vi "UHR-Fleezers Control (host) - 10.2.vi"() -> ()   [LabVIEW 2010]
uses:
  <vilib>/rvi/interface/nirviMethod/nirviMethod.xnode
  <vilib>/rvi/interface/nirviCloseFPGA/nirviCloseFPGA.xnode
  <vilib>/express/express analysis/Spectral/XNode/ExpressSpectralMeasurementsBlockNode.xnode
  <vilib>/rvi/interface/nirviReadWriteControl/nirviReadWriteControl.xnode
  <vilib>/Analysis/NI_AALBase.lvlib
  <vilib>/express/express analysis/Spectral/Block/exnSpectralBlock spectral measurements PSD poly.vi
  <vilib>/rvi/interface/nirviOpenFPGA/nirviOpenFPGA.xnode
  <vilib>/vision/Avi1.llb/AviRefnum.ctl
  <vilib>/Platform/TimedLoop/XDataNode/XDataNode.xnode
  <vilib>/Platform/TimedLoop/XDataNode/nitl_modes.ctl
  <vilib>/Platform/TimedLoop/XDataNode/XDNodeRunTimeDep.lvlib
  <vilib>/Platform/TimedLoop/XDataNode/wakeup.ctl
  <vilib>/Platform/TimedLoop/XDataNode/timing_clust.ctl
  <vilib>/Utility/miscctls.llb/LVPoint32TypeDef.ctl
  <vilib>/userDefined/High Color/nirio_resource_hc.ctl
  openfpgaref.8.6.ctl
  <vilib>/Utility/miscctls.llb/LVMinMaxIncTypeDef.ctl
  <vilib>/rvi/errors/niLvFpgaWhatHappensToTopLevelVI.ctl
  <vilib>/rvi/interface/common/niFpgaNodeNameForErrorReporting.ctl
  <vilib>/rvi/errors/niLvFpgaAdjustHostInterfaceError.vi
  <vilib>/vision/NI_Vision_Development_Module.lvlib
  <vilib>/Instr/_visa.llb/VISA Configure Serial Port (Instr).vi
  <vilib>/RVI Host/nirviSupport.llb/nirviErrorClusterFromErrorCode.vi
  FPGA Bitfiles/UHR-Fleezers Instr~3C_FPGA Target_UHR-Fleezers Contr~4B.lvbitx
  <vilib>/Waveform/WDTOps.llb/WDT Append Waveforms DBL.vi
  <vilib>/express/express analysis/Spectral/Block/exnSpectralBlock spectral measurements PSD WFM.vi
  UHR-Fleezers Control (fpga) - 10.3.vi
  FPGA Bitfiles/UHR-Fleezers Instr~F0_FPGA Target_UHR-Fleezers Contr~5A.lvbitx
  <vilib>/FPGAPlugInAG/PCIe-7852R/niLvFpga_Close_PCIe-7852R.vi
panel:
  in  "Sample Channel Flow":bool
  in  "Pump 3 contents":string="Left: ADig beads" caption="contents"
  in  "Pump 1 contents":string="Right: DNA beads" caption="contents"
  in  "Scripts":T1(tab)=enum."Stepping data"
  in  "Take Stepping Data":bool
  in  "Cap 1 Samp Flow ON":bool=TRUE
  in  "Cap 2 Samp Flow ON":bool=TRUE
  in  "Got DNA bead":bool
  in  "Got ADig bead":bool
  in  "Cap 2 Flow ON":bool=TRUE
  in  "Cap 1 Flow ON":bool=TRUE
  in  "Cap 2 T ON":bool=TRUE
  in  "Move Cap. 2 (ADig Left)":bool
  in  "Move Cap. 1 (DNA Right)":bool
  in  "Cal/Data Acq. Spot":bool
  in  "Dump Beads":bool
  in  "Lower Ch. Cap.":bool
  in  "Cap 1 T ON":bool=TRUE
  in  "Offset 2 Set":dbl=2.0
  in  "Offset 1 Set":dbl
  in  "Cal @ (MHz)":dbl=15.0
  in  "W/ Offset 1":bool=TRUE
  in  "Offset 1 Start (MHz)":dbl=13.0
  in  "W/ Offset 2":bool=TRUE
  in  "Offset 2 Start (MHz)":dbl=16.0
  in  "Move to Delta 2 (MHz)":dbl=13.0
  in  "Attempt Limit":dbl=30.0 caption="Limit"
  out "Attempts":dbl=1.0
  in  "Wait Before Save (s)":u32=1
  in  "Fish for Tether":bool
  in  "Closest Delta (MHz)":dbl=9.5 step=0.25
  in  "Stop F (pN)":dbl=3.0
  in  "Then...":string(combo)="5"
  in  "Move to Delta 1 (MHz)":dbl=13.0
  in  "Tether Alarm?":bool=TRUE
  out "Tether":bool
  in  "TA Cancel Save?":bool=TRUE
  in  "TA Green Off?":bool=TRUE
  in  "Raster Set Upon Tether":u32=1
  in  "Save at end (5, 6)":bool
  in  "N Steps":dbl=20.0
  in  "Step Size (nm)":dbl=0.34
  in  "Save ave factor":dbl=1.0
  in  "Dip Trap Delta 1 (MHz)":dbl=15.0
  in  "Move Trap Before?":bool
  in  "Save Data After?":bool
  in  "Green ON After?":bool
  in  "Dip Trap Delta 2 (MHz)":dbl=15.0
  in  "Move Trap After?":bool
  in  "Duration (s)":dbl=1.0
  in  "Dip for Protein":bool
  in  "APD to Watch":bool
  out "Duration (s)":dbl
  in  "Action":string(combo)="Yank"
  in  "Fl. Triggered...":bool
  in  "Fl. Delta Thresh. (kHz)":dbl=0.6
  out "Waiting":bool
  out "Fl. High":bool
  in  "N pts to average":u16=6
  in  "Yank Delay (s)":dbl=3.5
  in  "Yank to Delta Array (MHz)":dbl[](array[numeric])=[16.3, 15.85, 14.85]
  in  "N Array El":u8=3 min=1 step=1
  in  "Random Choice":bool=TRUE
  in  "Force Yank":bool
  in  "Force Reset":bool
  in  "Y change (mm)":dbl
  in  "Profile":bool
  out "Current Position":cluster{dbl, dbl, dbl}
  out "Sigma/Mean 2":dbl=nan caption="Sigma/Mean" format="%#_2g"
  out "Rate sigma (Hz) 2":dbl caption="Sigma (Hz)" format="%0.2f"
  out "APD 2 Rate (Hz)":dbl format="%#_3p"
  out "Primary Video Display":T2(plugin-control)
  out "Waveform Graph":dbl[](graph) caption="APD Line Scan"
  in  "Inject Pump 3":bool
  in  "Inject Pump 1":bool
  out "Messages":string="4:54 PM\tLost tether (723 s).\r4:42 PM\tFormed tether in 1 attempt(s).\r4:41 PM\tLost tether (470 s).\r4:34 PM\tFormed tether in 7 attempt(s).\r4:32 PM\tLost tether (992 s).\r4:15 PM\tFormed tether in 1 attempt(s).\r4:14 PM\tLost tether (454 s).\r4:06 PM\tFormed tether in 5 attempt(s).\r4:05 PM\tLost tether (206 s).\r4:01 PM\tFormed tether in 3 attempt(s).\r4:00 PM\tLost tether (153 s).\r3:57 PM\tFormed tether in 5 attempt(s).\r3:56 PM\tLost tether (759 s).\r3:43 PM\tFormed tether in 17 attempt(s).\r3:39 PM\tUHR-Fleezers ready.\r"
  in  "APD Ave N":dbl=10.0
  out "Int. Time (s)":dbl=3.0
  in  "Stop All":bool=TRUE
  out "Sigma/Mean":dbl=nan format="%#_2g"
  out "Rate sigma (Hz)":dbl caption="Sigma (Hz)" format="%0.2f"
  in  "Tab Control 6":T3(tab)
  in  "APD 2 Offset":dbl
  in  "APD 1 Offset":dbl
  out "RMS (Ang)":dbl=2.2363215515597568 format="%_2g"
  in  "Bead Sep. Int. Time (s)":dbl=5.0 caption="Int. Time (s)"
  in  "Below (kHz)":dbl=0.5
  in  "Above (kHz)":dbl=2.0
  in  "Adjust Scale\nto Mean":bool
  in  "Rescale on Mean":bool
  in  "Offset (nm)":dbl
  out "Mean":dbl=0.35502251163091847 caption="Mean (pN)" format="%#_3g"
  out "Force":waveform(dbl)[](graph)=[{"t0"=timestamp(4478.100000001255 s since 1904-01-01), "dt"=0.15, "Y"=[0.6544682133105884, 0.6829563430169571], "attributes"=variant("NI_ChannelName"=variant(string "T1 X"))}, {"t0"=timestamp(4478.100000001255 s since 1904-01-01), "dt"=0.15, "Y"=[0.05685503756215739, 0.025810452633971234], "attributes"=variant("NI_ChannelName"=variant(string "T2 X"))}]
  out "APD Chart":waveform(dbl)[](graph)=[{"t0"=timestamp(4478.100000001255 s since 1904-01-01), "dt"=0.15, "Y"=[0.0, 0.0], "attributes"=variant("NI_ChannelName"=variant(string "APD 1"))}, {"t0"=timestamp(4478.100000001255 s since 1904-01-01), "dt"=0.15, "Y"=[0.0, 0.0], "attributes"=variant("NI_ChannelName"=variant(string "APD 2"))}]
  in  "Calibration":u16(ring)=2 items=["None", "Position", "Force"]
  out "T1 X":dbl=0.6687122781637727 caption="T1 X (pN)" format="%0.2f"
  out "T2 X":dbl=-0.04133274509806431 caption="T2 X (pN)" format="%0.2f"
  out "Bead Separation":waveform(dbl)(graph)={"t0"=timestamp(4478.100000001255 s since 1904-01-01), "dt"=0.15, "Y"=[-2.9090620115549504, -2.8815158675481127], "attributes"=variant("NI_ChannelName"=variant(string "T1 X"))}
  in  "Amplitude (nm)":dbl=3.0
  out "Bead Mean (nm)":dbl=-2.9725093766937554 caption="Mean (nm)" format="%0.2f"
  out "Difference":dbl=0.6273795330657084 caption="Difference (pN)" format="%.2g"
  in  "Take Detection Laser\nImage":bool
  out "APD 2":T2(plugin-control) caption="APD 2 (Cy5)"
  in  "Flip Green Filter":bool
  in  "Set X Only":bool
  in  "Set Y Only":bool
  out "APD 1":T2(plugin-control) caption="APD 1 (Cy3)"
  out "Detection Laser Y":T2(plugin-control)
  out "Pointer Y (V)":dbl format="%_3g"
  out "Pointer X (V)":dbl format="%_3g"
  in  "Set Confocal Spot (X-Y)":bool
  out "Detection Laser X":T2(plugin-control)
  out "Saved APD":dbl[][](graph) caption="Most Recent Time Trace"
  out "Trap Delta Graph":dbl[](graph)=[-89.38744840610437, -89.37006347356015, -89.24966097161428, -89.27535644051642, -89.22559285551776, -88.86555051929984, -88.57164165504085, -88.51902465601101, -88.63501771008777, -89.20867383045751, -89.55461281382372, -89.55813284408976, -89.07876691073398, -89.12824891342606, -88.87613266846802, -89.2801470410057, -89.52897456305874, -89.30818962554463, -89.2603892282628, -89.55143394553988, -89.11898533922138, -89.25742201435101, -88.7246017921867, -89.05704019082833, -89.00438612954582, -89.05564776220227, -89.01771654795576, -88.8637677243877, -88.73420125440117, -88.90230035101814, -88.93449064288166, -88.68475787636112, -88.71497640229151, -88.98867971389947, -88.98987818265206, -88.8663554218612, -89.21049798942109, -88.87888603452649, -88.83494841134385, -88.8517410807533, -88.94938680318202, -88.98692447842114, -89.13767155188884, -89.05931890170092, -89.08641661114396, -89.05365179724527, -89.20227840355159, -89.31178251999566, -89.45607605619048, -88.83940363384923, -89.15369570967569, -89.08546468517298, -89.05175431278485, -88.87130156752026, -89.02771493961416, -89.34443740021561, -89.4552359343601, -89.16107171540548, -89.11889587027639, -89.3436162545047, -89.33942660204508, -89.3473584178231, -89.19585027499929, -89.139379143746, -89.2555989459276, -89.20141717607427, -89.21660561984382, -89.46769272591796, -89.07315603501014, -89.03933689450355, -89.0993712485838, -89.35756915821324, -89.35331075709209, -89.22317576092196, -89.508816612592, -89.2518218067191, -89.20936039087964, -89.44092145450193, -89.6477278697556, -89.08293610392039, -89.53347805395603, -89.64410456441405, -89.35761400349834, -89.34886843709035, -89.37851091701371, -89.41649939174766, -89.36071107503787, -89.57311912534034, -89.63101869252588, -89.43405030861993, -89.31069880452256, -89.3430526304503, -89.21823174554396, -89.21501556105062, -88.9111722206407, -89.18733719432157, -89.18722963976052, -89.32292422573383, -89.39588663013811, -89.82453679095343, -89.10638459364176, -89.47188371738739, -89.54185028737668, -89.5729147724991, -89.54460422995446, -89.18025179411762, -89.34220054522804, -89.5575088561865, -89.42069201414144, -89.26950662803745, -89.10557494488836, -89.34610419003715, -89.49955675225459, -89.22456738111956, -89.2027117963072, -89.1349219342003, -89.14160870895898, -89.33136024231399, -89.33342512716312, -89.37714552414755, -89.3803929736005, -89.35573543764183, -89.52038271838603, -89.27965821960461, -89.35600452793587, -89.22650740978278, -89.22614620509182, -89.12635779184048, -89.48788165476256, -89.13068590269111, -89.17357255767598, -89.08072258562063, -88.86940497190369, -88.77122041116284, -88.99968531958817, -89.00921784902013, -88.81448561314173, -88.84031989144572, -89.39146413421481, -88.86339059547717, -89.1673772901552, -89.15159384824292, -89.06085219395777, -89.51260432037202, -89.5536217833934, -88.98677652908017, -89.2701030586531, -89.24195272293136, -89.71292340734871, -89.2910030757885, -89.47786455696955, -89.48954430167501, -89.26584207463125, -89.10233578501436, -89.17707533292848, -89.305147933605, -89.18901651866418, -89.34296303989353, -89.09380910376896, -89.463391307056, -89.57679916102225, -88.71111300258505, -88.94498405110207, -88.49140535622053, -88.7341514685107, -88.89889681017223, -88.59002712151397, -88.76524603655983, -88.87121714891552, -89.1510876045764, -88.91862351911718, -88.82548575374531, -88.80051417887705, -88.54837294030075, -88.87140478869503, -88.89456579635265, -89.0056346348357, -88.55907846911137, -88.66759749781659, -88.44149474414237, -88.6870846816969, -88.6466799778529, -88.63814297254739, -88.78805261976106, -88.96824024662688, -89.1103699249511, -89.3905085878867, -88.9323741748437, -88.75430601059085, -88.82089140957092, -89.4535647245052, -88.85616866717044, -88.79523221810146, -88.9348514263713, -89.16871433406047, -88.67265636299146, -88.56040235473944, -88.91232897311664, -88.8089571372157, -88.91314583351732, -88.88683122051, -88.68204457129616, -88.85998808560862, -89.14884267359204, -89.22322206568205, -88.95108210276138, -88.64718246491319, -89.13249650680967, -88.76829543884, -88.95527962559021, -89.21056707808899, -89.0089527300235, -88.91866866096028, -88.80863987306557, -88.80089852688, -88.78342735706066, -88.56360335694336, -88.67735013119068, -88.59275253806658, -88.69077558769106, -89.13757241655324, -88.73750458538608, -88.78152831683693, -88.99066615201534, -88.82091590097372, -88.82476418112773, -88.85316711473837, -88.66503995216488, -88.79388285985826, -88.9563338555671, -88.71352135994421, -88.83999603213721, -88.74633806352192, -88.60900128977838, -88.53872550741977, -88.18424116231269, -88.3705578352791, -88.62148742046897, -88.54394496460543, -88.36251412656927, -88.4093878967337, -88.50258216055909, -88.35494559212471, -88.34341283426755, -88.37395270939074, -88.4979905289099, -88.46189758015758, -88.26844057461545, -88.2326502387395, -88.55042578244075, -88.63499132099773, -88.51319899426838, -88.73389987228151, -88.26715288988908, -88.21859961845635, -88.58277595542361, -88.59002127369436, -88.55251451009755, -88.37746006671004, -88.41015869076773, -88.51995467108634, -88.20521115956211, -88.2804480699595, -88.43819946605072, -88.33640124221915, -88.6531593764619, -88.34679755650652, -88.52043428631671, -88.95056941775016, -89.15761826470202, -89.0652452180153, -89.29976884961121, -89.28829699493275, -88.2664323951737, -88.30873224535377, -88.44209877116936, -88.24099191432931, -88.22287833843131, -88.29139893670066, -88.46447280750237, -88.3910852296664, -88.29985148131229, -88.30822091752688, -88.28362819582696, -88.48902213455159, -88.54998575425876, -88.60669758609019, -88.49144847059677, -88.16296003837576, -88.51396970073476, -88.33982443813122, -88.22394802157045, -88.29260704896129, -88.41055824500185, -88.33497551461949, -88.67759606488578, -88.58700366093623, -88.35694653040895, -88.47296601718023, -88.33423129919967, -88.47752188464662, -88.35512247733888, -88.3777986712967, -88.729655522916, -88.73598917774595, -88.51630362857102, -88.2074894465274, -88.29181479700983, -88.4672686755314, -88.16849552794635, -88.5951381838874, -88.13062428528687, -88.17216964798284, -88.10524634348789, -88.27800416343854, -88.13335451761374, -88.37825316932381, -88.56140566187452, -88.4425002811831, -88.0656866086508, -88.42547083397028, -88.25095406936146, -88.30824818401392, -87.68332283229768, -88.17932407982077, -88.1532062150512, -88.53375395739056, -88.30311164463794, -88.41589198652929, -88.30407778660808, -88.40367169747444, -88.3437214846239, -88.35594639765567, -88.45652784227724, -88.5842630911653, -88.41297448484298, -88.54859586632723, -88.58103611816637, -88.84792541633075, -88.01907631016554, -87.95324520506506, -87.78481343426844, -87.95560385851115, -87.85804482449285, -88.18551136231898, -88.01656053816524, -88.02895257484454, -87.92828548442509, -87.79710285471337, -88.00738538313797, -87.73682830549747, -88.07275568855894, -87.99433270558389, -87.72770755009651, -87.9267710314997, -87.96904944990774, -87.9253259336599, -88.05705393409421, -88.01203421488725, -87.91328847459181, -87.8071326736109, -88.01735651800155, -88.01900222553235, -87.9545136667229, -88.12450941379944, -87.93910654707737, -87.87354402092201, -87.92735293954016, -88.19340411458231, -88.30401091141142, -87.95775584337821, -87.73163787609764, -88.15344693968393, -87.96650228747762, -88.11064491691332, -87.54860462573924, -88.09354412638375, -87.8519133361432, -87.85881854278162, -88.20509785833131, -87.91760524446005, -87.95035519016639, -88.04278622326103, -88.02524699015602, -88.15194655200104, -88.00407435605808, -88.05793027060378, -87.77335005358424, -88.16544477454528, -87.89450200769897, -88.13982524656109, -87.97826541537938, -88.16268206508684, -87.71879293293877, -87.94985415206207, -87.8064061100325, -87.99934582850895, -88.22615609606846, -87.86093151137626, -87.6700537142207, -88.03078580167295, -87.87513742989012, -87.82347052576961, -87.94732046431275, -88.1156839391357, -88.20232764763225, -88.2994531521694, -88.18386916539099, -88.09031322297545, -88.15313742433287, -87.80239936551692, -87.60250611850887, -87.64533018569459, -87.60991041695632, -87.72676066199486, -87.33559917500989, -87.45284913194946, -87.25817364254561, -87.65430559235227, -87.53602431965585, -87.39786877894335, -87.58615486117924, -87.43227285896955, -87.71344886287676, -87.23377729485536, -87.64014203399677, -87.60239562637292, -87.2919811059202, -87.37115314323583, -87.37275952371664, -87.15051723589367, -87.39185774051927, -87.48653698268699, -87.45749749831653, -87.18067937552632, -87.27483719659506, -87.41864167455336, -87.25027078789361, -86.98471314584748, -87.28270035864435, -87.57027222590403, -87.7665499148163, -87.37999966120944, -87.28971186976376, -87.52306556218589, -87.36410821351811, -87.48529464229739, -87.44136200138482, -87.58907511569913, -87.78643723152783, -87.55681182743275, -87.48385705148843, -87.63330822003329, -87.61184020150489, -87.71616882826622, -87.5282648586323, -87.57071058488614, -87.57236293781206, -87.31757130397664, -87.77813876094464, -87.6257729513794, -87.69068528914049, -87.84520252155934, -87.86085934550638, -87.88195380904611, -87.60311641516779, -87.69122196636401, -87.8020108027814, -87.83361495277228, -87.67067092860452, -87.58389183513452, -87.56129213793758, -87.85975339337645, -87.40220585601887, -87.91728954021838, -87.75864018540607, -87.74689815457056, -87.68245059351156, -88.18451430943892, -87.88738917293477, -87.63757611994254, -87.5708434435605, -87.77278345407868, -87.93142286703629, -87.86352661774805, -87.76673769548492, -88.01908196291075, -87.89074636276199, -87.72684473268411, -87.57289839262214, -87.71597780604532, -87.78577424237625, -87.69032008091057, -87.62589406030267, -87.8174289613667, -87.67707669627433, -87.51845749917389, -87.71466525148008, -87.5606836249847, -87.7139674908129, -87.74094794957122, -87.7005157479694, -87.76640578300322, -87.70527246506592, -87.71611718410986, -87.81476293350636, -87.79251662258699, -87.88265447337088, -87.75795727658604, -87.9823722895671, -88.0836963787135, -87.62714330665065, -88.0089934508544, -87.40707301914264, -88.05177962004032, -87.8229318229869, -87.94390489036448, -87.84493365424993, -87.59509612382958, -87.72856415566281, -87.81497085062107, -87.92128557509571, -87.75918240002704, -87.93548815031771, -87.9012355596515, -87.54139193308774, -87.55828881541663, -87.51056903539299, -87.52039866561812, -87.63682624093673, -87.5432671707731, -87.64742561154168, -87.3288423556632, -87.48046022363206, -87.58910493044621, -87.6911525123038, -87.37349047159623, -87.4448807965905, -87.28808399952601, -87.54929046394128, -87.45969579508173, -87.58502984558035, -87.80226057043029, -88.0303971858355, -87.60810918962494, -87.84113021898624, -87.54927790962793, -87.56484012122169, -87.28054131732654, -87.70220256814717, -87.76341332349702, -87.54370605152829, -87.79205016647634, -88.09313027253401, -88.0620175534996, -87.94063041986826, -87.96896727307845, -87.80256403811197, -87.67239701062852, -87.6399317276719, -87.65889725479741, -87.28729774193249, -87.5214594744474, -87.62016692063344, -87.62735969457016, -87.45027005933, -87.21012664990556, -87.06867512023265, -87.33435958229319, -87.3177444330734, -87.34788825501778, -87.56436416954135, -87.61950903708983, -87.55425148575165, -87.55083323246308, -87.68012788709825, -87.51834206500418, -87.69598428135353, -87.71876397280123, -87.44913472298718, -87.6048484121969, -87.864444966875, -87.5501946692936, -87.45216722120793, -87.58237945926253, -87.78969615154085, -87.67686931387769, -87.5522680359406, -87.44068603371, -87.76799995194563, -87.60672463029596, -87.38968106380253, -87.63066293473824, -88.02940059078153, -87.86955200993, -87.9565636486737, -86.8106204704307, -87.18970625895963, -87.86114644151831, -87.58153303504436, -87.35048262951038, -87.51654038824094, -87.52922696429981, -87.36262242324574, -87.41629136303413, -87.28824237872385, -87.4798012921965, -87.41374424314733, -87.49898141290439, -87.49418606631315, -87.51862153043166, -87.71063407904339, -87.6430033186609, -87.57827338876646, -87.54690816845391, -87.37313105200109, -87.46919199453606, -87.25478433494307, -87.57636908224944, -87.58441520954747, -87.54338977306715, -87.67092323117731, -87.75299003095911, -87.48833905986369, -87.68958700633844, -87.45965031693086, -87.66116717927812, -87.27532000081274, -87.57990013934989, -87.3358908739909, -87.50397985078497, -87.46173599047975, -87.48897346231755, -87.72646057917159, -87.92686417098798, -87.66179360238937, -87.71096805882274, -87.58618277512232, -87.6988941155976, -87.5326287528062, -87.80961641383038, -87.30238479981065, -87.03358687200033, -87.2089031253125, -87.2851268921435, -87.57229679049586, -87.6250778220362, -87.63097627402095, -87.57340931013754, -87.37087860062384, -87.44919654211628, -87.55770928649892, -87.32390714182918, -87.3792060612991, -87.82257062874059, -87.91123683327902, -87.65663152557195, -87.45233009538237, -87.4503607791947, -87.44856346726229, -87.54674508286985, -87.48734914385216, -87.53493633794486, -87.77322141957666, -87.5360093515083, -87.92890453759716, -87.74937580384537, -88.0245676727105, -87.68532561768353, -87.63053250593893, -87.78213147465999, -87.78859059897012, -87.86455124009606, -87.82301747913752, -87.74384895388138, -87.53642726658066, -87.70265895169524, -87.6807943581295, -87.67232336986555, -87.55827287052955, -88.07948443555617, -87.63008108422747, -87.5546049107237, -88.02124763911905, -87.79747135539168, -87.69866730651353, -87.4907995965221, -87.66252496338981, -87.66651266475806, -87.32618843167079, -87.56224440214163, -87.7667193383105, -87.67475148682402, -87.67403549332289, -87.95538747106701, -87.84275776737468, -87.87501919379514, -87.71447099135949, -87.38634807332252, -87.67076191051662, -87.5610535281519, -87.72945280500126, -87.77329172363045, -87.58111844851547, -87.392924048304, -87.99966297359707, -87.66302572401112, -87.70180504315596, -87.7633988137739, -87.49898068274233, -87.60398327290125, -87.55264054889946, -87.7317147994365, -87.44896090874326, -87.73988451581835, -87.6824066023823, -87.7957256934875, -87.61022656628427, -87.63754876347582, -87.5711889574363, -87.81578244682522, -87.51567128404804, -87.5154423142066, -87.52661520916558, -87.90110240253, -87.72240271355116, -87.68284011358159, -87.47969610871385, -87.59549328973137, -87.49486631433797, -87.46292721937864, -87.53242593240981, -87.45177658061101, -87.49650273688985, -87.42222432382316, -87.40924809559812, -87.46155584573685, -87.67740538525773, -87.56795415780982, -87.38569221168117, -87.72497836510254, -87.63212095662197, -87.84874086155294, -87.68423502594806, -87.69248881745025, -87.55053270519312, -87.63792276742947, -87.79361374259113, -87.82594928518766, -88.02381615123241, -87.78573568385676, -87.627134578756, -87.48447531083156, -87.73805939615202, -87.48798012324937, -87.33294279112297, -87.4083676430875, -87.2125741263701, -87.64422154601172, -87.79647571090814, -87.60503235567646, -87.468032119514, -87.5182669364431, -87.69978210057371, -87.50350852296302, -87.05604169095596, -87.54120213385531, -87.52140297291606, -87.40543345419292, -87.5303247718758, -87.53081075788629, -87.29491010008809, -87.55816400580258, -87.41618663405671, -87.40015492786631, -87.66754109572479, -87.64535395323043, -87.7226826283207, -87.76140908067617, -87.55084152605826, -87.67412930855458, -87.66651847157189, -87.59259808382153, -87.76203239123596, -87.82422546599133, -87.83988157302704, -87.63815911780895, -87.49616243720268, -87.33562809133211, -87.4146581786975, -87.57917461085796, -87.58962249843225, -87.530135156205, -87.09582028024963, -87.24486712722238, -87.41117686085059, -87.43803047596957, -87.73298888735778, -87.54712937634724, -87.46411106964821, -87.54784999696707, -87.56584887970729, -87.4903532769867, -87.51231599593729, -87.33147942981621, -87.36305774594335, -87.89964736785245, -87.53883983178878, -87.53308382106005, -87.47942176100906, -87.56968963749078, -87.69694395129795, -87.60185059154233, -87.40409833135215, -87.48565441094152, -87.45295785173542, -87.8598746465701, -87.63829115936099, -87.72329824070167, -87.57755847822077, -87.34233590638961, -87.2456387390855, -87.69022291588266, -87.73497292018078, -87.67861746974165, -87.86636101340743, -87.86785313484236, -87.63076103469672, -87.73204340004872, -87.79896896759101, -87.81165856747944, -87.78886319309825, -87.47167338848682, -87.79033896032894, -87.7394988120906, -87.3593100996421, -87.67569559372204, -87.77973202885244, -87.55832238989285, -87.79523137457565, -87.47172572986554, -87.69117985917633, -87.8026233792443, -87.68335651454673, -87.71072805299252, -87.35688163306679, -87.68247685399328, -88.04111074383601, -87.71006837060239, -87.56964717410253, -87.67187827443692, -87.39882043046879, -87.49501995524523, -87.29313321533394, -87.58729015911976, -87.27415480591418, -87.553455177222, -87.28462813652112, -87.39034628415033, -87.58108941169114, -87.44564719863513, -87.53436292084444, -87.33001410378813, -87.36337024723107, -87.63510719338177, -87.65980368332251, -87.43363496068739, -87.4255269325382, -87.41182525493925, -87.72815339935283, -87.67216110676736, -87.72283448284864, -87.6723969435237, -87.6560403010696, -87.38016535112635, -87.55609880554229, -87.5762178841565, -87.72026364293265, -87.69566289957541, -87.31489376030962, -87.52499386095835, -87.56560915150533, -87.71637669594824, -87.65296554469052, -87.78329628957886, -87.76052147520979, -87.86389250978719, -87.60691705192471, -87.73801394328754, -87.53083942658031, -87.4768796085828, -87.78184542579447, -87.54612819815853, -87.36965481448632, -87.4204871602231, -87.50661200564672, -87.4524351274625, -87.76563007263547, -87.81140346193699, -87.35314925668533, -86.10503470178419, -89.85266012832051, -89.64460892206411, -89.63573878694366, -89.67437474838317, -89.43897047411551, -89.3737613977331, -89.28788917865882, -89.58069848429386, -89.53810567580396, -89.37138670815206, -89.42570077300456, -89.54084483748144, -89.38127981165223, -89.5094888428512, -89.43628497289689, -89.82742727406759, -89.58878997780671, -89.05083051594639, -89.2715449510282, -89.18302882011236, -89.11757972469984, -89.450025337766, -89.4918182082358, -89.48714535759302, -89.45673286538067, -89.3721865723953, -89.22628822081519, -89.54189155991992, -89.3527578161816, -89.55295636678755, -89.61525268024653, -89.60177253387754, -89.35091333052947, -89.65096893870835, -89.43826482992947, -89.26405785507977, -89.13333984803354, -89.27090710005496, -89.61146885238918, -89.38160521758422, -89.41398091645064, -89.56444238217698, -89.55467011390908, -89.49128237350648, -89.50437810521063, -89.49811847441696, -89.58142008085757, -89.70565907063485, -89.79032016312806, -89.49368126396514, -89.43538457890372, -89.22236432143751, -89.30147719799409, -89.6871672866815, -89.39666762420819, -89.53287835086593, -89.53103400899184, -89.30264681130458, -89.20241016917116, -89.20185024762415, -89.14667769335148, -89.4091163236507, -89.5303897169196, -89.37364072083844, -89.36478136588747, -89.52127318590307, -89.47972650316281, -89.5730482533163, -89.62064623540789, -89.5836723763713, -89.51543500545677, -89.38239305279464, -89.62184644095112, -89.7728958272249, -89.683935508047, -89.67854975684114, -89.50641274850042, -89.66409060311157, -89.22826919030574, -89.5351698052126, -89.52386617594226, -89.5762566923911, -89.12011896829341, -89.39440120296695, -89.31526150363645, -89.40699770807561, -89.27641788881832, -88.9980934526029, -89.22189882622396, -89.18320922801408, -89.07312242319608, -88.83297400882918, -89.2234100301694, -88.85288595229059, -89.2377991335614, -89.35741830027712, -89.26107817432187, -89.43580762503471, -89.41514590200433, -89.45677685231738, -89.34136783820585, -89.21998788359926, -88.86601818955353, -89.36404024707687, -89.18530760698397, -89.43678951078016, -89.18406807997061, -89.37969189195263, -89.62263416697985, -89.37304214824837, -89.3440877767074, -89.3598322726397, -89.34954279527221, -89.19348306086874, -89.2146973031071, -89.43625648517998, -89.34417299103697, -89.52160411222111, -89.53337708387906, -89.342069859851, -89.5743618155725, -89.30272336229824, -89.15741114850327, -89.21817485093237, -89.30503477455262, -89.36081784103939, -89.52459993172579, -89.6111165131166, -89.2619524554189, -89.35664568024671, -89.22996326941124, -89.42804922425438, -89.42197549285336, -89.62869122920705, -89.38083285342586, -89.54868019256227, -89.31926914035074, -89.55393076075502, -89.39585117735736, -89.56232500771125, -89.58429220453907, -89.2853335425489, -88.9554979363846, -89.82366236227894, -90.03241697822503, -89.87535834289318, -89.68803825964758, -89.90985739705187, -89.65052212097332, -89.63592492369258, -89.68901377113175, -89.61580926284557, -89.47648673035042, -89.5763572557888, -89.62979756653974, -89.48581314130413, -89.60156409856245, -89.521773057561, -89.2283702112482, -89.36270907008742, -89.3762029830632, -89.37264199967436, -89.47817702167433, -88.96620231000924, -89.54818090594742, -89.80996257603499, -89.63617690920825, -89.27694912725786, -89.17404501094248, -89.36048391493902, -88.88941872416451, -88.84313652275561, -89.25869975047635, -89.51915145305644, -89.3148346155159, -89.23949602638928, -89.27060642492778, -88.82059631185331, -89.22377299622616, -89.40471068902889, -89.67545363713047, -89.7105622164905, -89.59379751329226, -89.43763803920422, -89.73367902969775, -89.25258989064338, -88.92196116042703, -89.49284759320145, -89.43652161750485, -89.14923694928899, -89.31570366092012, -89.14198709968517, -89.22103878715308, -89.31243636768616, -89.35968282595243, -89.45840321040957, -88.9639394112719, -89.41425315620818, -89.36940537708537, -89.43031076815686, -89.20706343917448, -89.43495800271168, -89.29789897809772, -89.17597071053217, -89.2602152121373, -89.55991216232033, -89.13369209792404, -89.26909295138859, -89.3238551922488, -89.48669087227324, -89.423659006272, -89.50933552398729, -89.60114730778753, -89.36920727072032, -89.20780895747096, -89.67447177677113, -89.88591928368581, -89.34584482112372, -89.44820280802116, -89.49125823457338, -89.6568084287604, -89.43129708145736, -89.19178935178499, -89.28690969251289, -88.84810710672292, -89.40764696202572, -89.98838207910475, -89.46179401598928, -89.96003721353357, -90.29385321683213, -89.60860309937391, -89.06511935921438, -89.03125538678515, -89.51945033113051, -88.9977216866873, -89.23373707873185, -89.21931962136915, -89.87772162313416, -88.81461035446387, -89.41037526458646, -89.21597949792773, -89.12932586845321, -88.89371870329344, -89.33259816499356, -89.40470973446673, -89.3877910698847, -89.29257692524722, -89.76283867032404, -89.10096113503705, -89.0024552709693, -89.3505470549878, -89.37600264393359, -89.26597700316711, -89.5802441405524, -89.57893446891464, -88.91904199379911, -89.3815923013336, -89.18055657100285, -88.96373412987602, -89.15474436507003, -89.05102563118294, -88.91995887489625, -89.07392479076549, -89.34741814351625, -89.87526391116663, -89.19926148148149, -89.119620884163, -89.0393605559567, -88.77208870822894, -89.32195301903197, -89.09069786094281, -89.19673976535732, -89.14714102710515, -89.10779711665595, -89.08023600035908, -89.04761082212389, -89.00208857126661, -88.96839649386507, -88.76778670987548, -89.17048722940753, -89.30230976822241, -89.29160258844252, -89.3333423944874, -89.21683284951314, -89.31454210337398, -89.05934971458657, -89.23120006336663, -88.88610370286466, -88.97987228055663, -89.55143616735391, -89.45064218424297, -89.0965360803919, -89.14366272878738, -89.31218063333657, -89.0432226236395, -89.307677489395, -89.34063352548658, -89.32168023132036, -89.3126281281213, -89.20696593023561, -89.05718230378571, -89.16465103462701, -89.11847781964123, -89.24427371080426, -89.23214449007804, -89.27216161870632, -89.46769195656496, -89.45641376742469, -89.44714253031034, -89.04140792595314, -89.24701195071574, -89.39451905841605, -89.08543130907711, -89.45861193371825, -89.89974996696542, -89.43123387431251, -89.08641401326244, -89.13619110631862, -89.1826801708081, -89.17246493676171, -89.15652161423958, -88.78487650718846, -89.11971463463695, -88.76150695192209, -89.22036295485265, -89.20267147034549, -89.11729408223869, -89.4393059908418, -89.14636436459836, -89.15795395207269, -89.4275262122909, -89.22238485841942, -89.21940749412003, -89.08009114913443, -89.48920642046721, -89.15156442516772, -89.45698509789325, -88.87338314085522, -89.11045757349817, -89.46914647939062, -89.39797361779893, -89.420351098198, -89.38772867407957, -89.53347062365026, -89.25834313541426, -89.41957494353836, -89.29725722999143, -89.32381954159032, -89.39665434288693, -89.27290066010944, -89.49545804363956, -89.27060062024876, -89.3447405329835, -89.08272641196109, -89.305114113685, -89.42518021075358, -89.2482325160118, -89.38755628933976, -89.42168348053734, -89.04454862092464, -89.14915329392596, -89.37450589674879, -89.04039420204515, -89.1981375340063, -89.17596255924028, -89.13528304594989, -89.00356265969344, -89.261399469586, -88.96269949077983, -89.14333106859672, -89.41455145051421, -89.04943284927722, -88.86088894489063, -89.17453593650691, -88.66918119841439, -89.294146960962, -89.00819033468315, -89.04068043481627, -89.17620516400488, -89.09515362657663, -88.95981966328938, -89.15098552560895, -88.86236589470138, -89.21890741278276, -88.98251136025263, -89.03656163327432, -89.06019956154205, -89.23130134405736, -88.85390859847459, -89.22274938143335, -89.31166831425534, -89.76364552125162, -89.69880521261672, -89.34933991804397, -89.40903838807759, -89.11958827058041, -89.34058831435459, -89.64853755096333, -89.15690431343052, -89.45072666387912, -89.13948595908302, -89.40378733596806, -89.4634451436483, -88.0871954402557, -90.2523886297195, -90.32635437152004, -90.24503616401293, -90.17296891811858, -89.96316337641721, -90.19549823074706, -90.23014161336732, -90.13269117603848, -90.13546395158026, -90.24674659520822, -90.40157823810915, -89.73909437391183, -90.096832647288, -90.07515881472611, -90.41954622389525, -90.3825268323373, -90.18163811914361, -90.32412477840575, -90.19229216788813, -90.44522597500249, -90.13766390475877, -89.66968325889837, -89.9126565384995, -90.35605823166685, -90.28443307623621, -90.2234051820104, -90.21097840754392, -90.1434932206816, -90.24664411952034, -90.16297084625032, -89.99669745613257, -90.21337271531756, -90.021247708263, -90.06112766083584, -90.15294351289444, -90.19356620613507, -90.51319106617697, -90.09652105317282, -90.16690415325345, -90.45503996596538, -90.55116792842264, -90.07640911035573, -90.36256889908509, -90.20735243748508, -90.5326486662778, -90.41875749798626, -89.96515492584263, -89.8797442385357, -89.99429197617584, -90.21637803668041, -90.23608863956005, -90.30275101535133, -90.41942234871539, -90.33711424926108, -90.42214648701524, -90.27257976521608, -90.05960656456891, -90.03794536093727, -90.08741347741497, -90.43472618317658, -90.2522644360195, -90.29086269882997, -90.40629287671857, -90.61792619604786, -90.36613512437535, -90.29050508079987, -90.48790384558785, -90.12556116500082, -90.40000509329306, -90.51190694229909, -90.48024005146416, -90.63891561252724, -90.64839317421082, -90.1166652138771, -90.07533432694785, -90.34473101826771, -90.43451148283822, -90.61504799434994, -90.35172125444156, -90.5824314759526, -90.42203000224241, -90.45334459367774, -90.50472974606436, -90.64884364476089, -90.30968289889046, -90.45213831077214, -90.39147347172283, -90.17120557360909, -90.47525243001763, -90.396195657183, -90.31707930262343, -90.48713957741559, -90.42975001686625, -90.29789082657939, -90.46790304802579, -90.0947530517084, -90.328084029011, -90.30997424183043, -90.37316674979998, -90.29985642166363, -90.45006812043209, -90.17167534801723, -90.25468560102487, -90.15474421553142, -89.83393535067671, -90.20056478170406, -90.00296367297801, -90.21273519120342, -90.03490472002353, -89.94516964918006, -90.11067497816705, -90.18166776257632, -89.98882698225557, -89.85974377965816, -90.26505571518203, -90.15363713435593, -89.93316277964567, -89.95255251704741, -90.09698121390325, -90.04473329210172, -90.20534251503767, -90.458225224308, -90.2193790684706, -90.4599285306242, -90.5129940662291, -90.42282464467658, -90.37899575214976, -90.51315578513703, -90.50498529009057, -90.49201239331842, -90.50509139004552, -90.65465381069006, -90.24135716282727, -90.49818058178988, -90.54508650659335, -90.590507880303, -90.22481588702846, -90.44954328100238, -90.42767895442282, -90.40665355719054, -90.46603422132092, -90.22992008635563, -90.40089196820325, -90.2634868147749, -90.10206808676487, -90.536708726445, -90.1142016245376, -90.14149772635739, -90.14744631109205, -89.96547180840015, -90.21348545778108, -90.19073297991473, -90.37810903808769, -90.36879841716365, -90.42386666329647, -90.3715419481675, -90.29534431533034, -90.4028894344913, -90.15910175646306, -90.37091186837088, -90.1514934185192, -90.08503985404151, -90.29758609982272, -90.24521262721103, -90.22694052004285, -90.34910590301128, -90.31444089221904, -90.35215687320854, -90.26487760335966, -90.26219431605509, -89.97109692967945, -90.33087070872675, -90.45526539699613, -90.46167631785531, -90.44946334620084, -90.26650949052697, -90.38637346294726, -90.30254359116161, -89.97816869969462, -90.12232129716138, -91.63843000396554, -89.7362298577711, -89.54498333392092, -89.49938002867206, -89.49058379559563, -89.55044220270838, -89.60560601688277, -90.17027697268526, -89.6463463438765, -89.53794199525763, -89.10021704348154, -89.5457703413785, -89.25321894536543, -89.33345773463982, -89.58058389614905, -89.5168680518304, -89.47368234056128, -89.4058238856133, -89.15141597620514, -89.19282754602571, -89.58609886577267, -89.37019238993713, -89.37365136237787, -89.64303187671761, -89.2393858200982, -88.80127698898539, -89.11581946876925, -89.80767872863254, -88.93708737205955, -88.90962554991867, -88.88195933948012, -89.25706660886158, -89.02345428583934, -89.3022672789113, -89.2838649764038, -89.14654756383041, -88.86384783388766, -88.9175525867171, -89.21412651700874, -89.04860439238527, -89.25613750447775, -88.96517619327935, -89.12360954681394, -89.11224916640745, -89.16770424614049, -89.06094806010964, -89.0191470090751, -89.45687258453175, -89.60591860772492, -89.29585239378879, -89.83889261634286, -89.41013138045021, -89.63967513661015, -89.25797313024034, -89.6814018591188, -89.68821168672036, -89.58541567807737, -89.54188235417723, -89.61661971119183, -89.40723078839817, -89.34843089690773, -89.60515585313834, -89.56246156265125, -89.59370346754119, -89.66038143523066, -89.62559461914364, -89.42478326266355, -89.73029454506324, -89.43000935590837, -89.428288891753, -89.37564130633967, -89.02189968500151, -89.10788041065231, -89.32596209412588, -89.39404483901504, -89.4129768306943, -89.22209321815708, -89.10303797163806, -89.24924057430192, -89.49693081718887, -89.70833547833459, -89.6786839552272, -89.64591606711676, -89.51344631340291, -89.41101181324719, -88.44650019934619, -90.17731549807735, -90.27908072664212, -90.30349753540256, -90.42640638338176, -90.5461620039406, -90.40250304826327, -90.55184676162722, -90.22330217548966, -90.34604266504405, -90.34685720527591, -90.43543106648633, -90.32093998642343, -90.74190071075202, -90.36816598571811, -90.20018695449596, -89.69118008843904, -90.5408534144869, -90.44853203217406, -90.19896449655212, -90.26215618254675, -90.39783468271995, -90.19854594234243, -90.26812455801539, -90.4749038130671, -90.38385254518266, -90.38905614539564, -90.34356884533197, -90.06500891937931, -90.45591618755515, -90.18150542797281, -90.19969514913056, -90.37320685771269, -90.61570682788782, -90.34813631956763, -90.13750975570412, -90.07569812371833, -90.37642677753739, -90.33435317419614, -90.22555657098471, -90.23895375028121, -90.270246205725, -90.37600302883945, -90.2835538905631, -90.28385266083197, -89.78164047619508, -90.196635103456, -90.4809556207527, -90.01232719313069, -90.06390676586018, -90.22571765197469, -90.01167064927066, -90.29315367326132, -90.58357366716768, -90.26604080937142, -90.38515554970854, -90.1664830928737, -90.25566610607, -90.29182101093004, -90.33159656914417, -90.29740664846878, -90.12152543912441, -90.22505748118813, -90.07255937894185, -90.32626829459986, -90.29779540771625, -90.04335682238323, -90.14280906535224, -90.55964225477469, -90.30453958962217, -90.19593466265141, -89.77794966586396, -90.22246406101418, -90.49007992662617, -90.26741236776786, -89.94141182542884, -90.23288838691548, -90.07689253262124, -90.01473799333098, -89.96463099083859, -90.07745323671415, -89.94899441375048, -89.95495681210551, -90.00328638642554, -89.86870577366334, -90.08219568718776, -91.38615529550509, -89.0821447095635, -89.16820375058256, -89.10993184807809, -89.35779724956876, -89.36303709784403, -89.49757924729965, -89.44022066961067, -89.72624177725754, -89.75530879533176, -89.30836834709211, -89.7946009825269, -89.55671449854206, -89.61780451376646, -89.79357732437859, -89.44162363081644, -89.33239502158372, -89.478663009932, -89.66432476618351, -89.4937459042744, -89.41688638394041, -89.44460080624765, -89.43006349407366, -89.53283286899145, -89.48506102868743, -89.40024490411534, -89.32159922616273, -89.49189035607932, -89.0906531149945, -89.57154035461157, -89.3279294963929, -89.5262028900506, -89.4618575942215, -89.04150927193281, -89.23254167591475, -89.32036225135491, -89.52639856617733, -89.6790289190201, -89.8305547288756, -89.23930386276109, -89.5796936157711, -89.32856869184184, -89.48158078475134, -89.72828762784434, -89.32988515382098, -89.82246553111887, -89.1985184370172, -89.53893988629702, -89.54004424539605, -89.31296804318146, -89.40664149900778, -89.4095605730308, -88.90452677109064, -89.27638428969453, -89.4867258866616, -89.30965894808136, -89.05026439296921, -89.20221731059893, -89.15241321656985, -89.03046768602977, -88.97775540843435, -89.35393638033742, -88.87746997687707, -89.01446489393777, -89.42998809448717, -89.41951629723886, -89.29657619825127, -89.66517853351598, -89.26719513501837, -89.19856737181169, -89.31331613858958, -89.20024330138921, -89.68675314326693, -89.18691067885689, -89.44827735606182, -89.56832116008042, -89.3991673752302, -89.35338237886637, -89.19281493368959, -89.5844563456998, -89.59068903809967, -89.58125550151313, -89.55030349938028, -89.48631315915387, -89.49298165244711, -89.19463050450781, -89.41437069631509, -89.12268571079467, -89.18900910332924, -89.3859894958023, -89.25519191016045, -89.66257524290295, -89.33650806620477, -89.20722749651145, -89.38932496965388, -89.29148478789386, -89.39818187499321, -89.15663754761036, -89.5072792261119, -89.32672769334965, -89.57350830973445, -89.05634034293683, -89.00490134040983, -89.01083406418745, -89.37676924966965, -89.21254475296408, -89.03124620071928, -89.39281240345495, -89.33884438506695, -89.33682455468552, -89.49510453196741, -89.2372114044394, -89.55110664840826, -89.46857253003795, -89.05525600766862, -89.51341705464556, -89.49189351125247, -88.69254044548302, -88.8764894755446, -89.17120213281257, -89.22492294329365, -89.63664086781168, -89.74122661974911, -89.42327979427549, -89.55211561515353, -89.33928655995086, -89.30731392907573, -89.42224560331604, -89.21698045572563, -89.30015620250015, -72.02170105722757, 0.14802746146348256, 0.18182087058933108, 0.23145938781077158, 0.3745260603907764, 0.14339761464982548, 0.13744307201019235, 0.1999682238582624, 0.0488607450323251, 0.18909217445305565, 0.15803496802367173, 0.14030285755402744, -0.029758937979426924, -0.07388335400978263, 0.05173577743792419, 0.1120128372807348, -0.18369537610293946, -0.11094340057605118, -0.20700246867226446, 0.10559275090425473, -0.04850788802633353, -0.13341306859012336, -0.175179384438497, -0.147304334629956, -0.046157193510941066, -2.110428849563225, -2.827260759231172, -2.7882000038039294, -3.065306614418958, -2.6738823113174797, -2.840374309742303, -2.8750738677830467, -3.1398929972536034, -3.2420787696181153, -2.909460090063946, -3.322654750798421, -2.9504354301491165, -2.892884216735465, -2.6600659669938373, -2.962705147898145, -2.8667664458259563, -2.9913143616991413, -3.0237422733393706, -3.1941671849037543, -3.100885335284091, -2.648488912011631, -3.1201611300592274, -2.8671399365956125, -2.9393444108016835, -2.889238638161287, -3.067559137434417, -2.907857804168715, -2.715504853234837, -2.943189444947173, -2.749942778041302, -2.765556336531846, -2.8495372144488034, -3.2467998174444275, -3.0843775217642735, -2.7246418838225157, -2.915095163918644, -3.28651986346745, -2.868575252095781, -3.2263560407303267, -2.665341243673598, -2.9235009817725723, -2.7262262496104523, -2.956706675877592, -3.0687540749024307, -2.7511714031298604, -2.6762217304609814, -2.597560824458633, -3.1314839397787306, -2.939241757727324, -3.3114231119313624, -3.083958003204651, -3.018880629301152, -2.6562071342673255] caption="Most Recent Time Trace"
  out "Save APD Deriv":dbl[][](graph) caption="Most Recent Time Trace"
  out "Delta Fl. 1":dbl
  out "Delta Fl. 2":dbl
  out "All Signals":waveform(dbl)[](graph)=[{"t0"=timestamp(4478.100000001255 s since 1904-01-01), "dt"=0.15, "Y"=[0.0, 0.0], "attributes"=variant("NI_ChannelName"=variant(string "APD 1"))}, {"t0"=timestamp(4478.100000001255 s since 1904-01-01), "dt"=0.15, "Y"=[0.0, 0.0], "attributes"=variant("NI_ChannelName"=variant(string "APD 2"))}, {"t0"=timestamp(4478.100000001255 s since 1904-01-01), "dt"=0.15, "Y"=[0.03832069939271974, 0.03825193921460892], "attributes"=variant("NI_ChannelName"=variant(string "T1 Y"))}, {"t0"=timestamp(4478.100000001255 s since 1904-01-01), "dt"=0.15, "Y"=[-0.04115430382333141, -0.04098539428791512], "attributes"=variant("NI_ChannelName"=variant(string "T1 X"))}, {"t0"=timestamp(4478.100000001255 s since 1904-01-01), "dt"=0.15, "Y"=[8.223135319071018, 8.222352671895505], "attributes"=variant("NI_ChannelName"=variant(string "T1 Sum"))}, {"t0"=timestamp(4478.100000001255 s since 1904-01-01), "dt"=0.15, "Y"=[0.049969565217666184, 0.05022434551426698], "attributes"=variant("NI_ChannelName"=variant(string "T2 Y"))}, {"t0"=timestamp(4478.100000001255 s since 1904-01-01), "dt"=0.15, "Y"=[-0.04609831905596902, -0.04591761419661594], "attributes"=variant("NI_ChannelName"=variant(string "T2 X"))}, {"t0"=timestamp(4478.100000001255 s since 1904-01-01), "dt"=0.15, "Y"=[8.16038734092227, 8.159965300454726], "attributes"=variant("NI_ChannelName"=variant(string "T2 Sum"))}, {"t0"=timestamp(4478.100000001255 s since 1904-01-01), "dt"=0.15, "Y"=[0.008344782840181541, 0.008352712723844287], "attributes"=variant("NI_ChannelName"=variant(string "T1 FB X"))}, {"t0"=timestamp(4478.100000001255 s since 1904-01-01), "dt"=0.15, "Y"=[8.999798211615344, 8.999808099612414], "attributes"=variant("NI_ChannelName"=variant(string "T1 FB Sum"))}, {"t0"=timestamp(4478.100000001255 s since 1904-01-01), "dt"=0.15, "Y"=[0.01562539899484444, 0.015629296930858246], "attributes"=variant("NI_ChannelName"=variant(string "T2 FB X"))}, {"t0"=timestamp(4478.100000001255 s since 1904-01-01), "dt"=0.15, "Y"=[8.999790185247353, 8.999797753837703], "attributes"=variant("NI_ChannelName"=variant(string "T2 FB Sum"))}, {"t0"=timestamp(4478.100000001255 s since 1904-01-01), "dt"=0.15, "Y"=[-4.908334489551589, -4.898547275139339], "attributes"=variant("NI_ChannelName"=variant(string "PSD Y"))}, {"t0"=timestamp(4478.100000001255 s since 1904-01-01), "dt"=0.15, "Y"=[-0.42967373813057286, -0.42906247102062434], "attributes"=variant("NI_ChannelName"=variant(string "PSD X"))}, {"t0"=timestamp(4478.100000001255 s since 1904-01-01), "dt"=0.15, "Y"=[-0.019742362743003634, -0.019780571916867582], "attributes"=variant("NI_ChannelName"=variant(string "PSD Y Sum"))}]
  in  "Signals to Plot":i32(listbox)
  out "Trap Disp. Freq. (Hz)":dbl=6.666666666666667 caption="Freq. (Hz)" format="%#_6p"
  out "Display Period (s)":dbl=0.15 caption="Period (s)" format="%#_6p"
  in  "Trap Disp. Downsample":dbl=10000.0 caption="Downsample" max=20000.0
  in  "APD Disp. Scale":dbl=0.1 caption="Scale (Divide,\nfor above plot only)"
  in  "APD Disp. Downsample":dbl=15.0 caption="Integrate" min=1.0 max=30.0 step=1.0
  out "APD Display Freq. (Hz)":dbl=6.666666666666667 caption="Freq. (Hz)"
  out "APD Display Period (s)":dbl=0.15 caption="Period (s)"
  out "FFT 1":cluster{"f0":dbl, "df":dbl, "magnitude":dbl[]}[](graph)=[{"f0"=0.0, "df"=3.3333333333333335, "magnitude"=array[10000 elements]}, {"f0"=0.0, "df"=3.3333333333333335, "magnitude"=array[10000 elements]}]
  out "FFT 2":cluster{"f0":dbl, "df":dbl, "magnitude":dbl[]}[](graph)=[{"f0"=0.0, "df"=3.3333333333333335, "magnitude"=array[10000 elements]}, {"f0"=0.0, "df"=3.3333333333333335, "magnitude"=array[10000 elements]}]
  in  "FFT 1 Choice 1":u16(ring) items=["T1 Y", "T1 X", "T1 Sum", "T2 Y", "T2 X", "T2 Sum", "T1 FB X", "T1 FB Sum", "T2 FB X", "T2 FB Sum", "PSD Y", "PSD X", "PSD Y Sum", "none"]
  in  "FFT 2 Choice 1":u16(ring)=3 items=["T1 Y", "T1 X", "T1 Sum", "T2 Y", "T2 X", "T2 Sum", "T1 FB X", "T1 FB Sum", "T2 FB X", "T2 FB Sum", "PSD Y", "PSD X", "PSD Y Sum", "none"]
  in  "FFT 1 Choice 2":u16(ring)=1 items=["T1 Y", "T1 X", "T1 Sum", "T2 Y", "T2 X", "T2 Sum", "T1 FB X", "T1 FB Sum", "T2 FB X", "T2 FB Sum", "PSD Y", "PSD X", "PSD Y Sum", "none"]
  in  "FFT 2 Choice 2":u16(ring)=4 items=["T1 Y", "T1 X", "T1 Sum", "T2 Y", "T2 X", "T2 Sum", "T1 FB X", "T1 FB Sum", "T2 FB X", "T2 FB Sum", "PSD Y", "PSD X", "PSD Y Sum", "none"]
  in  "Compute FFT":bool=TRUE
  in  "Reset FFT":bool
  in  "# Spectra to Ave.":dbl=25.0
  out "Ave. Time (s)":dbl=7.5
  out "1 Channel":waveform(dbl)(graph)={"t0"=timestamp(0 s since 1904-01-01), "dt"=1.4999999999999999e-05, "Y"=array[20000 elements], "attributes"=variant("NI_ChannelName"=variant(string "T1 Y"))}
  out "Slow mean":dbl=0.04741485510254009 format="%0.2f"
  in  "Slow mean N ave.":dbl=1.0 min=1.0 step=1.0
  out "Mean Intensity":dbl=0.04741485510254009
  out "Sigma":dbl=0.006116447585273888
  out "Sigma/Mean":dbl=0.12899855060289364
  in  "Subtract mean":bool
  in  "High Res. Display":u16(ring) items=["T1 Y", "T1 X", "T1 Sum", "T2 Y", "T2 X", "T2 Sum", "T1 FB X", "T1 FB Sum", "T2 FB X", "T2 FB Sum", "PSD Y", "PSD X", "PSD Y Sum"]
  out "APD 1 Rate (Hz)":dbl format="%#_3p"
  in  "Tab Control":T4(tab)
  out "Stage Moving":bool
  in  "Read Cal":bool
  in  "Confocal Linescan":bool
  in  "Speed (nm/s)":dbl=100.0
  in  "Furthest Withdraw (MHz)":dbl=15.0
  in  "Confocal Image":bool
  in  "Round T1 X":bool caption="Round"
  in  "T1 offset_x (mV)":dbl=-45.0347243000155 format="%#_2g"
  in  "T1 kappa_x (pN/nm)":dbl=0.2471971927099238 min=0.0 step=0.001 format="%#_2g"
  out "Time (s)":dbl=279.9
  out "Total Time (s)":dbl=60.0
  in  "Start Saving":bool
  in  "Cal sets to save":u32=50 min=1 step=1
  in  "Comment (data description)":string="testing confocal setup"
  out "Calibrating Trap...":bool
  in  "Trap 2 (ON/OFF)":bool=TRUE
  in  "Trap 1 (ON/OFF)":bool=TRUE
  in  "Save Calibration":bool
  in  "N sets to save":u32=200 caption="N Sets"
  in  "Save N Sets":bool
  out "Save file name":path=path "E:/Data/101028/101028_052.dat"
  in  "Save ave N":dbl=500.0 caption="Averaging Factor"
  out "Saving...":bool
  in  "Stop Saving":bool
  out "Progress":u16(slide) scale=0.0..100.0
  out "Manipulating Trap":bool
  out "Buffer Status":dbl(slide) scale=0.0..1.0
  out "Overflow (data lost)":bool
  in  "Reset":bool
  out "Data Rate (Hz)":dbl=66666.66666666667 caption="Trap Data Rate (Hz)" format="%#_3p"
  out "Data Period (s)":dbl=1.4999999999999999e-05 caption="Trap Data Period (s)" format="%#_6p"
  out "Save Data Rate (Hz)":dbl=133.33333333333334 caption="Rate (Hz)" format="%#_6p"
  out "Save Data Period (s)":dbl=0.0075 caption="Period (s)" format="%#_6p"
  in  "T1 alpha_x (nm/V)":dbl=682.2856484824291 step=10.0 format="%#_3g"
  in  "T2 alpha_x (nm/V)":dbl=790.1873608955543 step=10.0 format="%#_3g"
  in  "T2 kappa_x (pN/nm)":dbl=0.2174132196053945 min=0.0 step=0.001 format="%#_2g"
  in  "T2 offset_x (mV)":dbl=-45.767376265464655 format="%#_2g"
  in  "BD 1 Frequency 1 (MHz)":dbl=70.0 caption="T1 X (MHz)" min=60.0 max=90.0 step=1.0 format="%#_6p"
  in  "BD 1 Frequency 2 (MHz)":dbl=85.0 caption="T2 X (MHz)" min=60.0 max=90.0 step=1.0 format="%#_6p"
  in  "Green Laser ON/Interlacing":bool
  in  "Round T2 X":bool caption="Round"
  in  "AO1":dbl(slide)=6.408063513378007 caption="Confocal Y (V)" min=0.0 max=10.0 step=0.01 scale=0.0..10.0 scale format="%_1f"
  in  "AO2":dbl(slide)=2.4332770775475328 caption="Confocal X (V)" min=0.0 max=10.0 step=0.01 scale=0.0..10.0 scale format="%_1f"
  in  "Trap Raster Scan":bool
  out "Raster Scanning...":bool
  in  "Trap Delta (MHz)":dbl=15.0
  in  "Setpoints (V)":cluster{"Set 1":dbl, "Set 2":dbl}={"Set 1"=9.0, "Set 2"=9.0}
  in  "Index":dbl=52.0 caption="Save File Index" min=1.0 step=1.0
  in  "Position Label 5":string="upper flow spot (UvrD)" caption="5"
  in  "Move to Position":bool
  in  "Position":dbl=1.0 min=1.0 max=10.0 step=1.0
  in  "Set Position":bool
  in  "Saved Stage Positions":dbl[][](array[numeric])=[[1.0, 2.24438, -0.22402, 0.00732], [2.0, 0.0, 0.0, 0.0], [3.0, 2.75063, -0.30498, 0.00732], [4.0, 2.75063, 0.39507, 0.00732], [5.0, 2.75063, -2.32612, 0.00732], [6.0, 0.0, 0.0, 0.0], [7.0, 0.0, 0.0, 0.0], [8.0, 0.0, 0.0, 0.0], [9.0, 0.0, 0.0, 0.0], [10.0, 0.0, 0.0, 0.0]]
  in  "Move to Position 5":bool
  in  "z nudge increment (um)":dbl=0.5
  in  "+z":bool
  in  "Position 1 Label":string="Right capillary (DNA beads)" caption="1"
  in  "Set Position 1":bool
  in  "Set Position 2":bool
  in  "Set Position 3":bool
  in  "Set Position 4":bool
  in  "Move to Position 3":bool
  in  "Move to Position 4":bool
  in  "Move to Position 2":bool
  in  "Move to Position 1":bool
  in  "Position 2 Label":string="Left capillary (ADig beads)" caption="2"
  in  "Position 3 Label":string="lower flow spot (ATP)" caption="3"
  in  "Position 4 Label":string="Dump beads" caption="4"
  in  "-z":bool
  in  "Set Position 5":bool
  out "Stage Control Serial Error":errorcluster={"status"=FALSE, "code"=1073676293, "source"="VISA Read in Set Stage Position.vi->UHR-Fleezers Control (host) - 10.2.vi"}
  out "Pump 3 cont disp":string="Left: ADig beads"
  out "Pump 1 cont disp":string="Right: DNA beads "
  in  "Ch 1 Inject Rate (ul/h)":dbl=50.0
  in  "Pump write delay (ms)":dbl=300.0
  in  "All Pump Parameters":T5={"Pump 1"={"Diameter (mm)"=4.61, "Units"=4.0, "Volume"=100.0, "Rate"=50.0}, "Pump 2"={"Diameter (mm)"=4.61, "Units"=3.0, "Volume"=0.0, "Rate"=0.0}, "Pump 3"={"Diameter (mm)"=4.61, "Units"=4.0, "Volume"=100.0, "Rate"=250.0}}
  in  "Ch 2 Inject Volume (uL)":dbl=100.0
  in  "Pump pause delay (ms)":u32
  in  "Ch 3 Inject Volume (uL)":dbl=100.0
  in  "Ch 3 Inject Rate (ul/h)":dbl=250.0
  in  "Flush Center Ch Volume (uL)":dbl=15.0
  in  "Flush Center Ch Rate (ul/m)":dbl=100.0
  in  "Inject Pump 2":bool caption="Inject Pump 2\n(Flush Center)"
  in  "Total Volume\nFlushed (uL)":dbl
  in  "Tab Control 2":T6(tab)=enum."AOD Raster Scan"
  out "Total Counts (ticks)":u32=600
  in  "Trap ON/OFF X or Y Amp?":bool=TRUE
  in  "Oscillate Set 1":bool
  in  "Trap 1 ON":bool=TRUE
  in  "Number Interlace Sets":u8=3 min=1 max=3
  in  "DIO count 3 (ticks)":u32=200
  in  "DIO count 2 (ticks)":u32=200
  in  "DIO count 1 (ticks)":u32=200
  in  "BD 2 Amplitude 3 (%)":dbl min=0.0 max=50.0 step=1.0
  in  "BD 2 Amplitude 2 (%)":dbl min=0.0 max=50.0 step=1.0
  in  "BD 2 Amplitude 1 (%)":dbl min=0.0 max=50.0 step=1.0
  in  "BD 1 Amplitude 3 (%)":dbl min=0.0 max=50.0 step=1.0
  in  "BD 1 Amplitude 2 (%)":dbl=35.0 min=0.0 max=50.0 step=1.0
  in  "BD 1 Amplitude 1 (%)":dbl=10.0 min=0.0 max=50.0 step=1.0
  in  "BD 2 Frequency 3 (MHz)":dbl=26.0 min=0.0 max=40.0 step=1.0 format="%#_6p"
  in  "BD 1 Frequency 3 (MHz)":dbl=70.0 min=60.0 max=90.0 step=1.0 format="%#_6p"
  in  "BD 2 Frequency 2 (MHz)":dbl=26.0 min=0.0 max=40.0 step=1.0 format="%#_6p"
  in  "BD 2 Frequency 1 (MHz)":dbl=26.0 min=0.0 max=40.0 step=1.0 format="%#_6p"
  in  "Not-Interlacing Set":enum32{"Set 1", "Set 2", "Set 3"}(radio)
  in  "Interlace":bool=TRUE
  in  "Trap 2 ON":bool=TRUE
  in  "Trap 3 ON":bool
  in  "Scan axis 2":bool=TRUE
  in  "Osc. freq. (Hz)":dbl=0.25
  in  "Osc. amp. (MHz)":dbl=2.0
  out "Coords":T7
  in  "Manipulation Scaling":cluster{"Horizontal":dbl, "Vertical":dbl}={"Horizontal"=0.075, "Vertical"=0.01}
  in  "Freq or Amp switch first":bool=TRUE
  in  "Swap F1 and F2":bool
  in  "Freq switch delay":u16
  in  "Amp switch delay":u16=5
  in  "MCL Step Increment (V_int)":dbl=3.0
  out "Time to Finish All (min)":dbl=0.66667 format="%#_2p"
  in  "Scan Speed (nm/s)":dbl=1.36
  in  "Scan Range (nm)":dbl=500.0
  in  "Step Size (nm)":dbl=1.0
  in  "MCL/AOM Scale Tweak":dbl=1.0
  in  "MCL Step Position Ratio":dbl=0.5
  in  "Move MCL Also?":bool=TRUE
  out "Final sep (nm)":dbl=1170.1999999999998
  out "Initial sep (nm)":dbl=1143.0
  out "Save index":dbl=52.0
  out "Final delta (MHz)":dbl=16.22113821138211
  out "Initial delta (MHz)":dbl=16.0
  out "Final freq. (MHz)":dbl=68.77886178861789
  out "Initial freq. (MHz)":dbl=69.0
  in  "Saved AOD Raster Scan Parameter Sets":T8(array[cluster])=[{"Scan Range AOD (nm) 2"=500.0, "Step Size AOD (nm) 2"=1.0, "Scan Speed AOD (nm/s) 2"=100.0, "Number of scans (AOD) 2"=1, "Label"="offset curve"}, {"Scan Range AOD (nm) 2"=420.0, "Step Size AOD (nm) 2"=1.0, "Scan Speed AOD (nm/s) 2"=100.0, "Number of scans (AOD) 2"=1, "Label"="hp raster check"}, {"Scan Range AOD (nm) 2"=6.8, "Step Size AOD (nm) 2"=0.34, "Scan Speed AOD (nm/s) 2"=0.34, "Number of scans (AOD) 2"=1, "Label"="3.4 kbp - 1 bp steps"}]
  in  "Load parameters":bool
  out "Scan Range (MHz)":dbl=-0.22113821138211381
  in  "Restart DMA? (AOD)":bool=TRUE caption="Restart DMA?"
  out "Incr. int (AOD)":i64=-10553126509
  out "Time/Scan (s) (AOD)":dbl=20.0001 format="%#_2p"
  out "Data points/scans":dbl=2666680.0
  out "Data points/scan (f/b)":dbl=2666680.0
  in  "Save scans":bool=TRUE
  out "AOD Scan I":u64=2 caption="Scan I"
  in  "Continuous AOD Scanning":bool caption="Continuous Scanning"
  in  "Abort AOD Scan":bool caption="Abort Scan"
  in  "Scan BD":bool=TRUE
  out "Cycles/step (AOD)":u64=66667 format="%.3p"
  in  "Number of F/B Scans (AOD)":u16=1 min=1
  out "Scan steps (AOD)":u64=20
  out "Scan Increment (MHz)":dbl=-0.01163885323063757
  out "AOD Scanning":bool caption="Scanning"
  in  "Start AOD Scan":bool caption="Start Scan"
  out "N sets should be saved":dbl=133.334
  out "Progress 2":u16(slide) caption="Progress" scale=0.0..100.0
  in  "Abort save 2":bool caption="Abort save"
  in  "Trap 1 Bead Size (nm)":dbl=860.0
  in  "Trap 2 Bead Size (nm)":dbl=790.0
  out "MCL Count":dbl=57626414.84707534
  in  "All FB On/Off":bool=TRUE
  in  "AI2 to Setpoint":cluster{"Set 1":bool, "Set 2":bool}
  out "AI2 (V)":cluster{"Set 1":dbl, "Set 2":dbl}={"Set 1"=8.970915860469376, "Set 2"=9.001129184850612}
  in  "Reset Feedback":cluster{"Set 1":bool, "Set 2":bool}
  in  "PID Gains":T9={"Set 1"={"proportional gain (Kc)"=0, "integral gain (Kc*Ts/Ti)"=5, "derivative gain (Kc*Td/Ts)"=0}, "Set 2"={"proportional gain (Kc)"=0, "integral gain (Kc*Ts/Ti)"=5, "derivative gain (Kc*Td/Ts)"=0}}
  in  "Feedback On/Off":cluster{"Set 1":bool, "Set 2":bool}={"Set 1"=TRUE, "Set 2"=TRUE}
  in  "Set SP to Reading":bool
  out "Trap X (AI1)":T10={"Trap 1"=-0.035400390625, "Trap 2"=-0.04693603515625}
  in  "Trap Pos FB SP":fxp<+/-,16,1>=-0.092803955078125 caption="Setpoint"
  in  "Trap Pos. FB ON":bool
  in  "Reset Trap Pos. FB":bool
  out "Trap Positions":waveform(dbl)[](graph)=[{"t0"=timestamp(4478.100000001255 s since 1904-01-01), "dt"=0.15, "Y"=[68.99999999999966, 68.99999999999966], "attributes"=variant("NI_ChannelName"=variant(string "Trap 1 Pos."))}, {"t0"=timestamp(4478.100000001255 s since 1904-01-01), "dt"=0.15, "Y"=[85.00000000000045, 85.00000000000045], "attributes"=variant("NI_ChannelName"=variant(string "Trap 2 Pos."))}]
  in  "Tab Control 8":enum32{"Main Setting", "Details"}(tab)
  in  "Trap Pos FB Int Count":u16=100
  in  "Trap Pos. FB Gains":T11={"proportional gain (Kc)"=10.0, "integral gain (Kc*Ts/Ti)"=10.0, "derivative gain (Kc*Td/Ts)"=0.0} {"proportional gain (Kc)" format="%.11g"; "integral gain (Kc*Ts/Ti)" format="%.11g"; "derivative gain (Kc*Td/Ts)" format="%.11g"}
  in  "Trap Pos. FB Offset Factor":i64
  in  "Trap Pos FB Negate Action":bool
  in  "Trap Pos. FB Mult Factor":i64=33554432
  in  "Trap Pos. AI1 X Pre-scale":u16
  in  "Trap Pos. FB Range":T12={"output high"=0.999969482421875, "output low"=-1.0}
  out "Trap Pos FB Int Signal":fxp<+/-,24,9>=-3.95257568359375 format="%.18g"
  out "Trap Pos FB Int-Norm Signal":fxp<+/-,16,1>=-0.039520263671875 format="%.16g"
  in  "Set SP Using...":bool
  in  "Trap Pos FB Monitor\nT1 or T2":bool
  out "Trap X AI1 (DMA)":T13={"Set 1"=-0.040985107421875, "Set 2"=-0.045928955078125}
  in  "N El. to Ave.":dbl=10000.0
  out "Trap Pos FB Action":i64=-32768
  out "Action (%)":dbl(knob)=-100.0030518509476 scale=-100.0..100.0
  in  "Trap Pos. FB Out Scale 2^n":u8=23 caption="Action Scale"
  out "Mean T1 Position (nm)":dbl caption="Mean T1 (nm)" format="%0.2f"
  out "Trap 1 Position RMS (A)":dbl caption="RMS (Ang)"
  in  "Tab Control 3":enum32{"Timing", "MCL Scan", "Analog Out"}(tab)
  out "APD 2 Gate Late Counter":u32
  out "APD 2 Gate Relative Phase":i16
  in  "Phase Adj. (APD 2 Gate)":i16=20
  in  "Initial Phase Adjustment (APD 2 Gate)":i16=55
  out "APD 1 Gate Late Counter":u32
  in  "- phase (APD 1 Gate)":bool
  in  "+ phase (APD 1 Gate)":bool
  out "APD 1 Gate Relative Phase":i16
  in  "Phase Adj. (APD 1 Gate)":i16=20
  in  "Initial Phase Adjustment (APD 1 Gate)":i16=60
  in  "Save APD Data\nwith Trap Data":bool=TRUE
  out "APD FIFO Elements Remaining":u32
  in  "- phase (APD Acq)":bool
  in  "+ phase (APD Acq)":bool
  out "APD Acq Late Counter":u32
  out "APD Acq Relative Phase":i16
  in  "Phase Adj. (APD Acq)":i16=20
  in  "Initial Phase Adjustment (APD Acq)":i16
  in  "Invert APD Gate":bool caption="Invert Gate"
  in  "APD Gate OFF Count":u32=450 caption="Gate OFF Count"
  in  "APD Gate ON Count":u32=150 caption="Gate ON Count"
  in  "APD Gate":enum32{"ON", "OFF", "Interlace"}(radio)=enum."Interlace"
  in  "APD Integration Time (s)":dbl=0.01 caption="Integration Time (s)"
  out "APD Acq Rate (Hz)":dbl=100.0 caption="Rate (Hz)"
  out "APD Samples/FIFO Acq.":dbl=30.0
  out "APD Elements/DMA read":u32=60
  out "APD Int. Count":u32=400000 format="%.0p"
  in  "+ phase (APD 2 Gate)":bool
  in  "- phase (APD 2 Gate)":bool
  in  "Tab Control 5":enum32{"PSD X", "PSD Y", "Other Data Channel"}(tab)
  out "Data map":dbl[][](graph)
  in  "Channel":i32=4
  in  "Abort MCL Scan":bool
  out "MCL Scan I":u64=2
  out "MCL Scanning":bool
  in  "Start MCL Scan":bool
  out "wait to reset values":bool
  in  "Tab Control 4":enum32{"Scan Settings", "MCL FPGA Loop Timing"}(tab)
  out "Total Time (s)":dbl=48.0
  in  "Scan lines (y)":u64=20
  in  "Fast Scan Dir":bool=TRUE
  in  "2D or 1D Scan":bool=TRUE
  out "Initial X":dbl
  out "Initial Y":dbl
  out "Time/f+b scan (s) (MCL)":dbl=2.4 caption="Time/scan (s)"
  in  "Number of scans (MCL)":u64=1 caption="Scans"
  in  "Scan steps (MCL)":u64=40 caption="Scan steps (x)"
  in  "N APD Samp/step":dbl=3.0
  in  "Scan Range (V)\n(of steps)":dbl=3.5
  in  "Restart DMA? (MCL)":bool=TRUE caption="Restart DMA?"
  in  "Continuous MCL Scanning":bool caption="Cont. Scanning"
  in  "Center Scan":bool=TRUE
  in  "Save Data (MCL)":bool=TRUE caption="Save Data"
  out "Actual Incr. int (MCL)":i16=294 caption="Incr. int"
  out "Desired incr (int)":dbl=294.0628205128205
  out "Desired Scan Incr (V)":dbl=0.08974358974358974
  out "N sets should be saved (MCL)":dbl=160.0 caption="N sets should be saved"
  out "Data points/scans (MCL)":dbl=4800.0 caption="Data points/scans"
  out "Data points/scan (f+b)":dbl=240.0 caption="points/scan (f+b)"
  out "Cycles/step (MCL)":u64=2000 caption="Cycles/step" format="%.0p"
  out "Actual MCL Inc (V)":dbl=0.08972441785943175
  in  "Phase adjust (MCL)":i16 caption="Phase adjust"
  out "Relative Phase (MCL)":i16 caption="Relative Phase"
  in  "Initial Phase Adj. (MCL)":i16 caption="Initial Phase Adj."
  in  "Update Count (MCL)":u32=600
  in  "+ phase (MCL)":bool
  in  "- phase (MCL)":bool
  out "MCL Late Counter":u32
  in  "APD 1 AO Mult.":i16=1 min=1
  in  "APD 2 AO Mult.":i16=1 min=1
  in  "Tab Control 7":enum32{"Green FB Signals", "Slow MCL Scan"}(tab)
  out "Green FB Plot":dbl(graph)=-0.012512588885158849
  out "MCL Scan 2":cluster{"Begin (V)":dbl, dbl, dbl[]}(graph)
  out "MCL Scan":cluster{"Begin (V)":dbl, dbl, dbl[]}(graph)
  in  "Green laser mode":enum32{"Laser ON", "Laser OFF", "Interlace"}(radio)=enum."Interlace"
  in  "GI Frequency, ON count":u32=150 min=1 step=1
  in  "Invert GI":bool
  out "GI Late Counter":u32
  in  "Phase adj. (GI)":i16=5
  out "GI relative phase":i16
  in  "+ phase (GI)":bool
  in  "Initial Phase Adjustment (GI)":i16=19
  in  "GI Frequency, OFF count":u32=450 min=1 step=1
  in  "- phase (GI)":bool
  out "Green FB Signals (V)":cluster{"Y":dbl, "X":dbl, "Sum":dbl}={"Y"=-799.1951219512196, "X"=-799.1951219512196, "Sum"=-0.012512588885158849}
  out "Relative phase (Green FB)":i16
  in  "+ phase (Green FB)":bool
  in  "- phase (Green FB)":bool
  in  "Green FB Count":u32=600
  in  "Phase adj. (Green FB)":i16=10
  in  "Initial Phase Adjustment (Green FB)":i16=50
  in  "Green FB On/Off":bool=TRUE
  in  "Current When FB OFF (%)":dbl=87.0 min=0.0 max=100.0 step=1.0
  in  "Green int current ON count adj":u32=150
  in  "Green FB Gains":T14={"proportional gain (Kc)"=10, "integral gain (Kc*Ts/Ti)"=5, "derivative gain (Kc*Td/Ts)"=0}
  in  "Green FB Setpoint (mV)":dbl=100.0
  in  "- phase (GI) 2":bool
  in  "Initial Phase Adjustment (GI) 2":i16=-100
  in  "+ phase (GI) 2":bool
  out "GI relative phase 2":i16
  in  "Phase adj. (GI) 2":i16=20
  out "GI Late Counter 2":u32
  in  "Trap Position FIFO Depth":u32=300000 format="%.0p"
  in  "# Samples/trap":u32=20000 format="%.0p"
  out "Trap AI Elements/DMA read":u32=320000 format="%.0p"
  out "Ave. Rate (Hz)":dbl=200000.0 format="%#_6p"
  out "FIFO El. Rem.":u32 format="%.0p"
  in  "Phase adj. (AI1)":i16=15
  out "Relative phase (AI1)":i16
  in  "+ phase (AI1)":bool
  in  "- phase (AI1)":bool
  out "Late Counter (AI1)":u32
  in  "Initial Phase Adjustment (AI1)":i16=220
  out "AI rate (Hz)":dbl=200000.0 format="%#_6p"
  in  "AI Count (ticks)":u32=200
  out "# Samples/channel":u32=40000 format="%.0p"
  in  "Trap AI FIFO Depth":u32=600000 format="%.0p"
  in  "Detector Type":string(combo)="IR-QPD + PSD + FB-QPD X position"
  in  "N Acq Sets (Traps + Fl.)":i16=3
  in  "Sets to FIFO (Traps)":T15={"Set 1"=TRUE, "Set 2"=TRUE, "Set 3"=FALSE}
  in  "FPGA Ave.":dbl=1.0 min=1.0 step=1.0
  out "Ave. Period (s)":dbl=5e-06 format="%#_6p"
  out "DMA Update Period (s)":dbl=0.3
  out "FPGA Averaging":bool
  out "Trap Sets":u32=2
  out "Counts/DMA":dbl=12000000.0 format="%#_6p"
  out "Trap Pos FIFO El Remaining":u32=450
  out "Trap Pos Elements/DMA read":u32=120000 format="%.0p"
  out "Trap AI FIFO Timeout":u16
  out "Trap Pos FIFO Timeout":u16
  in  "Video Capture Rate (Hz)":dbl=30.0
  in  "Video Index":dbl=1.0 min=1.0 step=1.0
  in  "New Video File":bool
  in  "Save Video":bool
  in  "Reset Averaging":bool
  in  "Averaging":bool
  in  "Save Image":bool
  in  "Image Index":dbl=1.0 min=1.0
  out "Path Out":path
  in  "Center Point":cluster{"X":i32, "Y":i32}={"X"=335, "Y"=271}
  in  "Zoom Factor":sgl=7.0
  out "Window Size":cluster{"Width":i32, "Height":i32}
  out "Window Position":cluster{"X Position":i32, "Y Position":i32}={"X Position"=40, "Y Position"=40}
  in  "Initial Window Size":cluster{"Width":i32, "Height":i32}={"Width"=884, "Height"=619}
  in  "Initial Window Position":cluster{"X Position":i32, "Y Position":i32}={"X Position"=796, "Y Position"=4}
  in  "Intensity Upper":dbl=88.0
  in  "Intensity Lower":dbl=66.0
  out "error out":errorcluster
  out "error out 2":errorcluster
  in  "Harvard Syringe Pump Serial Port":refnum<visa-resource-name>="ASRL5::INSTR"
  in  "Lost Tether Alarm Threshold (pN)":dbl=0.5
  in  "AOM X Cal (nm/MHz)":dbl=123.0
  in  "MCL X Cal (nm/V)":dbl=1070.0
  out "X RF Amplitude Limits (%)":T16={"Minimum"=0.0, "Maximum"=50.0, "Increment"=1.0}
  out "X RF Frequency Limits (MHz)":T16={"Minimum"=60.0, "Maximum"=90.0, "Increment"=1.0}
  out "Y RF Frequency Limits (MHz)":T16={"Minimum"=0.0, "Maximum"=40.0, "Increment"=1.0}
  out "Y RF Amplitude Limits (%)":T16={"Minimum"=0.0, "Maximum"=50.0, "Increment"=1.0}
  in  "Manip. X?":bool=TRUE
  in  "Manip. Y?":bool
  in  "Force Manip Abort":bool
  out "Read cal error":errorcluster
  in  "DAQ Delay (ms)":u32=1000
  in  "Start Scan":bool
  in  "Scan axis":bool=TRUE
  in  "Osc. amp. (V)":dbl=5.0
  in  "Osc. center (V)":dbl=5.0
  in  "Osc. freq. (Hz) 2":dbl=1.0
  in  "MCL Mode":u16(ring) items=["Manual Positioning", "Sinusoidal Wave", "Linear Scan"]
  in  "Begin (V)":dbl
  in  "End (V)":dbl=10.0
  in  "N Points":dbl=20.0
  in  "Delay to Interlace (s)":dbl
  in  "Delayed Interlace Start":bool
  in  "Read Lateness and Rel Phase":bool
  out "Vec Mean of T1 T2":dbl[](array[numeric])=[0.35566162543637286, 0.35438339782546413]
  in  "Cal read wait (s)":u32=5
  out "Time tether formed":timestamp=timestamp(3371146929.513132 s since 1904-01-01)
  in  "Sample Chamber Stage Serial Port":refnum<visa-resource-name>="ASRL4::INSTR"
  in  "Chemyx Syringe Pump Serial Port":refnum<visa-resource-name>="ASRL3::INSTR"
  in  "Limit Min (MHz)":dbl=10.0 caption="Min (MHz)"
  in  "Limit Max (MHz)":dbl=16.0 caption="Max (MHz)"
  in  "Limits Enable":bool=TRUE caption="Enable"
  out "AI labels":string[](array[string])=["T1 Y", "T1 X", "T1 Sum", "T2 Y", "T2 X", "T2 Sum", "T1 FB X", "T1 FB Sum", "T2 FB X", "T2 FB Sum", "PSD Y", "PSD X", "PSD Y Sum"]
  in  "Save Trap Pos. Data":bool=TRUE
  # "After"
  # "During"
  # "Trap On?"
  # "BD Flow ON?"
  # "Samp Flow ON?"
  # "1"
  # "2"
  # "Trap Display:"
  # "APD Display:"
  # "DAQ"
  # "Trap Manipulation"
  # "Data Saving"
  # "Bead Calibration"
  # "Harvard Pump\n(sample channel for flow exp)"
  # "Chemyx Pump 2"
  # "Units: \n1 = ml/m\n2 = ml/h\n3 = ul/m\n4 = ul/h"
  # "Rate param is ul/h\nVolume param is ul"
  # "X"
  # "Y"
  # "Oscillate Set 1 freq. (debugging)"
  # "BD 1"
  # "BD 2"
  # "AOD Raster Scan"
  # "Approx. trap separations"
  # "X"
  # "Y"
  # "FPGA\nreading"
  # "DMA\ntransfer"
  # "APD Gates"
  # "APD 2"
  # "APD 1"
  # "X"
  # "2D"
  # "Y"
  # "1D"
  # "Green Laser Interlacing"
  # "Green FB Measurement"
  # "Digital Gate"
  # "Current Analog Control"
  # "Total AI Rates (NOT rates/trap)"
  # "(Samples/trap x Trap Sets)"
  # "(Samples/channel x\n8 if averaging (8 channels)\n4 if no averaging)"
  # "Trap 1"
  # "Trap 2"
  # "Flour./Trap 3"
  # "External Video Window"
  # "MCL Position Debugging"
  # "Temporary Control Storage\n(these used to be somewhere else, still want to keep them)"
  # "Y"
  # "X"
  # "Trap Position Difference Limits"
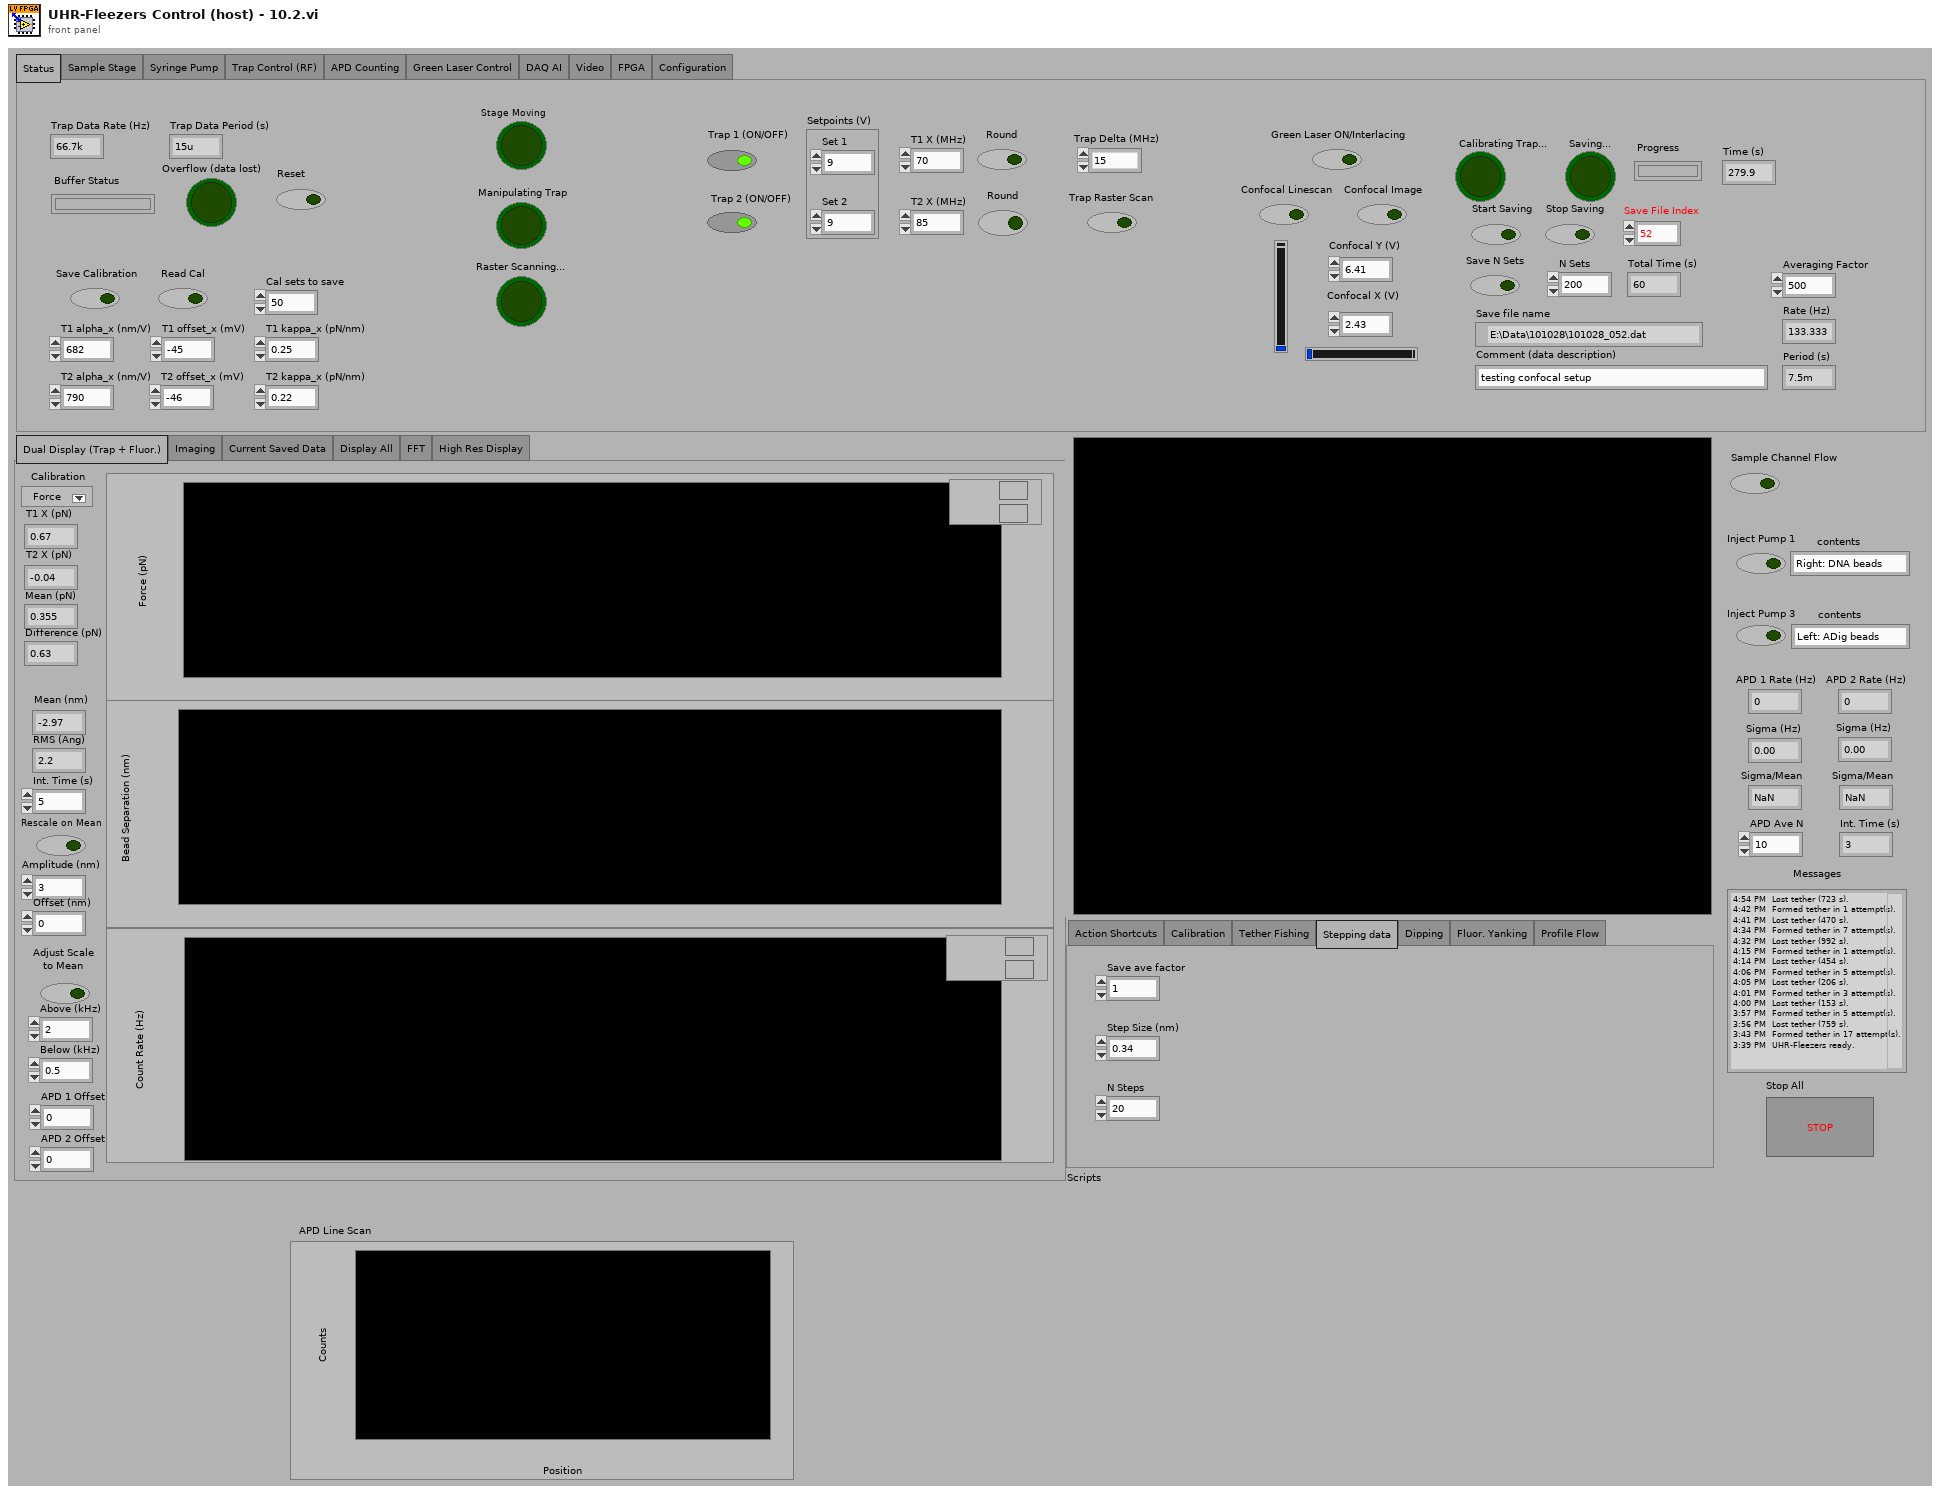
[diagram p1: front panel]
types:
  T1 = enum32{"Action Shortcuts", "Calibration", "Tether Fishing", "Stepping data", "Dipping", "Fluor. Yanking", "Profile Flow"}
  T2 = typedef "IMAQ Image.ctl" = refnum<image>
  T3 = enum32{"Dual Display (Trap + Fluor.)", "Imaging", "Current Saved Data", "Display All", "FFT", "High Res Display"}
  T4 = enum32{"Status", "Sample Stage", "Syringe Pump", "Trap Control (RF)", "APD Counting", "Green Laser Control", "DAQ AI", "Video", "FPGA", "Configuration"}
  T5 = cluster{"Pump 1":cluster{"Diameter (mm)":dbl, "Units":dbl, "Volume":dbl, "Rate":dbl}, "Pump 2":cluster{"Diameter (mm)":dbl, "Units":dbl, "Volume":dbl, "Rate":dbl}, "Pump 3":cluster{"Diameter (mm)":dbl, "Units":dbl, "Volume":dbl, "Rate":dbl}}
  T6 = enum32{"IR Laser Interlacing (Direct RF Board Control Method)", "AOD Raster Scan", "Feedback on Trap Intensity", "Feedback on Trap Position"}
  T7 = typedef "LVPoint32TypeDef.ctl" = cluster{"Horizontal":i32, "Vertical":i32}
  T8 = cluster{"Scan Range AOD (nm) 2":dbl, "Step Size AOD (nm) 2":dbl, "Scan Speed AOD (nm/s) 2":dbl, "Number of scans (AOD) 2":u16, "Label":string}[]
  T9 = cluster{"Set 1":cluster{"proportional gain (Kc)":i16, "integral gain (Kc*Ts/Ti)":i16, "derivative gain (Kc*Td/Ts)":i16}, "Set 2":cluster{"proportional gain (Kc)":i16, "integral gain (Kc*Ts/Ti)":i16, "derivative gain (Kc*Td/Ts)":i16}}
  T10 = cluster{"Trap 1":fxp<+/-,16,1>, "Trap 2":fxp<+/-,16,1>}
  T11 = cluster{"proportional gain (Kc)":fxp<+/-,16,8>, "integral gain (Kc*Ts/Ti)":fxp<+/-,16,8>, "derivative gain (Kc*Td/Ts)":fxp<+/-,16,8>}
  T12 = cluster{"output high":fxp<+/-,16,1>, "output low":fxp<+/-,16,1>}
  T13 = cluster{"Set 1":fxp<+/-,16,1>, "Set 2":fxp<+/-,16,1>}
  T14 = cluster{"proportional gain (Kc)":i16, "integral gain (Kc*Ts/Ti)":i16, "derivative gain (Kc*Td/Ts)":i16}
  T15 = cluster{"Set 1":bool, "Set 2":bool, "Set 3":bool}
  T16 = typedef "LVMinMaxIncTypeDef.ctl" = cluster{"Minimum":dbl, "Maximum":dbl, "Increment":dbl}
  T17 = typedef "Image Type" = u32
  T18 = typedef "nirio_resource_hc.ctl" = tag
  T19 = typedef "openfpgaref.8.6.ctl" = refnum<k20>
  T20 = typedef "niFpgaNodeNameForErrorReporting.ctl" = enum16{"Open FPGA VI Reference", "Read/Write Control", "Invoke Method: Abort", "Invoke Method: Acknowledge IRQ", "Invoke Method: Download", "Invoke Method: FIFO.Configure", "Invoke Method: FIFO.Read", "Invoke Method: FIFO.Start", "Invoke Method: FIFO.Stop", "Invoke Method: FIFO.Write", "Invoke Method: Reset", "Invoke Method: Run", "Invoke Method: Wait on IRQ", "Close FPGA VI Reference"}
  T21 = typedef "niLvFpgaWhatHappensToTopLevelVI.ctl" = enum16{"top level VI scripted behind XNode", "top level VI inlined behind XNode"}
  T22 = cluster{"New Image":T2, "New Image":T2, "New Image":T2, "New Image":T2}
  T23 = typedef "XDNodeRunTimeDep.lvlib/timing_clust.ctl" = cluster{"Expected End [f-1]":u64, "Actual End [f-1]":u64, "Finished Late? [f-1]":bool, "Expected End [i-1]":u64, "Actual End [i-1]":u64, "Finished Late? [i-1]":bool, "Expected Start [i]":u64, "Actual Start [i]":u64, "Expected Start [f]":u64, "Actual Start [f]":u64, "Source Name":string, "Structure Name":string, "Period":i64, "Deadline":i64, "Offset":i64, "Start":i64, "Priority":i32, "Timeout":i32, "Mode":T24, "Wakeup Reason":T25, "Error":errorcluster, "Source Type":string, "Secondary Source Type":string, "Global End Time":u64, "Global Start Time":u64, "Frame Duration":u64, "Iteration Duration":u64, "Assigned CPU":i32, "I/O Scan Engine Mode":u32}
  T24 = typedef "XDNodeRunTimeDep.lvlib/nitl_modes.ctl" = enum32{"No Change", "Process missed periods, maintain original phase", "Discard missed periods, maintain original phase", "Process missed periods, ignore original phase", "Discard missed periods, ignore original phase"}
  T25 = typedef "XDNodeRunTimeDep.lvlib/wakeup.ctl" = enum32{"Normal", "Aborted", "Asynchronous wakeup", "Timing source error", "Timed loop error", "Timeout"}
  T26 = enum32{"Normal Display", "Dual Display (APD)", "FFT", "High Res Display"}
  T27 = cluster{"Origin Pixel":cluster{"X":sgl, "Y":sgl}, "Angle Relative to Horizontal (deg)":sgl, "Axis Reference":u32}
  T28 = typedef "Simple Grid Descriptor" = cluster{"X Step":sgl, "Y Step":sgl, "Unit":T29}
  T29 = typedef "Image Unit" = enum32{"Undefined", "Angström", "Micrometer", "Millimeter", "Centimeter", "Meter", "Kilometer", "Microinch", "Inch", "Feet", "Nautical miles", "Standard miles", "Steps"}
  T30 = cluster{"averaging mode":u16, "weighting mode":u16, "number of averages":u32}
  T31 = cluster{"dB On (F)":bool, "unwrap phase (F)":bool, "convert to degree (F)":bool}
  T32 = enum16{"open", "replace", "create", "open or create", "replace or create", "replace or create with confirmation"}
  T33 = enum16{"big-endian, network order", "native, host order", "little-endian"}
  T34 = cluster{string, string, string, string, string, string, string, string}
  T35 = cluster{string, string, string, string, string, string, string, string, string, string, string, string}
  T36 = cluster{string, string, string, string, string, string, string, string, string, string, string, string, string}
  T37 = cluster{string, string, string, string, string, string, string, string, string, string, string, string, string, string}
  T38 = cluster{"BD 1 Frequency 1 (MHz)":dbl, "BD 1 Frequency 2 (MHz)":dbl}
  T39 = cluster{"f0":dbl, "df":dbl, "magnitude":dbl[]}[][]
  T40 = cluster{"Scan Range AOD (nm) 2":dbl, "Step Size AOD (nm) 2":dbl, "Scan Speed AOD (nm/s) 2":dbl, "Number of scans (AOD) 2":u16, "Label":string}
  T41 = cluster{"[0]":dbl, "[1]":dbl, "[2]":dbl, "[3]":dbl, "[4]":dbl, "[5]":dbl}
  T42 = cluster{"Diameter (mm)":dbl, "Units":dbl, "Volume":dbl, "Rate":dbl}
  T43 = cluster{"Left":i32, "Top":i32, "Width":u32, "Height":u32}
  T44 = cluster{cluster{"Left":i32, "Top":i32, "Width":u32, "Height":u32}}[]
  T45 = enum32{"setting", "request", "request control", "info", "statistics", "system settings", "I/O sub system", "HRT control", "camera descriptions", "device specific data", "event sub system settings", "event sub system results", "image memory manager"}
  T46 = typedef "AviRefnum.ctl" = refnum<k1>
  T47 = typedef "imagedata.ctl" = cluster{"image type":i32, "image depth":i32, "image":u8[], "mask":u8[], "colors":u32[], "Rectangle":cluster{"left":i16, "top":i16, "right":i16, "bottom":i16}}
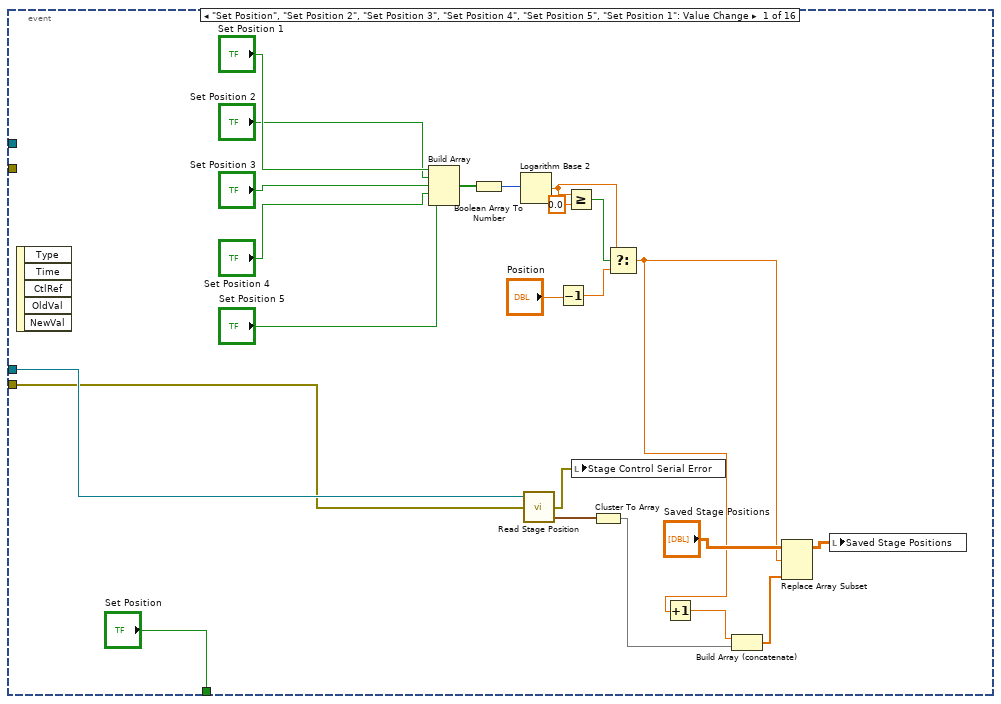
[diagram p2: hidden frame]
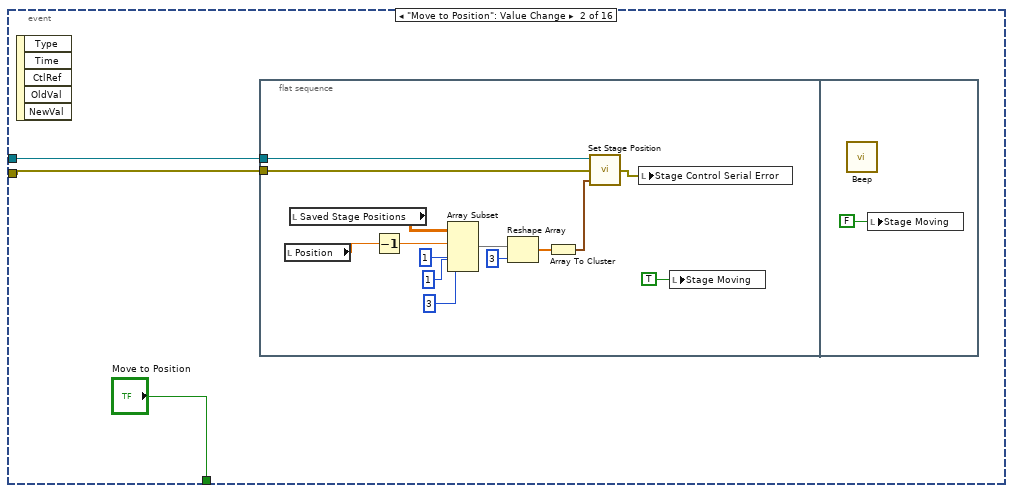
[diagram p3: hidden frame]
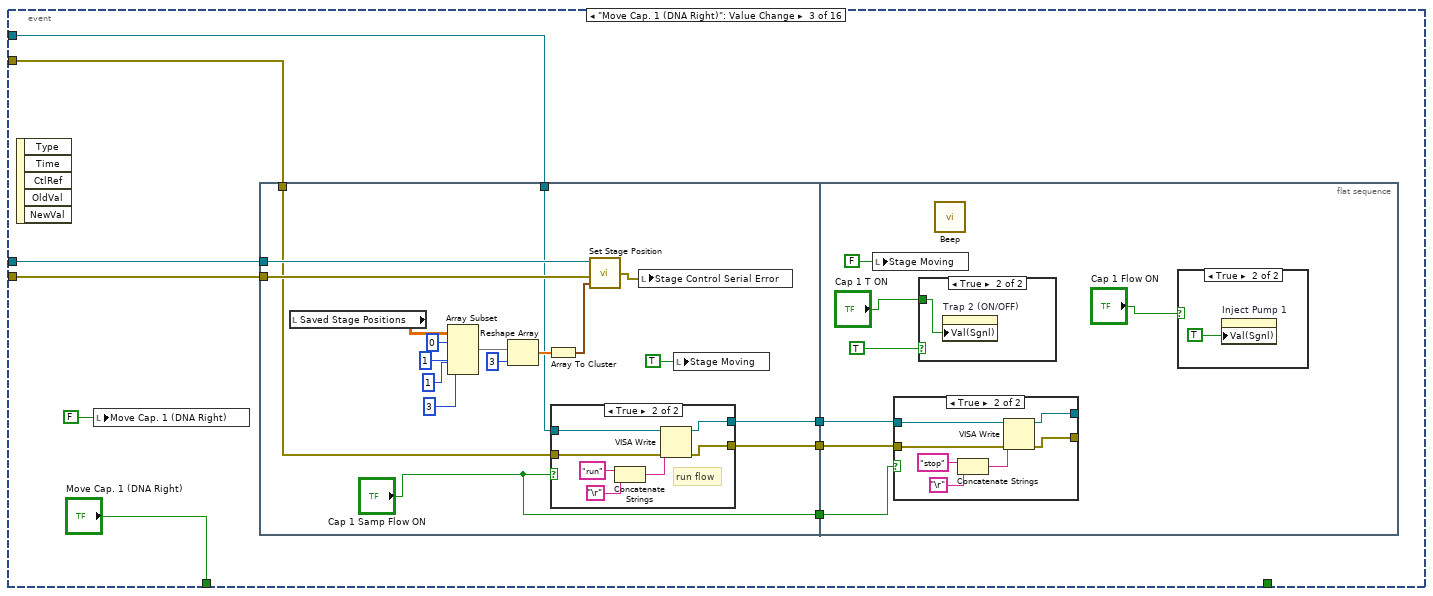
[diagram p4: hidden frame]
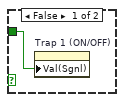
[diagram p8: hidden frame]
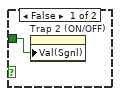
[diagram p12: hidden frame]
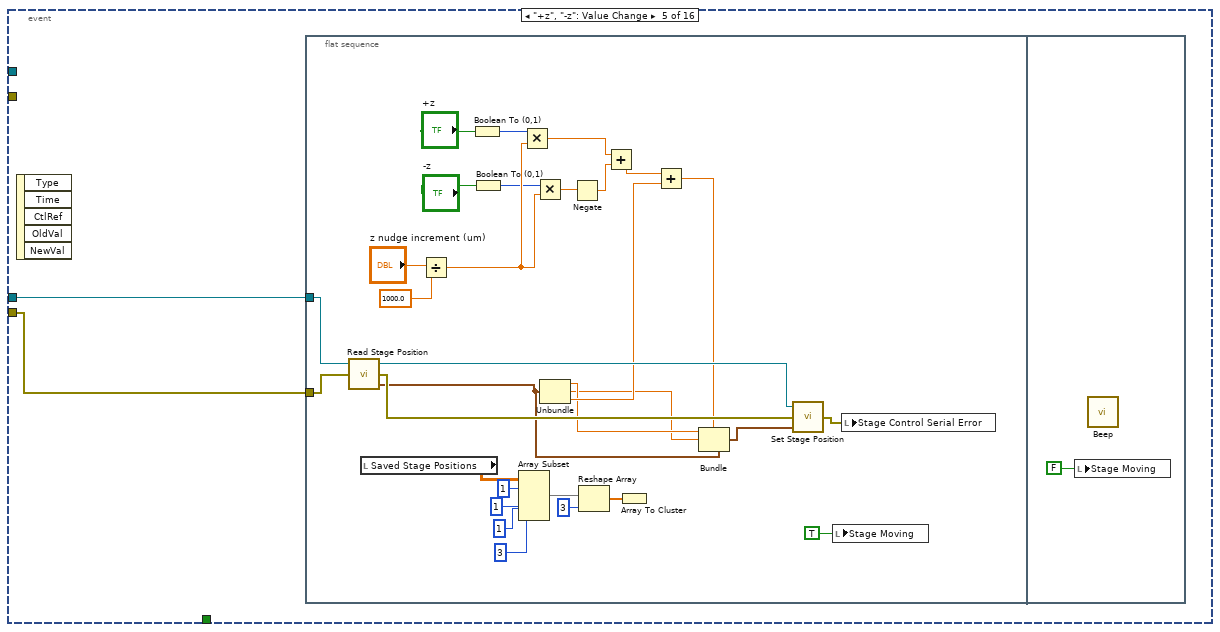
[diagram p13: hidden frame]
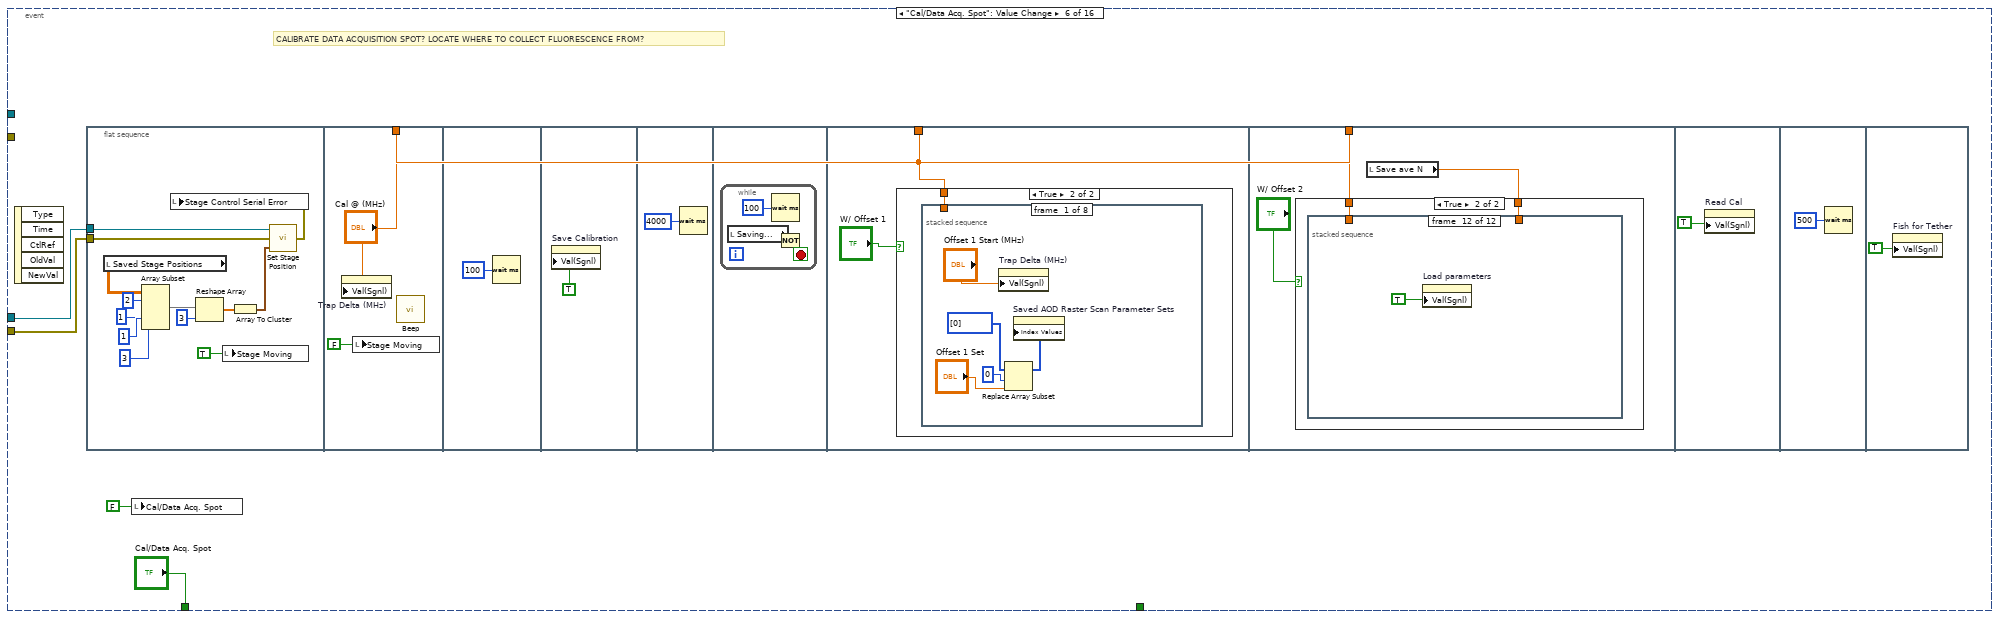
[diagram p14: hidden frame]
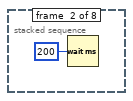
[diagram p16: hidden frame]
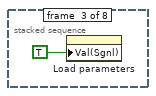
[diagram p17: hidden frame]
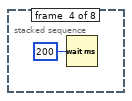
[diagram p18: hidden frame]
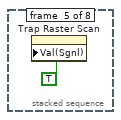
[diagram p19: hidden frame]
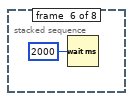
[diagram p20: hidden frame]
diagram:
  w25 = u16 20 items=["1.0"=10, "1.5"=15, "2.0"=20] ("stop bits (10: 1 bit)")
  w32 = T17 2 items=["Grayscale (U8)", "Grayscale (I16)", "Grayscale (SGL)", "Complex (CSG)", "RGB (U32)", "HSL (U32)", "RGB (U64)", "Grayscale (U16)"] ("Image Type")
  w100 = cluster{"output high":i16, "output low":i16} {"output high"=3000, "output low"=0} ("FB output range 1")
  w182 = 10.0 ("y")
  w181 = 32767.0 ("y")
  w197 = 6.0  # clock mult.
  w198 = 49152000.0  # TCXO frequ.
  n1 = Build Array("DIO count 1 (ticks)", "DIO count 2 (ticks)", "DIO count 3 (ticks)") -> (w87:u32[])
  n2 = Multiply(x="APD Integration Time (s)", y=40000000.0) -> (x*y=w107:dbl)
  n3 = Reciprocal(x="APD Integration Time (s)") -> (1/x=w104:dbl)
  n4 = local write "APD Acq Rate (Hz)"(w104) -> ()
  n5 = local read "AO1"() -> (w176:dbl)
  n6 = local read "AO2"() -> (w175:dbl)
  n7 = To Unsigned Long Integer(number=w107) -> (unsigned 32bit integer=w106:u32)
  "APD Int. Count" <- w106
  n8 = local read "Scan Increment (MHz)"() -> (w193:dbl)
  n9 = local read "Continuous MCL Scanning"() -> (w163:bool)
  n10 = local read "Fast Scan Dir"() -> (w162:bool)
  n11 = local read "Number of scans (MCL)"() -> (w164:u64)
  n12 = Multiply(x=w176, y=w181) -> (x*y=w178:dbl)
  n13 = Multiply(x=w175, y=w181) -> (x*y=w180:dbl)
  n14 = Divide(x=w178, y=w182) -> (x/y=w177:dbl)
  n15 = Divide(x=w180, y=w182) -> (x/y=w179:dbl)
  n16 = To Word Integer(number=w177) -> (16bit integer=w174:i16)
  n17 = To Word Integer(number=w179) -> (16bit integer=w173:i16)
  n18 = Not(x=w162) -> (.not. x?=w157:bool)
  n19 = local read "Cycles/step (MCL)"() -> (w165:u64)
  n20 = Multiply(x=w193, y=1000.0) -> (x*y=w200:dbl)
  n21 = local read "Scan steps (MCL)"() -> (w166:u64)
  n22 = local write "Trap Pos FIFO Timeout"(u16 0 ("Trap Pos FIFO Timeout")) -> ()
  n23 = local read "Desired Scan Incr (V)"() -> (w168:dbl)
  n24 = Scale By Power Of 2(n=48, x=w200) -> (x*2^n=w201:dbl)
  n25 = Multiply(x=w198, y=w197) -> (x*y=w196:dbl)
  n26 = Divide(x=w201, y=w196) -> (x/y=w195:dbl)
  n27 = local read "Setpoints (V)"() -> (w215:cluster{"Set 1":dbl, "Set 2":dbl})
  n28 = local read "Number Interlace Sets"() -> (w80:u8)
  n29 = Split 1D Array(array=w87, index=w80) -> (first subarray=w89:u32[])  [unwired: 1 out]
  n30 = Add Array Elements(numeric array=w89) -> (sum=w88:u32)
  n31 = property on="AI Count (ticks)" class="DigNum (strict)"("Val(Sgnl)"="AI Count (ticks)") -> ()  [unwired: 2 in, 2 out]
  n32 = local read "# Samples/channel"() -> (w185:u32)
  n33 = local read "Number of F/B Scans (AOD)"() -> (w186:u16)
  n34 = To Quad Integer(1:w195) -> (0:w192:i64)
  n35 = local read "Not-Interlacing Set"() -> (w79:enum32{"Set 1", "Set 2", "Set 3"})
  n36 = To Unsigned Byte Integer(number=w79) -> (unsigned 8bit integer=w85:u8)
  n37 = Index Array(array=w87, index=w85) -> (element=w86:u32)
  n38 = local read "Feedback On/Off"() -> (w218:cluster{"Set 1":bool, "Set 2":bool})
  n39 = local read "PID Gains"() -> (w210:T9)
  n40 = Divide(x=40000000.0, y="AI Count (ticks)") -> (x/y=w153:dbl)
  n41 = Multiply(x=w168, y=32767.0) -> (x*y=w170:dbl)
  n42 = local read "Scan steps (AOD)"() -> (w191:u64)
  n43 = local read "All FB On/Off"() -> (w219:bool)
  n44 = local read "Cycles/step (AOD)"() -> (w190:u64)
  n45 = local write "AI rate (Hz)"(w153) -> ()
  n46 = Divide(x=w170, y=10.0) -> (x/y=w169:dbl)
  n47 = Multiply(x=w191, y=w190) -> (x*y=w189:u64)
  n48 = Multiply(x=3276.7, y=w215) -> (x*y=w214:cluster{"Set 1":dbl, "Set 2":dbl})
  n49 = To Word Integer(number=w169) -> (16bit integer=w167:i16)
  n50 = Multiply(x=w189, y=u64 2) -> (x*y=w187:u64)
  n51 = local read "Sets to FIFO (Traps)"() -> (w222:T15)
  n52 = Divide(x=w153, y="FPGA Ave.") -> (x/y=w154:dbl)
  n53 = To Word Integer(number=w214) -> (16bit integer=w213:cluster{"Set 1":i16, "Set 2":i16})
  n54 = xnode "Open FPGA VI Reference"("resource name"=T18 "750kHzDAQ") -> ("FPGA VI Reference Out"=w207:T19, "error out"=w206:errorcluster)  [unwired: 1 in]
  n55 = Unbundle By Name(w210) -> ("Set 1"=w209:T14, "Set 2"=w208:T14)
  n56 = Multiply(x=w187, y=w186) -> (x*y=w184:u64)
  n57 = local write "Ave. Rate (Hz)"(w154) -> ()
  n58 = Divide(x=w184, y=w185) -> (x/y=w183:dbl)
  n59 = Unbundle By Name(w213) -> ("Set 1"=w212:i16, "Set 2"=w211:i16)
  n60 = local read "2D or 1D Scan"() -> (w101:bool)
  n61 = local write "Data points/scans"(w184) -> ()
  n62 = local read "Scan BD"() -> (w202:bool)
  n63 = And(x=w218, y=w219) -> (x .and. y?=w217:cluster{"Set 1":bool, "Set 2":bool})
  n64 = local write "Data points/scan (f/b)"(w187) -> ()
  n65 = Reciprocal(x=w154) -> (1/x=w155:dbl)
  n66 = local read "N Acq Sets (Traps + Fl.)"() -> (w146:i16)
  n67 = local write "N sets should be saved"(w183) -> ()
  n68 = Unbundle By Name(w217) -> ("Set 1"=w221:bool, "Set 2"=w220:bool)
  n69 = local read "Interlace"() -> (w81:bool)
  n70 = Select(t=w88, s=w81, f=w86) -> (s? t:f=w78:u32)
  n71 = local write "Update Count (MCL)"(w78) -> ()
  n72 = local write "Total Counts (ticks)"(w78) -> ()
  n73 = xnode "Invoke Method"("FPGA VI Reference In"=w207, "error in"=w206) -> ("FPGA VI Reference Out"=w99:T19, "error out"=w120:errorcluster)
  n74 = local write "Ave. Period (s)"(w155) -> ()
  n75 = property on="2D or 1D Scan" class="Bool (strict)"("Val(Sgnl)"=w101) -> ()  [unwired: 2 in, 2 out]
  n76 = xnode "Read/Write Control"("FPGA VI Reference In"=w98, "error in"=w120, "ai count"="AI Count (ticks)", "Interlace ON/OFF"=w81, "Number Interlace Cycles"=w80, "AI1 Sets to FIFO"=w222, "FB On/Off Set 1"=w221, "FB On/Off Set 2"=w220, "Interlace Off Parameters"=w79, "FB Setpoint Set 1"=w212, "FB Setpoint Set 2"=w211, "FB Gains Set 1"=w209, "FB Gains Set 2"=w208, "FB output range 1"=w100, "FB output range 2"=w100, "Cycles per step"=w190, "Scan BD"=w202, "Number of scans"=w186, "Scan steps"=w191, "Scan freq.  increment"=w192, "AO1"=w174, "AO2"=w173, "Scan freq.  increment (MCL)"=w167, "Scan steps (MCL)"=w166, "Cycles per step (MCL)"=w165, "Number of scans (MCL)"=w164, "MCL count"=w78, "Cont. Scan (MCL)"=w163, "MCL Scan Axis"=w157, "1D or 2D Scan?"=w101, "N of AI1 Int Acq Sets"=w146, "Freq or Amp switch first"="Freq or Amp switch first", "Freq switch delay"="Freq switch delay", "Amp switch delay"="Amp switch delay", "Swap F1 and F2"="Swap F1 and F2", "APD Acq Rate Count"=w106, "APD to FIFO"=FALSE, "APD Gate Operating Mode"="APD Gate", "APD Gate ON Count"="APD Gate ON Count", "APD Gate OFF Count"="APD Gate OFF Count", "Invert APD Gate"="Invert APD Gate", "DIO count 1 (ticks)"="DIO count 1 (ticks)", "DIO count 2 (ticks)"="DIO count 2 (ticks)", "DIO count 3 (ticks)"="DIO count 3 (ticks)", "APD 1 AO scale factor"="APD 1 AO Mult.", "APD 2 AO scale factor"="APD 2 AO Mult.") -> ("FPGA VI Reference Out"=w73:T19, "error out"=w75:errorcluster)  [unwired: 1 in]
  n77 = local read "Green Laser ON/Interlacing"() -> (w76:bool)
  n78 = local read "Green laser mode"() -> (w77:enum32{"Laser ON", "Laser OFF", "Interlace"})
  n79 = local read "GI Frequency, OFF count"() -> (w69:u32)
  n80 = local read "GI Frequency, ON count"() -> (w68:u32)
  n81 = Multiply(x="Current When FB OFF (%)", y=655.35) -> (x*y=w59:dbl)
  n82 = local read "Green FB Count"() -> (w67:u32)
  n83 = Multiply(x="Green FB Setpoint (mV)", y=3.2767) -> (x*y=w56:dbl)
  n84 = To Unsigned Word Integer(number=w59) -> (unsigned 16bit integer=w57:u16)
  n85 = local read "Invert GI"() -> (w71:bool)
  n86 = To Word Integer(number=w56) -> (16bit integer=w54:i16)
  n87 = case shown="False" w76 {
    tunnel: w77 -> [_ w248]
    tunnel: [enum32{"Laser ON", "Laser OFF", "Interlace"}."Laser OFF" ("Green laser mode") w248] -> w70
    frame False {
    }
    frame True {
    }
  }
  n88 = local read "Trap Pos. AI1 X Pre-scale"() -> (w11:u16)
  n89 = local read "Trap Pos FB Monitor\nT1 or T2"() -> (w18:bool)
  n90 = local read "Trap Pos FB Int Count"() -> (w4:u16)
  n91 = local read "Trap Pos FB Negate Action"() -> (w17:bool)
  n92 = local read "Trap Pos. FB Offset Factor"() -> (w16:i64)
  n93 = local read "Trap Pos. FB Mult Factor"() -> (w15:i64)
  n94 = local read "Trap Pos. FB Gains"() -> (w13:T11)
  n95 = local read "Trap Pos. FB Range"() -> (w14:T12)
  n96 = xnode "Read/Write Control"("FPGA VI Reference In"=w73, "error in"=w75, "Green interlace ON count 2"=w68, "Green interlace OFF count 2"=w69, "Invert GI 2"=w71, "Operating Mode 2"=w70, "Green FB Gains"="Green FB Gains", "Green FB Setpoint"=w54, "Green FB On/Off"="Green FB On/Off", "Current Out"=w57, "Green int current ON count adj"="Green int current ON count adj", "Green FB Count"=w67, "Operating Mode"=w70, "Green interlace OFF count"=w69, "Green interlace ON count"=w68, "Invert GI"=w71, "Trap Pos FB Monitor T1 or T2"=w18, "Trap Pos FB Negate Action"=w17, "Trap Pos. FB Offset Factor"=w16, "Trap Pos. FB Mult Factor"=w15, "Trap Pos. FB Range"=w14, "Trap Pos. FB Gains"=w13, "Force feedback"=FALSE, "AI1 X Scale"=w11, "Trap Pos to FIFO"=TRUE, "Trap Pos FB Int Count"=w4) -> ("FPGA VI Reference Out"=w72:T19, "error out"=w74:errorcluster)
  n97 = xnode "Invoke Method"("FPGA VI Reference In"=w72, "error in"=w74, "Depth"="Trap AI FIFO Depth") -> ("FPGA VI Reference Out"=w21:T19, "error out"=w20:errorcluster)
  n98 = xnode "Invoke Method"("FPGA VI Reference In"=w21, "error in"=w20, "Depth"="Trap Position FIFO Depth") -> ("FPGA VI Reference Out"=w6:T19, "error out"=w5:errorcluster)
  n99 = flat-sequence {
    tunnel: w99 -> [w253]
    tunnel: [w253] -> w98
    tunnel: [w252] -> w97
    tunnel: [w251] -> w96
    tunnel: [w249] -> w94
    tunnel: [w250] -> w95
    frame #0 {
      w250 = T16 {"Minimum"=0.0, "Maximum"=40.0, "Increment"=1.0} ("Min Max Inc")
      w249 = T16 {"Minimum"=0.0, "Maximum"=50.0, "Increment"=1.0} ("Data Entry Limits")
      w252 = T16 {"Minimum"=60.0, "Maximum"=90.0, "Increment"=1.0} ("Min Max Inc")
      w251 = T16 {"Minimum"=0.0, "Maximum"=50.0, "Increment"=1.0} ("Data Entry Limits")
      n100 = property on="BD 2 Frequency 1 (MHz)" class="DigNum (strict)"("Data Range"=w250) -> ()  [unwired: 2 in, 2 out]
      n101 = property on="BD 2 Frequency 3 (MHz)" class="DigNum (strict)"("Data Range"=w250) -> ()  [unwired: 2 in, 2 out]
      n102 = property on="BD 2 Frequency 2 (MHz)" class="DigNum (strict)"("Data Range"=w250) -> ()  [unwired: 2 in, 2 out]
      n103 = property on="BD 1 Frequency 1 (MHz)" class="DigNum (strict)"("Data Range"=w252) -> ()  [unwired: 2 in, 2 out]
      n104 = property on="BD 1 Frequency 2 (MHz)" class="DigNum (strict)"("Data Range"=w252) -> ()  [unwired: 2 in, 2 out]
      n105 = property on="BD 1 Frequency 3 (MHz)" class="DigNum (strict)"("Data Range"=w252) -> ()  [unwired: 2 in, 2 out]
      n106 = property on="BD 2 Amplitude 1 (%)" class="DigNum (strict)"("Data Range"=w249) -> ()  [unwired: 2 in, 2 out]
      n107 = property on="BD 2 Amplitude 2 (%)" class="DigNum (strict)"("Data Range"=w249) -> ()  [unwired: 2 in, 2 out]
      n108 = property on="BD 2 Amplitude 3 (%)" class="DigNum (strict)"("Data Range"=w249) -> ()  [unwired: 2 in, 2 out]
      n109 = property on="BD 1 Amplitude 3 (%)" class="DigNum (strict)"("Data Range"=w251) -> ()  [unwired: 2 in, 2 out]
      n110 = property on="BD 1 Amplitude 2 (%)" class="DigNum (strict)"("Data Range"=w251) -> ()  [unwired: 2 in, 2 out]
      n111 = property on="BD 1 Amplitude 1 (%)" class="DigNum (strict)"("Data Range"=w251) -> ()  [unwired: 2 in, 2 out]
      "X RF Frequency Limits (MHz)" <- w252
      "X RF Amplitude Limits (%)" <- w251
      "Y RF Amplitude Limits (%)" <- w249
      "Y RF Frequency Limits (MHz)" <- w250
    }
  }
  n112 = xnode "Invoke Method"("FPGA VI Reference In"=w6, "error in"=w5) -> ("FPGA VI Reference Out"=w119:T19, "error out"=w118:errorcluster)  [unwired: 1 out]
  n113 = flat-sequence "Initial FPGA Loop Relative Phase Adjustment" {
    tunnel: "Initial Phase Adjustment (AI1)" -> [w264]
    tunnel: "Initial Phase Adjustment (GI)" -> [w263]
    tunnel: w119 -> [w262]
    tunnel: w118 -> [w261]
    tunnel: "Initial Phase Adj. (MCL)" -> [w260]
    tunnel: [w265] -> w128
    tunnel: [w259] -> w124
    tunnel: "Initial Phase Adjustment (APD Acq)" -> [w258]
    tunnel: "Initial Phase Adjustment (APD 1 Gate)" -> [w257]
    tunnel: "Initial Phase Adjustment (Green FB)" -> [w256]
    tunnel: "Initial Phase Adjustment (GI) 2" -> [w255]
    tunnel: "Initial Phase Adjustment (APD 2 Gate)" -> [w254]
    tunnel: w128 -> [w323]
    tunnel: [w324] -> w125
    tunnel: w124 -> [w324]
    tunnel: [w323] -> w123
    tunnel: w125 -> [w327]
    tunnel: w123 -> [w326]
    tunnel: [w329] -> w122
    tunnel: [w328] -> w121
    tunnel: [w387] -> w126
    tunnel: [w388] -> w127
    tunnel: w122 -> [w388]
    tunnel: w121 -> [w387]
    frame #0 {
      n114 = xnode "Read/Write Control"("FPGA VI Reference In"=w262, "error in"=w261, "Phase count adjustment"=w264, "Phase count adjustment (GI)"=w263, "Phase count adjustment (MCL)"=w260, "Phase Count Adjustment (APD Acq)"=w258, "Phase count adjustment (APD 1 Gate)"=w257, "Phase count adjustment (APD 2 Gate)"=w254, "Phase count adjustment (Green FB)"=w256, "Phase count adjustment (GI) 2"=w255) -> ("FPGA VI Reference Out"=w259:T19, "error out"=w265:errorcluster)
    }
    frame #1 {
      n115 = Wait (ms)(milliseconds to wait=u32 100) -> ()  [unwired: 1 out]
    }
    frame #2 {
      w325 = TRUE
      n116 = xnode "Read/Write Control"("FPGA VI Reference In"=w327, "error in"=w326, "+ phase"=w325, "+ phase (GI)"=w325, "+ phase (MCL)"=w325, "+ phase (APD Acq)"=w325, "+ phase (APD 1 Gate)"=w325, "+ phase (APD 2 Gate)"=w325, "+ phase (Green FB)"=w325, "+ phase (GI) 2"=w325) -> ("FPGA VI Reference Out"=w328:T19, "error out"=w329:errorcluster)
    }
    frame #3 {
      n117 = Wait (ms)(milliseconds to wait=u32 100) -> ()  [unwired: 1 out]
    }
  }
  n118 = local read "Phase adj. (Green FB)"() -> (w90:i16)
  n119 = local read "Phase adj. (GI) 2"() -> (w60:i16)
  n120 = local read "Phase adjust (MCL)"() -> (w158:i16)
  n121 = local read "Phase adj. (AI1)"() -> (w160:i16)
  n122 = local read "Phase adj. (GI)"() -> (w159:i16)
  n123 = xnode "Read/Write Control"("FPGA VI Reference In"=w126, "error in"=w127, "Phase count adjustment"=w160, "Phase count adjustment (GI)"=w159, "Phase count adjustment (MCL)"=w158, "Phase Count Adjustment (APD Acq)"="Phase Adj. (APD Acq)", "Phase count adjustment (APD 1 Gate)"="Phase Adj. (APD 1 Gate)", "Phase count adjustment (APD 2 Gate)"="Phase Adj. (APD 2 Gate)", "Phase count adjustment (Green FB)"=w90, "Phase count adjustment (GI) 2"=w60) -> ("FPGA VI Reference Out"=w46:T19, "error out"=w135:errorcluster)
  n124 = call "Initialize RF boards - interlace 3.vi"("error in"=w135, "FPGA VI Reference In"=w46) -> ("error out"=w133:errorcluster, "FPGA VI Reference Out"=w134:T19)
  n125 = call "set RF board frequency - interlace.vi"("Board 2 Frequency Limits"=w95, "Board 1 Frequency Limits"=w97, "error in"=w133, "FPGA VI Reference In"=w134, "Board 2 Frequency 3 (MHz)"="BD 2 Frequency 3 (MHz)", "Board 1 Frequency 3 (MHz)"="BD 1 Frequency 3 (MHz)", "Board 2 Frequency 2 (MHz)"="BD 2 Frequency 2 (MHz)", "Board 2 Frequency 1 (MHz)"="BD 2 Frequency 1 (MHz)", "Board 1 Frequency 2 (MHz)"="BD 1 Frequency 2 (MHz)", "Board 1 Frequency 1  (MHz)"="BD 1 Frequency 1 (MHz)") -> ("error out"=w237:errorcluster, "FPGA VI Reference Out"=w238:T19)
  n126 = call "set RF board amplitude - interlace.vi"("Board 2 Amplitude Limits"=w94, "Board 1 Amplitude Limits"=w96, "error in"=w237, "FPGA VI Reference In"=w238, "Board 2 Amplitude 3 (%)"="BD 2 Amplitude 3 (%)", "Board 1 Amplitude 3 (%)"="BD 1 Amplitude 3 (%)", "Board 2 Amplitude 2 (%)"="BD 2 Amplitude 2 (%)", "Board 2 Amplitude 1 (%)"="BD 2 Amplitude 1 (%)", "Board 1 Amplitude 2 (%)"="BD 1 Amplitude 2 (%)", "Board 1 Amplitude 1 (%)"="BD 1 Amplitude 1 (%)") -> ("error out"=w225:errorcluster, "FPGA VI Reference Out"=w226:T19)
  n127 = flat-sequence {
    tunnel: w226 -> [w397]
    tunnel: w225 -> [w396]
    tunnel: [w395] -> w230
    tunnel: [w394] -> w229
    tunnel: [w422] -> w228
    tunnel: w230 -> [w422]
    tunnel: [w421] -> w227
    tunnel: w229 -> [w421]
    tunnel: w228 -> [w431]
    tunnel: w227 -> [w430]
    tunnel: [w429] -> w8
    tunnel: [w428] -> w7
    frame #0 {
      n128 = local read "Trap 1 (ON/OFF)"() -> (w389:bool)
      n129 = xnode "Read/Write Control"("FPGA VI Reference In"=w397, "error in"=w396, "Direct RF Box  Communication"=FALSE) -> ("FPGA VI Reference Out"=w395:T19, "error out"=w394:errorcluster)
      n130 = local write "Saving..."(FALSE ("Saving Data")) -> ()
      n131 = local write "Stop All"(FALSE ("Stop All")) -> ()
      n132 = local write "Index"(1.0 ("Index")) -> ()
      n133 = property on="Trap 1 ON" class="Bool (strict)"("Value"=w389) -> ()  [unwired: 2 in, 2 out]
      "Manipulating Trap" <- FALSE ("Manipulating Trap")
    }
    frame #1 {
      n134 = local read "Trap 2 (ON/OFF)"() -> (w420:bool)
      n135 = Wait (ms)(milliseconds to wait=u32 10) -> ()  [unwired: 1 out]
      n136 = property on="Trap 2 ON" class="Bool (strict)"("Val(Sgnl)"=w420) -> ()  [unwired: 2 in, 2 out]
    }
    frame #2 {
      n137 = local read "Scan Range (nm)"() -> (w424:dbl)
      n138 = xnode "Read/Write Control"("FPGA VI Reference In"=w431, "error in"=w430, "FPGA Controls  RF Box"=TRUE ("Direct RF Box  Communication")) -> ("FPGA VI Reference Out"=w429:T19, "error out"=w428:errorcluster)
      n139 = call "Update messages.vi"("Message to add"="UHR-Fleezers ready.", "Old message string"="") -> ("New message string"=w427:string)
      n140 = local write "Messages"(w427) -> ()
      n141 = property on="Scan Range (nm)" class="DigNum (strict)"("Val(Sgnl)"=w424) -> ()  [unwired: 2 in, 2 out]
    }
  }
  n142 = Subtract(x="BD 1 Frequency 1 (MHz)", y="BD 1 Frequency 2 (MHz)") -> (x-y=w145:dbl)
  n143 = Subtract(x="BD 2 Frequency 1 (MHz)", y="BD 2 Frequency 2 (MHz)") -> (x-y=w144:dbl)
  n144 = Square(x=w144) -> (x^2=w142:dbl)
  n145 = Square(x=w145) -> (x^2=w143:dbl)
  n146 = Add(x=w143, y=w142) -> (x+y=w141:dbl)
  n147 = Square Root(x=w141) -> (sqrt(x)=w140:dbl)
  n148 = local write "Trap Delta (MHz)"(w140) -> ()
  n149 = call-poly "VISA Configure Serial Port"("VISA resource name"="Sample Chamber Stage Serial Port") -> ("VISA resource name out"=w41:refnum<visa-resource-name>, "error out"=w42:errorcluster)  [unwired: 5 in, 8 out]
  "Stage Control Serial Error" <- w42
  n150 = call "IMAQ Create"("Image Name"="APD 1 Image", "Image Type"=w32) -> ("New Image"=w31:T2)  [unwired: 3 in, 1 out]
  n151 = call "IMAQ Create"("Image Name"="APD 2 Image", "Image Type"=w32) -> ("New Image"=w30:T2)  [unwired: 3 in, 1 out]
  n152 = call "IMAQ Create"("Image Name"="Det. X Image", "Image Type"=w32) -> ("New Image"=w29:T2)  [unwired: 3 in, 1 out]
  n153 = call "IMAQ Create"("Image Name"="Det. Y Image", "Image Type"=w32) -> ("New Image"=w28:T2)  [unwired: 3 in, 1 out]
  n154 = call-poly "VISA Configure Serial Port"("VISA resource name"="Harvard Syringe Pump Serial Port", "baud rate (9600)"=u32 115200, "stop bits (10: 1 bit)"=w25) -> ("VISA resource name out"=w22:refnum<visa-resource-name>, "error out"=w23:errorcluster)  [unwired: 4 in, 7 out]
  n155 = Bundle("New Image"=w31, "New Image"=w30, "New Image"=w29, "New Image"=w28) -> (w27:T22)  [unwired: 1 in]
  n156 = node-c288(i64 1 ("Period"), 1 ("Processor")) -> (w149:T23)  [unwired: 2 out]
  n157 = node-c288(2 ("Processor")) -> (w50:T23)  [unwired: 3 out]
  n158 = node-c288() -> (w37:T23)  [unwired: 4 in]
  n159 = node-c288() -> (w52:T23)  [unwired: 4 out]
  n160 = node-c288(3 ("Processor")) -> (w48:T23)  [unwired: 3 out]
  n161 = disable-structure shown="Disabled" {
    disable-tunnel: [w455 _] -> w205
    disable-tunnel: w8 -> [w454 _]
    frame Disabled {
      n162 = node-c288() -> (w457:T23)  [unwired: 4 out]
      n163 = timed-loop "Rough control of MCL mirror stage (debugging)" {
        tunnel: w454 -> [w460]
        tunnel: [w459] -> w455
        timing: w457 -> [_]
        timing-out: [_] -> w456
        stop <- w459 stop-if-true
        n164 = node-c288() -> ()  [unwired: 2 out]
        n165 = case shown="1" "MCL Mode" {
          tunnel: w460 -> [_ w463 w536]
          frame 0, Default {
          }
          frame 1 {
            n166 = node-c288() -> (w465:T23)  [unwired: 4 out]
            n167 = timed-loop "Oscillate MCL mirror" {
              timing: w465 -> [_]
              timing-out: [_] -> w464
              tunnel: w463 -> [w504]
              i -> [w503]
              stop <- w466 stop-if-true
              n168 = node-c288() -> (w502:i64)  [unwired: 1 out]
              n169 = Multiply(x="AO1", y=32767.0) -> (x*y=w498:dbl)
              n170 = Multiply(x="AO2", y=32767.0) -> (x*y=w493:dbl)
              n171 = Divide(x=w498, y=10.0) -> (x/y=w499:dbl)
              n172 = Divide(x=w493, y=10.0) -> (x/y=w494:dbl)
              n173 = To Word Integer(number=w499) -> (16bit integer=w491:i16)
              n174 = To Word Integer(number=w494) -> (16bit integer=w490:i16)
              n175 = Divide(x=w502, y=i64 1000) -> (x/y=w473:dbl)
              n176 = Multiply(x=w473, y=w503) -> (x*y=w484:dbl)
              n177 = Multiply(x="Osc. freq. (Hz) 2", y=6.283185307179586) -> (x*y=w485:dbl)
              n178 = Multiply(x=w485, y=w484) -> (x*y=w483:dbl)
              n179 = Sine(x=w483) -> (sin(x)=w482:dbl)
              n180 = Multiply(x=w482, y="Osc. amp. (V)") -> (x*y=w480:dbl)
              n181 = Add(x=w480, y="Osc. center (V)") -> (x+y=w478:dbl)
              n182 = Divide(x=w478, y=10.0) -> (x/y=w476:dbl)
              n183 = Multiply(x=w476, y=32767.0) -> (x*y=w471:dbl)
              n184 = Select(t=w471, s="Scan axis", f=w491) -> (s? t:f=w489:dbl)
              n185 = Select(t=w490, s="Scan axis", f=w471) -> (s? t:f=w488:dbl)
              n186 = local read "MCL Mode"() -> (w470:u16)
              n187 = Not Equal?(x=w470, y=u16 1) -> (x != y?=w467:bool)
              n188 = local read "Stop All"() -> (w468:bool)
              n189 = xnode "Read/Write Control"("FPGA VI Reference In"=w504, "AO1"=w489, "AO2"=w488) -> ()  [unwired: 1 in, 2 out]
              n190 = Compound Arithmetic op=OR(w468, w467) -> (w466:bool)
              n191 = node-c288() -> ()  [unwired: 2 out]
            }
            n192 = node-c288(w464) -> ()  [unwired: 1 out]
          }
          frame 2 {
            n193 = case shown="True" "Start Scan" {
              tunnel: w536 -> [_ w548]
              frame False {
              }
              frame True {
                n194 = Subtract(x="End (V)", y="Begin (V)") -> (x-y=w544:dbl)
                n195 = Decrement(x="N Points") -> (x-1=w543:dbl)
                n196 = Divide(x=w544, y=w543) -> (x/y=w541:dbl)
                n197 = for {
                  N: "N Points" -> [_]
                  tunnel: "Begin (V)" -> [w561]
                  tunnel: w548 -> [w553]
                  tunnel: [w552] -> w547 mode=indexing
                  tunnel: w541 -> [w551]
                  tunnel: [w549] -> w540 mode=indexing
                  i -> [w560]
                  n198 = Multiply(x=w551, y=w560) -> (x*y=w559:dbl)
                  n199 = Add(x=w561, y=w559) -> (x+y=w556:dbl)
                  n200 = local read "Scan axis"() -> (w550:bool)
                  n201 = local read "AO1"() -> (w558:dbl)
                  n202 = local read "AO2"() -> (w557:dbl)
                  n203 = Select(t=w556, s=w550, f=w558) -> (s? t:f=w555:dbl)
                  n204 = Select(t=w557, s=w550, f=w556) -> (s? t:f=w554:dbl)
                  n205 = flat-sequence {
                    tunnel: w555 -> [w565]
                    tunnel: w554 -> [w564]
                    tunnel: w553 -> [w562]
                    tunnel: [w601] -> w552
                    tunnel: [w600] -> w549
                    frame #0 {
                      w568 = 10.0 ("y")
                      w563 = 32767.0 ("y")
                      n206 = Multiply(x=w565, y=w563) -> (x*y=w571:dbl)
                      n207 = Multiply(x=w564, y=w563) -> (x*y=w569:dbl)
                      n208 = Divide(x=w571, y=w568) -> (x/y=w572:dbl)
                      n209 = Divide(x=w569, y=w568) -> (x/y=w570:dbl)
                      n210 = To Word Integer(number=w572) -> (16bit integer=w566:i16)
                      n211 = To Word Integer(number=w570) -> (16bit integer=w567:i16)
                      n212 = xnode "Read/Write Control"("FPGA VI Reference In"=w562, "AO1"=w566, "AO2"=w567) -> ()  [unwired: 1 in, 2 out]
                    }
                    frame #1 {
                      n213 = Wait (ms)(milliseconds to wait="DAQ Delay (ms)") -> ()  [unwired: 1 out]
                    }
                    frame #2 {
                      n214 = local read "Slow mean"() -> (w601:dbl)
                      n215 = local read "Sigma"() -> (w600:dbl)
                    }
                  }
                }
                n216 = Bundle("Begin (V)"="Begin (V)", w541, w547) -> (→"MCL Scan":cluster{"Begin (V)":dbl, dbl, dbl[]})  [unwired: 1 out]
                n217 = Bundle("Begin (V)"="Begin (V)", w541, w540) -> (→"MCL Scan 2":cluster{"Begin (V)":dbl, dbl, dbl[]})  [unwired: 1 out]
              }
            }
          }
        }
        n218 = local read "Stop All"() -> (w459:bool)
        n219 = node-c288() -> ()  [unwired: 2 out]
      }
      n220 = node-c288(w456) -> ()  [unwired: 1 out]
    }
    frame Enabled {
    }
  }
  n221 = timed-loop "Acquire Data" {
    tunnel: w8 -> [w855]
    tunnel: w7 -> [w854]
    tunnel: [w885] -> w245
    tunnel: [w879] -> w243
    timing: w149 -> [_]
    timing-out: [_] -> w148
    tunnel: w27 -> [w680]
    stop <- "Stop All" stop-if-true
    w665 = "NI_ChannelName" ("name")
    n222 = node-c288() -> ()  [unwired: 2 out]
    n223 = First Call?() -> (First Call?: T/F=w630:bool)
    n224 = Or(x="Reset", y=w630) -> (x .or. y?=w631:bool)
    n225 = case "Reset data stream" shown="True" w631 {
      tunnel: w855 -> [w2122 w2130]
      tunnel: w854 -> [w2121 w2129]
      tunnel: [w2122 w2124] -> w850
      tunnel: [w2121 w2123] -> w849
      frame False {
      }
      frame True {
        w2127 = TRUE ("AI to FIFO")
        n226 = local write "Overflow (data lost)"(FALSE ("Overflow (data lost)")) -> ()
        n227 = call "reset FPGA DMA.vi"("error in"=w2129, "FPGA VI Reference In"=w2130) -> ("error out"=w2125:errorcluster, "FPGA VI Reference Out"=w2126:T19)
        n228 = xnode "Read/Write Control"("FPGA VI Reference In"=w2126, "error in"=w2125, "AI to FIFO"=w2127, "APD to FIFO"=w2127) -> ("FPGA VI Reference Out"=w2124:T19, "error out"=w2123:errorcluster)
      }
    }
    n229 = Or(x="Start AOD Scan", y="Trap Raster Scan") -> (x .or. y?=w800:bool)
    n230 = case "Start AOM raster scan" shown="True" w800 {
      tunnel: w850 -> [w1768 w1778]
      tunnel: w849 -> [w1767 w1777]
      tunnel: [w1768 w1771] -> w848
      tunnel: [w1767 w1770] -> w847
      frame False {
      }
      frame True {
        n231 = case shown="True" "Restart DMA? (AOD)" {
          tunnel: [w1939 w1941] -> w1772
          tunnel: [w1938 w1940] -> w1773
          tunnel: w1778 -> [w1939 w1943]
          tunnel: w1777 -> [w1938 w1942]
          frame False {
          }
          frame True {
            n232 = local write "Overflow (data lost)"(FALSE ("Overflow (data lost)")) -> ()
            n233 = call "reset FPGA DMA.vi"("error in"=w1942, "FPGA VI Reference In"=w1943) -> ("error out"=w1940:errorcluster, "FPGA VI Reference Out"=w1941:T19)
          }
        }
        n234 = local write "Trap Raster Scan"(FALSE ("Trap Raster Scan")) -> ()
        n235 = case shown="True" "Move MCL Also?" {
          tunnel: w1773 -> [w1781 w1841]
          tunnel: w1772 -> [w1782 w1842]
          tunnel: [w1780 w1845] -> w1771
          tunnel: [w1779 w1844] -> w1770
          frame False {
            w1783 = TRUE ("AI to FIFO")
            n236 = xnode "Read/Write Control"("FPGA VI Reference In"=w1782, "error in"=w1781, "AI to FIFO"=w1783, "APD to FIFO"=w1783, "Start scan"=w1783) -> ("FPGA VI Reference Out"=w1780:T19, "error out"=w1779:errorcluster)
          }
          frame True {
            w1838 = FALSE ("1D or 2D Scan?")
            w1843 = TRUE ("AI to FIFO")
            # "Count for MCL loop"
            # "N total cycles"
            # "N steps"
            # "V_int"
            n237 = local read "Scan Range (nm)"() -> (w1820:dbl)
            n238 = local read "Number of F/B Scans (AOD)"() -> (w1837:u16)
            n239 = Sign(1:w1820) -> (0:w1819:dbl)
            n240 = Compound Arithmetic op=MULTIPLY(w1820, "MCL Step Position Ratio", "MCL/AOM Scale Tweak") -> (w1824:dbl)
            n241 = Negate(x=w1819) -> (-x=w1816:dbl)
            n242 = Multiply(x=w1816, y="MCL Step Increment (V_int)") -> (x*y=w1818:dbl)
            n243 = Divide(x=w1824, y="MCL X Cal (nm/V)") -> (x/y=w1830:dbl)
            n244 = Multiply(x=32767.0 ("y"), y=w1830) -> (x*y=w1836:dbl)
            n245 = local read "Total Counts (ticks)"() -> (w1821:u32)
            n246 = local read "Cycles/step (AOD)"() -> (w1832:u64)
            n247 = local read "Scan steps (AOD)"() -> (w1833:u64)
            n248 = Divide(x=w1836, y=10.0) -> (x/y=w1829:dbl)
            n249 = Divide(x=w1829, y="MCL Step Increment (V_int)") -> (x/y=w1827:dbl)
            n250 = Absolute Value(x=w1827) -> (abs(x)=w1815:dbl)
            n251 = Compound Arithmetic op=MULTIPLY(w1833, w1832, w1821) -> (w1828:u64)
            n252 = local write "wait to reset values"(w1843) -> ()
            n253 = local write "MCL Scanning"(w1843) -> ()
            n254 = Divide(x=w1828, y=w1815) -> (x/y=w1825:dbl)
            "MCL Count" <- w1825
            n255 = xnode "Read/Write Control"("FPGA VI Reference In"=w1842, "error in"=w1841, "Scan steps (MCL)"=w1815, "Number of scans (MCL)"=w1837, "Cycles per step (MCL)"=u64 1, "Scan freq.  increment (MCL)"=w1818, "1D or 2D Scan?"=w1838, "MCL Scan Axis"=w1838, "Cont. Scan (MCL)"=w1838, "MCL count"=w1825) -> ("FPGA VI Reference Out"=w1840:T19, "error out"=w1839:errorcluster)
            n256 = xnode "Read/Write Control"("FPGA VI Reference In"=w1840, "error in"=w1839, "AI to FIFO"=w1843, "APD to FIFO"=w1843, "Start scan"=w1843, "Start scan (MCL)"=w1843) -> ("FPGA VI Reference Out"=w1845:T19, "error out"=w1844:errorcluster)
          }
        }
        "Raster Scanning..." <- TRUE ("Scanning...")
      }
    }
    n257 = And(x="Save scans", y=w800) -> (x .and. y?=w846:bool)
    n258 = Compound Arithmetic op=OR("Start MCL Scan", "Confocal Image", "Confocal Linescan") -> (w798:bool)
    n259 = And(x="Save Data (MCL)", y=w798) -> (x .and. y?=w845:bool)
    n260 = case "Start MCL raster scan" shown="True" w798 {
      tunnel: w848 -> [w1283 w1298]
      tunnel: w847 -> [w1282 w1297]
      tunnel: [w1283 w1293] -> w678
      tunnel: [w1282 w1292] -> w677
      tunnel: [FALSE w1291] -> w831
      tunnel: "Start MCL Scan" -> [_ w1286]
      tunnel: "Confocal Image" -> [_ w1285]
      tunnel: "Confocal Linescan" -> [_ _]
      frame False {
      }
      frame True {
        w1291 = TRUE
        n261 = case shown="True" "Restart DMA? (MCL)" {
          tunnel: [w1415 w1417] -> w1296
          tunnel: [w1414 w1416] -> w1295
          tunnel: w1298 -> [w1415 w1420]
          tunnel: w1297 -> [w1414 w1419]
          frame False {
          }
          frame True {
            n262 = call "reset FPGA DMA.vi"("error in"=w1419, "FPGA VI Reference In"=w1420) -> ("error out"=w1416:errorcluster, "FPGA VI Reference Out"=w1417:T19)
            n263 = local write "Overflow (data lost)"(FALSE ("Overflow (data lost)")) -> ()
          }
        }
        n264 = case shown="False" w1286 {
          selector: w1286 -> [_ w1302]
          tunnel: w1285 -> [w1301 _]
          tunnel: [w1301 w1302] -> w1284
          frame False {
            n265 = property on="2D or 1D Scan" class="Bool (strict)"("Val(Sgnl)"=w1301) -> ()  [unwired: 2 in, 2 out]
            n266 = property on="Confocal Image" class="Bool (strict)"("Value"=FALSE ("Start Confocal Map")) -> ()  [unwired: 2 in, 2 out]
          }
          frame True {
          }
        }
        n267 = local write "MCL Scanning"(w1291) -> ()
        n268 = local read "AO1"() -> (w1288:dbl)
        n269 = local read "AO2"() -> (w1287:dbl)
        n270 = case shown="True" "Center Scan" {
          tunnel: w1296 -> [w1309 w1372]
          tunnel: w1295 -> [w1308 w1371]
          tunnel: [w1307 w1370] -> w1293
          tunnel: [w1306 w1369] -> w1292
          tunnel: [w1304 w1356] -> w1290
          tunnel: [w1303 w1355] -> w1289
          tunnel: w1288 -> [w1304 w1361]
          tunnel: w1287 -> [w1303 w1364]
          tunnel: w1284 -> [_ _]
          frame False {
            w1305 = TRUE ("AI to FIFO")
            n271 = xnode "Read/Write Control"("FPGA VI Reference In"=w1309, "error in"=w1308, "AI to FIFO"=w1305, "APD to FIFO"=w1305, "Start scan (MCL)"=w1305) -> ("FPGA VI Reference Out"=w1307:T19, "error out"=w1306:errorcluster)
          }
          frame True {
            w1368 = TRUE ("AI to FIFO")
            n272 = local read "Scan steps (MCL)"() -> (w1347:u64)
            n273 = local read "Scan lines (y)"() -> (w1343:u64)
            n274 = local read "Fast Scan Dir"() -> (w1354:bool)
            n275 = local read "Actual MCL Inc (V)"() -> (w1344:dbl)
            n276 = Decrement(x=w1343) -> (x-1=w1342:u64)
            n277 = Decrement(x=w1347) -> (x-1=w1346:u64)
            n278 = Multiply(x=w1344, y=w1342) -> (x*y=w1341:dbl)
            n279 = Divide(x=w1341, y=2.0) -> (x/y=w1351:dbl)
            n280 = Multiply(x=w1344, y=w1346) -> (x*y=w1345:dbl)
            n281 = Divide(x=w1345, y=2.0) -> (x/y=w1350:dbl)
            n282 = Select(t=w1350, s=w1354, f=w1351) -> (s? t:f=w1349:dbl)
            n283 = Select(t=w1351, s=w1354, f=w1350) -> (s? t:f=w1353:dbl)
            n284 = Subtract(x=w1361, y=w1353) -> (x-y=w1352:dbl)
            n285 = Subtract(x=w1364, y=w1349) -> (x-y=w1348:dbl)
            n286 = local read "2D or 1D Scan"() -> (w1366:bool)
            n287 = Not(x=w1354) -> (.not. x?=w1360:bool)
            n288 = Not(x=w1366) -> (.not. x?=w1362:bool)
            n289 = And(x=w1354, y=w1362) -> (x .and. y?=w1363:bool)
            n290 = And(x=w1362, y=w1360) -> (x .and. y?=w1365:bool)
            n291 = Select(t=w1364, s=w1365, f=w1348) -> (s? t:f=w1355:dbl)
            n292 = Select(t=w1361, s=w1363, f=w1352) -> (s? t:f=w1356:dbl)
            n293 = call "Volt to I16.vi"("Voltage In"=w1356) -> ("I16 Voltage Out"=w1359:i16)
            n294 = call "Volt to I16.vi"("Voltage In"=w1355) -> ("I16 Voltage Out"=w1358:i16)
            n295 = xnode "Read/Write Control"("FPGA VI Reference In"=w1372, "error in"=w1371, "AI to FIFO"=w1368, "APD to FIFO"=w1368, "Start scan (MCL)"=w1368, "AO1"=w1359, "AO2"=w1358) -> ("FPGA VI Reference Out"=w1370:T19, "error out"=w1369:errorcluster)
          }
        }
        "Initial Y" <- w1290
        "Initial X" <- w1289
        "wait to reset values" <- w1291
      }
    }
    n296 = local read "Trap Pos Elements/DMA read"() -> (w674:u32)
    n297 = local read "Trap AI Elements/DMA read"() -> (w759:u32)
    n298 = local read "APD Elements/DMA read"() -> (w719:u32)
    n299 = xnode "Get APD Data"("FPGA VI Reference In"=w678, "error in"=w677, "Number of Elements"=w719, "Timeout (ms)"=-1) -> ("Data"=w718:void[], "Elements Remaining"=→"APD FIFO Elements Remaining")  [unwired: 2 out]
    n300 = xnode "Invoke Method"("FPGA VI Reference In"=w678, "error in"=w677, "Number of Elements"=w674, "Timeout (ms)"=-1) -> ("Data"=w637:void[], "Elements Remaining"=→"Trap Pos FIFO El Remaining")  [unwired: 2 out]
    n301 = xnode "Get Trap Data"("FPGA VI Reference In"=w678, "error in"=w677, "Number of Elements"=w759, "Timeout (ms)"=-1 ("Timeout")) -> ("FPGA VI Reference Out"=w748:T19, "error out"=w747:errorcluster, "Data"=w638:void[], "Elements Remaining"=w894)
    "FIFO El. Rem." <- w894
    n302 = local read "Trap AI FIFO Depth"() -> (w896:u32)
    n303 = Subtract(x=w896, y=w759) -> (x-y=w895:u32)
    n304 = Decimate 1D Array(w637) -> (w634:void[], w636:void[], w635:void[])
    n305 = Divide(x=w894, y=w895) -> (x/y=w893:dbl)
    "Buffer Status" <- w893
    n306 = To Unsigned Long Integer(number=w634) -> (unsigned 32bit integer=w633:u32[])
    n307 = Join Numbers(hi=w636, lo=w635) -> ((hi.lo)=w632:u32)
    n308 = Equal?(x=w893, y=1.0) -> (x = y?=w891:bool)
    n309 = Join Numbers(hi=w633, lo=w632) -> ((hi.lo)=w626:u64[])
    n310 = call "IR AOM word to freq - vec.vi"("Frequency Word In (double vec)"=w626) -> ("Frequency Out"=w673:dbl[])
    n311 = case "Alert buffer overflow" shown="True" w891 {
      frame False {
      }
      frame True {
        n312 = call <vilib>:"Beep.vi"() -> ()  [unwired: 3 in, 9 out]
        "Overflow (data lost)" <- TRUE ("Overflow (data lost)")
      }
    }
    n313 = Decimate 1D Array(w673) -> (w672:dbl[], w671:dbl[])
    n314 = Build Array(w672, w671) -> (w670:dbl[][])
    n315 = local read "Trap Sets"() -> (w758:u32)
    n316 = case "Deinterlace trap data, average down PSD" shown="1, Default" w758 {
      tunnel: w638 -> [w1450 w1515]
      tunnel: [w1447 w1512] -> w751
      tunnel: [w1450 w1514] -> w629
      tunnel: "Detector Type" -> [w1449 w1510]
      tunnel: [w1448 w1513] -> w750
      tunnel: [w1446 w1511] -> w866
      frame 1, Default {
        n317 = Divide(x=w1450, y=3276.7) -> (x/y=w1451:dbl)
        n318 = Decimate 1D Array(w1451) -> (w1460:dbl[], w1459:dbl[], w1458:dbl[], w1457:dbl[], w1456:dbl[], w1455:dbl[], w1454:dbl[], w1453:dbl[])
        n319 = case shown="\"IR-QPD + PSD + FB-QPD position\"" w1449 {
          tunnel: w1460 -> [w1484 w1509]
          tunnel: w1459 -> [w1483 w1508]
          tunnel: w1458 -> [w1468 w1486]
          tunnel: w1457 -> [w1469 w1496]
          tunnel: w1456 -> [w1482 w1507]
          tunnel: w1455 -> [w1481 w1506]
          tunnel: w1454 -> [w1465 w1487]
          tunnel: w1453 -> [w1464 w1485]
          tunnel: [w1463 w1493] -> w1448
          tunnel: [w1462 w1492] -> w1447
          tunnel: [w1461 w1491] -> w1446
          frame "IR-QPD + PSD + FB-QPD", Default {
            w1461 = 0  # Channel pattern
            n320 = Divide(x=w1484, y=w1469) -> (x/y=w1471:dbl[])
            n321 = Divide(x=w1483, y=w1469) -> (x/y=w1470:dbl[])
            n322 = Divide(x=w1482, y=w1465) -> (x/y=w1467:dbl[])
            n323 = Divide(x=w1481, y=w1464) -> (x/y=w1466:dbl[])
            n324 = Build Array(w1471, w1470, w1469, w1468, w1467, w1466, w1465, w1464) -> (w1462:dbl[][])
            n325 = Bundle("T1 Y", "T1 X", "T1 Sum", "FB Sum", "PSD Y", "PSD X", "PSD Y Sum", "PSD X Sum") -> (w1480:T34)  [unwired: 1 out]
            n326 = Cluster To Array(cluster=w1480) -> (array=w1463:string[])
          }
          frame "IR-QPD + PSD + FB-QPD position" {
            w1491 = 3  # Channel pattern
            n327 = Negate(x=w1487) -> (-x=w1488:dbl[])
            n328 = Divide(x=w1509, y=w1496) -> (x/y=w1498:dbl[])
            n329 = Divide(x=w1508, y=w1496) -> (x/y=w1497:dbl[])
            n330 = Divide(x=w1507, y=w1487) -> (x/y=w1495:dbl[])
            n331 = Divide(x=w1506, y=w1488) -> (x/y=w1494:dbl[])
            n332 = Build Array(w1498, w1497, w1496, w1485, w1486, w1495, w1494, w1487) -> (w1492:dbl[][])
            n333 = Bundle("T1 Y", "T1 X", "T1 Sum", "FB X", "FB Sum", "PSD Y", "PSD X", "PSD Y Sum") -> (w1505:T34)  [unwired: 1 out]
            n334 = Cluster To Array(cluster=w1505) -> (array=w1493:string[])
          }
        }
      }
      frame 2 {
        n335 = case shown="\"IR-QPD + PSD + FB-QPD X position\"" w1510 {
          tunnel: w1515 -> [w1577 w1644 w1715]
          tunnel: [w1516 w1635 w1646] -> w1514
          tunnel: [w1543 w1626 w1693] -> w1513
          tunnel: [w1542 w1589 w1660] -> w1512
          tunnel: [w1536 w1624 w1691] -> w1511
          frame "IR-QPD + PSD + FB-QPD", Default {
            w1536 = 1  # Channel pattern
            # "time average x2 the 4th signal and the 4 psd signals (detection laser)"
            # "deinterlace 3 signals from qpd"
            n336 = Decimate 1D Array(w1577) -> (w1576:void[], w1575:void[], w1541:void[], w1574:void[], w1564:void[], w1562:void[], w1561:void[], w1559:void[])
            n337 = Decimate 1D Array(w1541) -> (w1540:void[], w1539:void[])
            n338 = Decimate 1D Array(w1576) -> (w1573:void[], w1545:void[])
            n339 = Decimate 1D Array(w1575) -> (w1572:void[], w1570:void[])
            n340 = Decimate 1D Array(w1574) -> (w1571:void[], w1569:void[])
            n341 = call "downsample 1D array - double.vi"("Ave N"=2.0, "Array In"=w1564) -> ("Array Out"=w1563:dbl[])  [unwired: 1 out]
            n342 = call "downsample 1D array - double.vi"("Ave N"=2.0, "Array In"=w1562) -> ("Array Out"=w1544:dbl[])  [unwired: 1 out]
            n343 = call "downsample 1D array - double.vi"("Ave N"=2.0, "Array In"=w1561) -> ("Array Out"=w1560:dbl[])  [unwired: 1 out]
            n344 = call "downsample 1D array - double.vi"("Ave N"=2.0, "Array In"=w1559) -> ("Array Out"=w1558:dbl[])  [unwired: 1 out]
            n345 = Interleave 1D Arrays(w1573, w1572, w1571, w1545, w1570, w1569, w1540, w1539, w1563, w1544, w1560, w1558) -> (w1557:dbl[])
            n346 = Divide(x=w1557, y=3276.7) -> (x/y=w1556:dbl[])
            n347 = Decimate 1D Array(w1556) -> (w1555:dbl[], w1554:dbl[], w1553:dbl[], w1552:dbl[], w1551:dbl[], w1550:dbl[], w1538:dbl[], w1537:dbl[], w1549:dbl[], w1548:dbl[], w1547:dbl[], w1546:dbl[])
            n348 = Divide(x=w1555, y=w1553) -> (x/y=w1523:dbl[])
            n349 = Divide(x=w1554, y=w1553) -> (x/y=w1522:dbl[])
            n350 = Divide(x=w1552, y=w1550) -> (x/y=w1521:dbl[])
            n351 = Divide(x=w1551, y=w1550) -> (x/y=w1520:dbl[])
            n352 = Divide(x=w1549, y=w1547) -> (x/y=w1519:dbl[])
            n353 = Divide(x=w1548, y=w1546) -> (x/y=w1518:dbl[])
            n354 = Build Array(w1523, w1522, w1553, w1521, w1520, w1550, w1538, w1537, w1519, w1518, w1547, w1546) -> (w1542:dbl[][])
            n355 = Bundle("T1 Y", "T1 X", "T1 Sum", "T2 Y", "T2 X", "T2 Sum", "T1 FB Sum", "T2 FB Sum", "PSD Y", "PSD X", "PSD Y Sum", "PSD X Sum") -> (w1524:T35)  [unwired: 1 out]
            n356 = To Word Integer(number=w1557) -> (16bit integer=w1516:i16[])
            n357 = Cluster To Array(cluster=w1524) -> (array=w1543:string[])
          }
          frame "IR-QPD + PSD + FB-QPD X position" {
            w1624 = 2  # Channel pattern
            # "time average x2 the 3 psd signals (detection laser)"
            # "deinterlace 3 signals from qpds"
            n358 = Decimate 1D Array(w1644) -> (w1643:void[], w1642:void[], w1625:void[], w1641:void[], w1587:void[], w1584:void[], w1581:void[], w1612:void[])
            n359 = Decimate 1D Array(w1625) -> (w1610:void[], w1608:void[])
            n360 = Decimate 1D Array(w1643) -> (w1640:void[], w1627:void[])
            n361 = Decimate 1D Array(w1642) -> (w1639:void[], w1637:void[])
            n362 = Decimate 1D Array(w1641) -> (w1638:void[], w1636:void[])
            n363 = Decimate 1D Array(w1612) -> (w1611:void[], w1609:void[])
            n364 = call "downsample 1D array - I16.vi"("Ave N"=2.0, "Array In"=w1587) -> ("Array Out"=w1585:i16[])  [unwired: 1 in]
            n365 = call "downsample 1D array - I16.vi"("Ave N"=2.0, "Array In"=w1581) -> ("Array Out"=w1579:i16[])  [unwired: 1 in]
            n366 = call "downsample 1D array - I16.vi"("Ave N"=2.0, "Array In"=w1584) -> ("Array Out"=w1582:i16[])  [unwired: 1 in]
            n367 = Interleave 1D Arrays(w1640, w1639, w1638, w1627, w1637, w1636, w1611, w1610, w1609, w1608, w1585, w1582, w1579) -> (w1635:i16[])
            n368 = Divide(x=w1635, y=3276.7) -> (x/y=w1634:dbl[])
            n369 = Decimate 1D Array(w1634) -> (w1633:dbl[], w1632:dbl[], w1631:dbl[], w1630:dbl[], w1629:dbl[], w1628:dbl[], w1600:dbl[], w1598:dbl[], w1597:dbl[], w1595:dbl[], w1594:dbl[], w1593:dbl[], w1590:dbl[])
            n370 = Negate(x=w1590) -> (-x=w1588:dbl[])
            n371 = Divide(x=w1594, y=w1590) -> (x/y=w1592:dbl[])
            n372 = Divide(x=w1593, y=w1588) -> (x/y=w1591:dbl[])
            n373 = Divide(x=w1633, y=w1631) -> (x/y=w1616:dbl[])
            n374 = Divide(x=w1632, y=w1631) -> (x/y=w1615:dbl[])
            n375 = Divide(x=w1630, y=w1628) -> (x/y=w1614:dbl[])
            n376 = Divide(x=w1629, y=w1628) -> (x/y=w1613:dbl[])
            n377 = Divide(x=w1600, y=w1598) -> (x/y=w1599:dbl[])
            n378 = Divide(x=w1597, y=w1595) -> (x/y=w1596:dbl[])
            n379 = Build Array(w1616, w1615, w1631, w1614, w1613, w1628, w1599, w1598, w1596, w1595, w1592, w1591, w1590) -> (w1589:dbl[][])
            n380 = Bundle("T1 Y", "T1 X", "T1 Sum", "T2 Y", "T2 X", "T2 Sum", "T1 FB X", "T1 FB Sum", "T2 FB X", "T2 FB Sum", "PSD Y", "PSD X", "PSD Y Sum") -> (w1617:T36)  [unwired: 1 out]
            n381 = Cluster To Array(cluster=w1617) -> (array=w1626:string[])
          }
          frame "IR-QPD + PSD + FB-QPD XY positions" {
            w1691 = 4  # Channel pattern
            # "time average x2 the 3 psd signals (detection laser)"
            # "deinterlace 3 signals from qpds"
            n382 = Decimate 1D Array(w1715) -> (w1714:void[], w1713:void[], w1692:void[], w1712:void[], w1658:void[], w1704:void[], w1703:void[], w1680:void[])
            n383 = Decimate 1D Array "Feedback Sum"(w1692) -> (w1676:void[], w1674:void[])
            n384 = Decimate 1D Array "QPD Y"(w1714) -> (w1711:void[], w1694:void[])
            n385 = Decimate 1D Array "QPD X"(w1713) -> (w1710:void[], w1708:void[])
            n386 = Decimate 1D Array "Feedback Y"(w1658) -> (w1657:void[], w1656:void[])
            n387 = Decimate 1D Array "QPD Sum"(w1712) -> (w1709:void[], w1707:void[])
            n388 = Decimate 1D Array "Feedback X"(w1680) -> (w1677:void[], w1675:void[])
            n389 = call "downsample 1D array - double.vi"("Ave N"=2.0, "Array In"=w1704) -> ("Array Out"=w1679:dbl[])  [unwired: 1 out]
            n390 = call "downsample 1D array - double.vi"("Ave N"=2.0, "Array In"=w1703) -> ("Array Out"=w1678:dbl[])  [unwired: 1 out]
            n391 = Interleave 1D Arrays(w1711, w1710, w1709, w1694, w1708, w1707, w1657, w1677, w1676, w1656, w1675, w1674, w1679, w1678) -> (w1702:dbl[])
            n392 = Divide(x=w1702, y=3276.7) -> (x/y=w1701:dbl[])
            n393 = Decimate 1D Array(w1701) -> (w1700:dbl[], w1699:dbl[], w1698:dbl[], w1697:dbl[], w1696:dbl[], w1695:dbl[], w1653:dbl[], w1667:dbl[], w1651:dbl[], w1652:dbl[], w1665:dbl[], w1649:dbl[], w1663:dbl[], w1661:dbl[])
            n394 = Negate(x=w1661) -> (-x=w1659:dbl[])
            n395 = Divide(x=w1663, y=w1659) -> (x/y=w1662:dbl[])
            n396 = Divide(x=w1652, y=w1649) -> (x/y=w1648:dbl[])
            n397 = Divide(x=w1653, y=w1651) -> (x/y=w1650:dbl[])
            n398 = Divide(x=w1700, y=w1698) -> (x/y=w1684:dbl[])
            n399 = Divide(x=w1699, y=w1698) -> (x/y=w1683:dbl[])
            n400 = Divide(x=w1697, y=w1695) -> (x/y=w1682:dbl[])
            n401 = Divide(x=w1696, y=w1695) -> (x/y=w1681:dbl[])
            n402 = Divide(x=w1667, y=w1651) -> (x/y=w1666:dbl[])
            n403 = Divide(x=w1665, y=w1649) -> (x/y=w1664:dbl[])
            n404 = Build Array(w1684, w1683, w1698, w1682, w1681, w1695, w1650, w1666, w1651, w1648, w1664, w1649, w1662, w1661) -> (w1660:dbl[][])
            n405 = Bundle("T1 Y", "T1 X", "T1 Sum", "T2 Y", "T2 X", "T2 Sum", "T1 FB Y", "T1 FB X", "T1 FB Sum", "T2 FB Y", "T2 FB X", "T2 FB Sum", "PSD X", "PSD Y Sum") -> (w1647:T37)  [unwired: 1 out]
            n406 = To Word Integer(number=w1702) -> (16bit integer=w1646:i16[])
            n407 = Cluster To Array(cluster=w1647) -> (array=w1693:string[])
          }
        }
      }
    }
    "AI labels" <- w750
    n408 = Decimate 1D Array(w718) -> (w746:void[], w682:void[])
    n409 = local read "DMA Update Period (s)"() -> (w760:dbl)
    n410 = local read "BD 1 Frequency 2 (MHz)"() -> (w621:dbl)
    n411 = local read "BD 1 Frequency 1 (MHz)"() -> (w622:dbl)
    n412 = Build Array(w746, w682) -> (w828:void[])
    n413 = local read "Data Period (s)"() -> (w731:dbl)
    n414 = Decimate 1D Array(w629) -> (w653:i16[], w652:i16[], w650:i16[], w649:i16[])  [unwired: 9 out]
    n415 = To Double Precision Float(number=w828) -> (double precision float=w829:dbl[])
    n416 = local read "APD Integration Time (s)"() -> (w695:dbl)
    n417 = Divide(x=w653, y=w652) -> (x/y=w654:dbl[])
    n418 = Divide(x=w650, y=w649) -> (x/y=w651:dbl[])
    n419 = feedback #1(0.0) -> (w667:dbl)
    n420 = Add(x=w760, y=w667) -> (x+y=w868:dbl)
    n421 = feedback-in #1(w868) -> ()
    n422 = local read "AOM X Cal (nm/MHz)"() -> (w619:dbl)
    n423 = To Time Stamp(1:w667) -> (0:w666:timestamp)
    n424 = Split 1D Array(array=w654, index="N El. to Ave.") -> (second subarray=w657:dbl[])  [unwired: 1 out]
    n425 = Split 1D Array(array=w651, index="N El. to Ave.") -> (second subarray=w656:dbl[])  [unwired: 1 out]
    n426 = local read "Trap X AI1 (DMA)"() -> (w655:T13)
    n427 = Multiply(x=w731, y="Trap Disp. Downsample") -> (x*y=w668:dbl)
    "Display Period (s)" <- w668
    n428 = Bundle("BD 1 Frequency 1 (MHz)"=w622, "BD 1 Frequency 2 (MHz)"=w621) -> (w623:T38)  [unwired: 1 out]
    n429 = for "Trap AI" {
      tunnel: [w1445] -> w862 mode=indexing
      tunnel: w666 -> [w1435]
      tunnel: "Trap Disp. Downsample" -> [w1443]
      tunnel: w751 -> [w1441] mode=indexing
      tunnel: w731 -> [w1440]
      tunnel: w750 -> [w1439] mode=indexing
      tunnel: w665 -> [w1438]
      tunnel: [w1437] -> w706 mode=indexing
      tunnel: w668 -> [w1436]
      workers-P: _ -> [_]
      n430 = Bundle By Name("Y"=w1441, "dt"=w1440) -> (w1442:waveform(dbl))  [unwired: 1 out]
      n431 = Set Waveform Attribute(5:w1439, 6:w1438, 7:w1442) -> (3:w1437:waveform(dbl))  [unwired: 1 in, 2 out]
      n432 = call "downsample 1D array - double.vi"("Ave N"=w1443, "Array In"=w1441) -> ("Array Out"=w1444:dbl[])  [unwired: 1 out]
      n433 = Bundle By Name(cluster=w1437, "t0"=w1435, "Y"=w1444, "dt"=w1436) -> (w1445:waveform(dbl))
    }
    n434 = call <vilib>:"Mean.vi"("X"=w656) -> ("mean"=w644:dbl)  [unwired: 1 out]
    n435 = call <vilib>:"Mean.vi"("X"=w657) -> ("mean"=w645:dbl)  [unwired: 1 out]
    n436 = Cluster To Array(cluster=w623) -> (array=w620:dbl[])
    n437 = Reciprocal(x=w668) -> (1/x=→"Trap Disp. Freq. (Hz)":dbl)
    n438 = local read "Data points/scans (MCL)"() -> (w840:dbl)
    n439 = To Fixed-Point(number=w644) -> (fixed-point=w642:fxp<+/-,16,1>)  [unwired: 1 in]
    n440 = To Fixed-Point(number=w645) -> (fixed-point=w643:fxp<+/-,16,1>)  [unwired: 1 in]
    n441 = Bundle("Trap 1 Pos.", "Trap 2 Pos.") -> (w664:cluster{string, string})  [unwired: 1 out]
    n442 = Bundle By Name(cluster=w655, "Set 1"=w643, "Set 2"=w642) -> (→"Trap X AI1 (DMA)":T13)
    n443 = Cluster To Array(cluster=w664) -> (array=w661:string[])
    n444 = for "Trap Position" {
      tunnel: w670 -> [w912] mode=indexing
      tunnel: "Trap Disp. Downsample" -> [w911]
      tunnel: w668 -> [w909]
      tunnel: w666 -> [w908]
      tunnel: w665 -> [w906]
      tunnel: w661 -> [w905] mode=indexing
      tunnel: [w904] -> w618 mode=indexing
      tunnel: w620 -> [w902] mode=indexing
      tunnel: w619 -> [w900]
      n445 = call "downsample 1D array - double.vi"("Ave N"=w911, "Array In"=w912) -> ("Array Out"=w910:dbl[])  [unwired: 1 out]
      n446 = Subtract(x=w910, y=w902) -> (x-y=w903:dbl[])
      n447 = Multiply(x=w900, y=w903) -> (x*y=w901:dbl[])
      n448 = Bundle By Name("Y"=w901, "dt"=w909, "t0"=w908) -> (w907:waveform(dbl))  [unwired: 1 out]
      n449 = Set Waveform Attribute(5:w905, 6:w906, 7:w907) -> (3:w904:waveform(dbl))  [unwired: 1 in, 2 out]
    }
    "Trap Positions" <- w618
    n450 = Bundle("APD 1", "APD 2") -> (w861:cluster{string, string})  [unwired: 1 out]
    n451 = Cluster To Array(cluster=w861) -> (array=w858:string[])
    n452 = for "APD" {
      tunnel: w829 -> [w1424] mode=indexing
      tunnel: w695 -> [w1432]
      tunnel: [w1428] -> w702 mode=indexing
      tunnel: "APD Disp. Scale" -> [w1429]
      tunnel: w665 -> [w1427]
      tunnel: w858 -> [w1426] mode=indexing
      tunnel: "APD Disp. Downsample" -> [w1422]
      tunnel: [w1425] -> w857
      workers-P: _ -> [_]
      tunnel: w666 -> [w1421]
      n453 = call "integrate 1D array interval - double.vi"("Ave N"=w1422, "Array In"=w1424) -> ("Array Out"=w1423:dbl[])  [unwired: 1 out]
      n454 = Multiply(x=w1432, y=w1422) -> (x*y=w1425:dbl)
      n455 = Divide(x=w1423, y=w1429) -> (x/y=w1430:dbl[])
      n456 = Bundle By Name("t0"=w1421, "Y"=w1430, "dt"=w1425) -> (w1431:waveform(dbl))  [unwired: 1 out]
      n457 = Set Waveform Attribute(5:w1426, 6:w1427, 7:w1431) -> (3:w1428:waveform(dbl))  [unwired: 1 in, 2 out]
    }
    "APD Display Period (s)" <- w857
    n458 = Reciprocal(x=w857) -> (1/x=→"APD Display Freq. (Hz)":dbl)
    n459 = local read "Display Period (s)"() -> (w730:dbl)
    n460 = Increment(x=w840) -> (x+1=w841:dbl)
    n461 = Index Array(array=w618, index=0) -> (element=w616:waveform(dbl))
    n462 = To Double Precision Float(number=w746) -> (double precision float=w745:dbl[])
    n463 = feedback #2(w841) -> (w844:dbl)
    n464 = Select(t=0, s=w831, f=w844) -> (s? t:f=w837:dbl)
    n465 = Array Size(array=w745) -> (size(s)=w843:i32)
    n466 = Add(x=w843, y=w837) -> (x+y=w838:dbl)
    n467 = Unbundle By Name(w616) -> ("Y"=w614:dbl[])
    n468 = feedback #3(w746) -> (w827:u32[])
    n469 = Build Array (concatenate)(w827, w746) -> (w824:u32[])
    n470 = feedback #4(w682) -> (w701:u32[])
    n471 = Divide(x="Bead Sep. Int. Time (s)", y=w730) -> (x/y=w612:dbl)
    n472 = Build Array (concatenate)(w701, w682) -> (w700:u32[])
    n473 = Greater?(x=w838, y=w840) -> (0:w839:bool)
    n474 = feedback #5(w614) -> (w615:dbl[])
    n475 = Build Array (concatenate)(w614, w615) -> (w613:dbl[])
    n476 = Select(t=w837, s=w839, f=w838) -> (s? t:f=w836:dbl)
    n477 = feedback-in #2(w836) -> ()
    n478 = Array Size(array=w824) -> (size(s)=w821:i32)
    n479 = Array Size(array=w746) -> (size(s)=w823:i32)
    n480 = local read "MCL Scanning"() -> (w834:bool)
    n481 = local read "APD Integration Time (s)"() -> (w709:dbl)
    n482 = Build Array (concatenate)(w702, w862) -> (w704:waveform(dbl)[])
    "All Signals" <- w704
    n483 = Split 1D Array(array=w613, index=w612) -> (first subarray=w606:dbl[])  [unwired: 1 out]
    n484 = feedback-in #5(w606) -> ()
    n485 = Multiply(x=w823, y="APD Ave N") -> (x*y=w822:dbl)
    n486 = Greater?(x=w821, y=w822) -> (0:w825:bool)
    n487 = Not(x=w839) -> (.not. x?=w833:bool)
    n488 = To Double Precision Float(number=w682) -> (double precision float=w681:dbl[])
    n489 = call <vilib>:"Mean.vi"("X"=w606) -> ("mean"=w605:dbl)  [unwired: 1 out]
    "Mean T1 Position (nm)" <- w605
    n490 = Subtract(x=w606, y=w605) -> (x-y=w611:dbl[])
    n491 = Square(x=w611) -> (x^2=w610:dbl[])
    n492 = And(x=w833, y=w834) -> (x .and. y?=w835:bool)
    n493 = call <vilib>:"Mean.vi"("X"=w610) -> ("mean"=w609:dbl)  [unwired: 1 out]
    n494 = case shown="True" w825 {
      tunnel: w824 -> [w1133 w1140]
      tunnel: [w1133 w1138] -> w765
      tunnel: w822 -> [_ w1135]
      tunnel: w821 -> [_ w1139]
      tunnel: w700 -> [w1132 w1137]
      tunnel: [w1132 w1134] -> w697
      frame False {
      }
      frame True {
        n495 = Subtract(x=w1139, y=w1135) -> (x-y=w1136:dbl)
        n496 = Array Subset(array=w1140, index=w1136, length=w1135) -> (w1138:u32[])
        n497 = Array Subset(array=w1137, index=w1136, length=w1135) -> (w1134:u32[])
      }
    }
    n498 = feedback-in #3(w765) -> ()
    n499 = feedback-in #4(w697) -> ()
    n500 = Or(x=w835, y=w831) -> (x .or. y?=w832:bool)
    n501 = Square Root(x=w609) -> (sqrt(x)=w608:dbl)
    n502 = Equal?(x="Tab Control 6", y=T26."High Res Display") -> (x = y?=w754:bool)
    n503 = Multiply(x="APD Disp. Scale", y=w702) -> (x*y=w711:waveform(dbl)[])
    n504 = Multiply(x="APD Disp. Downsample", y=w709) -> (x*y=w707:dbl)
    n505 = Multiply(x=10.0, y=w608) -> (x*y=→"Trap 1 Position RMS (A)":dbl)
    n506 = Divide(x=w711, y=w707) -> (x/y=w679:waveform(dbl)[])
    n507 = Index Array(array=w679, index=0) -> (element=w689:waveform(dbl))
    n508 = case "For computing FFTs for display" shown="True" "Compute FFT" {
      tunnel: w706 -> [_ w1972]
      frame False {
      }
      frame True {
        n509 = Build Array("FFT 1 Choice 1", "FFT 1 Choice 2", "FFT 2 Choice 1", "FFT 2 Choice 2") -> (w1965:u16[])
        n510 = Array Size(array=w1972) -> (size(s)=w1971:i32)
        n511 = feedback-in #6(w1965) -> ()
        n512 = feedback #6(u16[] [100, 100, 100, 100]) -> (w1966:u16[])
        n513 = feedback-in #7("# Spectra to Ave.") -> ()
        n514 = feedback #7("# Spectra to Ave.") -> (w1963:dbl)
        n515 = Not Equal?(x="# Spectra to Ave.", y=w1963) -> (x != y?=w1962:bool)
        n516 = Not Equal?(x=w1965, y=w1966) -> (x != y?=w1964:bool)
        n517 = feedback #8(1.0) -> (w1949:dbl)
        n518 = Compound Arithmetic op=OR("Reset FFT", w1964, w1962) -> (w1947:bool)
        n519 = Select(t=1.0, s=w1947, f=w1949) -> (s? t:f=w1951:dbl)
        n520 = Greater?(x=w1951, y="# Spectra to Ave.") -> (0:w1970:bool)
        n521 = Increment(x=w1951) -> (x+1=w1950:dbl)
        n522 = feedback-in #8(w1950) -> ()
        n523 = local read "DMA Update Period (s)"() -> (w1945:dbl)
        n524 = Multiply(x="# Spectra to Ave.", y=w1945) -> (x*y=→"Ave. Time (s)":dbl)
        n525 = Build Array(cluster{"f0":dbl, "df":dbl, "magnitude":dbl[]} {"f0"=0.0, "df"=0.0, "magnitude"=[]} ("PSD")) -> (w1954:cluster{"f0":dbl, "df":dbl, "magnitude":dbl[]}[])
        n526 = Build Array(w1954, w1954, w1954, w1954) -> (w1956:T39)
        n527 = feedback #9(w1956) -> (w1961:T39)
        n528 = for {
          N: 4 -> [_]
          tunnel: w1965 -> [w1994] mode=indexing
          tunnel: w1972 -> [w1995]
          tunnel: w1971 -> [w1997]
          tunnel: w1947 -> [w1990]
          tunnel: w1970 -> [w1989]
          tunnel: "# Spectra to Ave." -> [w1988]
          tunnel: [w1987] -> w1960 mode=indexing
          tunnel: w1961 -> [w1992] mode=indexing
          tunnel: [w1991] -> w1948 mode=indexing
          tunnel: w1951 -> [w1986]
          n529 = Less?(x=w1994, y=w1997) -> (x < y?=w1996:bool)
          n530 = Index Array(array=w1995, index=w1994) -> (element=w1993:waveform(dbl))
          n531 = case shown="True" w1996 {
            tunnel: w1993 -> [_ w2014]
            tunnel: w1992 -> [w1999 w2012]
            tunnel: [w1999 w2000] -> w1991
            tunnel: w1990 -> [_ w2011]
            tunnel: w1989 -> [_ w2004]
            tunnel: w1988 -> [_ w2003]
            tunnel: [cluster{"f0":dbl, "df":dbl, "magnitude":dbl[]} {"f0"=0.0, "df"=0.0, "magnitude"=[]} ("PSD") w2005] -> w1987
            tunnel: w1986 -> [_ w2002]
            frame False {
            }
            frame True {
              n532 = call <vilib>:"Std Deviation and Variance.vi"("X"=w2014) -> ("mean"=w2015:dbl)  [unwired: 1 in, 2 out]
              n533 = Subtract(x=w2014, y=w2015) -> (x-y=w2013:waveform(dbl))
              n534 = xnode "Spectral Measurements"("Signals"=w2013) -> ("PSD"=w2007:cluster{"f0":dbl, "df":dbl, "magnitude":dbl[]})  [unwired: 1 in, 1 out]
              n535 = case shown="False" w2011 {
                tunnel: w2012 -> [w2024 _]
                tunnel: [w2020 w2029] -> w2000
                tunnel: w2007 -> [w2023 w2030]
                tunnel: w2004 -> [w2022 _]
                frame False {
                  n536 = Build Array (concatenate)(w2024, w2023) -> (w2021:cluster{"f0":dbl, "df":dbl, "magnitude":dbl[]}[])
                  n537 = case shown="True" w2022 {
                    tunnel: w2021 -> [w2025 w2028]
                    tunnel: [w2025 w2026] -> w2020
                    frame False {
                    }
                    frame True {
                      n538 = Delete From Array(array=w2028, index=0) -> (array with subset deleted=w2026:cluster{"f0":dbl, "df":dbl, "magnitude":dbl[]}[])  [unwired: 1 in, 1 out]
                    }
                  }
                }
                frame True {
                  n539 = Build Array(w2030) -> (w2029:cluster{"f0":dbl, "df":dbl, "magnitude":dbl[]}[])
                }
              }
              n540 = for {
                tunnel: w2000 -> [w2019] mode=indexing
                tunnel: [w2018] -> w2010 mode=indexing
                workers-P: _ -> [_]
                n541 = Unbundle By Name(w2019) -> ("magnitude"=w2018:dbl[])
              }
              n542 = Transpose 2D Array(2D array=w2010) -> (transposed array=w2009:dbl[][])
              n543 = for {
                tunnel: w2009 -> [w2017] mode=indexing
                tunnel: [w2016] -> w2008 mode=indexing
                workers-P: _ -> [_]
                n544 = Add Array Elements(numeric array=w2017) -> (sum=w2016:dbl)
              }
              n545 = Select(t=w2003, s=w2004, f=w2002) -> (s? t:f=w2001:dbl)
              n546 = Divide(x=w2008, y=w2001) -> (x/y=w2006:dbl[])
              n547 = Bundle By Name(cluster=w2007, "magnitude"=w2006) -> (w2005:cluster{"f0":dbl, "df":dbl, "magnitude":dbl[]})
            }
          }
        }
        n548 = case shown="True" w1947 {
          tunnel: w1948 -> [w1979 w1985]
          tunnel: [w1979 w1980] -> w1946
          frame False {
          }
          frame True {
            n549 = Array Subset(array=w1985, index (row)=0 ("index"), length (row)=4 ("length"), index (col)=0 ("index"), length (col)=1 ("length")) -> (w1980:T39)
          }
        }
        n550 = feedback-in #9(w1946) -> ()
        n551 = Split 1D Array(array=w1960, index=2) -> (first subarray=→"FFT 1":cluster{"f0":dbl, "df":dbl, "magnitude":dbl[]}[], second subarray=→"FFT 2":cluster{"f0":dbl, "df":dbl, "magnitude":dbl[]}[])
      }
    }
    n552 = Index Array(array=w679, index=1) -> (element=w687:waveform(dbl))
    n553 = case "For displaying the high resolution display (no downsampling)" shown="True" w754 {
      tunnel: w706 -> [_ w932]
      frame False {
      }
      frame True {
        n554 = Index Array(array=w932, index="High Res. Display") -> (element=w933:waveform(dbl))
        n555 = call <vilib>:"Std Deviation and Variance.vi"("X"=w933) -> ("mean"=w940:dbl, "standard deviation"=w945:dbl)  [unwired: 1 in, 1 out]
        "Mean Intensity" <- w940
        "Sigma" <- w945
        n556 = Subtract(x=w933, y=w940) -> (x-y=w939:waveform(dbl))
        n557 = Select(t=w939, s="Subtract mean", f=w933) -> (s? t:f=→"1 Channel":waveform(dbl))
        n558 = Divide(x=w945, y=w940) -> (x/y=→"Sigma/Mean":dbl)
        n559 = feedback #10(1) -> (w934:i32)
        n560 = Greater Or Equal?(x=w934, y="Slow mean N ave.") -> (x >= y?=w947:bool)
        n561 = Increment(x=w934) -> (x+1=w949:i32)
        n562 = Select(t=1, s=w947, f=w949) -> (s? t:f=w936:i32)
        n563 = feedback-in #10(w936) -> ()
        n564 = feedback #11() -> (w937:waveform(dbl))  [unwired: 1 out]
        n565 = case shown="Default" w934 {
          tunnel: [w952 w955] -> w938
          tunnel: w937 -> [w954 _]
          tunnel: w933 -> [w953 w955]
          frame Default {
            n566 = call-poly <vilib>:"Append Waveforms.vi"("waveform B"=w953, "waveform A"=w954) -> ("waveform out"=w952:waveform(dbl))  [unwired: 1 in, 8 out]
          }
          frame 1 {
          }
        }
        n567 = feedback-in #11(w938) -> ()
        n568 = case shown="True" w947 {
          tunnel: w938 -> [_ w951]
          frame False {
          }
          frame True {
            n569 = call <vilib>:"Mean.vi"("X"=w951) -> ("mean"=→"Slow mean":dbl)  [unwired: 1 out]
          }
        }
      }
    }
    n570 = case "For plotting results of scanning MCL" shown="True" w832 {
      tunnel: w831 -> [_ w1173]
      tunnel: w745 -> [_ w1269]
      tunnel: w840 -> [_ _]
      tunnel: w706 -> [_ w1243]
      tunnel: w681 -> [_ w1174]
      tunnel: w680 -> [_ w1147]
      frame False {
      }
      frame True {
        w1154 = u32 0 items=["Horizontal", "Vertical", "Central", "1st Diagonal", "2nd Diagonal"] ("Type of Symmetry")
        w1182 = u32 0 items=["Horizontal", "Vertical", "Central", "1st Diagonal", "2nd Diagonal"] ("Type of Symmetry")
        w1185 = u32 0 items=["Horizontal", "Vertical", "Central", "1st Diagonal", "2nd Diagonal"] ("Type of Symmetry")
        w1214 = u32 0 items=["Horizontal", "Vertical", "Central", "1st Diagonal", "2nd Diagonal"] ("Type of Symmetry")
        n571 = Index Array(array=w1243, index=10) -> (element=w1249:waveform(dbl))
        n572 = Index Array(array=w1243, index=11) -> (element=w1246:waveform(dbl))
        n573 = local read "Cycles/step (MCL)"() -> (w1199:u64)
        n574 = Index Array(array=w1243, index="Channel") -> (element=w1245:waveform(dbl))
        n575 = Unbundle(w1147) -> ("New Image"=w1146:T2, "New Image"=w1145:T2, "New Image"=w1144:T2, "New Image"=w1143:T2)
        n576 = Unbundle By Name(w1249) -> ("Y"=w1201:dbl[])
        n577 = Unbundle By Name(w1246) -> ("Y"=w1203:dbl[])
        n578 = Unbundle By Name(w1245) -> ("Y"=w1208:dbl[])
        n579 = call "downsample 1D array - double.vi"("Ave N"=w1199, "Array In"=w1201) -> ("Array Out"=w1200:dbl[])  [unwired: 1 out]
        n580 = call "downsample 1D array - double.vi"("Ave N"=w1199, "Array In"=w1203) -> ("Array Out"=w1202:dbl[])  [unwired: 1 out]
        n581 = call "downsample 1D array - double.vi"("Ave N"=w1199, "Array In"=w1208) -> ("Array Out"=w1207:dbl[])  [unwired: 1 out]
        n582 = feedback #12(w1269) -> (w1270:dbl[])
        n583 = Build Array (concatenate)(w1270, w1269) -> (w1251:dbl[])
        n584 = feedback #13(w1174) -> (w1176:dbl[])
        n585 = Build Array (concatenate)(w1176, w1174) -> (w1175:dbl[])
        n586 = local read "Scan steps (MCL)"() -> (w1156:u64)
        n587 = Select(t=w1269, s=w1173, f=w1251) -> (s? t:f=w1255:dbl[])
        n588 = feedback-in #12(w1255) -> ()
        n589 = Select(t=w1174, s=w1173, f=w1175) -> (s? t:f=w1157:dbl[])
        n590 = feedback-in #13(w1157) -> ()
        n591 = local read "Scan lines (y)"() -> (w1142:u64)
        n592 = local read "N APD Samp/step"() -> (w1158:dbl)
        n593 = feedback #14(w1200) -> (w1257:dbl[])
        n594 = Build Array (concatenate)(w1257, w1200) -> (w1248:dbl[])
        n595 = feedback #15(w1207) -> (w1267:dbl[])
        n596 = Build Array (concatenate)(w1267, w1207) -> (w1266:dbl[])
        n597 = feedback #16(w1202) -> (w1259:dbl[])
        n598 = Build Array (concatenate)(w1259, w1202) -> (w1260:dbl[])
        n599 = Select(t=w1200, s=w1173, f=w1248) -> (s? t:f=w1204:dbl[])
        n600 = feedback-in #14(w1204) -> ()
        n601 = Select(t=w1207, s=w1173, f=w1266) -> (s? t:f=w1206:dbl[])
        n602 = feedback-in #15(w1206) -> ()
        n603 = Select(t=w1202, s=w1173, f=w1260) -> (s? t:f=w1205:dbl[])
        n604 = feedback-in #16(w1205) -> ()
        n605 = Multiply(x=w1156, y=u64 2) -> (x*y=w1141:u64)
        n606 = call "integrate 1D array interval - double.vi"("Ave N"=w1158, "Array In"=w1157) -> ("Array Out"=w1169:dbl[])  [unwired: 1 out]
        n607 = call "integrate 1D array interval - double.vi"("Ave N"=w1158, "Array In"=w1255) -> ("Array Out"=w1254:dbl[])  [unwired: 1 out]
        n608 = Array Size(array=w1169) -> (size(s)=w1170:i32)
        n609 = Array Size(array=w1254) -> (size(s)=w1256:i32)
        n610 = Multiply(x=w1142, y=w1141) -> (x*y=w1172:u64)
        n611 = Multiply(x=w1142, y=w1141) -> (x*y=w1264:u64)
        n612 = call <vilib>:"Mean.vi"("X"=w1204) -> ("mean"=w1188:dbl)  [unwired: 1 out]
        n613 = Subtract(x=w1172, y=w1170) -> (x-y=w1163:u64)
        n614 = call <vilib>:"Mean.vi"("X"=w1206) -> ("mean"=w1193:dbl)  [unwired: 1 out]
        n615 = call <vilib>:"Mean.vi"("X"=w1205) -> ("mean"=w1191:dbl)  [unwired: 1 out]
        n616 = call <vilib>:"Mean.vi"("X"=w1169) -> ("mean"=w1160:dbl)  [unwired: 1 out]
        n617 = Subtract(x=w1264, y=w1256) -> (x-y=w1198:u64)
        n618 = call <vilib>:"Mean.vi"("X"=w1254) -> ("mean"=w1195:dbl)  [unwired: 1 out]
        n619 = Initialize Array(1.0 ("element"), w1163) -> (w1159:dbl[])
        n620 = Initialize Array(1.0 ("element"), w1198) -> (w1189:dbl[])
        n621 = Multiply(x=w1159, y=w1160) -> (x*y=w1161:dbl[])
        n622 = Multiply(x=w1189, y=w1191) -> (x*y=w1192:dbl[])
        n623 = Multiply(x=w1189, y=w1193) -> (x*y=w1194:dbl[])
        n624 = Multiply(x=w1189, y=w1188) -> (x*y=w1190:dbl[])
        n625 = Multiply(x=w1189, y=w1195) -> (x*y=w1196:dbl[])
        n626 = Build Array (concatenate)(w1204, w1190) -> (w1258:dbl[])
        n627 = Build Array (concatenate)(w1206, w1194) -> (w1262:dbl[])
        n628 = Build Array (concatenate)(w1205, w1192) -> (w1261:dbl[])
        n629 = Build Array (concatenate)(w1169, w1161) -> (w1171:dbl[])
        n630 = Build Array (concatenate)(w1254, w1196) -> (w1263:dbl[])
        n631 = Reshape Array(w1258, w1142, w1141) -> (w1224:dbl[][])
        n632 = Reshape Array(w1171, w1142, w1141) -> (w1167:dbl[][])
        n633 = Reshape Array(w1262, w1142, w1141) -> (w1216:dbl[][])
        n634 = Reshape Array(w1261, w1142, w1141) -> (w1231:dbl[][])
        n635 = Reshape Array(w1263, w1142, w1141) -> (w1241:dbl[][])
        n636 = Array Subset(array=w1231, index (col)=0 ("index"), length (col)=w1156) -> (w1236:dbl[][])  [unwired: 2 in]
        n637 = Array Subset(array=w1231, index (col)=w1156) -> (w1234:dbl[][])  [unwired: 3 in]
        n638 = Array Subset(array=w1216, index (col)=0 ("index"), length (col)=w1156) -> (w1222:dbl[][])  [unwired: 2 in]
        n639 = Array Subset(array=w1216, index (col)=w1156) -> (w1220:dbl[][])  [unwired: 3 in]
        n640 = Array Subset(array=w1167, index (col)=0 ("index"), length (col)=w1156) -> (w1166:dbl[][])  [unwired: 2 in]
        n641 = Array Subset(array=w1167, index (col)=w1156) -> (w1164:dbl[][])  [unwired: 3 in]
        n642 = Array Subset(array=w1241, index (col)=0 ("index"), length (col)=w1156) -> (w1240:dbl[][])  [unwired: 2 in]
        n643 = Array Subset(array=w1241, index (col)=w1156) -> (w1238:dbl[][])  [unwired: 3 in]
        n644 = Array Subset(array=w1224, index (col)=0 ("index"), length (col)=w1156) -> (w1229:dbl[][])  [unwired: 2 in]
        n645 = Array Subset(array=w1224, index (col)=w1156) -> (w1227:dbl[][])  [unwired: 3 in]
        n646 = for {
          tunnel: w1236 -> [w1278] mode=indexing
          tunnel: [w1277] -> w1235 mode=indexing
          workers-P: _ -> [_]
          n647 = Reverse 1D Array(array=w1278) -> (reversed array=w1277:dbl[])
        }
        n648 = for {
          tunnel: w1222 -> [w1274] mode=indexing
          tunnel: [w1273] -> w1221 mode=indexing
          workers-P: _ -> [_]
          n649 = Reverse 1D Array(array=w1274) -> (reversed array=w1273:dbl[])
        }
        n650 = for {
          tunnel: w1166 -> [w1272] mode=indexing
          tunnel: [w1271] -> w1165 mode=indexing
          workers-P: _ -> [_]
          n651 = Reverse 1D Array(array=w1272) -> (reversed array=w1271:dbl[])
        }
        n652 = for {
          tunnel: w1240 -> [w1280] mode=indexing
          tunnel: [w1279] -> w1239 mode=indexing
          workers-P: _ -> [_]
          n653 = Reverse 1D Array(array=w1280) -> (reversed array=w1279:dbl[])
        }
        n654 = for {
          tunnel: w1229 -> [w1276] mode=indexing
          tunnel: [w1275] -> w1228 mode=indexing
          workers-P: _ -> [_]
          n655 = Reverse 1D Array(array=w1276) -> (reversed array=w1275:dbl[])
        }
        n656 = Index Array(array=w1241, index (row)=0) -> (element=→"Waveform Graph":dbl[])  [unwired: 1 in]
        n657 = Add(x=w1235, y=w1234) -> (x+y=w1233:dbl[][])
        n658 = Add(x=w1221, y=w1220) -> (x+y=w1219:dbl[][])
        n659 = Add(x=w1165, y=w1164) -> (x+y=w1149:dbl[][])
        n660 = Add(x=w1239, y=w1238) -> (x+y=w1213:dbl[][])
        n661 = Add(x=w1228, y=w1227) -> (x+y=w1226:dbl[][])
        n662 = Divide(x=w1219, y=2) -> (x/y=w1217:dbl[][])
        n663 = Divide(x=w1233, y=2) -> (x/y=w1178:dbl[][])
        n664 = Divide(x=w1226, y=2) -> (x/y=w1180:dbl[][])
        n665 = To Single Precision Float(number=w1213) -> (single precision float=w1212:sgl[][])
        n666 = Transpose 2D Array(2D array=w1217) -> (transposed array=→"Data map":dbl[][])
        n667 = To Single Precision Float(number=w1149) -> (single precision float=w1153:sgl[][])
        n668 = To Single Precision Float(number=w1178) -> (single precision float=w1184:sgl[][])
        n669 = To Single Precision Float(number=w1180) -> (single precision float=w1181:sgl[][])
        n670 = call "IMAQ ArrayToImage"("Image Pixels (Float)"=w1212, "Image"=w1146) -> ("Image Out"=w1215:T2)  [unwired: 8 in, 1 out]
        n671 = call "IMAQ ArrayToImage"("Image Pixels (Float)"=w1153, "Image"=w1145) -> ("Image Out"=w1155:T2)  [unwired: 8 in, 1 out]
        n672 = call "IMAQ ArrayToImage"("Image Pixels (Float)"=w1184, "Image"=w1144) -> ("Image Out"=w1186:T2)  [unwired: 8 in, 1 out]
        n673 = call "IMAQ ArrayToImage"("Image Pixels (Float)"=w1181, "Image"=w1143) -> ("Image Out"=w1183:T2)  [unwired: 8 in, 1 out]
        n674 = call "IMAQ Symmetry"("Type of Symmetry"=w1214, "Image Src"=w1215) -> ("Image Dst Out"=w1210:T2)  [unwired: 3 in, 1 out]
        n675 = call "IMAQ Symmetry"("Type of Symmetry"=w1154, "Image Src"=w1155) -> ("Image Dst Out"=w1151:T2)  [unwired: 3 in, 1 out]
        n676 = call "IMAQ Symmetry"("Type of Symmetry"=w1185, "Image Src"=w1186) -> ("Image Dst Out"=→"Detection Laser X":T2)  [unwired: 3 in, 1 out]
        n677 = call "IMAQ Symmetry"("Type of Symmetry"=w1182, "Image Src"=w1183) -> ("Image Dst Out"=→"Detection Laser Y":T2)  [unwired: 3 in, 1 out]
        n678 = call "IMAQ Set Simple Calibration"("Calibration Axis Info"=T27 {"Origin Pixel"={"X"=0.0, "Y"=0.0}, "Angle Relative to Horizontal (deg)"=0.0, "Axis Reference"=0}, "Grid Descriptor"=T28 {"X Step"=0.3, "Y Step"=0.3, "Unit"=enum."Undefined"}, "Image"=w1210) -> ("Calibrated Image"=→"APD 1":T2)  [unwired: 7 in, 1 out]
        n679 = call "IMAQ Set Simple Calibration"("Calibration Axis Info"=T27 {"Origin Pixel"={"X"=0.0, "Y"=0.0}, "Angle Relative to Horizontal (deg)"=0.0, "Axis Reference"=0}, "Grid Descriptor"=T28 {"X Step"=0.3, "Y Step"=0.3, "Unit"=enum."Undefined"}, "Image"=w1151) -> ("Calibrated Image"=→"APD 2":T2)  [unwired: 7 in, 1 out]
      }
    }
    n680 = Subtract(x=w687, y="APD 2 Offset") -> (x-y=w684:waveform(dbl))
    n681 = Subtract(x=w689, y="APD 1 Offset") -> (x-y=w685:waveform(dbl))
    n682 = Index Array(array=w704, index=3) -> (element=w776:waveform(dbl))
    n683 = Index Array(array=w704, index=6) -> (element=w773:waveform(dbl))
    n684 = Build Array(w685, w684) -> (→"APD Chart":waveform(dbl)[])
    n685 = Array Size(array=w765) -> (size(s)=w820:i32)
    n686 = call <vilib>:"Std Deviation and Variance.vi"("X"=w697) -> ("standard deviation"=w696:dbl)  [unwired: 1 in, 2 out]
    n687 = Add Array Elements(numeric array=w697) -> (sum=w699:u32)
    n688 = Add Array Elements(numeric array=w765) -> (sum=w830:u32)
    n689 = call <vilib>:"Std Deviation and Variance.vi"("X"=w765) -> ("standard deviation"=w764:dbl)  [unwired: 1 in, 2 out]
    n690 = Divide(x="T1 offset_x (mV)", y=1000.0) -> (x/y=w777:dbl)
    n691 = Divide(x=w696, y=w695) -> (x/y=w692:dbl)
    "Rate sigma (Hz) 2" <- w692
    n692 = Multiply(x=w695, y=w820) -> (x*y=w698:dbl)
    "Int. Time (s)" <- w698
    n693 = Divide(x=w699, y=w698) -> (x/y=w693:dbl)
    "APD 2 Rate (Hz)" <- w693
    n694 = Divide(x=w830, y=w698) -> (x/y=w762:dbl)
    "APD 1 Rate (Hz)" <- w762
    n695 = Divide(x=w764, y=w695) -> (x/y=w763:dbl)
    "Rate sigma (Hz)" <- w763
    n696 = Divide(x=w692, y=w693) -> (x/y=→"Sigma/Mean 2":dbl)
    n697 = Divide(x=w763, y=w762) -> (x/y=→"Sigma/Mean":dbl)
    n698 = Divide(x="T2 offset_x (mV)", y=1000.0) -> (x/y=w775:dbl)
    n699 = case shown="0, Default" "Calibration" {
      tunnel: "T1 alpha_x (nm/V)" -> [_ w1109 w1130]
      tunnel: "T1 kappa_x (pN/nm)" -> [_ _ w1120]
      tunnel: "T2 alpha_x (nm/V)" -> [_ w1108 w1128]
      tunnel: "T2 kappa_x (pN/nm)" -> [_ _ w1121]
      tunnel: w776 -> [w1091 w1106 w1126]
      tunnel: w773 -> [w1090 w1104 w1124]
      tunnel: [w1091 w1103 w1123] -> w806
      tunnel: [w1090 w1102 w1122] -> w805
      tunnel: ["T1 X (V)" ("Label.Text") "T1 X (nm)" ("Label.Text") "T1 X (pN)" ("Label.Text")] -> w794
      tunnel: ["T2 X (V)" ("Label.Text") "T2 X (nm)" ("Label.Text") "T2 X (pN)" ("Label.Text")] -> w793
      tunnel: ["Position (V)" ("Label.Text") "Position (nm)" ("Label.Text") "Force (pN)" ("Label.Text")] -> w795
      tunnel: w775 -> [_ w1094 w1113]
      tunnel: w777 -> [_ w1097 w1115]
      tunnel: ["Mean (V)" ("Label.Text") "Mean (nm)" ("Label.Text") "Mean (pN)" ("Label.Text")] -> w790
      tunnel: ["Difference (V)" ("Label.Text") "Difference (nm)" ("Label.Text") "Difference (pN)" ("Label.Text")] -> w712
      frame 0, Default {
      }
      frame 1 {
        n700 = Unbundle By Name(w1106) -> ("Y"=w1110:dbl[])
        n701 = Unbundle By Name(w1104) -> ("Y"=w1095:dbl[])
        n702 = Subtract(x=w1110, y=w1097) -> (x-y=w1098:dbl[])
        n703 = Subtract(x=w1095, y=w1094) -> (x-y=w1096:dbl[])
        n704 = Multiply(x=w1096, y=w1108) -> (x*y=w1105:dbl[])
        n705 = Multiply(x=w1109, y=w1098) -> (x*y=w1107:dbl[])
        n706 = Bundle By Name(cluster=w1104, "Y"=w1105) -> (w1102:waveform(dbl))
        n707 = Bundle By Name(cluster=w1106, "Y"=w1107) -> (w1103:waveform(dbl))
      }
      frame 2 {
        n708 = Unbundle By Name(w1126) -> ("Y"=w1131:dbl[])
        n709 = Unbundle By Name(w1124) -> ("Y"=w1129:dbl[])
        n710 = Subtract(x=w1129, y=w1113) -> (x-y=w1114:dbl[])
        n711 = Subtract(x=w1131, y=w1115) -> (x-y=w1116:dbl[])
        n712 = Compound Arithmetic op=MULTIPLY(w1114, w1128, w1121) -> (w1125:dbl[])
        n713 = Compound Arithmetic op=MULTIPLY(w1120, w1130, w1116) -> (w1127:dbl[])
        n714 = Bundle By Name(cluster=w1124, "Y"=w1125) -> (w1122:waveform(dbl))
        n715 = Bundle By Name(cluster=w1126, "Y"=w1127) -> (w1123:waveform(dbl))
      }
    }
    n716 = feedback-in #17("Calibration") -> ()
    n717 = feedback #17(u16 1 ("Calibration")) -> (w797:u16)
    n718 = Not Equal?(x=w797, y="Calibration") -> (x != y?=w752:bool)
    n719 = Unbundle By Name(w776) -> ("Y"=w779:dbl[])
    n720 = Unbundle By Name(w773) -> ("Y"=w782:dbl[])
    n721 = Subtract(x=w779, y=w777) -> (x-y=w780:dbl[])
    n722 = Subtract(x=w782, y=w775) -> (x-y=w781:dbl[])
    n723 = Multiply(x=w781, y="T2 alpha_x (nm/V)") -> (x*y=w772:dbl[])
    n724 = Multiply(x="T1 alpha_x (nm/V)", y=w780) -> (x*y=w771:dbl[])
    n725 = Multiply(x=w805, y=-1.0) -> (x*y=w784:waveform(dbl))
    n726 = case shown="True" "Read Lateness and Rel Phase" {
      tunnel: w748 -> [w956 w978]
      tunnel: w747 -> [w957 w977]
      tunnel: [w956 w976] -> w768
      tunnel: [w957 w975] -> w767
      frame False {
      }
      frame True {
        n727 = xnode "Read/Write Control"("FPGA VI Reference In"=w978, "error in"=w977) -> ("FPGA VI Reference Out"=w976:T19, "error out"=w975:errorcluster, "GI Relative phase"=→"GI relative phase", "Relative phase"=→"Relative phase (AI1)", "AI Late Counter"=→"Late Counter (AI1)", "GI Late Counter"=→"GI Late Counter", "MCL Late Counter"=→"MCL Late Counter", "MCL Relative Phase"=→"Relative Phase (MCL)", "APD Acq Relative Phase"=→"APD Acq Relative Phase", "APD 1 Gate Relative Phase"=→"APD 1 Gate Relative Phase", "APD 2 Gate Relative Phase"=→"APD 2 Gate Relative Phase", "APD Acq Late Counter"=→"APD Acq Late Counter", "APD 1 Gate Late Counter"=→"APD 1 Gate Late Counter", "APD 2 Gate Late Counter"=→"APD 2 Gate Late Counter", "Green FB Relative Phase"=→"Relative phase (Green FB)", "GI Relative phase 2"=→"GI relative phase 2", "GI Late Counter 2"=→"GI Late Counter 2", "Trap Pos FIFO Timeout"=→"Trap Pos FIFO Timeout", "Trap AI FIFO Timeout"=→"Trap AI FIFO Timeout")
      }
    }
    n728 = Subtract(x=w772, y=w771) -> (x-y=w770:dbl[])
    n729 = Unbundle By Name(w805) -> ("Y"=w737:dbl[])
    n730 = Unbundle By Name(w806) -> ("Y"=w738:dbl[])
    n731 = Build Array(w806, w784) -> (→"Force":waveform(dbl)[])
    n732 = Subtract(x=w770, y="Offset (nm)") -> (x-y=w735:dbl[])
    n733 = call <vilib>:"Mean.vi"("X"=w737) -> ("mean"=w716:dbl)  [unwired: 1 out]
    "T2 X" <- w716
    n734 = Absolute Value(x=w738) -> (abs(x)=w739:dbl[])
    n735 = Absolute Value(x=w737) -> (abs(x)=w740:dbl[])
    n736 = call <vilib>:"Mean.vi"("X"=w738) -> ("mean"=w717:dbl)  [unwired: 1 out]
    "T1 X" <- w717
    n737 = Add(x=w739, y=w740) -> (x+y=w741:dbl[])
    n738 = Bundle By Name(cluster=w776, "Y"=w735) -> (w703:waveform(dbl))
    "Bead Separation" <- w703
    n739 = Divide(x=w741, y=2.0) -> (x/y=→"Vec Mean of T1 T2":dbl[])
    n740 = case shown="True" w752 {
      tunnel: w795 -> [_ w1084]
      tunnel: w794 -> [_ w1083]
      tunnel: w793 -> [_ w1082]
      tunnel: w790 -> [_ w1081]
      tunnel: w712 -> [_ w1080]
      frame False {
      }
      frame True {
        n741 = property on="Force" class="WFChart (strict)"("YScale.NameLbl.Text"=w1084) -> ()  [unwired: 2 in, 2 out]
        n742 = property on="T2 X" class="DigNum (strict)"("Caption.Text"=w1082) -> ()  [unwired: 2 in, 2 out]
        n743 = property on="T1 X" class="DigNum (strict)"("Caption.Text"=w1083) -> ()  [unwired: 2 in, 2 out]
        n744 = property on="Mean" class="DigNum (strict)"("Caption.Text"=w1081) -> ()  [unwired: 2 in, 2 out]
        n745 = property on="Difference" class="DigNum (strict)"("Caption.Text"=w1080) -> ()  [unwired: 2 in, 2 out]
      }
    }
    n746 = local read "Tether"() -> (w744:bool)
    n747 = Absolute Value(x=w717) -> (abs(x)=w714:dbl)
    n748 = Absolute Value(x=w716) -> (abs(x)=w713:dbl)
    n749 = Add(x=w714, y=w713) -> (x+y=w792:dbl)
    n750 = Subtract(x=w714, y=w713) -> (x-y=→"Difference":dbl)
    n751 = feedback #18(w735) -> (w734:dbl[])
    n752 = Divide(x=w792, y=2.0) -> (x/y=w743:dbl)
    "Mean" <- w743
    n753 = case shown="True" w744 {
      tunnel: w743 -> [_ w915]
      frame False {
      }
      frame True {
        n754 = Greater?(x="Lost Tether Alarm Threshold (pN)", y=w915) -> (0:w913:bool)
        n755 = case shown="True" w913 {
          frame False {
          }
          frame True {
            n756 = flat-sequence {
              frame #0 {
                # "stop only if saving"
                n757 = local read "Saving..."() -> (w928:bool)
                n758 = And(x=w928, y="TA Cancel Save?") -> (x .and. y?=w927:bool)
                n759 = local write "Stop Saving"(w927) -> ()
              }
              frame #1 {
                n760 = case shown="True" "TA Green Off?" {
                  frame False {
                  }
                  frame True {
                    w931 = FALSE ("Fl. Triggered...")
                    n761 = local write "Fl. Triggered..."(w931) -> ()
                    n762 = property on="Green Laser ON/Interlacing" class="Bool (strict)"("Val(Sgnl)"=w931) -> ()  [unwired: 2 in, 2 out]
                  }
                }
              }
            }
            n763 = local read "Time tether formed"() -> (w922:timestamp)
            n764 = Get Date/Time In Seconds() -> (seconds since 1Jan1904=w923:timestamp)
            n765 = Subtract(x=w923, y=w922) -> (x-y=w921:dbl)
            n766 = Number To Decimal String(number=w921) -> (decimal integer string=w918:string)  [unwired: 1 out]
            n767 = local read "Messages"() -> (w925:string)
            n768 = call <vilib>:"Beep.vi"() -> ()  [unwired: 3 in, 9 out]
            n769 = Concatenate Strings("Lost tether (" ("Message to add"), w918, " s)." ("string")) -> (w920:string)
            n770 = local write "Tether"(FALSE ("Tether")) -> ()
            n771 = call "Update messages.vi"("Message to add"=w920, "Old message string"=w925) -> ("New message string"=w924:string)
            n772 = local write "Messages"(w924) -> ()
            n773 = property on="Trap Pos. FB ON" class="Bool (strict)"("Val(Sgnl)"=FALSE ("Value (Signaling)")) -> ()  [unwired: 2 in, 2 out]
          }
        }
      }
    }
    n774 = Build Array (concatenate)(w735, w734) -> (w733:dbl[])
    n775 = Split 1D Array(array=w733, index=w612) -> (first subarray=w729:dbl[])  [unwired: 1 out]
    n776 = feedback-in #18(w729) -> ()
    n777 = call <vilib>:"Mean.vi"("X"=w729) -> ("mean"=w728:dbl)  [unwired: 1 out]
    "Bead Mean (nm)" <- w728
    n778 = Subtract(x=w729, y=w728) -> (x-y=w727:dbl[])
    n779 = Square(x=w727) -> (x^2=w726:dbl[])
    n780 = call <vilib>:"Mean.vi"("X"=w726) -> ("mean"=w725:dbl)  [unwired: 1 out]
    n781 = Square Root(x=w725) -> (sqrt(x)=w724:dbl)
    n782 = Multiply(x=10.0, y=w724) -> (x*y=→"RMS (Ang)":dbl)
    n783 = xnode "Read/Write Control"("FPGA VI Reference In"=w768, "error in"=w767) -> ("FPGA VI Reference Out"=w886:T19, "error out"=w880:errorcluster, "AI2 Y Sum Set 1"=w876, "AI2 Y Sum Set 2"=w875, "AI1 X Set 1"=w647, "AI1 X Set 2"=w646, "Trap Pos FB Int Signal"=→"Trap Pos FB Int Signal", "Trap Pos FB Int-Norm Signal"=→"Trap Pos FB Int-Norm Signal", "Trap Pos FB Action"=w640, "Scanning"=→"AOD Scanning", "Scan I"=→"AOD Scan I", "Scanning MCL"=w878, "Scan I (MCL)"=→"MCL Scan I", "Green FB Signals"=w815)  [unwired: 1 out]
    "MCL Scanning" <- w878
    "Trap Pos FB Action" <- w640
    n784 = local read "AI2 (V)"() -> (w877:cluster{"Set 1":dbl, "Set 2":dbl})
    n785 = Bundle By Name(cluster=w877, "Set 1"=w876, "Set 2"=w875) -> (w873:cluster{"Set 1":dbl, "Set 2":dbl})
    n786 = Divide(x=w640, y=327.67) -> (x/y=→"Action (%)":dbl)
    n787 = local read "Trap X (AI1)"() -> (w660:T10)
    n788 = Divide(x=w873, y=3276.7) -> (x/y=w872:cluster{"Set 1":dbl, "Set 2":dbl})
    n789 = local write "AI2 (V)"(w872) -> ()
    n790 = Bundle(cluster=w660, "Trap 1"=w647, "Trap 2"=w646) -> (→"Trap X (AI1)":T10)
    n791 = Divide(x=w815, y=3276.7) -> (x/y=w811:dbl)
    n792 = Unbundle By Name(w811) -> ("Green FB Ch 0"=w814, "Green FB Ch 1"=w813, "Green FB Ch 2"=w812)
    n793 = Divide(x=w814, y=w812) -> (x/y=w810:dbl)
    n794 = Divide(x=w813, y=w812) -> (x/y=w809:dbl)
    n795 = flat-sequence "To save data" {
      tunnel: [w2185] -> w898
      tunnel: [w2186] -> w897
      tunnel: w846 -> [w2179]
      tunnel: w731 -> [w2183]
      tunnel: ["Save Calibration"] -> w869
      tunnel: w866 -> [w2182]
      tunnel: [w2175] -> w865
      tunnel: [w2172] -> w864
      tunnel: [w2169] -> w863
      tunnel: w845 -> [w2171]
      tunnel: w750 -> [w2165]
      tunnel: [w2165] -> w749
      tunnel: ["Start Saving"] -> w705
      tunnel: [w2159] -> w628
      tunnel: [w2158] -> w627
      tunnel: w898 -> [w2420]
      tunnel: w897 -> [w2419]
      tunnel: w629 -> [w2418]
      tunnel: w869 -> [w2417]
      tunnel: w865 -> [w2415]
      tunnel: w864 -> [w2414]
      tunnel: w863 -> [w2413]
      tunnel: w718 -> [w2412]
      tunnel: w760 -> [w2411]
      tunnel: w749 -> [w2410]
      tunnel: w705 -> [w2409]
      tunnel: w703 -> [w2408]
      tunnel: w679 -> [w2407]
      tunnel: w628 -> [w2406]
      tunnel: w627 -> [w2405]
      tunnel: w626 -> [w2404]
      frame #0 {
        n796 = Or(x="Save N Sets", y="Start Saving") -> (x .or. y?=w2166:bool)
        n797 = To Double Precision Float(number=w2182) -> (double precision float=w2176:dbl)
        n798 = Build Array(w2166, "Save Calibration", w2179, w2171) -> (w2181:bool[])
        n799 = Compound Arithmetic op=OR("Save Calibration", w2179, w2166, w2171) -> (w2184:bool)
        n800 = Boolean Array To Number(Boolean array=w2181) -> (number=w2178:u32)
        n801 = feedback #19(FALSE ("Save APD Data\nwith Trap Data")) -> (w2160:bool)
        n802 = feedback #20(refnum<k0> refnum) -> (w2187:refnum<file>)
        n803 = feedback #21(refnum<k0> refnum) -> (w2162:refnum<file>)
        n804 = feedback #22(FALSE ("Save APD Data\nwith Trap Data")) -> (w2170:bool)
        n805 = feedback #23(refnum<k0> refnum) -> (w2173:refnum<file>)
        n806 = feedback #24(0) -> (w2189:i32)
        n807 = feedback #25() -> (w2177:u32)  [unwired: 1 out]
        n808 = case shown="True" w2184 {
          tunnel: [w2196 1] -> w2185
          tunnel: w2189 -> [w2198 _]
          tunnel: [w2197 w2216] -> w2186
          tunnel: w2187 -> [w2197 _]
          tunnel: w2183 -> [_ w2236]
          tunnel: w2176 -> [_ w2234]
          tunnel: w2178 -> [_ w2237]
          tunnel: [w2195 w2215] -> w2175
          tunnel: w2177 -> [w2195 _]
          tunnel: [w2194 w2213] -> w2172
          tunnel: w2173 -> [w2194 _]
          tunnel: [w2193 w2212] -> w2169
          tunnel: w2170 -> [w2193 _]
          tunnel: "Start Saving" -> [_ w2210]
          tunnel: w2165 -> [_ w2209]
          tunnel: [w2192 w2200] -> w2158
          tunnel: w2162 -> [w2192 _]
          tunnel: [w2191 w2199] -> w2159
          tunnel: w2160 -> [w2191 _]
          frame False {
            n809 = Increment(x=w2198) -> (x+1=w2196:i32)
          }
          frame True {
            w2206 = FALSE ("Start Saving")
            w2211 = 9.0  # File Version
            w2219 = FALSE ("prepend array or string size? (T)")
            w2217 = T33."big-endian, network order" ("byte order (0:big-endian, network order)")
            n810 = local read "BD 1 Frequency 1 (MHz)"() -> (w2233:dbl)
            n811 = local read "BD 2 Frequency 1 (MHz)"() -> (w2232:dbl)
            n812 = local read "BD 1 Frequency 2 (MHz)"() -> (w2231:dbl)
            n813 = local read "BD 2 Frequency 2 (MHz)"() -> (w2230:dbl)
            n814 = local read "BD 1 Frequency 3 (MHz)"() -> (w2229:dbl)
            n815 = local read "BD 2 Frequency 3 (MHz)"() -> (w2228:dbl)
            n816 = Array Size(array=w2209) -> (size(s)=w2208:i32)
            n817 = To Double Precision Float(number=w2208) -> (double precision float=w2207:dbl)
            n818 = local write "Save Calibration"(w2206) -> ()
            n819 = local write "Start Saving"(w2206) -> ()
            n820 = Build Array("Save APD Data\nwith Trap Data", "Save Trap Pos. Data") -> (w2203:bool[])
            n821 = Boolean Array To Number(Boolean array=w2203) -> (number=w2202:u32)
            n822 = Build Array(w2233, w2232, w2231, w2230, w2229, w2228) -> (w2227:dbl[])
            n823 = case shown="4" w2237 {
              tunnel: w2236 -> [w2308 w2328 w2344 w2382]
              tunnel: w2207 -> [w2313 w2335 w2364 w2401]
              tunnel: w2234 -> [w2312 w2334 w2363 w2400]
              tunnel: [w2309 w2330 w2355 w2392] -> w2225
              tunnel: [w2300 "Cal sets to save" w2345 w2383] -> w2215
              tunnel: w2227 -> [w2310 w2331 w2357 w2394]
              tunnel: "Save APD Data\nwith Trap Data" -> [w2307 _ w2341 w2380]
              tunnel: [w2307 w2322 w2341 w2380] -> w2212
              tunnel: w2211 -> [w2303 w2323 w2339 w2378]
              tunnel: w2210 -> [w2302 _ _ _]
              tunnel: [w2293 w2322 w2338 w2368] -> w2199
              tunnel: "Save Trap Pos. Data" -> [w2293 _ w2338 w2368]
              tunnel: w2202 -> [w2292 _ w2337 w2367]
              frame 1, Default {
                # "timeseries"
                n824 = case shown="True" "Profile" {
                  tunnel: [w2316 w2320] -> w2297
                  tunnel: [w2316 w2319] -> w2296
                  tunnel: [w2316 w2318] -> w2295
                  tunnel: [w2316 w2317] -> w2294
                  frame False {
                    w2316 = 0.0 ("f")
                  }
                  frame True {
                    n825 = local read "Current Position"() -> (w2321:cluster{dbl, dbl, dbl})
                    n826 = local read "Y change (mm)"() -> (w2317:dbl)
                    n827 = Unbundle(w2321) -> (w2320:dbl, w2319:dbl, w2318:dbl)
                  }
                }
                n828 = local read "Save ave N"() -> (w2315:dbl)
                n829 = Multiply(x=w2315, y=w2308) -> (x*y=w2314:dbl)
                n830 = To Double Precision Float(number=w2292) -> (double precision float=w2306:dbl)
                n831 = Build Array(w2303, w2308, w2314, w2313, w2312, 0.0 ("f")) -> (w2311:dbl[])
                n832 = Build Array(w2306, w2297, w2296, w2295, w2294) -> (w2304:dbl[])
                n833 = Select(t=u32 4000000000, s=w2302, f="N sets to save") -> (s? t:f=w2300:u32)
                n834 = Build Array (concatenate)(w2311, w2310, w2304) -> (w2309:dbl[])
              }
              frame 2 {
                w2325 = 0.0 ("f")
                w2322 = FALSE ("Save APD Data\nwith Trap Data")
                # "calibration"
                n835 = Boolean To (0,1)(Boolean=w2322) -> (0, 1=w2327:i16)
                n836 = To Double Precision Float(number=w2327) -> (double precision float=w2326:dbl)
                n837 = Build Array(w2326, w2325, w2325, w2325, w2325) -> (w2324:dbl[])
                n838 = Build Array(w2323, w2328, w2328, w2335, w2334, 1.0 ("t")) -> (w2332:dbl[])
                n839 = Build Array (concatenate)(w2332, w2331, w2324) -> (w2330:dbl[])
                "Calibrating Trap..." <- TRUE ("Calibrating...")
              }
              frame 4 {
                w2342 = 0.0 ("f")
                # "scan dir (x/y = 0/1)"
                # "cycles/step"
                # "n scans (f/b)"
                # "steps"
                # "freq. range"
                # "AOD raster scan"
                n840 = local read "Number of F/B Scans (AOD)"() -> (w2349:u16)
                n841 = local read "Cycles/step (AOD)"() -> (w2351:u64)
                n842 = local read "Scan Range (MHz)"() -> (w2354:dbl)
                n843 = local read "Scan steps (AOD)"() -> (w2353:u64)
                n844 = local read "Scan BD"() -> (w2361:bool)
                n845 = local read "Save ave N"() -> (w2366:dbl)
                n846 = Boolean To (0,1)(Boolean=w2361) -> (0, 1=w2360:i16)
                n847 = To Double Precision Float(number=w2349) -> (double precision float=w2348:dbl)
                n848 = To Double Precision Float(number=w2353) -> (double precision float=w2352:dbl)
                n849 = To Double Precision Float(number=w2351) -> (double precision float=w2350:dbl)
                n850 = To Double Precision Float(number=w2360) -> (double precision float=w2359:dbl)
                n851 = Multiply(x=w2366, y=w2344) -> (x*y=w2365:dbl)
                n852 = To Double Precision Float(number=w2337) -> (double precision float=w2343:dbl)
                n853 = Build Array(w2343, w2342, w2342, w2342, w2342) -> (w2340:dbl[])
                n854 = local read "N sets should be saved"() -> (w2346:dbl)
                n855 = Build Array(w2359, w2354, w2352, w2350, w2348) -> (w2356:dbl[])
                n856 = Build Array(w2339, w2344, w2365, w2364, w2363, 2.0 ("t")) -> (w2358:dbl[])
                n857 = Round Toward +Infinity(x=w2346) -> (ceil(x): smallest int >= x=w2347:dbl)
                n858 = Build Array (concatenate)(w2358, w2357, w2340, w2356) -> (w2355:dbl[])
                n859 = To Unsigned Long Integer(number=w2347) -> (unsigned 32bit integer=w2345:u32)
              }
              frame 8 {
                w2375 = 0.0 ("f")
                # "MCL raster scan"
                n860 = local read "Number of scans (MCL)"() -> (w2370:u64)
                n861 = local read "Scan lines (y)"() -> (w2369:u64)
                n862 = local read "2D or 1D Scan"() -> (w2372:bool)
                n863 = local read "Scan Range (V)\n(of steps)"() -> (w2391:dbl)
                n864 = local read "Fast Scan Dir"() -> (w2398:bool)
                n865 = local read "Cycles/step (MCL)"() -> (w2388:u64)
                n866 = local read "Scan steps (MCL)"() -> (w2390:u64)
                n867 = Select(t=w2369, s=w2372, f=w2370) -> (s? t:f=w2371:u64)
                n868 = Boolean To (0,1)(Boolean=w2372) -> (0, 1=w2374:i16)
                n869 = local read "Save ave N"() -> (w2403:dbl)
                n870 = local read "Initial X"() -> (w2377:dbl)
                n871 = local read "Initial Y"() -> (w2376:dbl)
                n872 = To Double Precision Float(number=w2374) -> (double precision float=w2373:dbl)
                n873 = Boolean To (0,1)(Boolean=w2398) -> (0, 1=w2397:i16)
                n874 = To Double Precision Float(number=w2371) -> (double precision float=w2386:dbl)
                n875 = To Double Precision Float(number=w2390) -> (double precision float=w2389:dbl)
                n876 = To Double Precision Float(number=w2388) -> (double precision float=w2387:dbl)
                n877 = To Double Precision Float(number=w2397) -> (double precision float=w2396:dbl)
                n878 = Multiply(x=w2403, y=w2382) -> (x*y=w2402:dbl)
                n879 = To Double Precision Float(number=w2367) -> (double precision float=w2381:dbl)
                n880 = local read "N sets should be saved (MCL)"() -> (w2384:dbl)
                n881 = Build Array(w2381, w2373, w2375, w2375, w2375) -> (w2379:dbl[])
                n882 = Build Array(w2396, w2391, w2389, w2387, w2386, w2377, w2376) -> (w2393:dbl[])
                n883 = Build Array(w2378, w2382, w2402, w2401, w2400, 3.0 ("t")) -> (w2395:dbl[])
                n884 = Round Toward +Infinity(x=w2384) -> (ceil(x): smallest int >= x=w2385:dbl)
                n885 = Build Array (concatenate)(w2395, w2394, w2379, w2393) -> (w2392:dbl[])
                n886 = To Unsigned Long Integer(number=w2385) -> (unsigned 32bit integer=w2383:u32)
              }
            }
            n887 = local read "Index"() -> (w2242:dbl)
            n888 = call "Create new save file.vi"("Insert"="", "Ext"=".dat", "Index In"=w2242) -> ("Path Out"=w2201:path, "Index Out"=w2214:dbl)
            n889 = local write "Save file name"(w2201) -> ()
            n890 = local write "Index"(w2214) -> ()
            n891 = local write "Save index"(w2214) -> ()
            n892 = Array Size(array=w2225) -> (size(s)=w2226:i32)
            n893 = Open/Create/Replace File(file path (use dialog)=w2201, operation (0:open)=T32."create", access (0:read/write)=enum16{"read/write", "read-only", "write-only"}."write-only") -> (refnum out=w2239:refnum<file>)  [unwired: 1 in, 4 out]
            n894 = local write "Saving..."(TRUE ("Saving...")) -> ()
            n895 = To Double Precision Float(number=w2226) -> (double precision float=w2224:dbl)
            n896 = String Length(string="Comment (data description)") -> (length=w2222:i32)
            n897 = To Double Precision Float(number=w2222) -> (double precision float=w2221:dbl)
            n898 = Deny Access(7:w2239) -> (3:w2238:refnum<file>)  [unwired: 1 in, 2 out]
            n899 = Build Array (concatenate)(w2224, w2225, w2221) -> (w2223:dbl[])
            n900 = case "If fluorescence data to be saved" shown="True" w2212 {
              tunnel: w2201 -> [_ w2291]
              tunnel: [refnum<k0> refnum w2271] -> w2213
              frame False {
              }
              frame True {
                w2270 = 0.0
                n901 = local read "APD Integration Time (s)"() -> (w2276:dbl)
                n902 = local read "N APD Samp/step"() -> (w2269:dbl)
                n903 = Path To String(path=w2291) -> (string=w2290:string)
                n904 = String Length(string=w2290) -> (length=w2289:i32)
                n905 = Subtract(x=w2289, y=4) -> (x-y=w2287:i32)
                n906 = String Subset(string=w2290, length (rest)=w2287) -> (substring=w2286:string)  [unwired: 1 out]
                n907 = Build Array(w2276, w2269, w2270, w2270, w2270, w2270, w2270, w2270) -> (w2273:dbl[])
                n908 = Concatenate Strings(w2286, "_fl.dat" ("string")) -> (w2284:string)
                n909 = Array Size(array=w2273) -> (size(s)=w2275:i32)
                n910 = String To Path(string=w2284) -> (path=w2280:path)
                n911 = Open/Create/Replace File(file path (use dialog)=w2280, operation (0:open)=T32."create", access (0:read/write)=enum16{"read/write", "read-only", "write-only"}."write-only") -> (refnum out=w2281:refnum<file>)  [unwired: 1 in, 4 out]
                n912 = Deny Access(7:w2281) -> (3:w2277:refnum<file>)  [unwired: 1 in, 2 out]
                n913 = To Double Precision Float(number=w2275) -> (double precision float=w2274:dbl)
                n914 = Build Array (concatenate)(w2274, w2273) -> (w2272:dbl[])
                n915 = Write to Binary File(file (use dialog)=w2277, data=w2272, 5:FALSE ("prepend array or string size? (T)"), 9:T33."big-endian, network order" ("byte order (0:big-endian, network order)")) -> (refnum out=w2271:refnum<file>)  [unwired: 1 in, 3 out]
              }
            }
            n916 = case shown="True" w2199 {
              tunnel: w2201 -> [_ w2253]
              tunnel: [refnum<k0> refnum w2252] -> w2200
              frame False {
              }
              frame True {
                w2248 = 0.0 ("element")
                n917 = Path To String(path=w2253) -> (string=w2267:string)
                n918 = Build Array(w2248, w2248, w2248, w2248, w2248, w2248, w2248, w2248) -> (w2249:dbl[])
                n919 = String Length(string=w2267) -> (length=w2266:i32)
                n920 = Subtract(x=w2266, y=4) -> (x-y=w2264:i32)
                n921 = Array Size(array=w2249) -> (size(s)=w2251:i32)
                n922 = String Subset(string=w2267, length (rest)=w2264) -> (substring=w2263:string)  [unwired: 1 out]
                n923 = To Double Precision Float(number=w2251) -> (double precision float=w2250:dbl)
                n924 = Concatenate Strings(w2263, "_pos.dat" ("string")) -> (w2261:string)
                n925 = Build Array (concatenate)(w2250, w2249) -> (w2247:dbl[])
                n926 = String To Path(string=w2261) -> (path=w2257:path)
                n927 = Open/Create/Replace File(file path (use dialog)=w2257, operation (0:open)=T32."create", access (0:read/write)=enum16{"read/write", "read-only", "write-only"}."write-only") -> (refnum out=w2258:refnum<file>)  [unwired: 1 in, 4 out]
                n928 = Deny Access(7:w2258) -> (3:w2254:refnum<file>)  [unwired: 1 in, 2 out]
                n929 = Write to Binary File(file (use dialog)=w2254, data=w2247, 5:FALSE ("prepend array or string size? (T)"), 9:T33."big-endian, network order" ("byte order (0:big-endian, network order)")) -> (refnum out=w2252:refnum<file>)  [unwired: 1 in, 3 out]
              }
            }
            n930 = Write to Binary File(file (use dialog)=w2238, data=w2223, 5:w2219, 9:w2217) -> (refnum out=w2220:refnum<file>)  [unwired: 1 in, 3 out]
            n931 = Write to Binary File(file (use dialog)=w2220, data="Comment (data description)", 5:w2219, 9:w2217) -> (refnum out=w2216:refnum<file>)  [unwired: 1 in, 3 out]
          }
        }
        n932 = feedback-in #19(w2159) -> ()
        n933 = feedback-in #20(w2186) -> ()
        n934 = feedback-in #21(w2158) -> ()
        n935 = feedback-in #22(w2169) -> ()
        n936 = feedback-in #23(w2172) -> ()
        n937 = feedback-in #24(w2185) -> ()
        n938 = feedback-in #25(w2175) -> ()
      }
      frame #1 {
        n939 = local read "Saving..."() -> (w2416:bool)
        n940 = case shown="True" w2416 {
          tunnel: w2420 -> [_ w2430]
          tunnel: w2419 -> [_ w2444]
          tunnel: w2418 -> [_ w2440]
          tunnel: w2417 -> [_ w2439]
          tunnel: w2415 -> [_ w2438]
          tunnel: w2414 -> [_ w2433]
          tunnel: w2413 -> [_ w2432]
          tunnel: w2412 -> [_ w2431]
          tunnel: w2411 -> [_ w2429]
          tunnel: w2410 -> [_ w2427]
          tunnel: w2409 -> [_ w2426]
          tunnel: w2408 -> [_ w2425]
          tunnel: w2407 -> [_ w2424]
          tunnel: w2406 -> [_ w2423]
          tunnel: w2405 -> [_ w2422]
          tunnel: w2404 -> [_ w2421]
          frame False {
          }
          frame True {
            n941 = Multiply(x=w2430, y=w2429) -> (x*y=→"Time (s)":dbl)
            n942 = Less Or Equal?(x=w2430, y=w2438) -> (x <= y?=w2442:bool)
            n943 = Or(x="Stop Saving", y="Abort save 2") -> (x .or. y?=w2434:bool)
            n944 = Not(x=w2434) -> (.not. x?=w2443:bool)
            n945 = And(x=w2442, y=w2443) -> (x .and. y?=w2441:bool)
            n946 = case shown="True" w2441 {
              tunnel: w2444 -> [w2451 w2519]
              tunnel: [0.0 w2522] -> w2437
              tunnel: w2430 -> [_ w2520]
              tunnel: w2438 -> [_ w2521]
              tunnel: w2440 -> [_ w2516]
              tunnel: w2439 -> [_ _]
              tunnel: w2433 -> [w2449 w2509]
              tunnel: w2432 -> [w2448 w2510]
              tunnel: w2431 -> [_ w2508]
              tunnel: w2427 -> [_ w2507]
              tunnel: w2426 -> [_ w2461]
              tunnel: w2425 -> [_ w2500]
              tunnel: w2424 -> [_ w2478]
              tunnel: w2423 -> [w2445 w2459]
              tunnel: w2422 -> [w2446 w2458]
              tunnel: w2421 -> [_ w2455]
              frame False {
                w2447 = FALSE
                n947 = Close File(refnum=w2451) -> ()  [unwired: 1 in, 2 out]
                n948 = case shown="True" w2448 {
                  tunnel: w2449 -> [_ w2453]
                  frame False {
                  }
                  frame True {
                    n949 = Close File(refnum=w2453) -> ()  [unwired: 1 in, 2 out]
                  }
                }
                n950 = case shown="True" w2445 {
                  tunnel: w2446 -> [_ w2452]
                  frame False {
                  }
                  frame True {
                    n951 = Close File(refnum=w2452) -> ()  [unwired: 1 in, 2 out]
                  }
                }
                n952 = local write "Raster Scanning..."(w2447) -> ()
                n953 = local write "Calibrating Trap..."(w2447) -> ()
                n954 = call <vilib>:"Beep.vi"() -> ()  [unwired: 3 in, 9 out]
                n955 = local write "Stop Saving"(w2447) -> ()
                "Saving..." <- w2447
              }
              frame True {
                n956 = local read "Calibrating Trap..."() -> (w2511:bool)
                n957 = case "Write fl. data" shown="True" w2510 {
                  tunnel: w2509 -> [_ w2545]
                  tunnel: w2508 -> [_ w2544]
                  frame False {
                  }
                  frame True {
                    n958 = Write to Binary File(file (use dialog)=w2545, data=w2544, 5:FALSE ("prepend array or string size? (T)"), 9:T33."big-endian, network order" ("byte order (0:big-endian, network order)")) -> ()  [unwired: 1 in, 4 out]
                  }
                }
                n959 = Greater?(x="Save ave N", y=1.0) -> (0:w2514:bool)
                n960 = Not(x=w2511) -> (.not. x?=w2513:bool)
                n961 = And(x=w2513, y=w2514) -> (x .and. y?=w2456:bool)
                n962 = case shown="True" w2456 {
                  tunnel: w2455 -> [w2525 w2536]
                  tunnel: [w2525 w2528] -> w2454
                  tunnel: "Save ave N" -> [_ w2529]
                  frame False {
                  }
                  frame True {
                    w2526 = 2 ("dimension size")
                    n963 = Array Size(array=w2536) -> (size(s)=w2530:i32)
                    n964 = Divide(x=w2530, y=w2526) -> (x/y=w2534:dbl)
                    n965 = Reshape Array(w2536, w2534, w2526) -> (w2535:u64[][])
                    n966 = Transpose 2D Array(2D array=w2535) -> (transposed array=w2533:u64[][])
                    n967 = for {
                      tunnel: w2533 -> [w2538] mode=indexing
                      tunnel: [w2537] -> w2527 mode=indexing
                      tunnel: w2529 -> [w2539]
                      workers-P: _ -> [_]
                      n968 = call "downsample 1D array - U64.vi"("Ave N"=w2539, "Array In"=w2538) -> ("Array Out"=w2537:u64[])  [unwired: 1 in]
                    }
                    n969 = Transpose 2D Array(2D array=w2527) -> (transposed array=w2532:u64[][])
                    n970 = Divide(x=w2530, y=w2529) -> (x/y=w2531:dbl)
                    n971 = Reshape Array(w2532, w2531) -> (w2528:u64[])
                  }
                }
                n972 = case shown="True" w2456 {
                  tunnel: w2516 -> [w2548 w2560]
                  tunnel: [w2548 w2552] -> w2512
                  tunnel: "Save ave N" -> [_ w2553]
                  tunnel: w2507 -> [_ w2551]
                  frame False {
                  }
                  frame True {
                    n973 = Array Size(array=w2560) -> (size(s)=w2554:i32)
                    n974 = Array Size(array=w2551) -> (size(s)=w2550:i32)
                    n975 = Divide(x=w2554, y=w2550) -> (x/y=w2558:dbl)
                    n976 = Reshape Array(w2560, w2558, w2550) -> (w2559:i16[][])
                    n977 = Transpose 2D Array(2D array=w2559) -> (transposed array=w2557:i16[][])
                    n978 = for {
                      tunnel: w2557 -> [w2563] mode=indexing
                      tunnel: [w2562] -> w2549 mode=indexing
                      tunnel: w2553 -> [w2561]
                      workers-P: _ -> [_]
                      n979 = call "downsample 1D array - I16.vi"("Ave N"=w2561, "Array In"=w2563) -> ("Array Out"=w2562:i16[])  [unwired: 1 out]
                    }
                    n980 = Transpose 2D Array(2D array=w2549) -> (transposed array=w2556:i16[][])
                    n981 = Divide(x=w2554, y=w2553) -> (x/y=w2555:dbl)
                    n982 = Reshape Array(w2556, w2555) -> (w2552:i16[])
                  }
                }
                n983 = Index Array(array=w2478, index=1) -> (element=w2481:waveform(dbl))
                n984 = Index Array(array=w2478, index=0) -> (element=w2483:waveform(dbl))
                n985 = Unbundle By Name(w2481) -> ("Y"=w2485:dbl[])
                n986 = Unbundle By Name(w2483) -> ("Y"=w2493:dbl[])
                n987 = case "Write trap pos. data" shown="True" w2459 {
                  tunnel: w2458 -> [_ w2541]
                  tunnel: w2454 -> [_ w2540]
                  frame False {
                  }
                  frame True {
                    n988 = Write to Binary File(file (use dialog)=w2541, data=w2540, 5:FALSE ("prepend array or string size? (T)"), 9:T33."big-endian, network order" ("byte order (0:big-endian, network order)")) -> ()  [unwired: 1 in, 4 out]
                  }
                }
                n989 = Write to Binary File(file (use dialog)=w2519, data=w2512, 5:FALSE ("prepend array or string size? (T)"), 9:T33."big-endian, network order" ("byte order (0:big-endian, network order)")) -> ()  [unwired: 1 in, 4 out]
                n990 = feedback #26(w2485) -> (w2487:dbl[])
                n991 = Build Array (concatenate)(w2487, w2485) -> (w2486:dbl[])
                n992 = Select(t=w2485, s=w2461, f=w2486) -> (s? t:f=w2471:dbl[])
                n993 = feedback-in #26(w2471) -> ()
                n994 = feedback #27(w2493) -> (w2506:dbl[])
                n995 = Build Array (concatenate)(w2506, w2493) -> (w2505:dbl[])
                n996 = Select(t=w2493, s=w2461, f=w2505) -> (s? t:f=w2480:dbl[])
                n997 = feedback-in #27(w2480) -> ()
                n998 = Divide(x=w2520, y=w2521) -> (x/y=w2523:dbl)
                n999 = Multiply(x=w2523, y=100.0) -> (x*y=w2522:dbl)
                n1000 = Build Array(w2480, w2471) -> (→"Saved APD":dbl[][])
                n1001 = Array Size(array=w2480) -> (size(s)=w2498:i32)
                n1002 = Unbundle By Name(w2500) -> ("Y"=w2504:dbl[])
                n1003 = Subtract(x=w2498, y="N pts to average") -> (x-y=w2474:i32)
                n1004 = Multiply(x="N pts to average", y=u16 2) -> (x*y=w2475:u16)
                n1005 = Subtract(x=w2498, y=w2475) -> (x-y=w2473:i32)
                n1006 = feedback #28(w2504) -> (w2503:dbl[])
                n1007 = Build Array (concatenate)(w2503, w2504) -> (w2502:dbl[])
                n1008 = Select(t=w2504, s=w2461, f=w2502) -> (s? t:f=w2501:dbl[])
                "Trap Delta Graph" <- w2501
                n1009 = feedback-in #28(w2501) -> ()
                n1010 = Array Subset(array=w2480, index=w2474, length="N pts to average") -> (w2497:dbl[])
                n1011 = Array Subset(array=w2480, index=w2473, length="N pts to average") -> (w2496:dbl[])
                n1012 = Array Subset(array=w2471, index=w2474, length="N pts to average") -> (w2477:dbl[])
                n1013 = Array Subset(array=w2471, index=w2473, length="N pts to average") -> (w2476:dbl[])
                n1014 = call <vilib>:"Mean.vi"("X"=w2497) -> ("mean"=w2495:dbl)  [unwired: 1 out]
                n1015 = call <vilib>:"Mean.vi"("X"=w2477) -> ("mean"=w2470:dbl)  [unwired: 1 out]
                n1016 = call <vilib>:"Mean.vi"("X"=w2496) -> ("mean"=w2494:dbl)  [unwired: 1 out]
                n1017 = call <vilib>:"Mean.vi"("X"=w2476) -> ("mean"=w2469:dbl)  [unwired: 1 out]
                n1018 = Subtract(x=w2470, y=w2469) -> (x-y=w2460:dbl)
                "Delta Fl. 2" <- w2460
                n1019 = Subtract(x=w2495, y=w2494) -> (x-y=w2492:dbl)
                "Delta Fl. 1" <- w2492
                n1020 = Initialize Array(w2492, 1 ("dimension size")) -> (w2489:dbl[])
                n1021 = Initialize Array(w2460, 1 ("dimension size")) -> (w2466:dbl[])
                n1022 = feedback #29(w2489) -> (w2490:dbl[])
                n1023 = Build Array (concatenate)(w2490, w2489) -> (w2488:dbl[])
                n1024 = feedback #30(w2466) -> (w2467:dbl[])
                n1025 = Build Array (concatenate)(w2467, w2466) -> (w2465:dbl[])
                n1026 = Select(t=w2489, s=w2461, f=w2488) -> (s? t:f=w2464:dbl[])
                n1027 = feedback-in #29(w2464) -> ()
                n1028 = Select(t=w2466, s=w2461, f=w2465) -> (s? t:f=w2463:dbl[])
                n1029 = feedback-in #30(w2463) -> ()
                n1030 = Build Array(w2464, w2463) -> (→"Save APD Deriv":dbl[][])
              }
            }
            "Progress" <- w2437
            "Progress 2" <- w2437
          }
        }
      }
    }
    n1031 = Bundle By Name(cluster=w811, "Green FB Ch 0"=w810, "Green FB Ch 1"=w809) -> (w789:cluster{})
    "Green FB Signals (V)" <- w789
    n1032 = Unbundle By Name(w789) -> ("Green FB Ch 2"=→"Green FB Plot")
    n1033 = local read "wait to reset values"() -> (w881:bool)
    n1034 = Not(x=w878) -> (.not. x?=w882:bool)
    n1035 = And(x=w882, y=w881) -> (x .and. y?=w883:bool)
    n1036 = case "Part of MCL raster scanning: returns to initial positions after scan done" shown="True" w883 {
      tunnel: w886 -> [w1718 w1725]
      tunnel: [w1718 w1724] -> w885
      tunnel: w880 -> [w1717 w1723]
      tunnel: [w1717 w1722] -> w879
      frame False {
      }
      frame True {
        w1733 = 10.0 ("y")
        w1732 = 32767.0 ("y")
        # "to return scan values\nafter a synchronous \nAOM scan"
        n1037 = local read "AO2"() -> (w1726:dbl)
        n1038 = local read "AO1"() -> (w1727:dbl)
        n1039 = local write "wait to reset values"(FALSE ("wait to reset values")) -> ()
        n1040 = Multiply(x=w1727, y=w1732) -> (x*y=w1729:dbl)
        n1041 = Multiply(x=w1726, y=w1732) -> (x*y=w1731:dbl)
        n1042 = Divide(x=w1729, y=w1733) -> (x/y=w1728:dbl)
        n1043 = Divide(x=w1731, y=w1733) -> (x/y=w1730:dbl)
        n1044 = To Word Integer(number=w1728) -> (16bit integer=w1734:i16)
        n1045 = To Word Integer(number=w1730) -> (16bit integer=w1735:i16)
        n1046 = local read "Total Counts (ticks)"() -> (w1719:u32)
        n1047 = xnode "Read/Write Control"("FPGA VI Reference In"=w1725, "error in"=w1723, "AO1"=w1734, "AO2"=w1735, "MCL count"=w1719) -> ("FPGA VI Reference Out"=w1724:T19, "error out"=w1722:errorcluster)
        n1048 = local read "Scan Range (V)\n(of steps)"() -> (w1720:dbl)
        n1049 = property on="Scan Range (V)\n(of steps)" class="DigNum (strict)"("Val(Sgnl)"=w1720) -> ()  [unwired: 2 in, 2 out]
      }
    }
    n1050 = node-c288() -> ()  [unwired: 2 out]
  }
  n1051 = timed-loop "Control parameters (event loop)" {
    tunnel: w8 -> [w2568]
    shift-right: [w2567] -> _
    shift-left: errorcluster {"status"=FALSE, "code"=0, "source"=""} ("error out") -> [w2566]
    tunnel: [w2565] -> w203
    timing: w50 -> [_]
    timing-out: [_] -> w49
    tunnel: w22 -> [w2564]
    stop <- w2565 stop-if-true
    n1052 = node-c288() -> ()  [unwired: 2 out]
    n1053 = event shown="[0] \"AI Count (ticks)\", \"Sets to FIFO (Traps)\", \"Save ave N\", \"FPGA Ave.\", \"# Samples/channel\", \"N sets to save\": Value Change" {
      selector: _ -> [_ _ _ _ _ _ _ _ _ _ _ _ _ _ _ _ _ _ _ _ _ _ _ _ _ _ _ _ _ _ _ _ _ _ _ _ _ _ _ _ _ _ _ _ _ _ _ _ _ _ _ _ _]
      dyn-events: _ -> [_ _ _ _ _ _ _ _ _ _ _ _ _ _ _ _ _ _ _ _ _ _ _ _ _ _ _ _ _ _ _ _ _ _ _ _ _ _ _ _ _ _ _ _ _ _ _ _ _ _ _ _ _]
      timeout: _ -> [_ _ _ _ _ _ _ _ _ _ _ _ _ _ _ _ _ _ _ _ _ _ _ _ _ _ _ _ _ _ _ _ _ _ _ _ _ _ _ _ _ _ _ _ _ _ _ _ _ _ _ _ _]
      tunnel: w2568 -> [w2606 _ _ _ w2674 _ w2738 _ _ _ _ w2804 _ _ w2873 w2925 w2956 w2988 w3076 w3120 w3168 w3217 w3270 w3323 w3376 w3429 w3482 w3542 w3599 w3734 w3782 w3856 _ w3942 w3967 w3999 w4045 w4070 _ w4099 _ _ _ _ w4251 _ w4310 w4334 w4364 w4418 w4443 _ w4481]
      tunnel: [w2605 _ _ _ w2664 _ w2737 _ _ w2769 _ w2783 _ _ w2872 w2921 w2953 w2985 w3075 w3118 w3167 w3211 w3264 w3317 w3370 w3423 w3476 w3540 w3598 w3732 w3780 w3854 _ w3940 w3965 w3989 w4043 w4068 _ w4097 _ _ _ _ w4249 _ _ _ _ _ _ _ _] -> w2567
      tunnel: w2566 -> [w2604 _ _ _ w2673 _ w2736 _ _ w2769 _ w2803 _ _ w2871 w2920 w2952 w2984 w3074 w3119 w3166 w3216 w3269 w3322 w3375 w3428 w3481 w3541 w3597 w3733 w3781 w3855 _ w3941 w3966 w3998 w4044 w4069 _ w4098 _ _ _ _ w4250 _ w4309 w4333 w4363 w4417 w4442 _ w4480]
      tunnel: [_ _ _ _ _ _ _ _ _ w2768 _ _ _ _ _ _ _ _ _ _ _ _ _ _ _ _ _ _ _ _ _ _ _ _ _ _ _ _ _ _ _ _ _ _ _ _ _ _ _ _ _ _ _] -> w2565
      tunnel: [_ _ _ _ _ _ _ "Round T1 X" _ _ _ _ _ _ _ _ _ _ _ _ _ _ _ _ _ _ _ _ _ _ _ _ _ _ _ _ _ _ _ _ _ _ _ _ _ _ _ _ _ _ _ _ _] -> _
      tunnel: [_ _ _ "Adjust Scale\nto Mean" _ _ _ _ _ _ _ _ _ _ _ _ _ _ _ _ _ _ _ _ _ _ _ _ _ _ _ _ _ _ _ _ _ _ _ _ _ _ _ _ _ _ _ _ _ _ "Set SP to Reading" _ _] -> _
      tunnel: [_ _ _ _ _ _ _ _ "Round T2 X" _ "Delayed Interlace Start" _ _ _ _ _ _ _ _ _ _ _ _ _ _ _ _ _ _ _ _ _ _ _ _ _ _ _ _ _ _ _ _ _ _ _ _ _ _ _ _ _ _] -> _
      tunnel: w2564 -> [_ _ _ _ _ _ _ _ _ _ _ _ _ _ _ _ _ _ _ _ _ _ _ _ _ _ _ _ _ _ _ _ _ _ _ _ _ _ _ _ _ _ _ w4242 _ _ _ _ _ _ _ _ _]
      event "AI Count (ticks)", "Sets to FIFO (Traps)", "Save ave N", "FPGA Ave.", "# Samples/channel", "N sets to save": Value Change {
        # "So that if 'Save ave N' is updated, the AOD scanning code updates too."
        n1054 = event-data() -> ()  [unwired: 6 out]
        n1055 = local read "AI Count (ticks)"() -> (w2586:u32)
        n1056 = Boolean To (0,1)(Boolean="Sets to FIFO (Traps)") -> (0, 1=w2596:cluster{"Set 1":i16, "Set 2":i16, "Set 3":i16})
        n1057 = xnode "Read/Write Control"("FPGA VI Reference In"=w2606, "error in"=w2604, "ai count"=w2586, "AI1 Sets to FIFO"="Sets to FIFO (Traps)", "N of AI1 Int Acq Sets"="N Acq Sets (Traps + Fl.)") -> ("error out"=w2605:errorcluster)  [unwired: 1 out]
        n1058 = Cluster To Array(cluster=w2596) -> (array=w2595:i16[])
        n1059 = To Unsigned Long Integer(number=w2595) -> (unsigned 32bit integer=w2575:u32[])
        n1060 = local read "Scan steps (AOD)"() -> (w2597:u64)
        n1061 = Multiply(x=w2586, y="N Acq Sets (Traps + Fl.)") -> (x*y=w2584:u32)
        n1062 = Divide(x=40000000.0, y=w2586) -> (x/y=w2578:dbl)
        "AI rate (Hz)" <- w2578
        "Ave. Rate (Hz)" <- w2578
        n1063 = Add Array Elements(numeric array=w2575) -> (sum=w2587:u32)
        "Trap Sets" <- w2587
        n1064 = Reciprocal(x=w2578) -> (1/x=→"Ave. Period (s)":dbl)
        n1065 = property on="Scan steps (AOD)" class="DigNum (strict)"("Val(Sgnl)"=w2597) -> ()  [unwired: 2 in, 2 out]
        n1066 = Divide(x=w2578, y="N Acq Sets (Traps + Fl.)") -> (x/y=w2601:dbl)
        "Data Rate (Hz)" <- w2601
        n1067 = Reciprocal(x=w2601) -> (1/x=→"Data Period (s)":dbl)
        n1068 = local read "Save ave N"() -> (w2600:dbl)
        n1069 = Divide(x=w2601, y=w2600) -> (x/y=w2599:dbl)
        "Save Data Rate (Hz)" <- w2599
        n1070 = Reciprocal(x=w2599) -> (1/x=→"Save Data Period (s)":dbl)
        n1071 = Multiply(x=w2584, y="# Samples/trap") -> (x*y=w2582:u32)
        "Counts/DMA" <- w2582
        n1072 = property on="Trap Disp. Downsample" class="DigNum (strict)"("Maximum"="# Samples/trap") -> ()  [unwired: 2 in, 2 out]
        n1073 = Multiply(x=w2587, y="# Samples/trap") -> (x*y=w2576:u32)
        "# Samples/channel" <- w2576
        n1074 = Multiply(x=w2576, y=u32 8) -> (x*y=→"Trap AI Elements/DMA read":u32)
        n1075 = local read "APD Int. Count"() -> (w2583:u32)
        n1076 = Multiply(x=w2576, y=u32 3) -> (x*y=→"Trap Pos Elements/DMA read":u32)
        n1077 = Divide(x=w2582, y=w2583) -> (x/y=w2573:dbl)
        "APD Samples/FIFO Acq." <- w2573
        n1078 = Divide(x=w2582, y=40000000.0) -> (x/y=w2580:dbl)
        "DMA Update Period (s)" <- w2580
        n1079 = Multiply(x=2.0, y=w2573) -> (x*y=→"APD Elements/DMA read":dbl)
        n1080 = property on="APD Disp. Downsample" class="DigNum (strict)"("Maximum"=w2573) -> ()  [unwired: 2 in, 2 out]
        n1081 = local read "N sets to save"() -> (w2593:u32)
        n1082 = Multiply(x=w2580, y=w2593) -> (x*y=→"Total Time (s)":dbl)
        "FPGA Averaging" <- FALSE ("FPGA Averaging")
      }
      event "Rescale on Mean": Value Change {
        n1083 = event-data() -> ()  [unwired: 7 out]
        n1084 = And(x=FALSE, y="Rescale on Mean") -> (x .and. y?=w2639:bool)
        n1085 = local write "Rescale on Mean"(w2639) -> ()
        n1086 = local read "Bead Mean (nm)"() -> (w2644:dbl)
        n1087 = Add(x="Amplitude (nm)", y=w2644) -> (x+y=w2642:dbl)
        n1088 = Subtract(x=w2644, y="Amplitude (nm)") -> (x-y=w2641:dbl)
        n1089 = property on="Bead Separation" class="WFChart (strict)"("YScale.Minimum"=w2641) -> ()  [unwired: 2 in, 2 out]
        n1090 = property on="Bead Separation" class="WFChart (strict)"("YScale.Maximum"=w2642) -> ()  [unwired: 2 in, 2 out]
      }
      event "Detector Type": Value Change {
        n1091 = event-data() -> ()  [unwired: 7 out]
        n1092 = local read "AI labels"() -> (w2645:string[])
        n1093 = property on="High Res. Display" class="Ring (strict)"("Strings []"=w2645) -> ()  [unwired: 2 in, 2 out]
        n1094 = Build Array (concatenate)(w2645, "none") -> (w2646:string[])
        n1095 = property on="FFT 1 Choice 1" class="Ring (strict)"("Strings []"=w2646) -> ()  [unwired: 2 in, 2 out]
        n1096 = property on="FFT 1 Choice 2" class="Ring (strict)"("Strings []"=w2646) -> ()  [unwired: 2 in, 2 out]
        n1097 = property on="FFT 2 Choice 1" class="Ring (strict)"("Strings []"=w2646) -> ()  [unwired: 2 in, 2 out]
        n1098 = property on="FFT 2 Choice 2" class="Ring (strict)"("Strings []"=w2646) -> ()  [unwired: 2 in, 2 out]
        n1099 = Bundle("APD 1", "APD 2") -> (w2649:cluster{string, string})  [unwired: 1 out]
        n1100 = Cluster To Array(cluster=w2649) -> (array=w2647:string[])
        n1101 = Build Array (concatenate)(w2647, w2646) -> (w2651:string[])
        n1102 = Array Size(array=w2651) -> (size(s)=w2652:i32)
        n1103 = property on="Signals to Plot" class="LstBox (strict)"("Item Names"=w2651) -> ()  [unwired: 2 in, 2 out]
        n1104 = property on="Signals to Plot" class="LstBox (strict)"("Number of Rows"=w2652) -> ()  [unwired: 2 in, 2 out]
        n1105 = property on="All Signals" class="WFChart (strict)"("LegNumRows"=w2652) -> ()  [unwired: 2 in, 2 out]
      }
      event "Adjust Scale\nto Mean": Value Change {
        n1106 = event-data() -> ()  [unwired: 7 out]
        n1107 = local read "APD 1 Rate (Hz)"() -> (w2661:dbl)
        n1108 = Multiply(x=1000.0, y="Above (kHz)") -> (x*y=w2659:dbl)
        n1109 = Multiply(x=1000.0, y="Below (kHz)") -> (x*y=w2657:dbl)
        n1110 = Add(x=w2659, y=w2661) -> (x+y=w2654:dbl)
        n1111 = Subtract(x=w2661, y=w2657) -> (x-y=w2655:dbl)
        n1112 = property on="APD Chart" class="WFChart (strict)"("YScale.Minimum"=w2655) -> ()  [unwired: 2 in, 2 out]
        n1113 = property on="APD Chart" class="WFChart (strict)"("YScale.Maximum"=w2654) -> ()  [unwired: 2 in, 2 out]
      }
      event "Phase adj. (AI1)", "+ phase (AI1)", "- phase (AI1)": Value Change {
        n1114 = event-data() -> ()  [unwired: 7 out]
        n1115 = Negate(x="Phase adj. (AI1)") -> (-x=w2671:i16)
        n1116 = Select(t=w2671, s="- phase (AI1)", f="Phase adj. (AI1)") -> (s? t:f=w2670:i16)
        n1117 = xnode "Read/Write Control"("FPGA VI Reference In"=w2674, "error in"=w2673, "Phase count adjustment"=w2670) -> ("FPGA VI Reference Out"=w2669:T19, "error out"=w2668:errorcluster)
        n1118 = Or(x="- phase (AI1)", y="+ phase (AI1)") -> (x .or. y?=w2665:bool)
        n1119 = xnode "Read/Write Control"("FPGA VI Reference In"=w2669, "error in"=w2668, "+ phase"=w2665) -> ("error out"=w2664:errorcluster)  [unwired: 1 out]
      }
      event "Signals to Plot": Double Click {
        w2719 = u32 9868950 ("Color Box")
        n1120 = event-data() -> ("Row"=w2721:i32)  [unwired: 9 out]
        n1121 = property on="All Signals" class="WFChart (strict)"("Active Plot"=w2721) -> (error out=w2732:errorcluster)  [unwired: 2 in, 1 out]
        n1122 = property on="All Signals" class="WFChart (strict)" props=["Plot", "Visible?", "Plot", "Plot Color"](error in=w2732) -> (error out=w2731:errorcluster, "Plot.Visible?"=w2730:bool)  [unwired: 1 in, 2 out]
        n1123 = Select(t=FALSE ("Plot.Visible"), s=w2730, f=TRUE ("Plot.Visible")) -> (s? t:f=w2725:bool)
        n1124 = property on="All Signals" class="WFChart (strict)"(error in=w2731, "Plot.Visible?"=w2725) -> (error out=w2727:errorcluster)  [unwired: 1 in, 1 out]
        n1125 = property on="All Signals" class="WFChart (strict)"(error in=w2727) -> (error out=w2722:errorcluster, "Plot.Plot Color"=w2726:u32)  [unwired: 1 in, 1 out]
        n1126 = property on="Signals to Plot" class="LstBox (strict)"(error in=w2722, "Active Row"=w2721) -> (error out=w2720:errorcluster)  [unwired: 1 in, 1 out]
        n1127 = Select(t=w2726, s=w2725, f=u32 0) -> (s? t:f=w2723:u32)
        n1128 = property on="Signals to Plot" class="LstBox (strict)"(error in=w2720, "CellFontColor"=w2723, "SelColor"=w2719, "CellBG"=w2719, "CellFontSize"=u32 20 ("Active Row:Cell Font:Size"), "CellFontBold"=TRUE ("Active Row:Cell Font:Bold")) -> ()  [unwired: 1 in, 2 out]
      }
      event "BD 1 Frequency 1 (MHz)", "BD 1 Frequency 2 (MHz)", "BD 1 Frequency 3 (MHz)", "BD 2 Frequency 1 (MHz)", "BD 2 Frequency 2 (MHz)", "BD 2 Frequency 3 (MHz)", "Trap Delta (MHz)": Value Change {
        n1129 = event-data() -> ("CtlRef"=w2735:refnum<vi>)  [unwired: 6 out]
        n1130 = control-ref of="Trap Delta (MHz)"() -> (w2734:refnum<vi>)
        n1131 = Equal?(x=w2734, y=w2735) -> (x = y?=w2733:bool)
        n1132 = case shown="False" "Oscillate Set 1" {
          tunnel: w2738 -> [w2758 _]
          tunnel: [w2757 w2761] -> w2737
          tunnel: w2736 -> [w2756 w2761]
          tunnel: w2733 -> [w2741 _]
          frame False {
            n1133 = local read "BD 1 Frequency 2 (MHz)"() -> (w2745:dbl)
            n1134 = local read "BD 1 Frequency 1 (MHz)"() -> (w2743:dbl)
            n1135 = Subtract(x=w2745, y="Trap Delta (MHz)") -> (x-y=w2742:dbl)
            n1136 = Select(t=w2742, s=w2741, f=w2743) -> (s? t:f=w2740:dbl)
            n1137 = local read "Y RF Frequency Limits (MHz)"() -> (w2746:T16)
            n1138 = local read "X RF Frequency Limits (MHz)"() -> (w2747:T16)
            n1139 = local read "BD 1 Frequency 3 (MHz)"() -> (w2759:dbl)
            n1140 = local write "BD 1 Frequency 1 (MHz)"(w2740) -> ()
            n1141 = local read "BD 2 Frequency 1 (MHz)"() -> (w2750:dbl)
            n1142 = local read "BD 2 Frequency 2 (MHz)"() -> (w2749:dbl)
            n1143 = local read "BD 2 Frequency 3 (MHz)"() -> (w2760:dbl)
            n1144 = call "set RF board frequency - interlace.vi"("Board 2 Frequency Limits"=w2746, "Board 1 Frequency Limits"=w2747, "error in"=w2756, "FPGA VI Reference In"=w2758, "Board 2 Frequency 3 (MHz)"=w2760, "Board 1 Frequency 3 (MHz)"=w2759, "Board 2 Frequency 2 (MHz)"=w2749, "Board 2 Frequency 1 (MHz)"=w2750, "Board 1 Frequency 2 (MHz)"=w2745, "Board 1 Frequency 1  (MHz)"=w2740) -> ("error out"=w2757:errorcluster)  [unwired: 1 out]
            n1145 = Subtract(x=w2750, y=w2749) -> (x-y=w2754:dbl)
            n1146 = Subtract(x=w2740, y=w2745) -> (x-y=w2755:dbl)
            n1147 = Square(x=w2754) -> (x^2=w2752:dbl)
            n1148 = Square(x=w2755) -> (x^2=w2753:dbl)
            n1149 = Add(x=w2753, y=w2752) -> (x+y=w2751:dbl)
            n1150 = Square Root(x=w2751) -> (sqrt(x)=w2748:dbl)
            n1151 = local write "Trap Delta (MHz)"(w2748) -> ()
            n1152 = property on="Initial delta (MHz)" class="DigNum (strict)"("Val(Sgnl)"=w2748) -> ()  [unwired: 2 in, 2 out]
          }
          frame True {
          }
        }
      }
      event "Round T1 X": Value Change {
        n1153 = event-data() -> ()  [unwired: 7 out]
        n1154 = local read "BD 1 Frequency 1 (MHz)"() -> (w2764:dbl)
        n1155 = Round To Nearest(number=w2764) -> (nearest integer value=w2763:dbl)
        n1156 = property on="BD 1 Frequency 1 (MHz)" class="DigNum (strict)"("Val(Sgnl)"=w2763) -> ()  [unwired: 2 in, 2 out]
      }
      event "Round T2 X": Value Change {
        n1157 = event-data() -> ()  [unwired: 7 out]
        n1158 = local read "BD 1 Frequency 2 (MHz)"() -> (w2766:dbl)
        n1159 = Round To Nearest(number=w2766) -> (nearest integer value=w2765:dbl)
        n1160 = property on="BD 1 Frequency 2 (MHz)" class="DigNum (strict)"("Val(Sgnl)"=w2765) -> ()  [unwired: 2 in, 2 out]
      }
      event "Stop All": Value Change {
        n1161 = event-data() -> ()  [unwired: 7 out]
        n1162 = local read "Stop All"() -> (w2768:bool)
      }
      event "Delayed Interlace Start": Value Change {
        n1163 = event-data() -> ()  [unwired: 7 out]
        n1164 = flat-sequence {
          frame #0 {
            n1165 = Multiply(x="Delay to Interlace (s)", y=1000.0) -> (x*y=w2771:dbl)
            n1166 = Wait (ms)(milliseconds to wait=w2771) -> ()  [unwired: 1 out]
          }
          frame #1 {
            n1167 = property on="Green laser mode" class="RadioBtnsControl (strict)"("Val(Sgnl)"=enum32{"Laser ON", "Laser OFF", "Interlace"}."Interlace" ("Value (Signaling)")) -> ()  [unwired: 2 in, 2 out]
          }
        }
      }
      event "BD 1 Amplitude 1 (%)", "BD 1 Amplitude 2 (%)", "BD 1 Amplitude 3 (%)", "BD 2 Amplitude 1 (%)", "BD 2 Amplitude 2 (%)", "BD 2 Amplitude 3 (%)", "Trap 1 ON", "Trap 2 ON", "Trap 3 ON", "Feedback On/Off", "All FB On/Off": Value Change {
        w2795 = i16 1 ("f")
        n1168 = event-data() -> ()  [unwired: 7 out]
        n1169 = local write "Trap 1 (ON/OFF)"("Trap 1 ON") -> ()
        n1170 = local write "Trap 2 (ON/OFF)"("Trap 2 ON") -> ()
        n1171 = Boolean To (0,1)(Boolean="Trap 3 ON") -> (0, 1=w2796:i16)
        n1172 = Boolean To (0,1)(Boolean="Trap 1 ON") -> (0, 1=w2797:i16)
        n1173 = Boolean To (0,1)(Boolean="Trap 2 ON") -> (0, 1=w2798:i16)
        n1174 = Select(t=w2798, s="Trap ON/OFF X or Y Amp?", f=w2795) -> (s? t:f=w2793:i16)
        n1175 = Select(t=w2797, s="Trap ON/OFF X or Y Amp?", f=w2795) -> (s? t:f=w2794:i16)
        n1176 = Select(t=w2796, s="Trap ON/OFF X or Y Amp?", f=w2795) -> (s? t:f=w2792:i16)
        n1177 = Select(t=w2795, s="Trap ON/OFF X or Y Amp?", f=w2798) -> (s? t:f=w2790:i16)
        n1178 = Select(t=w2795, s="Trap ON/OFF X or Y Amp?", f=w2797) -> (s? t:f=w2791:i16)
        n1179 = Select(t=w2795, s="Trap ON/OFF X or Y Amp?", f=w2796) -> (s? t:f=w2789:i16)
        n1180 = And(x="All FB On/Off", y="Feedback On/Off") -> (x .and. y?=w2787:cluster{"Set 1":bool, "Set 2":bool})
        n1181 = local read "BD 1 Amplitude 1 (%)"() -> (w2807:dbl)
        n1182 = local read "BD 1 Amplitude 2 (%)"() -> (w2806:dbl)
        n1183 = local read "BD 1 Amplitude 3 (%)"() -> (w2805:dbl)
        n1184 = Unbundle By Name(w2787) -> ("Set 1"=w2782:bool, "Set 2"=w2779:bool)
        n1185 = local read "Y RF Amplitude Limits (%)"() -> (w2775:T16)
        n1186 = local read "X RF Amplitude Limits (%)"() -> (w2776:T16)
        n1187 = local read "BD 2 Amplitude 1 (%)"() -> (w2808:dbl)
        n1188 = local read "BD 2 Amplitude 2 (%)"() -> (w2809:dbl)
        n1189 = local read "BD 2 Amplitude 3 (%)"() -> (w2810:dbl)
        n1190 = And(x="Trap 2 ON", y=w2779) -> (x .and. y?=w2777:bool)
        n1191 = And(x="Trap 1 ON", y=w2782) -> (x .and. y?=w2780:bool)
        n1192 = Multiply(x=w2794, y=w2807) -> (x*y=w2802:dbl)
        n1193 = Multiply(x=w2806, y=w2793) -> (x*y=w2800:dbl)
        n1194 = Multiply(x=w2805, y=w2792) -> (x*y=w2801:dbl)
        n1195 = Multiply(x=w2808, y=w2791) -> (x*y=w2811:dbl)
        n1196 = Multiply(x=w2809, y=w2790) -> (x*y=w2812:dbl)
        n1197 = Multiply(x=w2810, y=w2789) -> (x*y=w2813:dbl)
        n1198 = call "set RF board amplitude - interlace.vi"("Board 2 Amplitude Limits"=w2775, "Board 1 Amplitude Limits"=w2776, "error in"=w2803, "FPGA VI Reference In"=w2804, "Board 2 Amplitude 3 (%)"=w2813, "Board 1 Amplitude 3 (%)"=w2801, "Board 2 Amplitude 2 (%)"=w2812, "Board 2 Amplitude 1 (%)"=w2811, "Board 1 Amplitude 2 (%)"=w2800, "Board 1 Amplitude 1 (%)"=w2802) -> ("error out"=w2784:errorcluster, "FPGA VI Reference Out"=w2785:T19)
        n1199 = xnode "Read/Write Control"("FPGA VI Reference In"=w2785, "error in"=w2784, "FB On/Off Set 1"=w2780, "FB On/Off Set 2"=w2777) -> ("error out"=w2783:errorcluster)  [unwired: 1 out]
      }
      event "Load parameters": Value Change {
        n1200 = event-data() -> ()  [unwired: 7 out]
        n1201 = property on="Saved AOD Raster Scan Parameter Sets" class="Arr (strict)"() -> ("Index Values"=w2850:u32[])  [unwired: 2 in, 2 out]
        n1202 = Index Array(array=w2850, index=0) -> (element=w2847:u32)
        n1203 = local write "Load parameters"(FALSE ("Load parameters")) -> ()
        n1204 = Index Array(array="Saved AOD Raster Scan Parameter Sets", index=w2847) -> (element=w2846:T40)
        n1205 = Unbundle By Name(w2846) -> ("Scan Range AOD (nm) 2"=w2845:dbl, "Step Size AOD (nm) 2"=w2844:dbl, "Scan Speed AOD (nm/s) 2"=w2843:dbl, "Number of scans (AOD) 2"=w2842:u16)
        n1206 = flat-sequence {
          tunnel: w2845 -> [w2853]
          tunnel: w2844 -> [w2852]
          tunnel: w2843 -> [w2851]
          tunnel: w2842 -> [w2854]
          frame #0 {
            n1207 = local write "Scan Speed (nm/s)"(w2851) -> ()
            n1208 = local write "Scan Range (nm)"(w2853) -> ()
            n1209 = local write "Step Size (nm)"(w2852) -> ()
          }
          frame #1 {
            n1210 = property on="Number of F/B Scans (AOD)" class="DigNum (strict)"("Val(Sgnl)"=w2854) -> ()  [unwired: 2 in, 2 out]
          }
        }
      }
      event "Trap 1 (ON/OFF)", "Trap 2 (ON/OFF)": Value Change {
        n1211 = event-data() -> ()  [unwired: 7 out]
        n1212 = property on="Trap 2 ON" class="Bool (strict)"("Val(Sgnl)"="Trap 2 (ON/OFF)") -> ()  [unwired: 2 in, 2 out]
        n1213 = property on="Trap 1 ON" class="Bool (strict)"("Val(Sgnl)"="Trap 1 (ON/OFF)") -> ()  [unwired: 2 in, 2 out]
      }
      event "DIO count 1 (ticks)", "DIO count 2 (ticks)", "DIO count 3 (ticks)", "Interlace", "Number Interlace Sets", "Not-Interlacing Set": Value Change {
        n1214 = event-data() -> ()  [unwired: 7 out]
        n1215 = local read "DIO count 3 (ticks)"() -> (w2867:u32)
        n1216 = local read "DIO count 1 (ticks)"() -> (w2869:u32)
        n1217 = local read "DIO count 2 (ticks)"() -> (w2868:u32)
        n1218 = To Unsigned Byte Integer(number="Not-Interlacing Set") -> (unsigned 8bit integer=w2858:u8)
        n1219 = Add(x=w2858, y=u8 1) -> (x+y=w2862:u8)
        n1220 = xnode "Read/Write Control"("FPGA VI Reference In"=w2873, "error in"=w2871, "DIO count 1 (ticks)"=w2869, "DIO count 2 (ticks)"=w2868, "DIO count 3 (ticks)"=w2867, "Interlace ON/OFF"="Interlace", "Number Interlace Cycles"="Number Interlace Sets", "Interlace Off Parameters"=w2862) -> ("error out"=w2872:errorcluster)  [unwired: 1 out]
        n1221 = Build Array(w2869, w2868, w2867) -> (w2860:u32[])
        n1222 = Split 1D Array(array=w2860, index="Number Interlace Sets") -> (first subarray=w2870:u32[])  [unwired: 1 out]
        n1223 = Index Array(array=w2860, index=w2858) -> (element=w2859:u32)
        n1224 = Add Array Elements(numeric array=w2870) -> (sum=w2864:u32)
        n1225 = Select(t=w2864, s="Interlace", f=w2859) -> (s? t:f=→"Total Counts (ticks)":u32)
      }
      event "Reset Feedback": Value Change {
        n1226 = event-data() -> ()  [unwired: 7 out]
        n1227 = Unbundle By Name("Reset Feedback") -> ("Set 1"=w2923:bool, "Set 2"=w2922:bool)
        n1228 = xnode "Read/Write Control"("FPGA VI Reference In"=w2925, "error in"=w2920, "FB Reset Set 1"=w2923, "FB Reset Set 2"=w2922) -> ("error out"=w2921:errorcluster)  [unwired: 1 out]
      }
      event "PID Gains": Value Change {
        n1229 = event-data() -> ()  [unwired: 7 out]
        n1230 = Unbundle By Name("PID Gains") -> ("Set 1"=w2955:T14, "Set 2"=w2954:T14)
        n1231 = xnode "Read/Write Control"("FPGA VI Reference In"=w2956, "error in"=w2952, "FB Gains Set 1"=w2955, "FB Gains Set 2"=w2954) -> ("error out"=w2953:errorcluster)  [unwired: 1 out]
      }
      event "AI2 to Setpoint", "Setpoints (V)": Value Change {
        n1232 = event-data() -> ()  [unwired: 7 out]
        n1233 = xnode "Read/Write Control"("FPGA VI Reference In"=w2988, "error in"=w2984) -> ("FPGA VI Reference Out"=w2987:T19, "error out"=w2986:errorcluster, "AI2 Y Sum Set 1"=w2995, "AI2 Y Sum Set 2"=w2994)
        n1234 = Cluster To Array(cluster="AI2 to Setpoint") -> (array=w2998:bool[])
        n1235 = local read "AI2 (V)"() -> (w2996:cluster{"Set 1":dbl, "Set 2":dbl})
        n1236 = Or Array Elements(Boolean array=w2998) -> (logical OR=w2999:bool)
        n1237 = Bundle By Name(cluster=w2996, "Set 1"=w2995, "Set 2"=w2994) -> (w2993:cluster{"Set 1":dbl, "Set 2":dbl})
        n1238 = Divide(x=w2993, y=3276.7) -> (x/y=w2992:cluster{"Set 1":dbl, "Set 2":dbl})
        "AI2 (V)" <- w2992
        n1239 = case shown="True" w2999 {
          tunnel: [w3028 w3045] -> w2991
          tunnel: "AI2 to Setpoint" -> [_ w3041]
          tunnel: "Setpoints (V)" -> [w3029 w3044]
          tunnel: w2992 -> [_ w3038]
          frame False {
            n1240 = Multiply(x=3276.7, y=w3029) -> (x*y=w3030:cluster{"Set 1":dbl, "Set 2":dbl})
            n1241 = To Word Integer(number=w3030) -> (16bit integer=w3028:cluster{"Set 1":i16, "Set 2":i16})
          }
          frame True {
            n1242 = Unbundle By Name(w3038) -> ("Set 1"=w3037:dbl, "Set 2"=w3036:dbl)
            n1243 = Unbundle By Name(w3044) -> ("Set 1"=w3043:dbl, "Set 2"=w3042:dbl)
            n1244 = Unbundle By Name(w3041) -> ("Set 1"=w3040:bool, "Set 2"=w3039:bool)
            n1245 = Select(t=w3037, s=w3040, f=w3043) -> (s? t:f=w3035:dbl)
            n1246 = Select(t=w3036, s=w3039, f=w3042) -> (s? t:f=w3034:dbl)
            n1247 = Bundle By Name(cluster=w3044, "Set 1"=w3035, "Set 2"=w3034) -> (w3032:cluster{"Set 1":dbl, "Set 2":dbl})
            n1248 = local write "Setpoints (V)"(w3032) -> ()
            n1249 = Multiply(x=3276.7, y=w3032) -> (x*y=w3033:cluster{"Set 1":dbl, "Set 2":dbl})
            n1250 = To Word Integer(number=w3033) -> (16bit integer=w3045:cluster{"Set 1":i16, "Set 2":i16})
          }
        }
        n1251 = Unbundle By Name(w2991) -> ("Set 1"=w2990:i16, "Set 2"=w2989:i16)
        n1252 = xnode "Read/Write Control"("FPGA VI Reference In"=w2987, "error in"=w2986, "FB Setpoint Set 1"=w2990, "FB Setpoint Set 2"=w2989) -> ("error out"=w2985:errorcluster)  [unwired: 1 out]
      }
      event "Invert GI": Value Change {
        n1253 = event-data() -> ()  [unwired: 7 out]
        n1254 = xnode "Read/Write Control"("FPGA VI Reference In"=w3076, "error in"=w3074, "Invert GI"="Invert GI", "Invert GI 2"="Invert GI") -> ("error out"=w3075:errorcluster)  [unwired: 1 out]
      }
      event "Green FB Setpoint (mV)", "Green FB Gains", "Green FB On/Off", "Current When FB OFF (%)", "Green int current ON count adj": Value Change {
        n1255 = event-data() -> ()  [unwired: 7 out]
        n1256 = local read "Green FB Setpoint (mV)"() -> (w3109:dbl)
        n1257 = local read "Current When FB OFF (%)"() -> (w3112:dbl)
        n1258 = Multiply(x=w3109, y=3.2767) -> (x*y=w3108:dbl)
        n1259 = Multiply(x=w3112, y=655.35) -> (x*y=w3113:dbl)
        n1260 = To Unsigned Word Integer(number=w3113) -> (unsigned 16bit integer=w3111:u16)
        n1261 = local read "Green int current ON count adj"() -> (w3116:u32)
        n1262 = local read "Green FB Gains"() -> (w3115:T14)
        n1263 = local read "Green Laser ON/Interlacing"() -> (w3106:bool)
        n1264 = local read "Green laser mode"() -> (w3105:enum32{"Laser ON", "Laser OFF", "Interlace"})
        n1265 = local read "Green FB On/Off"() -> (w3117:bool)
        n1266 = Equal?(x=w3105, y=enum32{"Laser ON", "Laser OFF", "Interlace"}."Interlace") -> (x = y?=w3103:bool)
        n1267 = Compound Arithmetic op=AND(w3103, w3117, w3106) -> (w3107:bool)
        n1268 = xnode "Read/Write Control"("FPGA VI Reference In"=w3120, "error in"=w3119, "Green FB Setpoint"=w3108, "Green FB On/Off"=w3107, "Current Out"=w3111, "Green int current ON count adj"=w3116, "Green FB Gains"=w3115) -> ("error out"=w3118:errorcluster)  [unwired: 1 out]
      }
      event "Green laser mode", "Green Laser ON/Interlacing": Value Change {
        n1269 = event-data() -> ()  [unwired: 7 out]
        n1270 = case shown="True" "Green Laser ON/Interlacing" {
          tunnel: "Green laser mode" -> [_ w3175]
          tunnel: [enum32{"Laser ON", "Laser OFF", "Interlace"}."Laser OFF" ("Green laser mode") w3175] -> w3163
          tunnel: [FALSE w3171] -> w3162
          frame False {
          }
          frame True {
            n1271 = local read "Green FB On/Off"() -> (w3172:bool)
            n1272 = Equal?(x=w3175, y=enum32{"Laser ON", "Laser OFF", "Interlace"}."Interlace") -> (x = y?=w3173:bool)
            n1273 = And(x=w3173, y=w3172) -> (x .and. y?=w3171:bool)
          }
        }
        n1274 = xnode "Read/Write Control"("FPGA VI Reference In"=w3168, "error in"=w3166, "Operating Mode"=w3163, "Operating Mode 2"=w3163, "Green FB On/Off"=w3162) -> ("error out"=w3167:errorcluster)  [unwired: 1 out]
      }
      event "- phase (APD 1 Gate)", "+ phase (APD 1 Gate)": Value Change {
        n1275 = event-data() -> ()  [unwired: 7 out]
        n1276 = local read "Phase Adj. (APD 1 Gate)"() -> (w3207:i16)
        n1277 = Negate(x=w3207) -> (-x=w3215:i16)
        n1278 = Select(t=w3215, s="- phase (APD 1 Gate)", f=w3207) -> (s? t:f=w3214:i16)
        n1279 = Or(x="- phase (APD 1 Gate)", y="+ phase (APD 1 Gate)") -> (x .or. y?=w3210:bool)
        n1280 = xnode "Read/Write Control"("FPGA VI Reference In"=w3217, "error in"=w3216, "Phase count adjustment (APD 1 Gate)"=w3214) -> ("FPGA VI Reference Out"=w3212:T19, "error out"=w3213:errorcluster)
        n1281 = xnode "Read/Write Control"("FPGA VI Reference In"=w3212, "error in"=w3213, "+ phase (APD 1 Gate)"=w3210) -> ("error out"=w3211:errorcluster)  [unwired: 1 out]
      }
      event "+ phase (APD 2 Gate)", "- phase (APD 2 Gate)": Value Change {
        n1282 = event-data() -> ()  [unwired: 7 out]
        n1283 = local read "Phase Adj. (APD 2 Gate)"() -> (w3260:i16)
        n1284 = Negate(x=w3260) -> (-x=w3268:i16)
        n1285 = Select(t=w3268, s="- phase (APD 2 Gate)", f=w3260) -> (s? t:f=w3267:i16)
        n1286 = Or(x="- phase (APD 2 Gate)", y="+ phase (APD 2 Gate)") -> (x .or. y?=w3263:bool)
        n1287 = xnode "Read/Write Control"("FPGA VI Reference In"=w3270, "error in"=w3269, "Phase count adjustment (APD 2 Gate)"=w3267) -> ("FPGA VI Reference Out"=w3265:T19, "error out"=w3266:errorcluster)
        n1288 = xnode "Read/Write Control"("FPGA VI Reference In"=w3265, "error in"=w3266, "+ phase (APD 2 Gate)"=w3263) -> ("error out"=w3264:errorcluster)  [unwired: 1 out]
      }
      event "Phase Adj. (APD Acq)", "+ phase (APD Acq)", "- phase (APD Acq)": Value Change {
        n1289 = event-data() -> ()  [unwired: 7 out]
        n1290 = local read "Phase Adj. (APD Acq)"() -> (w3315:i16)
        n1291 = Negate(x=w3315) -> (-x=w3321:i16)
        n1292 = Select(t=w3321, s="+ phase (APD Acq)", f=w3315) -> (s? t:f=w3320:i16)
        n1293 = Or(x="+ phase (APD Acq)", y="- phase (APD Acq)") -> (x .or. y?=w3316:bool)
        n1294 = xnode "Read/Write Control"("FPGA VI Reference In"=w3323, "error in"=w3322, "Phase Count Adjustment (APD Acq)"=w3320) -> ("FPGA VI Reference Out"=w3318:T19, "error out"=w3319:errorcluster)
        n1295 = xnode "Read/Write Control"("FPGA VI Reference In"=w3318, "error in"=w3319, "+ phase (APD Acq)"=w3316) -> ("error out"=w3317:errorcluster)  [unwired: 1 out]
      }
      event "Phase adj. (GI)", "+ phase (GI)", "- phase (GI)": Value Change {
        n1296 = event-data() -> ()  [unwired: 7 out]
        n1297 = Negate(x="Phase adj. (GI)") -> (-x=w3374:i16)
        n1298 = Select(t=w3374, s="+ phase (GI)", f="Phase adj. (GI)") -> (s? t:f=w3373:i16)
        n1299 = Or(x="+ phase (GI)", y="- phase (GI)") -> (x .or. y?=w3369:bool)
        n1300 = xnode "Read/Write Control"("FPGA VI Reference In"=w3376, "error in"=w3375, "Phase count adjustment (GI)"=w3373) -> ("FPGA VI Reference Out"=w3371:T19, "error out"=w3372:errorcluster)
        n1301 = xnode "Read/Write Control"("FPGA VI Reference In"=w3371, "error in"=w3372, "+ phase (GI)"=w3369) -> ("error out"=w3370:errorcluster)  [unwired: 1 out]
      }
      event "Phase adj. (GI) 2", "+ phase (GI) 2", "- phase (GI) 2": Value Change {
        n1302 = event-data() -> ()  [unwired: 7 out]
        n1303 = Negate(x="Phase adj. (GI) 2") -> (-x=w3427:i16)
        n1304 = Select(t=w3427, s="+ phase (GI) 2", f="Phase adj. (GI) 2") -> (s? t:f=w3426:i16)
        n1305 = Or(x="+ phase (GI) 2", y="- phase (GI) 2") -> (x .or. y?=w3422:bool)
        n1306 = xnode "Read/Write Control"("FPGA VI Reference In"=w3429, "error in"=w3428, "Phase count adjustment (GI) 2"=w3426) -> ("FPGA VI Reference Out"=w3424:T19, "error out"=w3425:errorcluster)
        n1307 = xnode "Read/Write Control"("FPGA VI Reference In"=w3424, "error in"=w3425, "+ phase (GI) 2"=w3422) -> ("error out"=w3423:errorcluster)  [unwired: 1 out]
      }
      event "Phase adj. (Green FB)", "- phase (Green FB)", "+ phase (Green FB)": Value Change {
        n1308 = event-data() -> ()  [unwired: 7 out]
        n1309 = Negate(x="Phase adj. (Green FB)") -> (-x=w3480:i16)
        n1310 = Select(t=w3480, s="+ phase (Green FB)", f="Phase adj. (Green FB)") -> (s? t:f=w3479:i16)
        n1311 = Or(x="+ phase (Green FB)", y="- phase (Green FB)") -> (x .or. y?=w3475:bool)
        n1312 = xnode "Read/Write Control"("FPGA VI Reference In"=w3482, "error in"=w3481, "Phase count adjustment (Green FB)"=w3479) -> ("FPGA VI Reference Out"=w3477:T19, "error out"=w3478:errorcluster)
        n1313 = xnode "Read/Write Control"("FPGA VI Reference In"=w3477, "error in"=w3478, "+ phase (Green FB)"=w3475) -> ("error out"=w3476:errorcluster)  [unwired: 1 out]
      }
      event "Invert APD Gate", "APD Gate ON Count", "APD Gate OFF Count", "APD Gate", "APD Integration Time (s)", "APD 1 AO Mult.", "APD 2 AO Mult.": Value Change {
        n1314 = event-data() -> ()  [unwired: 7 out]
        n1315 = local read "APD Integration Time (s)"() -> (w3525:dbl)
        n1316 = local read "APD Gate ON Count"() -> (w3538:u32)
        n1317 = local read "APD Gate OFF Count"() -> (w3537:u32)
        n1318 = local read "Invert APD Gate"() -> (w3539:bool)
        n1319 = local read "APD Gate"() -> (w3536:enum32{"ON", "OFF", "Interlace"})
        n1320 = Multiply(x=w3525, y=40000000.0) -> (x*y=w3534:dbl)
        n1321 = Reciprocal(x=w3525) -> (1/x=→"APD Acq Rate (Hz)":dbl)
        n1322 = To Unsigned Long Integer(number=w3534) -> (unsigned 32bit integer=w3533:u32)
        n1323 = local read "DMA Update Period (s)"() -> (w3526:dbl)
        n1324 = Divide(x=w3526, y=w3525) -> (x/y=w3529:dbl)
        n1325 = local read "APD 1 AO Mult."() -> (w3531:i16)
        n1326 = local read "APD 2 AO Mult."() -> (w3530:i16)
        n1327 = Multiply(x=2.0, y=w3529) -> (x*y=w3528:dbl)
        n1328 = local write "APD Samples/FIFO Acq."(w3529) -> ()
        n1329 = local write "APD Elements/DMA read"(w3528) -> ()
        n1330 = xnode "Read/Write Control"("FPGA VI Reference In"=w3542, "error in"=w3541, "Invert APD Gate"=w3539, "APD Gate ON Count"=w3538, "APD Gate OFF Count"=w3537, "APD Acq Rate Count"=w3533, "APD Gate Operating Mode"=w3536, "APD 1 AO scale factor"=w3531, "APD 2 AO scale factor"=w3530) -> ("error out"=w3540:errorcluster)  [unwired: 1 out]
      }
      event "GI Frequency, ON count", "Green FB Count", "GI Frequency, OFF count": Value Change {
        n1331 = event-data() -> ()  [unwired: 7 out]
        n1332 = xnode "Read/Write Control"("FPGA VI Reference In"=w3599, "error in"=w3597, "Green interlace ON count"="GI Frequency, ON count", "Green interlace OFF count"="GI Frequency, OFF count", "Green interlace ON count 2"="GI Frequency, ON count", "Green interlace OFF count 2"="GI Frequency, OFF count", "Green FB Count"="Green FB Count") -> ("error out"=w3598:errorcluster)  [unwired: 1 out]
      }
      event "Number of F/B Scans (AOD)", "Scan Speed (nm/s)", "Scan BD", "Initial delta (MHz)", "Step Size (nm)", "Scan Range (nm)": Value Change {
        w3702 = 123.0  # AOM cal (nm/MHz)
        n1333 = event-data() -> ()  [unwired: 7 out]
        n1334 = local read "BD 1 Frequency 1 (MHz)"() -> (w3685:dbl)
        n1335 = local read "AOM X Cal (nm/MHz)"() -> (w3677:dbl)
        n1336 = local read "X RF Frequency Limits (MHz)"() -> (w3689:T16)
        n1337 = local read "Y RF Frequency Limits (MHz)"() -> (w3686:T16)
        n1338 = local read "BD 2 Frequency 1 (MHz)"() -> (w3691:dbl)
        n1339 = Negate(x="Scan Range (nm)") -> (-x=w3655:dbl)
        n1340 = Divide(x=w3655, y=w3677) -> (x/y=w3659:dbl)
        n1341 = Select(t=w3689, s="Scan BD", f=w3686) -> (s? t:f=w3688:T16)
        n1342 = Select(t=w3685, s="Scan BD", f=w3691) -> (s? t:f=w3690:dbl)
        n1343 = Unbundle By Name(w3688) -> ("Maximum"=w3697:dbl, "Minimum"=w3696:dbl)
        n1344 = Add(x=w3659, y=w3690) -> (x+y=w3694:dbl)
        n1345 = Divide(x=w3655, y="Step Size (nm)") -> (x/y=w3674:dbl)
        n1346 = Divide(x="Step Size (nm)", y=w3677) -> (x/y=w3683:dbl)
        n1347 = Absolute Value(x=w3674) -> (abs(x)=w3658:dbl)
        n1348 = Sign(1:w3655) -> (0:w3656:dbl)
        n1349 = In Range and Coerce(upper limit=w3697, x=w3694, lower limit=w3696) -> (coerced(x)=w3693:dbl, In Range?=w3695:bool)
        n1350 = To Unsigned Quad Integer(1:w3658) -> (0:w3673:u64)
        "Scan steps (AOD)" <- w3673
        n1351 = call "IR AOM freq to word.vi"("Frequency In (MHz)"=w3683) -> ("Frequency Word Out (double)"=w3680:dbl)
        n1352 = Multiply(x=w3656, y=w3680) -> (x*y=w3657:dbl)
        n1353 = Subtract(x=w3694, y=w3693) -> (x-y=w3692:dbl)
        n1354 = To Quad Integer(1:w3657) -> (0:w3679:i64)
        "Incr. int (AOD)" <- w3679
        n1355 = Subtract(x=w3659, y=w3692) -> (x-y=w3678:dbl)
        "Scan Range (MHz)" <- w3678
        n1356 = Select(t=w3659, s=w3695, f=w3678) -> (s? t:f=w3698:dbl)
        n1357 = Multiply(x=w3678, y=w3677) -> (x*y=w3676:dbl)
        n1358 = Decrement(x=w3673) -> (x-1=w3726:u64)
        n1359 = Negate(x=w3676) -> (-x=w3672:dbl)
        n1360 = local write "Scan Range (nm)"(w3672) -> ()
        n1361 = Divide(x=w3698, y=w3726) -> (x/y=w3682:dbl)
        "Scan Increment (MHz)" <- w3682
        n1362 = call "IR AOM freq to word.vi"("Frequency In (MHz)"=w3682) -> ("Frequency Word Out (double)"=w3681:dbl)
        n1363 = Divide(x="Step Size (nm)", y="Scan Speed (nm/s)") -> (x/y=w3669:dbl)
        n1364 = To Quad Integer(1:w3681) -> ()  [unwired: 1 out]
        n1365 = local read "Number Interlace Sets"() -> (w3653:u8)
        n1366 = local read "AI Count (ticks)"() -> (w3654:u32)
        n1367 = local read "Total Counts (ticks)"() -> (w3652:u32)
        n1368 = local read "# Samples/trap"() -> (w3684:u32)
        n1369 = Multiply(x=w3654, y=w3653) -> (x*y=w3651:u32)
        n1370 = Divide(x=w3652, y=w3651) -> (x/y=w3650:dbl)
        n1371 = Select(t=w3685, s="Scan BD", f=w3691) -> (s? t:f=w3723:dbl)
        "Initial freq. (MHz)" <- w3723
        n1372 = Add(x=w3698, y=w3723) -> (x+y=→"Final freq. (MHz)":dbl)
        n1373 = Divide(x=w3652, y=40000000.0) -> (x/y=w3668:dbl)
        n1374 = Divide(x=w3669, y=w3668) -> (x/y=w3667:dbl)
        n1375 = To Unsigned Quad Integer(1:w3667) -> (0:w3642:u64)
        n1376 = Quotient & Remainder(x=w3642, y=u64 2) -> (x-y*floor(x/y)=w3646:u64)  [unwired: 1 out]
        n1377 = Equal?(x=w3646, y=u64 0) -> (x = y?=w3644:bool)
        n1378 = Decrement(x=w3642) -> (x-1=w3643:u64)
        n1379 = Select(t=w3642, s=w3644, f=w3643) -> (s? t:f=w3641:u64)
        "Cycles/step (AOD)" <- w3641
        n1380 = xnode "Read/Write Control"("FPGA VI Reference In"=w3734, "error in"=w3733, "Scan steps"=w3673, "Number of scans"="Number of F/B Scans (AOD)", "Cycles per step"=w3641, "Scan freq.  increment"=w3679, "Scan BD"="Scan BD") -> ("error out"=w3732:errorcluster)  [unwired: 1 out]
        n1381 = Multiply(x=w3673, y=w3641) -> (x*y=w3727:u64)
        n1382 = Multiply(x=w3727, y=u64 2) -> (x*y=w3649:u64)
        n1383 = Multiply(x=w3650, y=w3649) -> (x*y=w3648:dbl)
        "Data points/scan (f/b)" <- w3648
        n1384 = Multiply(x=w3648, y="Number of F/B Scans (AOD)") -> (x*y=w3730:dbl)
        "Data points/scans" <- w3730
        n1385 = Divide(x=w3730, y=w3684) -> (x/y=→"N sets should be saved":dbl)
        n1386 = Multiply(x=w3727, y=w3668) -> (x*y=w3666:dbl)
        "Time/Scan (s) (AOD)" <- w3666
        n1387 = Select(t=w3698, s="Scan BD", f=0.0) -> (s? t:f=w3724:dbl)
        n1388 = Select(t=0.0, s="Scan BD", f=w3698) -> (s? t:f=w3720:dbl)
        n1389 = local read "BD 2 Frequency 2 (MHz)"() -> (w3716:dbl)
        n1390 = local read "BD 1 Frequency 2 (MHz)"() -> (w3719:dbl)
        n1391 = Add(x=w3720, y=w3691) -> (x+y=w3717:dbl)
        n1392 = Add(x=w3685, y=w3724) -> (x+y=w3718:dbl)
        n1393 = Multiply(x=w3666, y=2.0) -> (x*y=w3665:dbl)
        n1394 = Multiply(x=w3665, y="Number of F/B Scans (AOD)") -> (x*y=w3662:dbl)
        n1395 = Divide(x=w3662, y=60.0) -> (x/y=→"Time to Finish All (min)":dbl)
        n1396 = Add(x="Trap 2 Bead Size (nm)", y="Trap 1 Bead Size (nm)") -> (x+y=w3706:dbl)
        n1397 = Divide(x=w3706, y=2.0) -> (x/y=w3700:dbl)
        n1398 = local read "Initial delta (MHz)"() -> (w3703:dbl)
        n1399 = Subtract(x=w3717, y=w3716) -> (x-y=w3714:dbl)
        n1400 = Subtract(x=w3718, y=w3719) -> (x-y=w3715:dbl)
        n1401 = Square(x=w3714) -> (x^2=w3713:dbl)
        n1402 = Square(x=w3715) -> (x^2=w3712:dbl)
        n1403 = Add(x=w3712, y=w3713) -> (x+y=w3711:dbl)
        n1404 = Square Root(x=w3711) -> (sqrt(x)=w3710:dbl)
        "Final delta (MHz)" <- w3710
        n1405 = Multiply(x=w3702, y=w3710) -> (x*y=w3709:dbl)
        n1406 = Multiply(x=w3703, y=w3702) -> (x*y=w3701:dbl)
        n1407 = Subtract(x=w3701, y=w3700) -> (x-y=→"Initial sep (nm)":dbl)
        n1408 = Subtract(x=w3709, y=w3700) -> (x-y=→"Final sep (nm)":dbl)
      }
      event "Freq or Amp switch first", "Swap F1 and F2", "Freq switch delay", "Amp switch delay": Value Change {
        n1409 = event-data() -> ()  [unwired: 7 out]
        n1410 = local read "Freq or Amp switch first"() -> (w3776:bool)
        n1411 = local read "Amp switch delay"() -> (w3777:u16)
        n1412 = local read "Freq switch delay"() -> (w3779:u16)
        n1413 = local read "Swap F1 and F2"() -> (w3778:bool)
        n1414 = xnode "Read/Write Control"("FPGA VI Reference In"=w3782, "error in"=w3781, "Freq switch delay"=w3779, "Swap F1 and F2"=w3778, "Amp switch delay"=w3777, "Freq or Amp switch first"=w3776) -> ("error out"=w3780:errorcluster)  [unwired: 1 out]
      }
      event "Scan steps (MCL)", "Number of scans (MCL)", "Scan Range (V)\n(of steps)", "2D or 1D Scan", "N APD Samp/step", "Fast Scan Dir", "Continuous MCL Scanning", "Scan lines (y)": Value Change {
        w3820 = 32767.0 ("y")
        n1415 = event-data() -> ()  [unwired: 7 out]
        n1416 = Select(t="Scan lines (y)", s="2D or 1D Scan", f="Number of scans (MCL)") -> (s? t:f=w3825:u64)
        n1417 = Decrement(x="Scan steps (MCL)") -> (x-1=w3841:u64)
        n1418 = Divide(x="Scan Range (V)\n(of steps)", y=w3841) -> (x/y=w3840:dbl)
        "Desired Scan Incr (V)" <- w3840
        n1419 = local read "APD Integration Time (s)"() -> (w3833:dbl)
        n1420 = Multiply(x=w3840, y=w3820) -> (x*y=w3849:dbl)
        n1421 = Divide(x=w3849, y=10.0) -> (x/y=w3839:dbl)
        "Desired incr (int)" <- w3839
        n1422 = local read "Update Count (MCL)"() -> (w3845:u32)
        n1423 = Round Toward -Infinity(1:w3839) -> (0:w3848:dbl)
        n1424 = To Word Integer(number=w3848) -> (16bit integer=w3823:i16)
        "Actual Incr. int (MCL)" <- w3823
        n1425 = Multiply(x=w3833, y=40000000.0) -> (x*y=w3846:dbl)
        n1426 = Divide(x=w3846, y=w3845) -> (x/y=w3844:dbl)
        n1427 = Multiply(x=i16 10, y=w3823) -> (x*y=w3821:i16)
        n1428 = Multiply(x="N APD Samp/step", y=w3844) -> (x*y=w3843:dbl)
        "Cycles/step (MCL)" <- w3843
        n1429 = Divide(x=w3821, y=w3820) -> (x/y=→"Actual MCL Inc (V)":dbl)
        n1430 = Multiply(x="N APD Samp/step", y="Scan steps (MCL)") -> (x*y=w3835:dbl)
        n1431 = local read "APD Samples/FIFO Acq."() -> (w3832:dbl)
        n1432 = Multiply(x=w3835, y=u64 2) -> (x*y=w3834:dbl)
        "Data points/scan (f+b)" <- w3834
        n1433 = Multiply(x=w3834, y=w3825) -> (x*y=w3852:dbl)
        "Data points/scans (MCL)" <- w3852
        n1434 = Multiply(x=w3833, y=w3834) -> (x*y=w3826:dbl)
        "Time/f+b scan (s) (MCL)" <- w3826
        n1435 = Divide(x=w3852, y=w3832) -> (x/y=→"N sets should be saved (MCL)":dbl)
        n1436 = Multiply(x=w3826, y=w3825) -> (x*y=→"Total Time (s)":dbl)
        n1437 = Not(x="Fast Scan Dir") -> (.not. x?=w3830:bool)
        n1438 = xnode "Read/Write Control"("FPGA VI Reference In"=w3856, "error in"=w3855, "Scan steps (MCL)"="Scan steps (MCL)", "Number of scans (MCL)"=w3825, "Cycles per step (MCL)"=w3843, "Scan freq.  increment (MCL)"=w3823, "1D or 2D Scan?"="2D or 1D Scan", "MCL Scan Axis"=w3830, "Cont. Scan (MCL)"="Continuous MCL Scanning") -> ("error out"=w3854:errorcluster)  [unwired: 1 out]
      }
      event "Read Cal": Value Change {
        w3909 = 1000.0 ("y")
        n1439 = event-data() -> ()  [unwired: 7 out]
        n1440 = local read "Save file name"() -> (w3934:path)
        n1441 = local write "Read Cal"(FALSE ("Read Cal")) -> ()
        n1442 = Strip Path(path=w3934) -> (stripped path=w3933:path)  [unwired: 1 out]
        n1443 = Path To String(path=w3933) -> (string=w3932:string)
        n1444 = Concatenate Strings(w3932, "\\current.cal" ("string")) -> (w3930:string)
        n1445 = String To Path(string=w3930) -> (path=w3929:path)
        n1446 = Open/Create/Replace File(file path (use dialog)=w3929, operation (0:open)=T32."open", access (0:read/write)=enum16{"read/write", "read-only", "write-only"}."read-only") -> (refnum out=w3937:refnum<file>, error out=w3923:errorcluster)  [unwired: 1 in, 3 out]
        n1447 = Deny Access(4:w3923, 7:w3937) -> (0:w3922:errorcluster, 3:w3928:refnum<file>)  [unwired: 1 out]
        n1448 = Read from Binary File(5:0.0, 8:w3922, 9:T33."big-endian, network order" ("byte order (0:big-endian, network order)"), 10:-1 ("count (1)"), 11:w3928) -> (0:w3921:errorcluster, 2:w3919:dbl[], 3:w3924:refnum<file>)  [unwired: 2 out]
        n1449 = Array To Cluster(array=w3919) -> (cluster=w3918:T41)
        n1450 = Unbundle(w3918) -> ("[0]"=w3917:dbl, "[1]"=w3916:dbl, "[2]"=w3915:dbl, "[3]"=w3914:dbl, "[4]"=w3913:dbl, "[5]"=w3912:dbl)
        n1451 = Close File(refnum=w3924, error in=w3921) -> (error out=→"Read cal error":errorcluster)  [unwired: 1 out]
        n1452 = Multiply(x=w3912, y=w3909) -> (x*y=w3910:dbl)
        n1453 = local write "T2 kappa_x (pN/nm)"(w3914) -> ()
        n1454 = local write "T1 kappa_x (pN/nm)"(w3915) -> ()
        n1455 = local write "T1 alpha_x (nm/V)"(w3917) -> ()
        n1456 = local write "T2 alpha_x (nm/V)"(w3916) -> ()
        n1457 = Multiply(x=w3913, y=w3909) -> (x*y=w3911:dbl)
        n1458 = local write "T1 offset_x (mV)"(w3911) -> ()
        n1459 = local write "T2 offset_x (mV)"(w3910) -> ()
      }
      event "Abort MCL Scan": Value Change {
        n1460 = event-data() -> ()  [unwired: 7 out]
        n1461 = local write "MCL Scanning"(FALSE ("MCL Scanning")) -> ()
        n1462 = xnode "Read/Write Control"("FPGA VI Reference In"=w3942, "error in"=w3941, "Abort scan (MCL)"="Abort MCL Scan") -> ("error out"=w3940:errorcluster)  [unwired: 1 out]
      }
      event "Update Count (MCL)": Value Change {
        n1463 = event-data() -> ()  [unwired: 7 out]
        n1464 = xnode "Read/Write Control"("FPGA VI Reference In"=w3967, "error in"=w3966, "MCL count"="Update Count (MCL)") -> ("error out"=w3965:errorcluster)  [unwired: 1 out]
      }
      event "Phase adjust (MCL)", "+ phase (MCL)", "- phase (MCL)": Value Change {
        n1465 = event-data() -> ()  [unwired: 7 out]
        n1466 = Negate(x="Phase adjust (MCL)") -> (-x=w3997:i16)
        n1467 = Select(t=w3997, s="- phase (MCL)", f="Phase adjust (MCL)") -> (s? t:f=w3995:i16)
        n1468 = Or(x="- phase (MCL)", y="+ phase (MCL)") -> (x .or. y?=w3990:bool)
        n1469 = xnode "Read/Write Control"("FPGA VI Reference In"=w3999, "error in"=w3998, "Phase count adjustment (MCL)"=w3995) -> ("FPGA VI Reference Out"=w3991:T19, "error out"=w3992:errorcluster)
        n1470 = xnode "Read/Write Control"("FPGA VI Reference In"=w3991, "error in"=w3992, "+ phase (MCL)"=w3990) -> ("error out"=w3989:errorcluster)  [unwired: 1 out]
      }
      event "Abort AOD Scan": Value Change {
        n1471 = event-data() -> ()  [unwired: 7 out]
        n1472 = xnode "Read/Write Control"("FPGA VI Reference In"=w4045, "error in"=w4044, "Abort scan"="Abort AOD Scan") -> ("error out"=w4043:errorcluster)  [unwired: 1 out]
      }
      event "Continuous AOD Scanning": Value Change {
        n1473 = event-data() -> ()  [unwired: 7 out]
        n1474 = xnode "Read/Write Control"("FPGA VI Reference In"=w4070, "error in"=w4069, "Cont. Scan"="Continuous AOD Scanning") -> ("error out"=w4068:errorcluster)  [unwired: 1 out]
      }
      event "Index": Value Change {
        n1475 = event-data() -> ()  [unwired: 7 out]
        n1476 = call "Create new save file.vi"("Insert"="", "Ext"=".dat" ("string"), "Index In"="Index") -> ("Path Out"=→"Save file name":path, "Index Out"=w4092:dbl)
        "Save index" <- w4092
        n1477 = local write "Index"(w4092) -> ()
      }
      event "AO1", "AO2": Value Change {
        w4107 = 10.0 ("y")
        w4106 = 32767.0 ("y")
        n1478 = event-data() -> ()  [unwired: 7 out]
        n1479 = local read "AO2"() -> (w4105:dbl)
        n1480 = local read "AO1"() -> (w4102:dbl)
        n1481 = Multiply(x=w4102, y=w4106) -> (x*y=w4101:dbl)
        n1482 = Multiply(x=w4105, y=w4106) -> (x*y=w4104:dbl)
        n1483 = Divide(x=w4101, y=w4107) -> (x/y=w4100:dbl)
        n1484 = Divide(x=w4104, y=w4107) -> (x/y=w4103:dbl)
        n1485 = To Word Integer(number=w4100) -> (16bit integer=w4108:i16)
        n1486 = To Word Integer(number=w4103) -> (16bit integer=w4109:i16)
        n1487 = xnode "Read/Write Control"("FPGA VI Reference In"=w4099, "error in"=w4098, "AO1"=w4108, "AO2"=w4109) -> ("error out"=w4097:errorcluster)  [unwired: 1 out]
      }
      event "Inject Pump 1": Value Change {
        n1488 = local read "Chemyx Syringe Pump Serial Port"() -> (w4136:refnum<visa-resource-name>)
        n1489 = event-data() -> ()  [unwired: 7 out]
        n1490 = local read "Pump write delay (ms)"() -> (w4137:dbl)
        n1491 = case shown="True" "Inject Pump 1" {
          tunnel: w4137 -> [w4144 w4158]
          tunnel: w4136 -> [w4141 w4157]
          frame False {
            n1492 = flat-sequence {
              tunnel: w4141 -> [w4145]
              tunnel: [w4145] -> w4142
              tunnel: w4144 -> [_]
              tunnel: [w4148] -> w4143
              tunnel: w4142 -> [w4148]
              tunnel: w4143 -> [w4149]
              tunnel: [w4149] -> w4139
              tunnel: [w4151] -> w4140
              tunnel: w4139 -> [w4151]
              tunnel: w4140 -> [w4153]
              frame #0 {
                n1493 = call "Write to pump.vi"("string"="enter pump1", "VISA resource name"=w4145) -> ()  [unwired: 1 out]
              }
              frame #1 {
                n1494 = Wait (ms)(milliseconds to wait="Pump pause delay (ms)") -> ()  [unwired: 1 out]
              }
              frame #2 {
                n1495 = call "Write to pump.vi"("string"="stop", "VISA resource name"=w4149) -> ()  [unwired: 1 out]
              }
              frame #3 {
                n1496 = Wait (ms)(milliseconds to wait=u32 500) -> ()  [unwired: 1 out]
              }
              frame #4 {
                n1497 = call "Write to pump.vi"("string"="stop", "VISA resource name"=w4153) -> ()  [unwired: 1 out]
              }
            }
          }
          frame True {
            n1498 = flat-sequence {
              tunnel: w4157 -> [w4167]
              tunnel: w4158 -> [w4162]
              tunnel: w4158 -> [w4169]
              tunnel: w4157 -> [w4170]
              tunnel: [w4170] -> w4155
              tunnel: [w4172] -> w4156
              tunnel: w4155 -> [w4172]
              tunnel: w4156 -> [w4174]
              frame #0 {
                n1499 = local read "All Pump Parameters"() -> (w4161:T5)
                n1500 = Unbundle By Name(w4161) -> ("Pump 1"=w4168:T42)
                n1501 = call "Set pump parameters.vi"("Pump write delay (ms)"=w4162, "Volume (uL)"="Ch 2 Inject Volume (uL)", "Rate (uL/h)"="Ch 1 Inject Rate (ul/h)", "Units"=4.0, "Pump #"=1.0, "Pump Parameters In"=w4168, "VISA resource name"=w4167) -> ("Pump Parameters Out"=w4160:T42)  [unwired: 3 in]
                n1502 = Bundle By Name(cluster=w4161, "Pump 1"=w4160) -> (w4159:T5)
                n1503 = local write "All Pump Parameters"(w4159) -> ()
              }
              frame #1 {
                n1504 = Wait (ms)(milliseconds to wait=w4169) -> ()  [unwired: 1 out]
              }
              frame #2 {
                n1505 = call "Write to pump.vi"("string"="start", "VISA resource name"=w4170) -> ()  [unwired: 1 out]
              }
              frame #3 {
                n1506 = Wait (ms)(milliseconds to wait=u32 500) -> ()  [unwired: 1 out]
              }
              frame #4 {
                n1507 = call "Write to pump.vi"("string"="start", "VISA resource name"=w4174) -> ()  [unwired: 1 out]
              }
            }
          }
        }
      }
      event "Inject Pump 3": Value Change {
        n1508 = event-data() -> ()  [unwired: 7 out]
        n1509 = local read "Pump write delay (ms)"() -> (w4177:dbl)
        n1510 = case shown="False" "Inject Pump 3" {
          tunnel: w4177 -> [w4184 w4198]
          tunnel: "Chemyx Syringe Pump Serial Port" -> [w4181 w4197]
          frame False {
            n1511 = flat-sequence {
              tunnel: w4181 -> [w4185]
              tunnel: [w4185] -> w4182
              tunnel: w4184 -> [_]
              tunnel: [w4188] -> w4183
              tunnel: w4182 -> [w4188]
              tunnel: w4183 -> [w4189]
              tunnel: [w4189] -> w4179
              tunnel: [w4191] -> w4180
              tunnel: w4179 -> [w4191]
              tunnel: w4180 -> [w4193]
              frame #0 {
                n1512 = call "Write to pump.vi"("string"="enter pump3", "VISA resource name"=w4185) -> ()  [unwired: 1 out]
              }
              frame #1 {
                n1513 = local read "Pump pause delay (ms)"() -> (w4187:u32)
                n1514 = Wait (ms)(milliseconds to wait=w4187) -> ()  [unwired: 1 out]
              }
              frame #2 {
                n1515 = call "Write to pump.vi"("string"="stop", "VISA resource name"=w4189) -> ()  [unwired: 1 out]
              }
              frame #3 {
                n1516 = Wait (ms)(milliseconds to wait=u32 0) -> ()  [unwired: 1 out]
              }
              frame #4 {
                n1517 = call "Write to pump.vi"("string"="stop", "VISA resource name"=w4193) -> ()  [unwired: 1 out]
              }
            }
          }
          frame True {
            n1518 = flat-sequence {
              tunnel: w4197 -> [w4207]
              tunnel: w4198 -> [w4202]
              tunnel: w4198 -> [w4209]
              tunnel: w4197 -> [w4210]
              tunnel: [w4210] -> w4195
              tunnel: [w4213] -> w4196
              tunnel: w4195 -> [w4213]
              tunnel: w4196 -> [w4214]
              frame #0 {
                n1519 = local read "All Pump Parameters"() -> (w4201:T5)
                n1520 = Unbundle By Name(w4201) -> ("Pump 3"=w4208:T42)
                n1521 = call "Set pump parameters.vi"("Pump write delay (ms)"=w4202, "Volume (uL)"="Ch 3 Inject Volume (uL)", "Rate (uL/h)"="Ch 3 Inject Rate (ul/h)", "Units"=4.0, "Pump #"=3.0, "Pump Parameters In"=w4208, "VISA resource name"=w4207) -> ("Pump Parameters Out"=w4200:T42)  [unwired: 3 in]
                n1522 = Bundle By Name(cluster=w4201, "Pump 3"=w4200) -> (w4199:T5)
                n1523 = local write "All Pump Parameters"(w4199) -> ()
              }
              frame #1 {
                n1524 = Wait (ms)(milliseconds to wait=w4209) -> ()  [unwired: 1 out]
              }
              frame #2 {
                n1525 = call "Write to pump.vi"("string"="start", "VISA resource name"=w4210) -> ()  [unwired: 1 out]
              }
              frame #3 {
                n1526 = Wait (ms)(milliseconds to wait=u32 500) -> ()  [unwired: 1 out]
              }
              frame #4 {
                n1527 = call "Write to pump.vi"("string"="start", "VISA resource name"=w4214) -> ()  [unwired: 1 out]
              }
            }
          }
        }
      }
      event "Inject Pump 2": Value Change {
        n1528 = event-data() -> ()  [unwired: 7 out]
        n1529 = local read "Pump write delay (ms)"() -> (w4218:dbl)
        n1530 = flat-sequence {
          tunnel: w4216 -> [w4231]
          tunnel: w4218 -> [w4227]
          tunnel: "Inject Pump 2" -> [_]
          tunnel: w4218 -> [w4233]
          tunnel: w4216 -> [w4234]
          frame #0 {
            n1531 = local read "All Pump Parameters"() -> (w4226:T5)
            n1532 = Multiply(x=60.0, y="Flush Center Ch Rate (ul/m)") -> (x*y=w4223:dbl)
            n1533 = Unbundle By Name(w4226) -> ("Pump 2"=w4232:T42)
            n1534 = call "Set pump parameters.vi"("Pump write delay (ms)"=w4227, "Volume (uL)"="Flush Center Ch Volume (uL)", "Rate (uL/h)"=w4223, "Units"=3.0, "Pump #"=2.0, "Pump Parameters In"=w4232, "VISA resource name"=w4231) -> ("Pump Parameters Out"=w4225:T42)  [unwired: 3 in]
            n1535 = Bundle By Name(cluster=w4226, "Pump 2"=w4225) -> (w4224:T5)
            n1536 = local write "All Pump Parameters"(w4224) -> ()
            n1537 = Add(x="Flush Center Ch Volume (uL)", y="Total Volume\nFlushed (uL)") -> (x+y=w4220:dbl)
            n1538 = local write "Total Volume\nFlushed (uL)"(w4220) -> ()
          }
          frame #1 {
            n1539 = Wait (ms)(milliseconds to wait=w4233) -> ()  [unwired: 1 out]
          }
          frame #2 {
            n1540 = call "Write to pump.vi"("string"="start", "VISA resource name"=w4234) -> ()  [unwired: 1 out]
          }
        }
        n1541 = local read "Chemyx Syringe Pump Serial Port"() -> (w4216:refnum<visa-resource-name>)
      }
      event "Sample Channel Flow": Value Change {
        n1542 = event-data() -> ()  [unwired: 7 out]
        n1543 = Select(t="run" ("string"), s="Sample Channel Flow", f="stop" ("string")) -> (s? t:f=w4236:string)
        n1544 = Concatenate Strings(w4236, "\r") -> (w4240:string)
        n1545 = VISA Write(VISA resource name=w4242, write buffer=w4240) -> ()  [unwired: 1 in, 3 out]
      }
      event "Flip Green Filter": Value Change {
        n1546 = event-data() -> ()  [unwired: 7 out]
        n1547 = Not(x="Flip Green Filter") -> (.not. x?=w4243:bool)
        n1548 = local write "Flip Green Filter"(w4243) -> ()
        n1549 = flat-sequence {
          tunnel: w4251 -> [w4256]
          tunnel: w4250 -> [w4255]
          tunnel: [w4253] -> w4248
          tunnel: [w4252] -> w4247
          tunnel: [w4279] -> w4246
          tunnel: w4248 -> [w4279]
          tunnel: [w4278] -> w4245
          tunnel: w4247 -> [w4278]
          tunnel: w4246 -> [w4283]
          tunnel: w4245 -> [w4282]
          tunnel: [w4281] -> w4249
          frame #0 {
            n1550 = xnode "Read/Write Control"("FPGA VI Reference In"=w4256, "error in"=w4255, "Green Filter Flipper"=TRUE) -> ("FPGA VI Reference Out"=w4253:T19, "error out"=w4252:errorcluster)
          }
          frame #1 {
            n1551 = Wait (ms)(milliseconds to wait=u32 100) -> ()  [unwired: 1 out]
          }
          frame #2 {
            n1552 = xnode "Read/Write Control"("FPGA VI Reference In"=w4283, "error in"=w4282, "Green Filter Flipper"=FALSE) -> ("error out"=w4281:errorcluster)  [unwired: 1 out]
          }
        }
      }
      event "Pump 1 contents", "Pump 3 contents": Value Change {
        n1553 = event-data() -> ()  [unwired: 7 out]
        n1554 = local read "Pump 1 contents"() -> (→"Pump 1 cont disp":string)
        n1555 = local read "Pump 3 contents"() -> (→"Pump 3 cont disp":string)
      }
      event "Reset Trap Pos. FB": Value Change {
        n1556 = event-data() -> ()  [unwired: 7 out]
        n1557 = xnode "Read/Write Control"("FPGA VI Reference In"=w4310, "error in"=w4309, "Trap Pos. FB Reset"="Reset Trap Pos. FB") -> ()  [unwired: 2 out]
      }
      event "Trap Pos. FB ON": Value Change {
        n1558 = event-data() -> ()  [unwired: 7 out]
        n1559 = xnode "Read/Write Control"("FPGA VI Reference In"=w4334, "error in"=w4333, "Force feedback"="Trap Pos. FB ON") -> ()  [unwired: 2 out]
      }
      event "Trap Pos. FB Range", "Trap Pos. FB Gains", "Trap Pos. FB Mult Factor", "Trap Pos. FB Offset Factor", "Trap Pos FB Negate Action", "Trap Pos FB Monitor\nT1 or T2": Value Change {
        n1560 = event-data() -> ()  [unwired: 7 out]
        n1561 = xnode "Read/Write Control"("FPGA VI Reference In"=w4364, "error in"=w4363, "Trap Pos. FB Range"="Trap Pos. FB Range", "Trap Pos. FB Gains"="Trap Pos. FB Gains", "Trap Pos. FB Mult Factor"="Trap Pos. FB Mult Factor", "Trap Pos. FB Offset Factor"="Trap Pos. FB Offset Factor", "Trap Pos FB Negate Action"="Trap Pos FB Negate Action", "Trap Pos FB Monitor T1 or T2"="Trap Pos FB Monitor\nT1 or T2", "AI1 X Scale"="Trap Pos. AI1 X Pre-scale") -> ()  [unwired: 2 out]
      }
      event "Trap Pos FB SP": Value Change {
        n1562 = event-data() -> ()  [unwired: 7 out]
        n1563 = xnode "Read/Write Control"("FPGA VI Reference In"=w4418, "error in"=w4417, "Trap Pos. FB SP"="Trap Pos FB SP") -> ()  [unwired: 2 out]
      }
      event "Set SP to Reading": Value Change {
        n1564 = event-data() -> ()  [unwired: 7 out]
        n1565 = local read "Trap Pos FB Monitor\nT1 or T2"() -> (w4447:bool)
        n1566 = local read "Trap X AI1 (DMA)"() -> (w4450:T13)
        n1567 = local read "Trap X (AI1)"() -> (w4453:T10)
        n1568 = Unbundle By Name(w4453) -> ("Trap 1"=w4452:fxp<+/-,16,1>, "Trap 2"=w4451:fxp<+/-,16,1>)
        n1569 = Unbundle By Name(w4450) -> ("Set 1"=w4449:fxp<+/-,16,1>, "Set 2"=w4448:fxp<+/-,16,1>)
        n1570 = Select(t=w4452, s=w4447, f=w4451) -> (s? t:f=w4446:fxp<+/-,16,1>)
        n1571 = Select(t=w4449, s=w4447, f=w4448) -> (s? t:f=w4445:fxp<+/-,16,1>)
        n1572 = Not(x="Set SP Using...") -> (.not. x?=w4440:bool)
        n1573 = Select(t=w4446, s=w4440, f=w4445) -> (s? t:f=w4441:fxp<+/-,16,1>)
        n1574 = xnode "Read/Write Control"("FPGA VI Reference In"=w4443, "error in"=w4442, "Trap Pos. FB SP"=w4441) -> ()  [unwired: 2 out]
        n1575 = local write "Trap Pos FB SP"(w4441) -> ()
      }
      event "Trap Pos. FB Out Scale 2^n": Value Change {
        n1576 = event-data() -> ()  [unwired: 7 out]
        n1577 = Scale By Power Of 2(n="Trap Pos. FB Out Scale 2^n", x=ext 1.0) -> (x*2^n=w4476:ext)
        n1578 = property on="Trap Pos. FB Mult Factor" class="DigNum (strict)"("Val(Sgnl)"=w4476) -> ()  [unwired: 2 in, 2 out]
      }
      event "Trap Pos FB Int Count": Value Change {
        n1579 = event-data() -> ()  [unwired: 7 out]
        n1580 = xnode "Read/Write Control"("FPGA VI Reference In"=w4481, "error in"=w4480, "Trap Pos FB Int Count"="Trap Pos FB Int Count") -> ()  [unwired: 2 out]
      }
    }
    "error out 2" <- w2567
    n1581 = node-c288() -> ()  [unwired: 2 out]
  }
  n1582 = timed-loop "Run Scripts, including: stage motion" {
    tunnel: w42 -> [w4505]
    tunnel: w41 -> [w4506]
    tunnel: [w4506] -> w40
    tunnel: [w4505] -> w39
    timing: w37 -> [_]
    timing-out: [_] -> w36
    tunnel: w22 -> [w4504]
    tunnel: w23 -> [w4503]
    stop <- w4507 stop-if-true
    n1583 = node-c288() -> ()  [unwired: 1 in, 1 out]
    n1584 = event shown="[3] \"Move Cap. 2 (ADig Left)\": Value Change" {
      selector: _ -> [_ _ _ _ _ _ _ _ _ _ _ _ _ _ _ _]
      dyn-events: _ -> [_ _ _ _ _ _ _ _ _ _ _ _ _ _ _ _]
      timeout: _ -> [_ _ _ _ _ _ _ _ _ _ _ _ _ _ _ _]
      tunnel: ["Set Position" "Move to Position" "Move Cap. 1 (DNA Right)" "Move Cap. 2 (ADig Left)" _ "Cal/Data Acq. Spot" "Dump Beads" "Dip for Protein" _ _ "Got ADig bead" "Got DNA bead" "Take Stepping Data" _ "Take Detection Laser\nImage" _] -> _
      tunnel: [_ _ _ _ _ _ _ _ _ _ _ _ _ _ _ w4998] -> w4507
      tunnel: w4505 -> [w4525 w4533 w4557 w4612 w4657 w4693 w4771 w4796 w4846 w4872 _ _ _ _ _ _]
      tunnel: w4506 -> [w4526 w4534 w4558 w4613 w4658 w4694 w4772 w4797 w4847 w4873 _ _ _ _ _ _]
      tunnel: w4504 -> [_ _ w4555 w4609 _ _ _ _ _ _ _ _ _ _ _ _]
      tunnel: w4503 -> [_ _ w4554 w4610 _ _ _ _ _ _ _ _ _ _ _ _]
      event "Set Position", "Set Position 2", "Set Position 3", "Set Position 4", "Set Position 5", "Set Position 1": Value Change {
        n1585 = event-data() -> ()  [unwired: 1 in, 5 out]
        n1586 = Build Array("Set Position 1", "Set Position 2", "Set Position 3", "Set Position 4", "Set Position 5") -> (w4524:bool[])
        n1587 = Boolean Array To Number(Boolean array=w4524) -> (number=w4523:u32)
        n1588 = Logarithm Base 2(1:w4523) -> (0:w4515:dbl)
        n1589 = call "Read Stage Position.vi"("error in"=w4525, "VISA resource name in"=w4526) -> ("Current Position"=w4530:cluster{dbl, dbl, dbl}, "error out"=w4529:errorcluster)  [unwired: 2 out]
        n1590 = Decrement(x="Position") -> (x-1=w4513:dbl)
        n1591 = Greater Or Equal?(x=w4515, y=0.0) -> (x >= y?=w4516:bool)
        n1592 = local write "Stage Control Serial Error"(w4529) -> ()
        n1593 = Cluster To Array(cluster=w4530) -> (array=w4527:dbl[])
        n1594 = Select(t=w4515, s=w4516, f=w4513) -> (s? t:f=w4512:dbl)
        n1595 = Increment(x=w4512) -> (x+1=w4511:dbl)
        n1596 = Build Array (concatenate)(w4511, w4527) -> (w4510:dbl[])
        n1597 = Replace Array Subset(array="Saved Stage Positions", new element=w4510, index (row)=w4512) -> (w4528:dbl[][])  [unwired: 1 in]
        n1598 = local write "Saved Stage Positions"(w4528) -> ()
      }
      event "Move to Position": Value Change {
        n1599 = event-data() -> ()  [unwired: 1 in, 5 out]
        n1600 = flat-sequence {
          tunnel: w4534 -> [w4537]
          tunnel: w4533 -> [w4536]
          frame #0 {
            n1601 = local read "Position"() -> (w4549:dbl)
            n1602 = local read "Saved Stage Positions"() -> (w4547:dbl[][])
            n1603 = Decrement(x=w4549) -> (x-1=w4546:dbl)
            n1604 = Array Subset(array=w4547, index (row)=w4546, length (row)=1 ("length"), index (col)=1 ("index"), length (col)=3 ("length")) -> (w4543:dbl[][])
            n1605 = Reshape Array(w4543, 3 ("dimension size")) -> (w4541:dbl[])
            n1606 = Array To Cluster(array=w4541) -> (cluster=w4540:cluster{"[0]":dbl, "[1]":dbl, "[2]":dbl})
            n1607 = call "Set Stage Position.vi"("Position"=w4540, "error in"=w4536, "VISA resource name in"=w4537) -> ("error out"=w4539:errorcluster)  [unwired: 2 out]
            n1608 = local write "Stage Control Serial Error"(w4539) -> ()
            n1609 = local write "Stage Moving"(TRUE ("Stage Moving")) -> ()
          }
          frame #1 {
            n1610 = call <vilib>:"Beep.vi"() -> ()  [unwired: 3 in, 9 out]
            n1611 = local write "Stage Moving"(FALSE ("Stage Moving")) -> ()
          }
        }
      }
      event "Move Cap. 1 (DNA Right)": Value Change {
        n1612 = event-data() -> ()  [unwired: 1 in, 5 out]
        n1613 = local write "Move Cap. 1 (DNA Right)"(FALSE ("Move Cap. 1 (DNA Right)")) -> ()
        n1614 = flat-sequence {
          tunnel: w4558 -> [w4566]
          tunnel: w4557 -> [w4565]
          tunnel: w4555 -> [w4564]
          tunnel: w4554 -> [w4563]
          tunnel: [w4562] -> w4553
          tunnel: [w4561] -> w4552
          tunnel: ["Cap 1 Samp Flow ON"] -> w4551
          tunnel: w4553 -> [w4589]
          tunnel: w4552 -> [w4588]
          tunnel: w4551 -> [w4587]
          frame #0 {
            n1615 = local read "Saved Stage Positions"() -> (w4576:dbl[][])
            n1616 = Array Subset(array=w4576, index (row)=0 ("index"), length (row)=1 ("length"), index (col)=1 ("index"), length (col)=3 ("length")) -> (w4573:dbl[][])
            n1617 = Reshape Array(w4573, 3 ("dimension size")) -> (w4571:dbl[])
            n1618 = Array To Cluster(array=w4571) -> (cluster=w4570:cluster{"[0]":dbl, "[1]":dbl, "[2]":dbl})
            n1619 = case shown="True" "Cap 1 Samp Flow ON" {
              tunnel: w4563 -> [w4578 w4584]
              tunnel: w4564 -> [w4579 w4583]
              tunnel: [w4579 w4581] -> w4562
              tunnel: [w4578 w4580] -> w4561
              frame False {
              }
              frame True {
                # "run flow"
                n1620 = Concatenate Strings("run" ("string"), "\r") -> (w4585:string)
                n1621 = VISA Write(VISA resource name=w4583, write buffer=w4585, error in (no error)=w4584) -> (VISA resource name out=w4581:refnum<visa-resource-name>, error out=w4580:errorcluster)  [unwired: 1 out]
              }
            }
            n1622 = call "Set Stage Position.vi"("Position"=w4570, "error in"=w4565, "VISA resource name in"=w4566) -> ("error out"=w4569:errorcluster)  [unwired: 2 out]
            n1623 = local write "Stage Control Serial Error"(w4569) -> ()
            n1624 = local write "Stage Moving"(TRUE ("Stage Moving")) -> ()
          }
          frame #1 {
            n1625 = local write "Stage Moving"(FALSE ("Stage Moving")) -> ()
            n1626 = case shown="True" w4587 {
              tunnel: w4588 -> [w4594 w4600]
              tunnel: w4589 -> [w4595 w4599]
              tunnel: [w4595 w4597] -> _
              tunnel: [w4594 w4596] -> _
              frame False {
              }
              frame True {
                n1627 = Concatenate Strings("stop" ("string"), "\r") -> (w4601:string)
                n1628 = VISA Write(VISA resource name=w4599, write buffer=w4601, error in (no error)=w4600) -> (VISA resource name out=w4597:refnum<visa-resource-name>, error out=w4596:errorcluster)  [unwired: 1 out]
              }
            }
            n1629 = case shown="True" TRUE {
              tunnel: "Cap 1 T ON" -> [w4604 w4605]
              frame False {
                n1630 = property on="Trap 1 (ON/OFF)" class="Bool (strict)"("Val(Sgnl)"=w4604) -> ()  [unwired: 2 in, 2 out]
              }
              frame True {
                n1631 = property on="Trap 2 (ON/OFF)" class="Bool (strict)"("Val(Sgnl)"=w4605) -> ()  [unwired: 2 in, 2 out]
              }
            }
            n1632 = call <vilib>:"Beep.vi"() -> ()  [unwired: 3 in, 9 out]
            n1633 = case shown="True" "Cap 1 Flow ON" {
              frame False {
              }
              frame True {
                n1634 = property on="Inject Pump 1" class="Bool (strict)"("Val(Sgnl)"=TRUE ("Value (Signaling)")) -> ()  [unwired: 2 in, 2 out]
              }
            }
          }
        }
      }
      event "Move Cap. 2 (ADig Left)": Value Change {
        n1635 = event-data() -> ()  [unwired: 1 in, 5 out]
        n1636 = local write "Move Cap. 2 (ADig Left)"(FALSE ("Move Cap. 2 (ADig Left)")) -> ()
        n1637 = flat-sequence {
          tunnel: w4613 -> [w4621]
          tunnel: w4612 -> [w4620]
          tunnel: w4610 -> [w4619]
          tunnel: w4609 -> [w4618]
          tunnel: [w4617] -> w4608
          tunnel: [w4616] -> w4607
          tunnel: ["Cap 2 Samp Flow ON"] -> w4606
          tunnel: w4608 -> [w4644]
          tunnel: w4607 -> [w4643]
          tunnel: w4606 -> [w4642]
          frame #0 {
            n1638 = local read "Saved Stage Positions"() -> (w4631:dbl[][])
            n1639 = case shown="True" "Cap 2 Samp Flow ON" {
              tunnel: w4619 -> [w4633 w4639]
              tunnel: w4618 -> [w4634 w4638]
              tunnel: [w4634 w4636] -> w4617
              tunnel: [w4633 w4635] -> w4616
              frame False {
              }
              frame True {
                # "run flow"
                n1640 = Concatenate Strings("run" ("string"), "\r") -> (w4640:string)
                n1641 = VISA Write(VISA resource name=w4638, write buffer=w4640, error in (no error)=w4639) -> (VISA resource name out=w4636:refnum<visa-resource-name>, error out=w4635:errorcluster)  [unwired: 1 out]
              }
            }
            n1642 = Array Subset(array=w4631, index (row)=1 ("index"), length (row)=1 ("length"), index (col)=1 ("index"), length (col)=3 ("length")) -> (w4628:dbl[][])
            n1643 = Reshape Array(w4628, 3 ("dimension size")) -> (w4626:dbl[])
            n1644 = Array To Cluster(array=w4626) -> (cluster=w4625:cluster{"[0]":dbl, "[1]":dbl, "[2]":dbl})
            n1645 = call "Set Stage Position.vi"("Position"=w4625, "error in"=w4620, "VISA resource name in"=w4621) -> ("error out"=w4624:errorcluster)  [unwired: 2 out]
            n1646 = local write "Stage Moving"(TRUE ("Stage Moving")) -> ()
            n1647 = local write "Stage Control Serial Error"(w4624) -> ()
          }
          frame #1 {
            n1648 = local write "Stage Moving"(FALSE ("Stage Moving")) -> ()
            n1649 = case shown="True" TRUE {
              tunnel: "Cap 2 T ON" -> [w4655 w4656]
              frame False {
                n1650 = property on="Trap 2 (ON/OFF)" class="Bool (strict)"("Val(Sgnl)"=w4655) -> ()  [unwired: 2 in, 2 out]
              }
              frame True {
                n1651 = property on="Trap 1 (ON/OFF)" class="Bool (strict)"("Val(Sgnl)"=w4656) -> ()  [unwired: 2 in, 2 out]
              }
            }
            n1652 = call <vilib>:"Beep.vi"() -> ()  [unwired: 3 in, 9 out]
            n1653 = case shown="True" w4642 {
              tunnel: w4644 -> [_ w4650]
              tunnel: w4643 -> [_ w4649]
              frame False {
              }
              frame True {
                n1654 = Concatenate Strings("stop" ("string"), "\r") -> (w4652:string)
                n1655 = VISA Write(VISA resource name=w4650, write buffer=w4652, error in (no error)=w4649) -> ()  [unwired: 3 out]
              }
            }
            n1656 = case shown="True" "Cap 2 Flow ON" {
              frame False {
              }
              frame True {
                n1657 = property on="Inject Pump 3" class="Bool (strict)"("Val(Sgnl)"=TRUE ("Value (Signaling)")) -> ()  [unwired: 2 in, 2 out]
              }
            }
          }
        }
      }
      event "+z", "-z": Value Change {
        n1658 = event-data() -> ()  [unwired: 1 in, 5 out]
        n1659 = flat-sequence {
          tunnel: w4657 -> [w4679]
          tunnel: w4658 -> [w4659]
          frame #0 {
            n1660 = call "Read Stage Position.vi"("error in"=w4679, "VISA resource name in"=w4659) -> ("Current Position"=w4664:cluster{dbl, dbl, dbl}, "error out"=w4677:errorcluster, "VISA resource name out"=w4678:refnum<visa-resource-name>)  [unwired: 1 out]
            n1661 = local read "Saved Stage Positions"() -> (w4688:dbl[][])
            n1662 = Divide(x="z nudge increment (um)", y=1000.0) -> (x/y=w4676:dbl)
            n1663 = Boolean To (0,1)(Boolean="+z") -> (0, 1=w4668:i16)
            n1664 = Boolean To (0,1)(Boolean="-z") -> (0, 1=w4669:i16)
            n1665 = Array Subset(array=w4688, index (row)=1 ("index"), length (row)=1 ("length"), index (col)=1 ("index"), length (col)=3 ("length")) -> (w4685:dbl[][])
            n1666 = Multiply(x=w4668, y=w4676) -> (x*y=w4672:dbl)
            n1667 = Multiply(x=w4669, y=w4676) -> (x*y=w4670:dbl)
            n1668 = Unbundle(w4664) -> (w4662:dbl, w4661:dbl, w4665:dbl)
            n1669 = Negate(x=w4670) -> (-x=w4671:dbl)
            n1670 = Reshape Array(w4685, 3 ("dimension size")) -> (w4683:dbl[])
            n1671 = Add(x=w4672, y=w4671) -> (x+y=w4673:dbl)
            n1672 = Array To Cluster(array=w4683) -> ()  [unwired: 1 out]
            n1673 = Add(x=w4673, y=w4665) -> (x+y=w4663:dbl)
            n1674 = Bundle(cluster=w4664, w4662, w4661, w4663) -> (w4660:cluster{dbl, dbl, dbl})
            n1675 = call "Set Stage Position.vi"("Position"=w4660, "error in"=w4677, "VISA resource name in"=w4678) -> ("error out"=w4682:errorcluster)  [unwired: 2 out]
            n1676 = local write "Stage Moving"(TRUE ("Stage Moving")) -> ()
            n1677 = local write "Stage Control Serial Error"(w4682) -> ()
          }
          frame #1 {
            n1678 = local write "Stage Moving"(FALSE ("Stage Moving")) -> ()
            n1679 = call <vilib>:"Beep.vi"() -> ()  [unwired: 3 in, 9 out]
          }
        }
      }
      event "Cal/Data Acq. Spot": Value Change {
        # "CALIBRATE DATA ACQUISITION SPOT? LOCATE WHERE TO COLLECT FLUORESCENCE FROM?"
        n1680 = event-data() -> ()  [unwired: 1 in, 5 out]
        n1681 = flat-sequence {
          tunnel: w4694 -> [w4697]
          tunnel: w4693 -> [w4696]
          tunnel: ["Cal @ (MHz)"] -> w4691
          tunnel: w4691 -> [w4717]
          tunnel: w4691 -> [w4738]
          frame #0 {
            n1682 = local read "Saved Stage Positions"() -> (w4700:dbl[][])
            n1683 = Array Subset(array=w4700, index (row)=2 ("index"), length (row)=1 ("length"), index (col)=1 ("index"), length (col)=3 ("length")) -> (w4703:dbl[][])
            n1684 = Reshape Array(w4703, 3 ("dimension size")) -> (w4705:dbl[])
            n1685 = local write "Stage Moving"(TRUE ("Stage Moving")) -> ()
            n1686 = Array To Cluster(array=w4705) -> (cluster=w4706:cluster{"[0]":dbl, "[1]":dbl, "[2]":dbl})
            n1687 = call "Set Stage Position.vi"("Position"=w4706, "error in"=w4696, "VISA resource name in"=w4697) -> ("error out"=w4707:errorcluster)  [unwired: 2 out]
            n1688 = local write "Stage Control Serial Error"(w4707) -> ()
          }
          frame #1 {
            n1689 = property on="Trap Delta (MHz)" class="DigNum (strict)"("Val(Sgnl)"="Cal @ (MHz)") -> ()  [unwired: 2 in, 2 out]
            n1690 = local write "Stage Moving"(FALSE ("Stage Moving")) -> ()
            n1691 = call <vilib>:"Beep.vi"() -> ()  [unwired: 3 in, 9 out]
          }
          frame #2 {
            n1692 = Wait (ms)(milliseconds to wait=u32 100) -> ()  [unwired: 1 out]
          }
          frame #3 {
            n1693 = property on="Save Calibration" class="Bool (strict)"("Val(Sgnl)"=TRUE ("Value (Signaling)")) -> ()  [unwired: 2 in, 2 out]
          }
          frame #4 {
            n1694 = Wait (ms)(milliseconds to wait=u32 4000) -> ()  [unwired: 1 out]
          }
          frame #5 {
            n1695 = while {
              stop <- w4714 stop-if-true
              n1696 = local read "Saving..."() -> (w4715:bool)
              n1697 = Wait (ms)(milliseconds to wait=u32 100) -> ()  [unwired: 1 out]
              n1698 = Not(x=w4715) -> (.not. x?=w4714:bool)
            }
          }
          frame #6 {
            n1699 = case shown="True" "W/ Offset 1" {
              tunnel: w4717 -> [_ w4719]
              frame False {
              }
              frame True {
                n1700 = stacked-sequence {
                  tunnel: w4719 -> [_ _ _ _ _ _ _ w4736]
                  frame #0 {
                    n1701 = property on="Trap Delta (MHz)" class="DigNum (strict)"("Val(Sgnl)"="Offset 1 Start (MHz)") -> ()  [unwired: 2 in, 2 out]
                    n1702 = Replace Array Subset(array=u32[] [0] ("Index Values"), new element="Offset 1 Set", index=0) -> (w4720:u32[])
                    n1703 = property on="Saved AOD Raster Scan Parameter Sets" class="Arr (strict)"("Index Values"=w4720) -> ()  [unwired: 2 in, 2 out]
                  }
                  frame #1 {
                    n1704 = Wait (ms)(milliseconds to wait=u32 200) -> ()  [unwired: 1 out]
                  }
                  frame #2 {
                    n1705 = property on="Load parameters" class="Bool (strict)"("Val(Sgnl)"=TRUE ("Value (Signaling)")) -> ()  [unwired: 2 in, 2 out]
                  }
                  frame #3 {
                    n1706 = Wait (ms)(milliseconds to wait=u32 200) -> ()  [unwired: 1 out]
                  }
                  frame #4 {
                    n1707 = property on="Trap Raster Scan" class="Bool (strict)"("Val(Sgnl)"=TRUE ("Value (Signaling)")) -> ()  [unwired: 2 in, 2 out]
                  }
                  frame #5 {
                    n1708 = Wait (ms)(milliseconds to wait=u32 2000) -> ()  [unwired: 1 out]
                  }
                  frame #6 {
                    n1709 = while {
                      stop <- w4733 stop-if-true
                      n1710 = local read "Raster Scanning..."() -> (w4735:bool)
                      n1711 = local read "Saving..."() -> (w4731:bool)
                      n1712 = Wait (ms)(milliseconds to wait=u32 100) -> ()  [unwired: 1 out]
                      n1713 = Not(x=w4731) -> (.not. x?=w4730:bool)
                      n1714 = Not(x=w4735) -> (.not. x?=w4732:bool)
                      n1715 = And(x=w4732, y=w4730) -> (x .and. y?=w4733:bool)
                    }
                  }
                  frame #7 {
                    n1716 = property on="Trap Delta (MHz)" class="DigNum (strict)"("Val(Sgnl)"=w4736) -> ()  [unwired: 2 in, 2 out]
                  }
                }
              }
            }
          }
          frame #7 {
            n1717 = local read "Save ave N"() -> (w4737:dbl)
            n1718 = case shown="True" "W/ Offset 2" {
              tunnel: w4738 -> [_ w4744]
              tunnel: w4737 -> [_ w4743]
              frame False {
                n1719 = Multiply(x="Cal read wait (s)", y=u32 1000 ("milliseconds to wait")) -> (x*y=w4741:u32)
                n1720 = Wait (ms)(milliseconds to wait=w4741) -> ()  [unwired: 1 out]
              }
              frame True {
                n1721 = stacked-sequence {
                  tunnel: w4744 -> [_ _ _ _ _ _ _ _ _ w4765 _ _]
                  tunnel: w4743 -> [_ _ _ _ _ _ _ _ _ w4763 _ _]
                  frame #0 {
                    n1722 = property on="Save ave N" class="DigNum (strict)"("Val(Sgnl)"=1.0 ("Value (Signaling)")) -> ()  [unwired: 2 in, 2 out]
                  }
                  frame #1 {
                    n1723 = Wait (ms)(milliseconds to wait=u32 500) -> ()  [unwired: 1 out]
                  }
                  frame #2 {
                    n1724 = property on="Trap Delta (MHz)" class="DigNum (strict)"("Val(Sgnl)"="Offset 2 Start (MHz)") -> ()  [unwired: 2 in, 2 out]
                    n1725 = Replace Array Subset(array=u32[] [0] ("Index Values"), new element="Offset 2 Set", index=0) -> (w4749:u32[])
                    n1726 = property on="Saved AOD Raster Scan Parameter Sets" class="Arr (strict)"("Index Values"=w4749) -> ()  [unwired: 2 in, 2 out]
                  }
                  frame #3 {
                    n1727 = Wait (ms)(milliseconds to wait=u32 500) -> ()  [unwired: 1 out]
                  }
                  frame #4 {
                    n1728 = property on="Load parameters" class="Bool (strict)"("Val(Sgnl)"=TRUE ("Value (Signaling)")) -> ()  [unwired: 2 in, 2 out]
                  }
                  frame #5 {
                    n1729 = Wait (ms)(milliseconds to wait=u32 500) -> ()  [unwired: 1 out]
                  }
                  frame #6 {
                    n1730 = property on="Trap Raster Scan" class="Bool (strict)"("Val(Sgnl)"=TRUE ("Value (Signaling)")) -> ()  [unwired: 2 in, 2 out]
                  }
                  frame #7 {
                    n1731 = Wait (ms)(milliseconds to wait=u32 2000) -> ()  [unwired: 1 out]
                  }
                  frame #8 {
                    n1732 = while {
                      stop <- w4758 stop-if-true
                      n1733 = local read "Raster Scanning..."() -> (w4761:bool)
                      n1734 = local read "Saving..."() -> (w4759:bool)
                      n1735 = Wait (ms)(milliseconds to wait=u32 100) -> ()  [unwired: 1 out]
                      n1736 = Not(x=w4759) -> (.not. x?=w4757:bool)
                      n1737 = Not(x=w4761) -> (.not. x?=w4760:bool)
                      n1738 = And(x=w4760, y=w4757) -> (x .and. y?=w4758:bool)
                    }
                  }
                  frame #9 {
                    n1739 = property on="Trap Delta (MHz)" class="DigNum (strict)"("Val(Sgnl)"=w4765) -> ()  [unwired: 2 in, 2 out]
                    n1740 = property on="Saved AOD Raster Scan Parameter Sets" class="Arr (strict)"("Index Values"=u32[] [0]) -> ()  [unwired: 2 in, 2 out]
                    n1741 = property on="Save ave N" class="DigNum (strict)"("Val(Sgnl)"=w4763) -> ()  [unwired: 2 in, 2 out]
                  }
                  frame #10 {
                    n1742 = Wait (ms)(milliseconds to wait=u32 500) -> ()  [unwired: 1 out]
                  }
                  frame #11 {
                    n1743 = property on="Load parameters" class="Bool (strict)"("Val(Sgnl)"=TRUE ("Value (Signaling)")) -> ()  [unwired: 2 in, 2 out]
                  }
                }
              }
            }
          }
          frame #8 {
            n1744 = property on="Read Cal" class="Bool (strict)"("Val(Sgnl)"=TRUE ("Value (Signaling)")) -> ()  [unwired: 2 in, 2 out]
          }
          frame #9 {
            n1745 = Wait (ms)(milliseconds to wait=u32 500) -> ()  [unwired: 1 out]
          }
          frame #10 {
            n1746 = property on="Fish for Tether" class="Bool (strict)"("Val(Sgnl)"=TRUE ("Value (Signaling)")) -> ()  [unwired: 2 in, 2 out]
          }
        }
        n1747 = local write "Cal/Data Acq. Spot"(FALSE ("Cal/Data Acq. Spot")) -> ()
      }
      event "Dump Beads": Value Change {
        # "SCRIPT TO REMOVE BOTH BEADS FROM THE TRAPS. TURNS ON LIGHT WHICH INDICATES THAT STAGE IS MOVING. THEN STOPS SAVING DATA. \nSETS Sample Channel Flow TO TRUE. STOPS INTERLACING GREEN FLUORESCENCE. TURNS OFF Tether INDICATOR BECAUSE WE ARE THROWING IT\nAWAY. SHUTS OFF TRAP POSITION FEEDBACK."
        n1748 = event-data() -> ()  [unwired: 1 in, 5 out]
        n1749 = flat-sequence {
          tunnel: w4772 -> [w4778]
          tunnel: w4771 -> [w4777]
          frame #0 {
            w4774 = FALSE ("Fl. Triggered...")
            w4775 = TRUE ("Stage Moving")
            n1750 = local read "Saving..."() -> (w4776:bool)
            n1751 = local write "Fl. Triggered..."(w4774) -> ()
            n1752 = local write "Stage Moving"(w4775) -> ()
            n1753 = local write "Tether"(w4774) -> ()
            n1754 = property on="Green Laser ON/Interlacing" class="Bool (strict)"("Val(Sgnl)"=w4774) -> ()  [unwired: 2 in, 2 out]
            n1755 = property on="Trap Pos. FB ON" class="Bool (strict)"("Val(Sgnl)"=w4774) -> ()  [unwired: 2 in, 2 out]
            n1756 = property on="Sample Channel Flow" class="Bool (strict)"("Val(Sgnl)"=w4775) -> ()  [unwired: 2 in, 2 out]
            n1757 = local write "Stop Saving"(w4776) -> ()
          }
          frame #1 {
            # "MOVES TO THE DUMP BEADS POSITION"
            n1758 = local read "Saved Stage Positions"() -> (w4779:dbl[][])
            n1759 = Array Subset(array=w4779, index (row)=3 ("index"), length (row)=1 ("length"), index (col)=1 ("index"), length (col)=3 ("length")) -> (w4784:dbl[][])
            n1760 = Reshape Array(w4784, 3 ("dimension size")) -> (w4782:dbl[])
            n1761 = Array To Cluster(array=w4782) -> (cluster=w4781:cluster{"[0]":dbl, "[1]":dbl, "[2]":dbl})
            n1762 = call "Set Stage Position.vi"("Position"=w4781, "error in"=w4777, "VISA resource name in"=w4778) -> ()  [unwired: 3 out]
          }
          frame #2 {
            w4788 = FALSE ("Value (Signaling)")
            # "TURNS TRAPS OFF SO THAT\nBEADS REMAIN AT DUMP \nBEADS POSITION"
            n1763 = property on="Trap 1 (ON/OFF)" class="Bool (strict)"("Val(Sgnl)"=w4788) -> ()  [unwired: 2 in, 2 out]
            n1764 = property on="Trap 2 (ON/OFF)" class="Bool (strict)"("Val(Sgnl)"=w4788) -> ()  [unwired: 2 in, 2 out]
            n1765 = call <vilib>:"Beep.vi"() -> ()  [unwired: 3 in, 9 out]
          }
          frame #3 {
            # "MOVES STAGE BACK TO THE\nANTIDIG CAPILARY BY CALLING\nTHE Move Cap. 2 SCRIPT"
            n1766 = property on="Move Cap. 2 (ADig Left)" class="Bool (strict)"("Val(Sgnl)"=TRUE ("Value (Signaling)")) -> ()  [unwired: 2 in, 2 out]
          }
        }
      }
      event "Dip for Protein": Value Change {
        n1767 = event-data() -> ()  [unwired: 1 in, 5 out]
        n1768 = flat-sequence {
          tunnel: w4796 -> [w4800]
          tunnel: w4797 -> [w4801]
          tunnel: [w4801] -> w4791
          tunnel: [w4800] -> w4790
          tunnel: [w4804] -> w4794
          tunnel: [w4803] -> w4792
          tunnel: w4791 -> [w4807]
          tunnel: w4790 -> [w4806]
          tunnel: [w4817] -> w4795
          tunnel: w4794 -> [w4817]
          tunnel: [w4816] -> w4793
          tunnel: w4792 -> [w4816]
          tunnel: w4795 -> [w4822]
          tunnel: w4793 -> [w4821]
          frame #0 {
            n1769 = case shown="True" "Move Trap Before?" {
              frame False {
              }
              frame True {
                n1770 = property on="Trap Delta (MHz)" class="DigNum (strict)"("Val(Sgnl)"="Dip Trap Delta 1 (MHz)") -> ()  [unwired: 2 in, 2 out]
              }
            }
          }
          frame #1 {
            n1771 = local read "Saved Stage Positions"() -> (w4805:dbl[][])
            n1772 = Array Subset(array=w4805, index (row)=4 ("index"), length (row)=1 ("length"), index (col)=1 ("index"), length (col)=3 ("length")) -> (w4812:dbl[][])
            n1773 = Reshape Array(w4812, 3 ("dimension size")) -> (w4810:dbl[])
            n1774 = Array To Cluster(array=w4810) -> (cluster=w4809:cluster{"[0]":dbl, "[1]":dbl, "[2]":dbl})
            n1775 = call "Set Stage Position.vi"("Position"=w4809, "error in"=w4806, "VISA resource name in"=w4807) -> ("error out"=w4803:errorcluster, "VISA resource name out"=w4804:refnum<visa-resource-name>)  [unwired: 1 out]
          }
          frame #2 {
            n1776 = Multiply(x="Duration (s)", y=1000.0) -> (x*y=w4818:dbl)
            n1777 = Wait (ms)(milliseconds to wait=w4818) -> ()  [unwired: 1 out]
          }
          frame #3 {
            n1778 = local read "Saved Stage Positions"() -> (w4823:dbl[][])
            n1779 = Array Subset(array=w4823, index (row)=2 ("index"), length (row)=1 ("length"), index (col)=1 ("index"), length (col)=3 ("length")) -> (w4828:dbl[][])
            n1780 = Reshape Array(w4828, 3 ("dimension size")) -> (w4826:dbl[])
            n1781 = Array To Cluster(array=w4826) -> (cluster=w4825:cluster{"[0]":dbl, "[1]":dbl, "[2]":dbl})
            n1782 = call "Set Stage Position.vi"("Position"=w4825, "error in"=w4821, "VISA resource name in"=w4822) -> ()  [unwired: 3 out]
          }
          frame #4 {
            n1783 = case shown="True" "Move Trap After?" {
              frame False {
              }
              frame True {
                n1784 = property on="Trap Delta (MHz)" class="DigNum (strict)"("Val(Sgnl)"="Dip Trap Delta 2 (MHz)") -> ()  [unwired: 2 in, 2 out]
              }
            }
          }
          frame #5 {
            n1785 = case shown="True" "Green ON After?" {
              frame False {
              }
              frame True {
                n1786 = property on="Green Laser ON/Interlacing" class="Bool (strict)"("Val(Sgnl)"=TRUE ("Value (Signaling)")) -> ()  [unwired: 2 in, 2 out]
              }
            }
          }
          frame #6 {
            n1787 = Wait (ms)(milliseconds to wait=u32 500) -> ()  [unwired: 1 out]
          }
          frame #7 {
            n1788 = case shown="True" "Save Data After?" {
              frame False {
              }
              frame True {
                n1789 = property on="Start Saving" class="Bool (strict)"("Val(Sgnl)"=TRUE ("Value (Signaling)")) -> ()  [unwired: 2 in, 2 out]
              }
            }
          }
        }
      }
      event "Profile": Value Change {
        n1790 = event-data() -> ()  [unwired: 1 in, 5 out]
        n1791 = flat-sequence {
          tunnel: w4847 -> [w4850]
          tunnel: w4846 -> [w4858]
          tunnel: [w4852] -> w4845
          tunnel: [w4851] -> w4844
          tunnel: [w4849] -> w4842
          tunnel: [w4848] -> w4839
          tunnel: w4845 -> [w4865]
          tunnel: w4844 -> [w4864]
          tunnel: [w4862] -> w4843
          tunnel: w4842 -> [w4863]
          tunnel: [w4861] -> w4841
          tunnel: [w4860] -> w4840
          tunnel: w4839 -> [w4860]
          tunnel: w4843 -> [w4869]
          tunnel: w4841 -> [w4868]
          tunnel: w4840 -> [w4867]
          frame #0 {
            n1792 = call "Read Stage Position.vi"("error in"=w4858, "VISA resource name in"=w4850) -> ("Current Position"=w4848:cluster{dbl, dbl, dbl}, "error out"=w4851:errorcluster, "VISA resource name out"=w4849:refnum<visa-resource-name>)  [unwired: 1 out]
            "Current Position" <- w4848
            n1793 = local write "Stage Control Serial Error"(w4851) -> ()
            n1794 = Unbundle(w4848) -> (w4855:dbl, w4857:dbl, w4853:dbl)
            n1795 = Add(x=w4857, y="Y change (mm)") -> (x+y=w4854:dbl)
            n1796 = Bundle(w4855, w4854, w4853) -> (w4852:cluster{dbl, dbl, dbl})  [unwired: 1 in]
          }
          frame #1 {
            # "move to new position and start saving"
            n1797 = local write "Stage Moving"(TRUE ("Stage Moving")) -> ()
            n1798 = local write "Start Saving"(TRUE ("Start Saving")) -> ()
            n1799 = call "Set Stage Position.vi"("Position"=w4865, "error in"=w4864, "VISA resource name in"=w4863) -> ("error out"=w4861:errorcluster, "VISA resource name out"=w4862:refnum<visa-resource-name>)  [unwired: 1 out]
          }
          frame #2 {
            # "go back to start"
            n1800 = call "Set Stage Position.vi"("Position"=w4867, "error in"=w4868, "VISA resource name in"=w4869) -> ()  [unwired: 3 out]
          }
          frame #3 {
            # "stop saving"
            n1801 = local write "Stop Saving"(TRUE ("Stop Saving")) -> ()
            n1802 = local write "Stage Moving"(FALSE ("Stage Moving")) -> ()
          }
        }
      }
      event "Move to Position 1", "Move to Position 2", "Move to Position 3", "Move to Position 4", "Move to Position 5", "Lower Ch. Cap.": Value Change {
        n1803 = event-data() -> ()  [unwired: 1 in, 5 out]
        n1804 = Or(x="Move to Position 5", y="Lower Ch. Cap.") -> (x .or. y?=w4875:bool)
        n1805 = Build Array("Move to Position 1", "Move to Position 2", "Move to Position 3", "Move to Position 4", w4875) -> (w4878:bool[])
        n1806 = Boolean Array To Number(Boolean array=w4878) -> (number=w4877:u32)
        n1807 = Logarithm Base 2(1:w4877) -> (0:w4876:dbl)
        n1808 = flat-sequence {
          tunnel: w4876 -> [w4887]
          tunnel: w4873 -> [w4885]
          tunnel: w4872 -> [w4884]
          frame #0 {
            n1809 = local read "Saved Stage Positions"() -> (w4895:dbl[][])
            n1810 = Array Subset(array=w4895, index (row)=w4887, length (row)=1 ("length"), index (col)=1 ("index"), length (col)=3 ("length")) -> (w4892:dbl[][])
            n1811 = Reshape Array(w4892, 3 ("dimension size")) -> (w4890:dbl[])
            n1812 = Array To Cluster(array=w4890) -> (cluster=w4889:cluster{"[0]":dbl, "[1]":dbl, "[2]":dbl})
            n1813 = call "Set Stage Position.vi"("Position"=w4889, "error in"=w4884, "VISA resource name in"=w4885) -> ("error out"=w4888:errorcluster)  [unwired: 2 out]
            n1814 = local write "Stage Moving"(TRUE ("Stage Moving")) -> ()
            n1815 = local write "Stage Control Serial Error"(w4888) -> ()
          }
          frame #1 {
            n1816 = local write "Stage Moving"(FALSE ("Stage Moving")) -> ()
            n1817 = call <vilib>:"Beep.vi"() -> ()  [unwired: 3 in, 9 out]
          }
        }
      }
      event "Got ADig bead": Value Change {
        n1818 = event-data() -> ()  [unwired: 1 in, 5 out]
        n1819 = property on="Move Cap. 1 (DNA Right)" class="Bool (strict)"("Val(Sgnl)"=TRUE ("Value (Signaling)")) -> ()  [unwired: 2 in, 2 out]
        n1820 = property on="Inject Pump 3" class="Bool (strict)"("Val(Sgnl)"=FALSE ("Value (Signaling)")) -> ()  [unwired: 2 in, 2 out]
      }
      event "Got DNA bead": Value Change {
        n1821 = event-data() -> ()  [unwired: 1 in, 5 out]
        n1822 = property on="Cal/Data Acq. Spot" class="Bool (strict)"("Val(Sgnl)"=TRUE ("Value (Signaling)")) -> ()  [unwired: 2 in, 2 out]
        n1823 = property on="Inject Pump 1" class="Bool (strict)"("Val(Sgnl)"=FALSE ("Value (Signaling)")) -> ()  [unwired: 2 in, 2 out]
      }
      event "Take Stepping Data": Value Change {
        n1824 = event-data() -> ()  [unwired: 1 in, 5 out]
        n1825 = local read "Save ave N"() -> (w4912:dbl)
        n1826 = flat-sequence {
          tunnel: w4912 -> [w4914]
          tunnel: [w4914] -> w4907
          tunnel: [w4916] -> w4908
          tunnel: w4907 -> [w4916]
          tunnel: [w4918] -> w4909
          tunnel: w4908 -> [w4918]
          tunnel: [w4921] -> w4910
          tunnel: w4909 -> [w4921]
          tunnel: [w4923] -> w4911
          tunnel: w4910 -> [w4923]
          tunnel: [w4925] -> w4905
          tunnel: w4911 -> [w4925]
          tunnel: w4905 -> [w4928]
          tunnel: [w4928] -> w4904
          tunnel: w4904 -> [w4929]
          tunnel: [w4929] -> w4906
          tunnel: w4906 -> [w4935]
          frame #0 {
            n1827 = property on="Save ave N" class="DigNum (strict)"("Val(Sgnl)"="Save ave factor") -> ()  [unwired: 2 in, 2 out]
          }
          frame #1 {
            n1828 = Wait (ms)(milliseconds to wait=u32 100) -> ()  [unwired: 1 out]
          }
          frame #2 {
            n1829 = local read "Offset 2 Start (MHz)"() -> (w4920:dbl)
            n1830 = property on="Saved AOD Raster Scan Parameter Sets" class="Arr (strict)"("Index Values"=u32[] [2]) -> ()  [unwired: 2 in, 2 out]
            n1831 = property on="Trap Delta (MHz)" class="DigNum (strict)"("Val(Sgnl)"=w4920) -> ()  [unwired: 2 in, 2 out]
          }
          frame #3 {
            n1832 = property on="Load parameters" class="Bool (strict)"("Val(Sgnl)"=TRUE ("Value (Signaling)")) -> ()  [unwired: 2 in, 2 out]
          }
          frame #4 {
            n1833 = Wait (ms)(milliseconds to wait=u32 100) -> ()  [unwired: 1 out]
          }
          frame #5 {
            n1834 = property on="Trap Raster Scan" class="Bool (strict)"("Val(Sgnl)"=TRUE ("Value (Signaling)")) -> ()  [unwired: 2 in, 2 out]
          }
          frame #6 {
            n1835 = Wait (ms)(milliseconds to wait=u32 1000) -> ()  [unwired: 1 out]
          }
          frame #7 {
            n1836 = while {
              stop <- w4932 stop-if-true
              n1837 = local read "Raster Scanning..."() -> (w4934:bool)
              n1838 = local read "Saving..."() -> (w4933:bool)
              n1839 = Not(x=w4933) -> (.not. x?=w4930:bool)
              n1840 = Not(x=w4934) -> (.not. x?=w4931:bool)
              n1841 = And(x=w4931, y=w4930) -> (x .and. y?=w4932:bool)
            }
          }
          frame #8 {
            n1842 = property on="Save ave N" class="DigNum (strict)"("Val(Sgnl)"=w4935) -> ()  [unwired: 2 in, 2 out]
          }
        }
      }
      event "Step Size (nm)": Value Change {
        n1843 = event-data() -> ()  [unwired: 1 in, 5 out]
        n1844 = flat-sequence {
          frame #0 {
            n1845 = property on="Saved AOD Raster Scan Parameter Sets" class="Arr (strict)"("Index Values"=u32[] [1]) -> ()  [unwired: 2 in, 2 out]
          }
          frame #1 {
            n1846 = Multiply(x="N Steps", y="Step Size (nm)") -> (x*y=w4937:dbl)
            n1847 = property on="Scan Speed AOD (nm/s) 2" class="DigNum (strict)"("Value"="Step Size (nm)") -> ()  [unwired: 2 in, 2 out]
            n1848 = property on="Step Size AOD (nm) 2" class="DigNum (strict)"("Value"="Step Size (nm)") -> ()  [unwired: 2 in, 2 out]
            n1849 = property on="Scan Range AOD (nm) 2" class="DigNum (strict)"("Value"=w4937) -> ()  [unwired: 2 in, 2 out]
          }
        }
      }
      event "Take Detection Laser\nImage": Value Change {
        n1850 = event-data() -> ()  [unwired: 1 in, 5 out]
        n1851 = flat-sequence {
          tunnel: [w4965] -> w4955
          tunnel: [w4964] -> w4948
          tunnel: [w4963] -> w4940
          tunnel: [w4968] -> w4956
          tunnel: w4955 -> [w4968]
          tunnel: [w4967] -> w4949
          tunnel: w4948 -> [w4967]
          tunnel: [w4966] -> w4941
          tunnel: w4940 -> [w4966]
          tunnel: [w4972] -> w4957
          tunnel: w4956 -> [w4972]
          tunnel: [w4971] -> w4950
          tunnel: w4949 -> [w4971]
          tunnel: [w4970] -> w4942
          tunnel: w4941 -> [w4970]
          tunnel: [w4978] -> w4958
          tunnel: w4957 -> [w4978]
          tunnel: [w4977] -> w4951
          tunnel: w4950 -> [w4977]
          tunnel: [w4976] -> w4943
          tunnel: w4942 -> [w4976]
          tunnel: [w4982] -> w4959
          tunnel: w4958 -> [w4982]
          tunnel: [w4981] -> w4952
          tunnel: w4951 -> [w4981]
          tunnel: [w4980] -> w4944
          tunnel: w4943 -> [w4980]
          tunnel: [w4986] -> w4960
          tunnel: w4959 -> [w4986]
          tunnel: [w4985] -> w4953
          tunnel: w4952 -> [w4985]
          tunnel: [w4984] -> w4945
          tunnel: w4944 -> [w4984]
          tunnel: [w4990] -> w4961
          tunnel: w4960 -> [w4990]
          tunnel: [w4989] -> w4954
          tunnel: w4953 -> [w4989]
          tunnel: [w4988] -> w4946
          tunnel: w4945 -> [w4988]
          tunnel: w4961 -> [w4996]
          tunnel: w4954 -> [w4995]
          tunnel: [w4993] -> w4947
          tunnel: w4946 -> [w4993]
          tunnel: w4947 -> [w4997]
          frame #0 {
            n1852 = local read "Green Laser ON/Interlacing"() -> (w4965:bool)
            n1853 = local read "Green laser mode"() -> (w4964:enum32{"Laser ON", "Laser OFF", "Interlace"})
            n1854 = local read "Green FB On/Off"() -> (w4963:bool)
          }
          frame #1 {
            n1855 = property on="Green FB On/Off" class="Bool (strict)"("Val(Sgnl)"=FALSE ("Value (Signaling)")) -> ()  [unwired: 2 in, 2 out]
          }
          frame #2 {
            n1856 = property on="Green Laser ON/Interlacing" class="Bool (strict)"("Val(Sgnl)"=TRUE ("Value (Signaling)")) -> ()  [unwired: 2 in, 2 out]
            n1857 = property on="Flip Green Filter" class="Bool (strict)"("Val(Sgnl)"=TRUE ("Value (Signaling)")) -> ()  [unwired: 2 in, 2 out]
            n1858 = property on="Green laser mode" class="RadioBtnsControl (strict)"("Val(Sgnl)"=enum32{"Laser ON", "Laser OFF", "Interlace"}."Laser ON" ("Value (Signaling)")) -> ()  [unwired: 2 in, 2 out]
          }
          frame #3 {
            n1859 = Wait (ms)(milliseconds to wait=u32 500) -> ()  [unwired: 1 out]
          }
          frame #4 {
            n1860 = property on="Confocal Image" class="Bool (strict)"("Val(Sgnl)"=TRUE ("Value (Signaling)")) -> ()  [unwired: 2 in, 2 out]
          }
          frame #5 {
            n1861 = Wait (ms)(milliseconds to wait=u32 2000) -> ()  [unwired: 1 out]
          }
          frame #6 {
            n1862 = while {
              stop <- w4991 stop-if-true
              n1863 = local read "Saving..."() -> (w4992:bool)
              n1864 = Not(x=w4992) -> (.not. x?=w4991:bool)
            }
          }
          frame #7 {
            n1865 = property on="Flip Green Filter" class="Bool (strict)"("Val(Sgnl)"=TRUE ("Value (Signaling)")) -> ()  [unwired: 2 in, 2 out]
            n1866 = property on="Green Laser ON/Interlacing" class="Bool (strict)"("Val(Sgnl)"=w4996) -> ()  [unwired: 2 in, 2 out]
            n1867 = property on="Green laser mode" class="RadioBtnsControl (strict)"("Val(Sgnl)"=w4995) -> ()  [unwired: 2 in, 2 out]
          }
          frame #8 {
            n1868 = property on="Green FB On/Off" class="Bool (strict)"("Val(Sgnl)"=w4997) -> ()  [unwired: 2 in, 2 out]
          }
        }
      }
      event "Stop All": Value Change {
        n1869 = event-data() -> ()  [unwired: 1 in, 5 out]
        n1870 = local read "Stop All"() -> (w4998:bool)
      }
    }
    n1871 = node-c288() -> ()  [unwired: 1 in, 1 out]
  }
  n1872 = timed-loop "Mouse control: trap position (AOM deflection), set confocal spot from image" {
    tunnel: [w5000] -> w156
    tunnel: w8 -> [w4999]
    timing: w52 -> [_]
    timing-out: [_] -> w51
    stop <- w5000 stop-if-true
    n1873 = node-c288() -> ()  [unwired: 2 out]
    n1874 = event shown="[0] \"Pane\": Mouse Down" {
      selector: _ -> [_ _]
      dyn-events: _ -> [_ _]
      timeout: _ -> [_ _]
      tunnel: w4999 -> [w5003 _]
      event Mouse Down {
        n1875 = event-data() -> ("Time"=w5005:u32, "Coords"=w5004:T7, "Button"=w5006:u16)  [unwired: 6 out]
        n1876 = case shown="1" w5006 {
          tunnel: w5005 -> [_ _ w5109]
          tunnel: w5004 -> [_ w5043 w5107]
          tunnel: w5003 -> [_ _ w5105]
          frame 0, Default {
          }
          frame 1 {
            n1877 = property on="APD 2" class="ImageControl"() -> ("Displayed Image Position"=w5013:cluster{"Left":i32, "Top":i32})  [unwired: 2 in, 2 out]
            n1878 = property on="APD 1" class="ImageControl"() -> ("Displayed Image Position"=w5042:cluster{"Left":i32, "Top":i32})  [unwired: 2 in, 2 out]
            n1879 = property on="Detection Laser X" class="ImageControl"() -> ("Displayed Image Position"=w5039:cluster{"Left":i32, "Top":i32})  [unwired: 2 in, 2 out]
            n1880 = property on="Detection Laser Y" class="ImageControl"() -> ("Displayed Image Position"=w5038:cluster{"Left":i32, "Top":i32})  [unwired: 2 in, 2 out]
            n1881 = property on="APD 2" class="ImageControl"() -> ("Displayed Image Size"=w5012:cluster{"Width":u32, "Height":u32})  [unwired: 2 in, 2 out]
            n1882 = property on="APD 1" class="ImageControl"() -> ("Displayed Image Size"=w5040:cluster{"Width":u32, "Height":u32})  [unwired: 2 in, 2 out]
            n1883 = property on="Detection Laser X" class="ImageControl"() -> ("Displayed Image Size"=w5041:cluster{"Width":u32, "Height":u32})  [unwired: 2 in, 2 out]
            n1884 = property on="Detection Laser Y" class="ImageControl"() -> ("Displayed Image Size"=w5037:cluster{"Width":u32, "Height":u32})  [unwired: 2 in, 2 out]
            n1885 = Unbundle By Name(w5012) -> ("Width"=w5009:u32, "Height"=w5008:u32)
            n1886 = Unbundle By Name(w5013) -> ("Left"=w5011:i32, "Top"=w5010:i32)
            n1887 = Unbundle By Name(w5040) -> ("Width"=w5034:u32, "Height"=w5033:u32)
            n1888 = Unbundle By Name(w5041) -> ("Width"=w5030:u32, "Height"=w5029:u32)
            n1889 = Unbundle By Name(w5037) -> ("Width"=w5026:u32, "Height"=w5025:u32)
            n1890 = Unbundle By Name(w5042) -> ("Left"=w5036:i32, "Top"=w5035:i32)
            n1891 = Unbundle By Name(w5039) -> ("Left"=w5032:i32, "Top"=w5031:i32)
            n1892 = Unbundle By Name(w5038) -> ("Left"=w5028:i32, "Top"=w5027:i32)
            n1893 = Bundle("Left"=w5011, "Top"=w5010, "Width"=w5009, "Height"=w5008) -> (w5007:T43)  [unwired: 1 in]
            n1894 = Bundle("Left"=w5036, "Top"=w5035, "Width"=w5034, "Height"=w5033) -> (w5024:T43)  [unwired: 1 in]
            n1895 = Bundle("Left"=w5032, "Top"=w5031, "Width"=w5030, "Height"=w5029) -> (w5023:T43)  [unwired: 1 in]
            n1896 = Bundle("Left"=w5028, "Top"=w5027, "Width"=w5026, "Height"=w5025) -> (w5022:T43)  [unwired: 1 in]
            n1897 = Build Cluster Array(w5007, w5024, w5023, w5022) -> (w5021:T44)
            n1898 = for {
              tunnel: w5043 -> [w5054]
              tunnel: w5021 -> [w5055] mode=indexing
              shift-right: [w5052] -> w5019
              shift-left: TRUE -> [w5053]
              shift-right: [w5051] -> w5017
              shift-left: _ -> [w5047]
              shift-right: [w5050] -> w5016
              shift-left: _ -> [w5046]
              shift-right: [w5049] -> w5015
              shift-left: _ -> [w5045]
              shift-right: [w5048] -> w5014
              shift-left: _ -> [w5044]
              n1899 = case shown="True" w5053 {
                selector: w5053 -> [w5060 _]
                tunnel: w5055 -> [_ w5069]
                tunnel: w5054 -> [_ w5067]
                tunnel: [w5060 w5065] -> w5052
                tunnel: [w5059 w5064] -> w5051
                tunnel: [w5058 w5063] -> w5050
                tunnel: [w5057 w5062] -> w5049
                tunnel: [w5056 w5061] -> w5048
                tunnel: w5047 -> [w5059 _]
                tunnel: w5046 -> [w5058 _]
                tunnel: w5045 -> [w5057 _]
                tunnel: w5044 -> [w5056 _]
                frame False {
                }
                frame True {
                  n1900 = Unbundle(w5069) -> (w5068:T43)
                  n1901 = call "isclickinwindow.vi"("Image Param"=w5068, "Point32"=w5067) -> ("4 Y"=w5061:i32, "3 Height"=w5062:i32, "2 X"=w5063:i32, "1 Width"=w5064:i32, "In image?"=w5066:bool)  [unwired: 1 in]
                  n1902 = Not(x=w5066) -> (.not. x?=w5065:bool)
                }
              }
            }
            n1903 = Not(x=w5019) -> (.not. x?=w5018:bool)
            n1904 = case shown="True" w5018 {
              tunnel: w5016 -> [_ w5082]
              tunnel: w5014 -> [_ w5081]
              tunnel: w5017 -> [_ w5080]
              tunnel: w5015 -> [_ w5079]
              frame False {
              }
              frame True {
                w5075 = FALSE ("Get Point")
                n1905 = local read "Scan lines (y)"() -> (w5084:u64)
                n1906 = local read "Actual MCL Inc (V)"() -> (w5076:dbl)
                n1907 = local read "Scan steps (MCL)"() -> (w5083:u64)
                n1908 = Divide "Y Pix/step"(x=w5079, y=w5084) -> (x/y=w5091:dbl)
                n1909 = Divide "Y V/pix"(x=w5076, y=w5091) -> (x/y=w5090:dbl)
                n1910 = Divide "Y half step offset"(x=w5076, y=2.0) -> (x/y=w5092:dbl)
                n1911 = Divide "X pix/step"(x=w5080, y=w5083) -> (x/y=w5089:dbl)
                n1912 = Negate(x=w5092) -> (-x=w5093:dbl)
                n1913 = local read "Initial Y"() -> (w5099:dbl)
                n1914 = Multiply(x=w5081, y=w5090) -> (x*y=w5100:dbl)
                n1915 = Divide "X half step offset"(x=w5076, y=2.0) -> (x/y=w5086:dbl)
                n1916 = Divide "X V/pix"(x=w5076, y=w5089) -> (x/y=w5088:dbl)
                n1917 = Multiply(x=w5076, y=w5083) -> (x*y=w5095:dbl)
                n1918 = Compound Arithmetic op=ADD(w5093, w5100, w5099) -> (w5077:dbl)
                "Pointer Y (V)" <- w5077
                n1919 = Multiply(x=w5088, y=w5082) -> (x*y=w5097:dbl)
                n1920 = Negate(x=w5086) -> (-x=w5085:dbl)
                n1921 = local read "Initial X"() -> (w5098:dbl)
                n1922 = Negate(x=w5097) -> (-x=w5096:dbl)
                n1923 = Compound Arithmetic op=ADD(w5085, w5095, w5098, w5096) -> (w5078:dbl)
                "Pointer X (V)" <- w5078
                n1924 = Or(x="Set X Only", y="Set Confocal Spot (X-Y)") -> (x .or. y?=w5071:bool)
                n1925 = Or(x="Set Confocal Spot (X-Y)", y="Set Y Only") -> (x .or. y?=w5070:bool)
                n1926 = case shown="True" w5071 {
                  tunnel: w5078 -> [_ w5101]
                  frame False {
                  }
                  frame True {
                    n1927 = property on="AO2" class="Slide (strict)"("Val(Sgnl)"=w5101) -> ()  [unwired: 2 in, 2 out]
                  }
                }
                n1928 = case shown="True" w5070 {
                  tunnel: w5077 -> [_ w5102]
                  frame False {
                  }
                  frame True {
                    n1929 = property on="AO1" class="Slide (strict)"("Val(Sgnl)"=w5102) -> ()  [unwired: 2 in, 2 out]
                  }
                }
                n1930 = local write "Set Confocal Spot (X-Y)"(w5075) -> ()
                n1931 = local write "Set X Only"(w5075) -> ()
                n1932 = local write "Set Y Only"(w5075) -> ()
              }
            }
          }
          frame 3 {
            n1933 = local read "BD 2 Frequency 1 (MHz)"() -> (w5103:dbl)
            n1934 = local read "BD 1 Frequency 1 (MHz)"() -> (w5104:dbl)
            n1935 = local write "Manipulating Trap"(TRUE ("Manipulating Trap")) -> ()
            n1936 = local write "Coords"(T7 {"Horizontal"=0, "Vertical"=0} ("Coords")) -> ()
            n1937 = while {
              tunnel: w5109 -> [w5114]
              tunnel: w5107 -> [w5113]
              tunnel: w5105 -> [w5112]
              tunnel: w5104 -> [w5111]
              tunnel: w5103 -> [w5110]
              stop <- w5115 stop-if-true
              n1938 = event shown="[0] \"Pane\": Mouse Move" {
                selector: _ -> [_ _]
                dyn-events: _ -> [_ _]
                timeout: _ -> [_ _]
                tunnel: ["Force Manip Abort" w5179] -> w5115
                tunnel: w5114 -> [w5122 _]
                tunnel: w5113 -> [w5120 _]
                tunnel: w5112 -> [w5119 _]
                tunnel: w5111 -> [w5118 _]
                tunnel: w5110 -> [w5117 _]
                event Mouse Move {
                  n1939 = event-data() -> ("Time"=w5123:u32, "Coords"=w5124:T7)  [unwired: 3 out]
                  n1940 = Less?(x=w5123, y=w5122) -> (x < y?=w5121:bool)
                  n1941 = case "Makes sure old motion events prior to mouse click aren't used" shown="False" w5121 {
                    tunnel: w5124 -> [w5166 _]
                    tunnel: w5120 -> [w5167 _]
                    tunnel: w5119 -> [w5144 _]
                    tunnel: w5118 -> [w5140 _]
                    tunnel: w5117 -> [w5139 _]
                    frame False {
                      n1942 = Subtract(x=w5166, y=w5167) -> (x-y=w5165:T7)
                      "Coords" <- w5165
                      n1943 = local read "Y RF Frequency Limits (MHz)"() -> (w5125:T16)
                      n1944 = To Double Precision Float(number=w5165) -> (double precision float=w5164:cluster{"Horizontal":dbl, "Vertical":dbl})
                      n1945 = Multiply(x=cluster{"Horizontal":dbl, "Vertical":dbl} {"Horizontal"=-1.0, "Vertical"=1.0}, y="Manipulation Scaling") -> (x*y=w5160:cluster{"Horizontal":dbl, "Vertical":dbl})
                      n1946 = local read "X RF Frequency Limits (MHz)"() -> (w5126:T16)
                      n1947 = Multiply(x=w5164, y=w5160) -> (x*y=w5162:cluster{"Horizontal":dbl, "Vertical":dbl})
                      n1948 = Unbundle By Name(w5162) -> ("Horizontal"=w5157:dbl, "Vertical"=w5161:dbl)
                      n1949 = Unbundle By Name(w5125) -> ("Maximum"=w5128:dbl, "Minimum"=w5127:dbl)
                      n1950 = Boolean To (0,1)(Boolean="Manip. X?") -> (0, 1=w5155:i16)
                      n1951 = Boolean To (0,1)(Boolean="Manip. Y?") -> (0, 1=w5152:i16)
                      n1952 = local read "BD 1 Frequency 2 (MHz)"() -> (w5142:dbl)
                      n1953 = Multiply(x=w5161, y=w5152) -> (x*y=w5154:dbl)
                      n1954 = Multiply(x=w5155, y=w5157) -> (x*y=w5158:dbl)
                      n1955 = local read "BD 2 Frequency 2 (MHz)"() -> (w5141:dbl)
                      n1956 = Unbundle By Name(w5126) -> ("Maximum"=w5130:dbl, "Minimum"=w5129:dbl)
                      n1957 = Add(x=w5139, y=w5154) -> (x+y=w5132:dbl)
                      n1958 = Add(x=w5140, y=w5158) -> (x+y=w5134:dbl)
                      n1959 = In Range and Coerce(upper limit=w5130, x=w5134, lower limit=w5129) -> (coerced(x)=w5133:dbl)  [unwired: 1 out]
                      n1960 = In Range and Coerce(upper limit=w5128, x=w5132, lower limit=w5127) -> (coerced(x)=w5131:dbl)  [unwired: 1 out]
                      n1961 = Subtract(x=w5133, y=w5142) -> (x-y=w5151:dbl)
                      n1962 = Subtract(x=w5131, y=w5141) -> (x-y=w5150:dbl)
                      n1963 = Square(x=w5151) -> (x^2=w5149:dbl)
                      n1964 = Square(x=w5150) -> (x^2=w5148:dbl)
                      n1965 = Add(x=w5149, y=w5148) -> (x+y=w5147:dbl)
                      n1966 = Square Root(x=w5147) -> (sqrt(x)=w5143:dbl)
                      n1967 = In Range and Coerce(upper limit="Limit Max (MHz)", x=w5143, lower limit="Limit Min (MHz)") -> (In Range?=w5136:bool)  [unwired: 1 out]
                      n1968 = Not(x="Limits Enable") -> (.not. x?=w5135:bool)
                      n1969 = Or(x=w5136, y=w5135) -> (x .or. y?=w5137:bool)
                      n1970 = case shown="True" w5137 {
                        tunnel: w5144 -> [_ w5177]
                        tunnel: w5143 -> [_ w5168]
                        tunnel: w5133 -> [_ w5175]
                        tunnel: w5142 -> [_ w5174]
                        tunnel: w5131 -> [_ w5173]
                        tunnel: w5141 -> [_ w5172]
                        tunnel: w5126 -> [_ w5170]
                        tunnel: w5125 -> [_ w5169]
                        frame False {
                        }
                        frame True {
                          n1971 = local read "BD 1 Frequency 3 (MHz)"() -> (w5176:dbl)
                          n1972 = local read "BD 2 Frequency 3 (MHz)"() -> (w5171:dbl)
                          n1973 = local write "Trap Delta (MHz)"(w5168) -> ()
                          n1974 = property on="Initial delta (MHz)" class="DigNum (strict)"("Val(Sgnl)"=w5168) -> ()  [unwired: 2 in, 2 out]
                          n1975 = call "set RF board frequency - interlace.vi"("Board 2 Frequency Limits"=w5169, "Board 1 Frequency Limits"=w5170, "FPGA VI Reference In"=w5177, "Board 2 Frequency 3 (MHz)"=w5171, "Board 1 Frequency 3 (MHz)"=w5176, "Board 2 Frequency 2 (MHz)"=w5172, "Board 2 Frequency 1 (MHz)"=w5173, "Board 1 Frequency 2 (MHz)"=w5174, "Board 1 Frequency 1  (MHz)"=w5175) -> ()  [unwired: 1 in, 2 out]
                          n1976 = local write "BD 2 Frequency 1 (MHz)"(w5173) -> ()
                          n1977 = local write "BD 1 Frequency 1 (MHz)"(w5175) -> ()
                        }
                      }
                    }
                    frame True {
                    }
                  }
                }
                event Mouse Up {
                  n1978 = event-data() -> ("Button"=w5178:u16)  [unwired: 8 out]
                  n1979 = case shown="3" w5178 {
                    tunnel: [FALSE TRUE] -> w5179
                    frame 0, Default {
                    }
                    frame 3 {
                      n1980 = local write "Manipulating Trap"(FALSE ("Manipulating Trap")) -> ()
                    }
                  }
                }
              }
            }
          }
        }
      }
      event Mouse Move {
        n1981 = event-data() -> ()  [unwired: 6 out]
      }
    }
    n1982 = local read "Stop All"() -> (w5000:bool)
    n1983 = node-c288() -> ()  [unwired: 2 out]
  }
  n1984 = flat-sequence "Video" {
    tunnel: [w5191] -> w38
    tunnel: w38 -> [w5232]
    frame #0 {
      n1985 = while {
        stop <- w5184 continue-if-true
        n1986 = call "Close Video Capture.vi"() -> ("error code OUT"=w5186:i32)
        n1987 = Equal?(x=w5186, y=0) -> (x = y?=w5184:bool)
      }
      n1988 = local write "Stop All"(FALSE ("Stop All")) -> ()
    }
    frame #1 {
      n1989 = call "DMR_Init.vi"() -> ()  [unwired: 3 out]
    }
    frame #2 {
      # "Setting the destination format to Mono8 makes sure that the image can be displayed in the intensity plot."
      n1990 = call "DMR_GetDevice.vi"("search string IN"="DE019116701") -> ("device handle OUT"=w5209:i32)  [unwired: 4 in, 2 out]
      n1991 = call "DMR_OpenDevice.vi"("device handle IN"=w5209) -> ("driver handle OUT"=w5192:i32)  [unwired: 4 out]
      n1992 = call "DMR_FindList.vi"("flags IN"=u32 0 ("flags"), "list name IN"="" ("String"), "list type IN"=T45."camera descriptions", "driver handle IN"=w5192) -> ("list handle OUT"=w5195:i32)  [unwired: 2 out]
      n1993 = call "DMR_FindList.vi"("flags IN"=u32 0 ("flags"), "list name IN"="Base", "list type IN"=T45."setting", "driver handle IN"=w5192) -> ("list handle OUT"=w5193:i32)  [unwired: 2 out]
      n1994 = call "OBJ_GetHandle.vi"("object name IN"="VideoStandard", "list handle IN"=w5195) -> ("object handle OUT"=w5189:i32)  [unwired: 3 out]
      n1995 = call "OBJ_GetHandle.vi"("object name IN"="PixelFormat", "list handle IN"=w5193) -> ("object handle OUT"=w5203:i32)  [unwired: 3 out]
      n1996 = call "OBJ_SetS.vi"("value index IN"=0, "value IN"="NTSC M", "object handle IN"=w5189) -> ()  [unwired: 2 out]
      n1997 = call "OBJ_SetS.vi"("value index IN"=0, "value IN"="Mono8" ("value"), "object handle IN"=w5203) -> ()  [unwired: 2 out]
      n1998 = call "OBJ_GetHandle.vi"("object name IN"="VideoChannel", "list handle IN"=w5193) -> ("object handle OUT"=w5199:i32)  [unwired: 3 out]
      n1999 = while {
        tunnel: [w5214] -> w5191
        tunnel: w5192 -> [w5211]
        stop <- w5212 continue-if-true
        n2000 = call "DMR_ImageRequestSingle.vi"("request control IN"=0, "driver handle IN"=w5211) -> ("error code OUT"=w5213:i32, "driver handle OUT"=w5214:i32)  [unwired: 2 out]
        n2001 = Equal To 0?(x=w5213) -> (x = 0?=w5212:bool)
      }
      n2002 = call "OBJ_SetI.vi"("value index IN"=0, "value IN"=3 ("Video channel"), "object handle IN"=w5199) -> ()  [unwired: 2 out]
    }
    frame #3 {
      w5220 = T17 0 items=["Grayscale (U8)", "Grayscale (I16)", "Grayscale (SGL)", "Complex (CSG)", "RGB (U32)", "HSL (U32)", "RGB (U64)"] ("Image Type")
      w5228 = T17 0 items=["Grayscale (U8)", "Grayscale (I16)", "Grayscale (SGL)", "Complex (CSG)", "RGB (U32)", "HSL (U32)", "RGB (U64)"] ("Image Type")
      n2003 = for "Create Greyscale map" {
        N: 256 -> [_]
        tunnel: [w5234] -> w5217 mode=indexing
        workers-P: _ -> [_]
        i -> [w5237]
        n2004 = To Unsigned Byte Integer(number=w5237) -> (unsigned 8bit integer=w5233:u8)
        n2005 = Join Numbers(hi=w5233, lo=w5233) -> ((hi.lo)=w5236:u16)
        n2006 = Join Numbers(hi=w5233, lo=w5233) -> ((hi.lo)=w5235:u16)
        n2007 = Join Numbers(hi=w5236, lo=w5235) -> ((hi.lo)=w5234:u32)
      }
      n2008 = call "IMAQ Create"("Image Name"="Scaled video", "Image Type"=w5220) -> ("New Image"=w5219:T2)  [unwired: 2 in, 2 out]
      n2009 = call "IMAQ Create"("Image Name"="Main video", "Image Type"=w5228) -> ("New Image"=w5229:T2)  [unwired: 2 in, 2 out]
      n2010 = node-c288(0 ("Processor")) -> (w5227:T23)  [unwired: 3 out]
      n2011 = Initialize Array(u32 0 ("Window Number (0...15)"), 480 ("dimension size"), 640 ("dimension size")) -> (w5222:u32[][])
      n2012 = timed-loop {
        tunnel: w5232 -> [w5254]
        tunnel: [w5253] -> w5231
        tunnel: w5229 -> [w5252]
        timing: w5227 -> [_]
        timing-out: [_] -> w5226
        tunnel: w5222 -> [w5241]
        tunnel: w5219 -> [w5239]
        tunnel: w5217 -> [w5238]
        stop <- w5240 stop-if-true
        # "This block performs the \nactual image capture."
        n2013 = node-c288() -> ()  [unwired: 2 out]
        n2014 = local read "Stop All"() -> (w5240:bool)
        n2015 = Reciprocal(x="Video Capture Rate (Hz)") -> (1/x=w5244:dbl)
        n2016 = Multiply(x=w5244, y=1000.0) -> (x*y=w5242:dbl)
        n2017 = call "DMR_ImageRequestWaitFor.vi"("queue number IN"=0, "timeout(ms) IN"=500, "driver handle IN"=w5254) -> ("error code OUT"=w5258:i32, "request number OUT"=w5255:i32, "driver handle OUT"=w5256:i32)
        n2018 = feedback #31(T46 refnum ("Avi Refnum")) -> (w5246:T46)
        n2019 = case shown="True" "New Video File" {
          tunnel: [T46 refnum ("Avi Refnum") w5275] -> w5248
          tunnel: [FALSE TRUE] -> w5249
          tunnel: w5246 -> [_ w5271]
          frame False {
          }
          frame True {
            n2020 = call "Create new save file.vi"("Ext"=".avi" ("string"), "Index In"="Video Index") -> ("Path Out"=w5267:path, "Index Out"=w5268:dbl)  [unwired: 1 in]
            "Path Out" <- w5267
            n2021 = Not Equal?(x=w5271, y=T46 refnum ("Avi Refnum")) -> (x != y?=w5272:bool)
            n2022 = Increment(x=w5268) -> (x+1=w5277:dbl)
            n2023 = case shown="True" w5272 {
              tunnel: w5271 -> [_ w5278]
              frame False {
              }
              frame True {
                n2024 = call "IMAQ AVI Close"("Avi Refnum"=w5278) -> ()  [unwired: 1 in, 10 out]
              }
            }
            n2025 = local write "Video Index"(w5277) -> ()
            n2026 = call "IMAQ AVI Create"("Frames Per Second"=u32 30, "AVI Path"=w5267) -> ("Avi Refnum"=w5275:T46)  [unwired: 5 in, 4 out]
          }
        }
        n2027 = Equal To 0?(x=w5258) -> (x = 0?=w5257:bool)
        n2028 = Select(t=w5248, s=w5249, f=w5246) -> (s? t:f=w5247:T46)
        n2029 = feedback-in #31(w5247) -> ()
        n2030 = case shown="True" w5257 {
          tunnel: w5256 -> [w5279 w5304]
          tunnel: w5255 -> [_ w5303]
          tunnel: [w5279 w5300] -> w5253
          tunnel: w5252 -> [_ w5284]
          tunnel: w5241 -> [_ w5288]
          tunnel: w5247 -> [_ w5286]
          tunnel: w5239 -> [_ w5281]
          tunnel: w5238 -> [_ w5280]
          frame False {
          }
          frame True {
            w5294 = u32 0 ("X-offset IN")
            n2031 = call "DMR_GetImageRequestBufferData.vi"("driver handle IN"=w5304, "request number IN"=w5303) -> ("width OUT"=w5293:i32, "height OUT"=w5292:i32, "driver handle OUT"=w5299:i32, "request number OUT"=w5298:i32, "bytes per pixel OUT"=w5295:i32)  [unwired: 13 out]
            n2032 = call "DMR_GetImageRequestBufferImageData.vi"("driver handle IN"=w5299, "request number IN"=w5298, "bytes per pixel IN"=w5295, "X-offset IN"=w5294, "Y-offset IN"=w5294, "height IN"=w5292, "width IN"=w5293) -> ("driver handle OUT"=w5297:u32, "request number OUT"=w5296:u32, "image OUT"=w5289:u32[][])  [unwired: 10 out]
            n2033 = call "DMR_ImageRequestUnlock.vi"("request number IN"=w5296, "driver handle IN"=w5297) -> ("driver handle OUT"=w5302:i32)  [unwired: 1 in, 2 out]
            n2034 = case shown="True" "Averaging" {
              tunnel: w5289 -> [w5340 w5345]
              tunnel: [w5340 w5344] -> w5285
              tunnel: w5288 -> [_ w5342]
              frame False {
              }
              frame True {
                (unwired) 1
                w5350 = 1
                n2035 = feedback #32(w5342) -> (w5341:u32[][])
                n2036 = Add(x=w5345, y=w5341) -> (x+y=w5346:u32[][])
                n2037 = Select(t=w5342, s="Reset Averaging", f=w5346) -> (s? t:f=w5348:u32[][])
                n2038 = feedback-in #32(w5348) -> ()
                n2039 = feedback #33(w5350) -> (w5343:i32)
                n2040 = Divide(x=w5346, y=w5343) -> (x/y=w5347:dbl[][])
                n2041 = Increment(x=w5343) -> (x+1=w5351:i32)
                n2042 = To Unsigned Long Integer(number=w5347) -> (unsigned 32bit integer=w5344:u32[][])
                n2043 = Select(t=w5350, s="Reset Averaging", f=w5351) -> (s? t:f=w5349:i32)
                n2044 = feedback-in #33(w5349) -> ()
              }
            }
            n2045 = call "DMR_ImageRequestSingle.vi"("request control IN"=0, "driver handle IN"=w5302) -> ("driver handle OUT"=w5300:i32)  [unwired: 3 out]
            n2046 = disable-structure shown="Disabled" {
              disable-tunnel: w5285 -> [w5317 _]
              disable-tunnel: w5281 -> [w5316 _]
              frame Disabled {
                n2047 = To Double Precision Float(number=w5317) -> (double precision float=w5315:dbl[][])
                n2048 = In Range and Coerce(upper limit="Intensity Upper", x=w5315, lower limit="Intensity Lower") -> (coerced(x)=w5314:dbl[][])  [unwired: 1 out]
                n2049 = Subtract(x="Intensity Upper", y="Intensity Lower") -> (x-y=w5311:dbl)
                n2050 = Subtract(x=w5314, y="Intensity Lower") -> (x-y=w5312:dbl[][])
                n2051 = Divide(x=w5312, y=w5311) -> (x/y=w5313:dbl[][])
                n2052 = Multiply(x=255.0, y=w5313) -> (x*y=w5309:dbl[][])
                n2053 = To Unsigned Byte Integer(number=w5309) -> (unsigned 8bit integer=w5318:u8[][])
                n2054 = call "IMAQ ArrayToImage"("Image Pixels (U8)"=w5318, "Image"=w5316) -> ("Image Out"=w5305:T2)  [unwired: 4 in, 5 out]
                n2055 = First Call?() -> (First Call?: T/F=w5306:bool)
                n2056 = case shown="True" w5306 {
                  tunnel: w5305 -> [w5319 w5330]
                  frame False {
                    n2057 = flat-sequence {
                      tunnel: w5319 -> [w5325]
                      frame #0 {
                        w5322 = FALSE ("Get/Set Status? (Set)")
                        w5321 = 0 ("Window Number (0...15)")
                        n2058 = call "IMAQ WindSize"("Get/Set Status? (Set)"=w5322, "Window Number"=w5321) -> ("Width & Height out"=→"Window Size":cluster{"Width":i32, "Height":i32})  [unwired: 4 in, 2 out]
                        n2059 = call "IMAQ WindMove"("Window Number (0...15)"=w5321, "Get/Set Status? (Set)"=w5322) -> ("Coordinates (screen)"=→"Window Position":cluster{"X Position":i32, "Y Position":i32})  [unwired: 3 in, 1 out]
                        n2060 = call "IMAQ WindDraw"("Resize to Image Size? (Y)"=FALSE, "Window Number (0...15)"=w5321, "Image"=w5325) -> ()  [unwired: 7 in, 2 out]
                      }
                      frame #1 {
                        n2061 = call "IMAQ WindZoom 2"("Center Point"="Center Point", "Zoom to Fit? (False)"=FALSE, "Zoom Factor"="Zoom Factor") -> ()  [unwired: 5 in, 4 out]
                      }
                    }
                  }
                  frame True {
                    n2062 = flat-sequence {
                      tunnel: w5330 -> [w5333]
                      tunnel: [w5331] -> w5329
                      tunnel: w5329 -> [w5335]
                      frame #0 {
                        w5332 = TRUE ("Resize to Image Size? (Y)")
                        w5331 = 0 ("Window Number (0...15)")
                        n2063 = call "IMAQ WindNonTearing"("Window Number"=w5331, "NonTearing? (True)"=w5332) -> ()  [unwired: 8 in, 2 out]
                        n2064 = call "IMAQ WindDraw"("Resize to Image Size? (Y)"=w5332, "Window Number (0...15)"=w5331, "Image"=w5333) -> ()  [unwired: 7 in, 2 out]
                      }
                      frame #1 {
                        n2065 = call "IMAQ WindSize"("Scrollbars? (N)"=FALSE, "Width & Height"="Initial Window Size", "Window Number"=w5335) -> ()  [unwired: 3 in, 3 out]
                        n2066 = call "IMAQ WindMove"("Window Number (0...15)"=w5335, "Coordinates (screen)"="Initial Window Position") -> ()  [unwired: 3 in, 2 out]
                      }
                    }
                  }
                }
              }
              frame Enabled {
              }
            }
            n2067 = To Unsigned Byte Integer(number=w5285) -> (unsigned 8bit integer=w5283:u8[][])
            n2068 = call "IMAQ ArrayToImage"("Image Pixels (U8)"=w5283, "Image"=w5284) -> ("Image Out"=w5282:T2)  [unwired: 4 in, 5 out]
            "Primary Video Display" <- w5282
            n2069 = case shown="True" "Save Video" {
              tunnel: w5286 -> [_ w5339]
              tunnel: w5282 -> [_ w5338]
              frame False {
              }
              frame True {
                n2070 = call "IMAQ AVI Write Frame"("Image"=w5338, "Avi Refnum"=w5339) -> ()  [unwired: 2 in, 8 out]
              }
            }
            n2071 = case shown="True" "Save Image" {
              tunnel: w5283 -> [_ w5354]
              tunnel: w5280 -> [_ w5353]
              frame False {
              }
              frame True {
                n2072 = call <vilib>:"Flatten Pixmap.vi"("colors"=w5353, "8-bit pixmap"=w5354) -> ("image data"=w5360:T47)  [unwired: 4 in, 5 out]
                n2073 = call "Create new save file.vi"("Insert"="video_frame_" ("string"), "Ext"=".bmp" ("string"), "Index In"="Image Index") -> ("Path Out"=w5356:path, "Index Out"=w5361:dbl)
                n2074 = Increment(x=w5361) -> (x+1=w5355:dbl)
                n2075 = local write "Image Index"(w5355) -> ()
                n2076 = call <vilib>:"Write BMP File.vi"("image data"=w5360, "path to BMP file"=w5356) -> ()  [unwired: 1 in, 9 out]
              }
            }
          }
        }
        n2077 = node-c288(w5242) -> ()  [unwired: 1 out]
      }
      n2078 = node-c288(w5226) -> ()  [unwired: 1 out]
      n2079 = call "DMR_CloseDevice.vi"("driver handle IN"=w5231) -> ()  [unwired: 1 in, 4 out]
    }
    frame #4 {
      n2080 = call "DMR_Close.vi"() -> ()  [unwired: 1 out]
    }
  }
  n2081 = timed-loop "Oscillate AOD (debugging)" {
    tunnel: w8 -> [w5367]
    tunnel: [w5366] -> w53
    timing: w48 -> [_]
    timing-out: [_] -> w47
    stop <- w5366 stop-if-true
    n2082 = node-c288() -> ()  [unwired: 2 out]
    n2083 = event shown="[0] \"Oscillate Set 1\", \"Fish for Tether\": Value Change" {
      selector: _ -> [_ _ _]
      dyn-events: _ -> [_ _ _]
      timeout: _ -> [_ _ _]
      tunnel: w5367 -> [w5374 _ _]
      tunnel: [FALSE ("Stop All") _ w5642] -> w5366
      event "Oscillate Set 1", "Fish for Tether": Value Change {
        n2084 = event-data() -> ()  [unwired: 6 out]
        n2085 = local read "Oscillate Set 1"() -> (w5373:bool)
        n2086 = Or(x=w5373, y="Fish for Tether") -> (x .or. y?=w5371:bool)
        n2087 = case shown="True" w5371 {
          tunnel: w5374 -> [_ w5376]
          tunnel: "Fish for Tether" -> [_ w5375]
          frame False {
          }
          frame True {
            n2088 = case shown="True" w5375 {
              frame False {
              }
              frame True {
                n2089 = local write "Scan axis 2"(TRUE) -> ()
                n2090 = local write "Tether"(FALSE ("Tether")) -> ()
              }
            }
            n2091 = node-c288() -> (w5378:T23)  [unwired: 4 out]
            n2092 = timed-loop "Oscillate AOD" {
              timing: w5378 -> [_]
              timing-out: [_] -> w5377
              tunnel: w5376 -> [w5388]
              tunnel: w5375 -> [w5387]
              i -> [w5390]
              stop <- w5386 stop-if-true
              n2093 = node-c288() -> (w5389:i64)  [unwired: 1 out]
              n2094 = flat-sequence {
                tunnel: w5390 -> [w5417]
                tunnel: w5389 -> [w5416]
                tunnel: w5388 -> [w5395]
                tunnel: w5387 -> [w5398]
                tunnel: [w5398] -> w5385
                tunnel: [w5397] -> w5384
                tunnel: [w5394] -> w5383
                tunnel: [w5391] -> w5381
                tunnel: w5385 -> [w5453]
                tunnel: w5384 -> [w5451]
                tunnel: w5383 -> [w5450]
                tunnel: [w5449] -> w5382
                tunnel: w5381 -> [w5448]
                tunnel: [w5516] -> w5386
                tunnel: w5382 -> [w5515]
                frame #0 {
                  n2095 = Divide(x=w5416, y=i64 1000) -> (x/y=w5411:dbl)
                  n2096 = Multiply(x=w5411, y=w5417) -> (x*y=w5413:dbl)
                  n2097 = local read "BD 1 Frequency 2 (MHz)"() -> (w5396:dbl)
                  n2098 = Multiply(x="Osc. freq. (Hz)", y=6.283185307179586) -> (x*y=w5414:dbl)
                  n2099 = Multiply(x=w5414, y=w5413) -> (x*y=w5393:dbl)
                  n2100 = local read "BD 1 Frequency 1 (MHz)"() -> (w5401:dbl)
                  n2101 = case shown="True" w5398 {
                    tunnel: w5393 -> [w5423 w5428]
                    tunnel: w5401 -> [_ w5439]
                    tunnel: w5396 -> [_ w5440]
                    tunnel: [w5420 w5434] -> w5399
                    tunnel: [FALSE w5431] -> w5394
                    tunnel: [0.0 w5424] -> w5391
                    frame False {
                      n2102 = Sine(x=w5423) -> (sin(x)=w5421:dbl)
                      n2103 = Multiply(x=w5421, y="Osc. amp. (MHz)") -> (x*y=w5420:dbl)
                    }
                    frame True {
                      n2104 = Cosine(x=w5428) -> (cos(x)=w5443:dbl)
                      n2105 = Subtract(x=w5440, y=w5439) -> (x-y=w5438:dbl)
                      n2106 = Decrement(x=w5443) -> (x-1=w5442:dbl)
                      n2107 = Subtract(x=w5438, y="Closest Delta (MHz)") -> (x-y=w5435:dbl)
                      n2108 = Divide(x=w5442, y=-2.0) -> (x/y=w5436:dbl)
                      n2109 = Multiply(x=w5436, y=w5435) -> (x*y=w5434:dbl)
                      n2110 = local read "Vec Mean of T1 T2"() -> (w5430:dbl[])
                      n2111 = Greater?(x=w5430, y="Stop F (pN)") -> (0:w5432:bool[])
                      n2112 = Or Array Elements(Boolean array=w5432) -> (logical OR=w5431:bool)
                      n2113 = Divide(x=w5428, y=6.283185307179586) -> (x/y=w5427:dbl)
                      n2114 = Round Toward +Infinity(x=w5427) -> (ceil(x): smallest int >= x=w5424:dbl)
                      "Attempts" <- w5424
                      n2115 = Greater?(x=w5424, y="Attempt Limit") -> (0:w5426:bool)
                      n2116 = case shown="True" w5426 {
                        frame False {
                        }
                        frame True {
                          n2117 = local write "Fish for Tether"(FALSE ("Fish for Tether")) -> ()
                          n2118 = call <vilib>:"Beep.vi"() -> ()  [unwired: 3 in, 9 out]
                          n2119 = local read "Messages"() -> (w5445:string)
                          n2120 = call "Update messages.vi"("Message to add"="Tether fishing timeout." ("Messages"), "Old message string"=w5445) -> ("New message string"=→"Messages":string)
                        }
                      }
                    }
                  }
                  n2121 = local read "BD 2 Frequency 1 (MHz)"() -> (w5400:dbl)
                  n2122 = Select(t=w5401, s="Scan axis 2", f=w5400) -> (s? t:f=w5404:dbl)
                  n2123 = Add(x=w5399, y=w5404) -> (x+y=w5397:dbl)
                  n2124 = Select(t=w5397, s="Scan axis 2", f=w5401) -> (s? t:f=w5407:dbl)
                  n2125 = Select(t=w5400, s="Scan axis 2", f=w5397) -> (s? t:f=w5406:dbl)
                  n2126 = local read "Y RF Frequency Limits (MHz)"() -> (w5402:T16)
                  n2127 = local read "X RF Frequency Limits (MHz)"() -> (w5403:T16)
                  n2128 = local read "BD 1 Frequency 3 (MHz)"() -> (w5410:dbl)
                  n2129 = local read "BD 2 Frequency 2 (MHz)"() -> (w5409:dbl)
                  n2130 = local read "BD 2 Frequency 3 (MHz)"() -> (w5408:dbl)
                  n2131 = call "set RF board frequency - interlace.vi"("Board 2 Frequency Limits"=w5402, "Board 1 Frequency Limits"=w5403, "FPGA VI Reference In"=w5395, "Board 2 Frequency 3 (MHz)"=w5408, "Board 1 Frequency 3 (MHz)"=w5410, "Board 2 Frequency 2 (MHz)"=w5409, "Board 2 Frequency 1 (MHz)"=w5406, "Board 1 Frequency 2 (MHz)"=w5396, "Board 1 Frequency 1  (MHz)"=w5407) -> ()  [unwired: 1 in, 2 out]
                }
                frame #1 {
                  n2132 = And(x=w5453, y=w5450) -> (x .and. y?=w5452:bool)
                  n2133 = case "Only if were fishing and now formed tether" shown="True" w5452 {
                    tunnel: w5451 -> [w5455 w5468]
                    tunnel: [w5454 w5467] -> w5449
                    tunnel: w5448 -> [_ w5463]
                    frame False {
                      n2134 = local read "Fish for Tether"() -> (w5454:bool)
                      n2135 = case shown="False" w5454 {
                        tunnel: w5455 -> [w5456 _]
                        frame False {
                          n2136 = property on="BD 1 Frequency 1 (MHz)" class="DigNum (strict)"("Val(Sgnl)"=w5456) -> ()  [unwired: 2 in, 2 out]
                        }
                        frame True {
                        }
                      }
                    }
                    frame True {
                      w5467 = FALSE ("Fish for Tether")
                      n2137 = call <vilib>:"Beep.vi"() -> ()  [unwired: 3 in, 9 out]
                      n2138 = Number To Decimal String(number=w5463, width (-)=i16 1) -> (decimal integer string=w5461:string)
                      n2139 = case shown="\"2\", \"3\", \"4\", \"5\", \"6\"" "Then..." {
                        selector: "Then..." -> [_ w5471]
                        tunnel: w5468 -> [w5470 _]
                        frame "1", Default {
                          n2140 = property on="BD 1 Frequency 1 (MHz)" class="DigNum (strict)"("Val(Sgnl)"=w5470) -> ()  [unwired: 2 in, 2 out]
                        }
                        frame "2", "3", "4", "5", "6" {
                          n2141 = flat-sequence {
                            tunnel: w5471 -> [w5473]
                            frame #0 {
                              n2142 = property on="Trap Delta (MHz)" class="DigNum (strict)"("Val(Sgnl)"="Move to Delta 1 (MHz)") -> ()  [unwired: 2 in, 2 out]
                            }
                            frame #1 {
                              n2143 = case shown="\"5\", \"6\"" w5473 {
                                selector: w5473 -> [w5476 w5486 _]
                                frame "3", "4" {
                                n2144 = flat-sequence {
                                tunnel: w5476 -> [w5477]
                                tunnel: [w5477] -> w5474
                                tunnel: [w5479] -> w5475
                                tunnel: w5474 -> [w5479]
                                tunnel: w5475 -> [w5483]
                                frame #0 {
                                n2145 = property on="Green Laser ON/Interlacing" class="Bool (strict)"("Val(Sgnl)"=TRUE ("Value (Signaling)")) -> ()  [unwired: 2 in, 2 out]
                                }
                                frame #1 {
                                n2146 = Multiply(x="Wait Before Save (s)", y=u32 1000 ("x")) -> (x*y=w5481:u32)
                                n2147 = Wait (ms)(milliseconds to wait=w5481) -> ()  [unwired: 1 out]
                                }
                                frame #2 {
                                n2148 = property on="Start Saving" class="Bool (strict)"("Value"=TRUE ("Start Saving")) -> ()  [unwired: 2 in, 2 out]
                                n2149 = case shown="\"4\"" w5483 {
                                frame Default {
                                }
                                frame "4" {
                                n2150 = property on="Fl. Triggered..." class="Bool (strict)"("Val(Sgnl)"=TRUE ("Value (Signaling)")) -> ()  [unwired: 2 in, 2 out]
                                }
                                }
                                }
                                }
                                }
                                frame "5", "6" {
                                n2151 = stacked-sequence {
                                tunnel: w5486 -> [_ _ _ _ _ _ _ _ w5503 _ _]
                                frame #0 {
                                n2152 = Replace Array Subset(array=u32[] [0] ("Index Values"), new element="Raster Set Upon Tether", index=0) -> (w5487:u32[])
                                n2153 = property on="Saved AOD Raster Scan Parameter Sets" class="Arr (strict)"("Index Values"=w5487) -> ()  [unwired: 2 in, 2 out]
                                }
                                frame #1 {
                                n2154 = Wait (ms)(milliseconds to wait=u32 500) -> ()  [unwired: 1 out]
                                }
                                frame #2 {
                                n2155 = property on="Load parameters" class="Bool (strict)"("Val(Sgnl)"=TRUE ("Value (Signaling)")) -> ()  [unwired: 2 in, 2 out]
                                }
                                frame #3 {
                                n2156 = Wait (ms)(milliseconds to wait=u32 500) -> ()  [unwired: 1 out]
                                }
                                frame #4 {
                                n2157 = property on="Trap Raster Scan" class="Bool (strict)"("Val(Sgnl)"=TRUE ("Value (Signaling)")) -> ()  [unwired: 2 in, 2 out]
                                }
                                frame #5 {
                                n2158 = Wait (ms)(milliseconds to wait=u32 2000) -> ()  [unwired: 1 out]
                                }
                                frame #6 {
                                n2159 = while {
                                stop <- w5498 stop-if-true
                                n2160 = local read "Raster Scanning..."() -> (w5497:bool)
                                n2161 = local read "Saving..."() -> (w5500:bool)
                                n2162 = Wait (ms)(milliseconds to wait=u32 100) -> ()  [unwired: 1 out]
                                n2163 = Not(x=w5500) -> (.not. x?=w5499:bool)
                                n2164 = Not(x=w5497) -> (.not. x?=w5496:bool)
                                n2165 = And(x=w5499, y=w5496) -> (x .and. y?=w5498:bool)
                                }
                                }
                                frame #7 {
                                n2166 = property on="Trap Delta (MHz)" class="DigNum (strict)"("Val(Sgnl)"="Move to Delta 2 (MHz)") -> ()  [unwired: 2 in, 2 out]
                                }
                                frame #8 {
                                n2167 = local read "Tether"() -> (w5504:bool)
                                n2168 = case shown="True" w5504 {
                                tunnel: w5503 -> [_ w5505]
                                frame False {
                                }
                                frame True {
                                n2169 = flat-sequence {
                                tunnel: w5505 -> [w5507]
                                frame #0 {
                                n2170 = Wait (ms)(milliseconds to wait=u32 500) -> ()  [unwired: 1 out]
                                }
                                frame #1 {
                                n2171 = case shown="\"6\"" w5507 {
                                frame Default {
                                }
                                frame "6" {
                                n2172 = property on="Green Laser ON/Interlacing" class="Bool (strict)"("Val(Sgnl)"=TRUE ("Green Laser ON/Interlacing")) -> ()  [unwired: 2 in, 2 out]
                                }
                                }
                                }
                                frame #2 {
                                n2173 = Wait (ms)(milliseconds to wait=u32 500) -> ()  [unwired: 1 out]
                                }
                                frame #3 {
                                n2174 = local write "Start Saving"("Save at end (5, 6)") -> ()
                                }
                                }
                                }
                                }
                                }
                                frame #9 {
                                n2175 = local read "Bead Sep. Int. Time (s)"() -> (w5513:dbl)
                                n2176 = Multiply(x=w5513, y=1000.0) -> (x*y=w5512:dbl)
                                n2177 = Wait (ms)(milliseconds to wait=w5512) -> ()  [unwired: 1 out]
                                }
                                frame #10 {
                                n2178 = property on="Rescale on Mean" class="Bool (strict)"("Val(Sgnl)"=TRUE ("Value (Signaling)")) -> ()  [unwired: 2 in, 2 out]
                                }
                                }
                                }
                                frame "2", Default {
                                }
                              }
                            }
                          }
                        }
                      }
                      n2179 = Concatenate Strings("Formed tether in ", w5461, " attempt(s)." ("string")) -> (w5458:string)
                      n2180 = local read "Messages"() -> (w5465:string)
                      n2181 = local write "Fish for Tether"(w5467) -> ()
                      n2182 = call "Update messages.vi"("Message to add"=w5458, "Old message string"=w5465) -> ("New message string"=w5464:string)
                      n2183 = local write "Messages"(w5464) -> ()
                      n2184 = Get Date/Time In Seconds() -> (seconds since 1Jan1904=→"Time tether formed":timestamp)
                      "Tether" <- "Tether Alarm?"
                    }
                  }
                }
                frame #2 {
                  n2185 = local read "Oscillate Set 1"() -> (w5520:bool)
                  n2186 = local read "Stop All"() -> (w5518:bool)
                  n2187 = Or(x=w5520, y=w5515) -> (x .or. y?=w5517:bool)
                  n2188 = Not(x=w5517) -> (.not. x?=w5519:bool)
                  n2189 = Compound Arithmetic op=OR(w5518, w5519) -> (w5516:bool)
                }
              }
              n2190 = node-c288() -> ()  [unwired: 2 out]
            }
            n2191 = node-c288(w5377) -> ()  [unwired: 1 out]
          }
        }
      }
      event "Fl. Triggered...": Value Change {
        n2192 = event-data() -> ()  [unwired: 7 out]
        n2193 = case shown="True" "Fl. Triggered..." {
          frame False {
          }
          frame True {
            n2194 = node-c288() -> (w5530:T23)  [unwired: 4 out]
            n2195 = timed-loop {
              timing: w5530 -> [_]
              timing-out: [_] -> w5529
              tunnel: "Action" -> [w5534]
              shift-right: [w5531] -> _
              shift-left: u8 255 -> [w5533]
              stop <- w5535 stop-if-true
              n2196 = node-c288() -> ()  [unwired: 2 out]
              n2197 = flat-sequence {
                tunnel: w5534 -> [w5547]
                tunnel: w5533 -> [w5544]
                tunnel: [w5543] -> w5532
                tunnel: [w5633] -> w5535
                tunnel: w5532 -> [w5632]
                tunnel: [w5632] -> w5531
                frame #0 {
                  n2198 = local read "Delta Fl. 2"() -> (w5538:dbl)
                  n2199 = local read "Delta Fl. 1"() -> (w5539:dbl)
                  n2200 = Select(t=w5539, s="APD to Watch", f=w5538) -> (s? t:f=w5537:dbl)
                  n2201 = Multiply(x="Fl. Delta Thresh. (kHz)", y=1000.0) -> (x*y=w5546:dbl)
                  n2202 = Greater?(x=w5537, y=w5546) -> (0:w5541:bool)
                  n2203 = Or(x="Force Yank", y=w5541) -> (x .or. y?=w5542:bool)
                  n2204 = case shown="True" w5542 {
                    tunnel: w5547 -> [_ w5557]
                    tunnel: w5544 -> [w5549 w5553]
                    tunnel: [w5549 w5550] -> w5543
                    frame False {
                    }
                    frame True {
                      n2205 = flat-sequence {
                        tunnel: w5554 -> [w5563]
                        tunnel: [w5563] -> w5558
                        tunnel: w5557 -> [w5562]
                        tunnel: [w5562] -> w5556
                        tunnel: [w5561] -> w5555
                        tunnel: w5553 -> [w5560]
                        tunnel: [w5559] -> w5552
                        tunnel: w5558 -> [w5588]
                        tunnel: w5556 -> [w5587]
                        tunnel: w5555 -> [w5586]
                        tunnel: w5552 -> [w5585]
                        tunnel: [w5585] -> w5551
                        tunnel: w5551 -> [w5630]
                        tunnel: [w5630] -> w5550
                        frame #0 {
                          n2206 = call <vilib>:"Beep.vi"() -> ()  [unwired: 3 in, 9 out]
                          n2207 = local write "Waiting"(FALSE ("Waiting")) -> ()
                          n2208 = Increment(x=w5560) -> (x+1=w5559:u8)
                          n2209 = case shown="\"Yank\"" w5562 {
                            tunnel: w5559 -> [_ _ w5569]
                            frame "Image" {
                              n2210 = property on="Confocal Image" class="Bool (strict)"("Val(Sgnl)"=TRUE ("Value (Signaling)")) -> ()  [unwired: 2 in, 2 out]
                            }
                            frame "Alarm", Default {
                            }
                            frame "Yank" {
                              n2211 = flat-sequence {
                                tunnel: w5569 -> [w5572]
                                tunnel: [w5571] -> w5568
                                tunnel: ["N Array El"] -> w5567
                                tunnel: w5568 -> [w5582]
                                tunnel: w5567 -> [w5578]
                                frame #0 {
                                n2212 = Multiply(x="Yank Delay (s)", y=1000.0) -> (x*y=w5575:dbl)
                                n2213 = Quotient & Remainder(x=w5572, y="N Array El") -> (x-y*floor(x/y)=w5571:u8)  [unwired: 1 out]
                                n2214 = Wait (ms)(milliseconds to wait=w5575) -> ()  [unwired: 1 out]
                                }
                                frame #1 {
                                n2215 = Random Number (0-1)() -> (number: 0 to 1=w5579:dbl)
                                n2216 = Multiply(x=w5578, y=w5579) -> (x*y=w5577:dbl)
                                n2217 = Round Toward -Infinity(1:w5577) -> (0:w5576:dbl)
                                n2218 = Select(t=w5576, s="Random Choice", f=w5582) -> (s? t:f=w5580:dbl)
                                n2219 = Index Array(array="Yank to Delta Array (MHz)", index=w5580) -> (element=w5583:dbl)
                                n2220 = property on="Trap Delta (MHz)" class="DigNum (strict)"("Val(Sgnl)"=w5583) -> ()  [unwired: 2 in, 2 out]
                                }
                              }
                            }
                          }
                          n2221 = local read "Time (s)"() -> (w5561:dbl)
                          "Fl. High" <- TRUE ("Yanking")
                        }
                        frame #1 {
                          n2222 = node-c288() -> (w5590:T23)  [unwired: 4 out]
                          n2223 = timed-loop {
                            timing: w5590 -> [_]
                            timing-out: [_] -> w5589
                            tunnel: w5588 -> [w5606]
                            tunnel: w5587 -> [w5604]
                            tunnel: w5586 -> [w5603]
                            stop <- w5605 stop-if-true
                            n2224 = node-c288() -> ()  [unwired: 2 out]
                            n2225 = local read "Fl. Delta Thresh. (kHz)"() -> (w5598:dbl)
                            n2226 = local read "Fl. Triggered..."() -> (w5607:bool)
                            n2227 = local read "Delta Fl. 1"() -> (w5594:dbl)
                            n2228 = local read "Delta Fl. 2"() -> (w5592:dbl)
                            n2229 = local read "Stop All"() -> (w5601:bool)
                            n2230 = local read "APD to Watch"() -> (w5593:bool)
                            n2231 = Select(t=w5594, s=w5593, f=w5592) -> (s? t:f=w5591:dbl)
                            n2232 = Not(x=w5607) -> (.not. x?=w5602:bool)
                            n2233 = Multiply(x=w5598, y=1000.0) -> (x*y=w5597:dbl)
                            n2234 = Negate(x=w5597) -> (-x=w5596:dbl)
                            n2235 = Less?(x=w5591, y=w5596) -> (x < y?=w5600:bool)
                            n2236 = Compound Arithmetic op=OR(w5600, w5601, w5602, "Force Reset") -> (w5605:bool)
                            n2237 = case shown="True" w5605 {
                              tunnel: w5606 -> [_ w5618]
                              tunnel: w5604 -> [_ w5617]
                              tunnel: w5603 -> [_ w5615]
                              frame False {
                              }
                              frame True {
                                n2238 = case shown="\"Yank\"" w5617 {
                                tunnel: w5618 -> [_ w5619]
                                frame "Image", Default {
                                }
                                frame "Yank" {
                                n2239 = flat-sequence {
                                tunnel: [w5624] -> w5620
                                tunnel: w5619 -> [w5624]
                                tunnel: w5620 -> [w5625]
                                frame #0 {
                                n2240 = local read "Yank Delay (s)"() -> (w5623:dbl)
                                n2241 = Multiply(x=w5623, y=1000.0) -> (x*y=w5621:dbl)
                                n2242 = Wait (ms)(milliseconds to wait=w5621) -> ()  [unwired: 1 out]
                                }
                                frame #1 {
                                n2243 = property on="Trap Delta (MHz)" class="DigNum (strict)"("Val(Sgnl)"=w5625) -> ()  [unwired: 2 in, 2 out]
                                }
                                }
                                }
                                }
                                n2244 = local read "Time (s)"() -> (w5616:dbl)
                                n2245 = Subtract(x=w5616, y=w5615) -> (x-y=w5612:dbl)
                                "Duration (s)" <- w5612
                                n2246 = Number To Decimal String(number=w5612, width (-)=i16 0) -> (decimal integer string=w5610:string)
                                n2247 = Concatenate Strings(w5610, " s fluorescence event." ("string")) -> (w5608:string)
                                n2248 = local read "Messages"() -> (w5614:string)
                                n2249 = call "Update messages.vi"("Message to add"=w5608, "Old message string"=w5614) -> ("New message string"=w5613:string)
                                n2250 = call <vilib>:"Beep.vi"() -> ()  [unwired: 3 in, 9 out]
                                n2251 = local write "Messages"(w5613) -> ()
                              }
                            }
                            n2252 = node-c288() -> ()  [unwired: 2 out]
                          }
                          n2253 = node-c288(w5589) -> ()  [unwired: 1 out]
                        }
                        frame #2 {
                          n2254 = local write "Fl. High"(FALSE ("Yanking")) -> ()
                        }
                      }
                      n2255 = local read "Trap Delta (MHz)"() -> (w5554:dbl)
                    }
                  }
                }
                frame #1 {
                  n2256 = local read "Stop All"() -> (w5636:bool)
                  n2257 = local read "Fl. Triggered..."() -> (w5634:bool)
                  n2258 = Not(x=w5634) -> (.not. x?=w5635:bool)
                  n2259 = Or(x=w5635, y=w5636) -> (x .or. y?=w5633:bool)
                  n2260 = Not(x=w5633) -> (.not. x?=→"Waiting":bool)
                }
              }
              n2261 = node-c288() -> ()  [unwired: 2 out]
            }
            n2262 = node-c288(w5529) -> ()  [unwired: 1 out]
          }
        }
      }
      event "Stop All": Value Change {
        n2263 = event-data() -> ()  [unwired: 7 out]
        n2264 = local read "Stop All"() -> (w5642:bool)
      }
    }
    n2265 = node-c288() -> ()  [unwired: 2 out]
  }
  n2266 = node-c288(w49) -> ()  [unwired: 1 out]
  n2267 = node-c288(w36) -> ()  [unwired: 1 out]
  n2268 = VISA Close(VISA resource name=w40, error in (no error)=w39) -> (error out=w93:errorcluster)
  n2269 = node-c288(w51) -> ()  [unwired: 1 out]
  n2270 = call <vilib>:"Simple Error Handler.vi"("error in (no error)"=w93) -> ()  [unwired: 1 in, 8 out]
  n2271 = node-c288(w47) -> ()  [unwired: 1 out]
  n2272 = node-c288(w148) -> ()  [unwired: 1 out]
  n2273 = flat-sequence {
    tunnel: w243 -> [w5646]
    tunnel: w245 -> [w5647]
    tunnel: [w5645] -> w224
    tunnel: [w5644] -> w223
    tunnel: w205 -> [_]
    tunnel: w203 -> [_]
    tunnel: w156 -> [_]
    tunnel: w53 -> [_]
    tunnel: w224 -> [w5674]
    tunnel: w223 -> [w5675]
    frame #0 {
      w5643 = FALSE ("AI to FIFO")
      n2274 = xnode "Read/Write Control"("FPGA VI Reference In"=w5647, "error in"=w5646, "AI to FIFO"=w5643, "APD to FIFO"=w5643) -> ("FPGA VI Reference Out"=w5645:T19, "error out"=w5644:errorcluster)
    }
    frame #1 {
      n2275 = xnode "Close FPGA VI Reference"("FPGA VI Reference In"=w5674, "error in"=w5675) -> ("error out"=→"error out":errorcluster)
    }
  }
